vi "UNITEST MAIN v01.2.vi"() -> ()   [LabVIEW 2025]
uses:
  controls/LAB-IQ UI Data.ctl
  HEAVE vi's/Heave Write enum.ctl
  HEAVE vi's/Heave Right enum.ctl
  SWAY vi's/Sway Write enum.ctl
  SWAY vi's/Sway Right enum.ctl
  d081153b-36ca-4bc4-8478-749476f82ba4.vi
  1202965f-721d-4349-8d61-5de826f379ef.vi
  785ec975-e53d-4ed4-be48-2cc128d7a91f.vi
  02c5850b-52e8-4ed5-91f8-6f0ad62f4994.vi
  1223eb78-e4c4-4b69-bf80-185c82055158.vi
  e5651a45-6a49-4a3f-b503-ff1eaf449b4a.vi
  <vilib>/Utility/error.llb/Trim Whitespace One-Sided.vi
  support/Message Queue/Enqueue Message (Single).vi
  <vilib>/Utility/error.llb/Error Cluster From Error Code.vi
  <vilib>/Utility/file.llb/Read Delimited Spreadsheet (string).vi
  <vilib>/Utility/file.llb/Write Delimited Spreadsheet (string).vi
  <vilib>/ErrorRing/Error Ring.xnode
  support/Message Queue/LAB-IQ Message Queue.lvlib
  support/User Event - Stop/LAB-IQ User Event - Stop.lvlib
panel:
  out "Scratch Start Recording":bool
  in  "SwaySpeed Set":bool
  in  "Update":bool
  in  "Analysis Home":bool
  in  "Installation/Replacement completed":bool
  in  "Loahead":bool
  in  "Heave and Surge COM Port:":refnum<visa-resource-name>="COM9"
  in  "Sway COM Port:":refnum<visa-resource-name>="COM10"
  out "Test Trip":bool
  out "Hymidity":bool
  in  "Humidity Disable trip":bool=TRUE
  in  "CoF Trip  2":dbl=540.0 min=100.0 max=540.0 step=1.0
  in  "File Path :  2":path
  out "Wear Track Diameter":dbl
  in  "Stribeck table":bool
  in  "seq":bool=TRUE
  out "Drive Error":string
  out "mm/s  Surge":dbl=7.0 caption="Jog" min=0.001 max=50.0 step=0.0001 format="%.2f"
  in  "Update Surge Speed":bool
  out "mm/s  Sway":dbl=7.0 caption="Jog" min=0.001 max=50.0 step=0.0001 format="%.2f"
  in  "Update Sway Speed":bool
  in  "Update Heave Speed":bool
  out "mm/s Heave":dbl=7.0 caption="Jog" min=0.001 max=30.0 step=0.0001 format="%.2f"
  in  "mm/sec":dbl=1.0 caption="Jog" min=0.001 max=50.0 step=0.001 format="%.2f"
  out "Scratch Start Test":bool
  in  "HomeScratch":bool
  in  "TEST SELECTION":enum32{"Time", "Cycle"}(radio)
  in  "Sway Loop Delay":dbl
  in  "Sway PID Speed":dbl=1.0 format="%.4f"
  in  "Sway Jog Speed":dbl=1.0 format="%.4f"
  out "HEAVE ENABLE":bool
  in  "SPARE  5":u8
  in  "Manual Write SWAY":bool
  out "SWAY WRITE":string
  in  "SPARE  4":u8
  in  "SPARE  3":u8
  in  "SPARE 2":u8
  in  "SPARE 1":u8
  out "Spare 15":u8
  out "Spare 14":u8
  out "Spare 13":u8
  out "Spare 12":u8
  out "Spare 11":u8
  out "Spare 10":u8
  out "Spare 9":u8
  out "Spare 8":u8
  out "Spare 7":u8
  out "Spare 6":u8
  out "Spare 5":u8
  out "Spare 4":u8
  out "Spare 3":u8
  out "Spare 2":u8
  out "Spare 1":u8
  out "Node Id":u8
  out "Read SWAY Temp":bool
  out "fwMinor":u8
  out "fwMajor":u8
  out "faultCode":u16
  out "Rotary POSE":sgl format="%#.6f"
  out "SWAY POSE":sgl format="%#.6f"
  out "Homed":u8
  out "State":u8
  out "Ack ID":u16
  in  "SPEED":sgl=10000.0
  in  "Distance":sgl=10000.0
  in  "Mode Command":u8=2
  out "Sequence ID":u16
  out "error out Read SWAY":errorcluster
  out "error out Write  SWAY":errorcluster
  out "SWAY READ":string
  in  "min_finetune_floor":dbl=0.15
  in  "min_deadband_floor":dbl=0.05
  in  "fine_tune_pct":dbl=100.0
  out "Start Test Temp":bool
  in  "AppLoadSeq scratch":bool
  out "Pulse delta":dbl
  in  "Fine Tune Zone":dbl=10.0
  in  "PID Delay (sec)":dbl=1.0 format="%#_6p"
  in  "Max_pos_limit":dbl=50000000.0
  in  "Min_pos_limit":dbl
  in  "i_limit":dbl=10.0
  in  "Max Step Linit":dbl=10.0
  in  "Init Step":dbl=10.0
  in  "pct_scale":dbl=100.0
  in  "Deadband":dbl=0.1
  in  "Kd":dbl
  in  "Ki":dbl
  in  "Kp":dbl=1.0
  out "Current Position":dbl
  in  "Set Load":dbl
  in  "Current Load":dbl
  in  "Manual Write Heave & Surge":bool
  out "Heave and Surge Write":string
  in  "Heave Loop Delay":dbl
  in  "Heave PID Speed":dbl=15.0
  in  "Surge Jog Speed":dbl=1.0 format="%.4f"
  in  "Heave Jog Speed":dbl=15.0
  in  "SPARE 4":u8
  in  "SPARE 3":u8
  in  "SPARE 2":u8
  in  "SPARE 1":u8
  out "Spare 15":u8
  out "Spare 14":u8
  out "Spare 13":u8
  out "Spare 12":u8
  out "Spare 11":u8
  out "Spare 10":u8
  out "Spare 9":u8
  out "Spare 8":u8
  out "Spare 7":u8
  out "Spare 6":u8
  out "Spare 5":u8
  out "Spare 4":u8
  out "Spare 3":u8
  out "Spare 2":u8
  out "Spare 1":u8
  out "Node Id":u8
  out "Read Heave Temp":bool
  out "fwMinor":u8
  out "fwMajor":u8
  out "faultCode":u16
  out "SURGE POSE":sgl format="%#.6f"
  out "HEAVE POSE":sgl format="%#.6f"
  out "Homed":u8
  out "State":u8
  out "Ack ID":u16
  in  "SPEED":sgl=10000.0
  in  "Distance":sgl=10000.0
  in  "Mode Command":u8=2
  out "Sequence ID":u16
  out "error out Read":errorcluster
  out "error out Write":errorcluster
  out "Heave and Surge Read":string
  out "Load Cell Temp":bool
  in  "Stop Scratch":bool
  in  "Enter Fixed SRR 2":dbl min=0.0 max=0.0 format="%.3f"
  in  "E.Velocity 2":bool=TRUE caption="SRR"
  in  "Tab Control 3":T1(tab)
  in  "Tab Control 5":enum32{""}(tab)
  in  "Tab Control 14":T2(tab)=enum."Motor Load"
  in  "Ramp MulFac":dbl=2.0
  in  "pulses LoadDiffRamp(2..10)":dbl=9.0
  in  "PulseControlRamp(diff<=3N)":dbl=5.0 min=1.0 max=1000.0 step=1.0 format="%#.1f"
  in  "SetLoadDeadband(%) Load(0-10N)":dbl=0.1 min=0.0001 max=100.0 step=0.0001 format="%#.6f"
  in  "PID gains out delay (microForce)":T3={"proportional gain (Kc)"=300.0, "integral time (Ti, min)"=0.00011, "derivative time (Td, min)"=0.0} {"derivative time (Td, min)" format="%.3f"; "integral time (Ti, min)" min=1e-05 max=100.0 step=1e-06 format="%.6f"; "proportional gain (Kc)" format="%.3f"}
  in  "Ramp":bool
  in  "Gain 2":dbl=0.016
  in  "pulses LoadDiff(2..10)":dbl=10.0
  in  "pulses LoadDiff(11..50)":dbl=40.0
  in  "PulseControl(diff<=3N)":dbl=1.0 min=1.0 max=1000.0 step=1.0 format="%#.1f"
  out "SetLoadDeadband(%)  2":dbl=1.0 min=0.001 max=100.0 step=0.001 format="%#.6f"
  in  "Dummy Run":bool
  out "Vertical load (N)":dbl format="%#.3f"
  in  "AutoTune":bool
  in  "Offset  3":dbl=1.5
  in  "apply load":bool
  in  "Enter ByPass Load":dbl
  in  "reinit 3":bool=TRUE
  in  "output range delay":cluster{"output high":dbl, "output low":dbl}={"output high"=100.0, "output low"=-100.0} {"output low" format="%.2f"; "output high" format="%.2f"}
  in  "PID gains out delay":T3={"proportional gain (Kc)"=30.0, "integral time (Ti, min)"=0.00101, "derivative time (Td, min)"=0.0} {"derivative time (Td, min)" format="%.3f"; "integral time (Ti, min)" min=1e-05 max=100.0 step=0.0001 format="%.4f"; "proportional gain (Kc)" format="%.3f"}
  in  "Bypass Load":bool
  in  "pulsesSent":dbl=200.0
  out "pulses":dbl
  out "actpid":dbl
  out "gFF Rot 7":cluster{dbl, dbl, dbl}(graph)
  in  "pulses LoadDiff(21..1000)":dbl=40.0
  in  "Delay":dbl=1.5 min=0.001 max=5.0 step=0.001 format="%#.6f"
  in  "deadband":dbl=0.2
  in  "Tab Control 26":enum32{"Page 1", "Page 2"}(tab)
  in  "ClearAll":bool
  out "Mz(Nm)":dbl[](array[numeric])
  out "My(Nm)":dbl[](array[numeric])
  out "Mx(Nm)":dbl[](array[numeric])
  in  "Save Dwell":dbl=0.015 caption="Save Dwell (sec)" min=0.0 max=5.0 step=0.001 format="%.3f"
  out "Mx":dbl[](graph)
  out "My":dbl[](graph)
  out "Mz":dbl[](graph)
  out "Fy(N)":dbl[](graph)
  out "Fz(N)":dbl[](graph)
  in  "ZeroAll":bool
  in  "Acq Delay (ms)":dbl=10.0
  in  "Burst Delay (ms)":dbl=10.0
  out "model":string
  out "SN":i32
  out "FFx(N)":dbl[](array[numeric])
  in  "Sensor IP":string="192.168.1.100"
  in  "Port":i32=8080
  out "FFy(N)":dbl[](array[numeric])
  out "Load(N)":dbl[](array[numeric])
  out "Fx(N)":dbl[](graph)
  out "AE":bool
  in  "delete Handle":bool
  in  "Create Handle":bool=TRUE
  out "ft_data":dbl[](array[numeric])=[1.0, 1.0, 1.0, 1.0, 1.0, 1.0]
  out "ft_range":dbl[](array[numeric])=[1.0, 1.0, 1.0, 1.0, 1.0, 1.0]
  in  "stop 6":bool
  out "running_flag":bool
  out "ft_udp_handle":i32
  out "get-data-return":i32
  out "get-range-return":i32
  out "zero-return":i32
  out "filter-return":i32
  out "initial-return":i32
  out "deleteHandle-result":i32
  in  "Tab Control 19":enum32{"Platform COM", "Config ", "DevInfo"}(tab)=enum."Config "
  in  "SAMPLES":dbl=100.0
  in  "Re-initilaize":bool
  in  "Filter ON/OFF":bool=TRUE
  in  "TracHomeSurgeOffsetCounts 10MM":dbl=505100.0
  in  "TracHomeSwayOffsetCounts 10MM":dbl=1432.0
  in  "Acoustic Emission:":dbl=1.0 min=0.0001 max=200.0 step=0.0001 format="%.4f"
  in  "Apply Filter (FF)":bool
  in  "Filter% 2":dbl=50.0 min=50.0 max=100.0 step=0.1 format="%.1f"
  in  "Apply Filter (Load)":bool=TRUE
  in  "Filter%":dbl=80.0 min=50.0 max=100.0 step=0.1 format="%.1f"
  in  "Sway distance (mm)":dbl=245.0
  in  "Surge distance (mm)":dbl=370.0
  in  "DataSavingLoopDelay(ms)":dbl=15.0
  in  "SAVE  2":bool
  in  "Enter Distance":bool caption="Enter Counts"
  in  "Sway Counts:":dbl=100.0 min=0.0 max=100000000.0 step=1.0 format="%.2f"
  in  "Distance (mm): 3":dbl=100.0 caption="Distance (mm):" min=0.0 max=1500.0 step=0.001 format="%.5f"
  in  "Surge Counts:":dbl=100.0 min=0.0 max=100000000.0 step=1.0 format="%.1f"
  in  "Distance (mm): 2":dbl=100.0 caption="Distance (mm):" min=0.0 max=1500.0 step=0.0001 format="%.3f"
  in  "Distance (mm):":dbl=100.0 min=0.0 max=1500.0 step=0.001 format="%.5f"
  in  "Heave Counts:":dbl=100.0 min=0.0 max=100000000.0 step=1.0
  in  "LRMHomeSurgeOffsetCounts":dbl=307197.0
  in  "LRMHomeSwayOffsetCounts":dbl=26880.0
  in  "TracHomeSurgeOffsetCounts 20MM":dbl=505100.0
  in  "TracHomeSwayOffsetCounts 20MM":dbl=1432.0
  in  "RotHomeSwayOffsetCounts":dbl=14656.0
  in  "RotHomeSurgeOffsetCounts":dbl=311465.0
  in  "Heave distance":dbl=340.0
  out "Zmm":dbl=1600.0
  out "Heave Pulses/mm":dbl=1600.0
  out "Surge Pulses/mm":dbl=1600.0
  out "Sway Pulses/mm":dbl=320.0
  in  "Heave Pitch":dbl=4.0
  in  "Surge Pitch":dbl=3.0
  in  "Sway Pitch":dbl=2.0
  in  "Heave PPR":dbl=6400.0
  in  "Surge PPR":dbl=6400.0
  in  "Sway PPR":dbl=6400.0
  in  "GUI":T4(tab)
  in  "Platform Settings":bool caption="Password"
  in  "Configure":bool caption="Password"
  in  "Home":bool caption="Password"
  in  "EXIT":bool
  in  "Analysis":bool caption="Password"
  in  "service 2":bool caption="Password"
  in  "MainPage":T5(tab)=enum."HOME"
  in  "Select Load Head":bool
  in  "Notes :":string
  in  "FILE":string
  in  "Sample ID :":string
  in  "Operator ID :":string
  in  "Operator Name :":string
  in  "Auto":bool caption="Power Status"
  in  "Disable Axis Jog Soft Limits m":bool
  out "Sway and Surge COM Status":bool=TRUE caption="Load COM Status"
  out "Heave COM Status":bool=TRUE caption="Load COM Status"
  in  "Enable Platform":bool
  in  "Surge Forward Main":bool
  in  "Surge Backward Main":bool
  in  "Sway Right Main":bool
  in  "Sway Left Main":bool
  in  "Heave Down Main":bool
  in  "Heave Up main":bool
  in  "mm":dbl=0.001 caption="Jog" min=1.0 max=100.0 step=0.01 format="%#.3f"
  in  "Surface Analysis":bool
  in  "Imaging":bool
  in  "Image Analysis":bool
  in  "Post Analysis":bool
  in  "SSP 0.75":bool
  in  "SSP 0.5":bool
  in  "SSP 0.3":bool
  in  "Warning":enum32{"Page 2"}(tab)
  in  "gui GIF":enum32{"Check", "Deca", "kilo", "Micro"}(tab)
  out "Communication is established":bool=TRUE caption="Load COM Status"
  in  "Reference Sample":u16(ring) items=["None", "Brass", "Aluminium", "Mild Steel"]
  out "Load Cell Communication Slide":u8(slide)=1 min=1 max=10 step=1 scale=0.0..10.0
  in  "com 3":bool
  out "com":bool
  out "DecaForce COM Status":bool caption="Load COM Status"
  in  "Loading Mode":u16(ring) items=["Constant", "Ramp", "Steps", "Indentation"]
  in  "Enter the CoF Trip":dbl=1.0
  in  "Enter the Friction Force Trip":dbl=520.0 min=500.0 max=500.0 step=1.0 format="%#.1f"
  in  "Enter the Normal load Trip":dbl=520.0 min=500.0 max=500.0 step=0.001 format="%.3f"
  in  "KiloForce":bool
  in  "DecaForce":bool
  in  "MicroForce":bool
  in  "LHBack":bool
  in  "LHNext":bool
  in  "Load Selection":T6(tab)
  in  "Enter the Load  (N)":dbl=2.0 caption="Enter the Load (N)" min=2.0 max=200.0 step=0.1 format="%#.4f"
  in  "Enter the Final Load (N)":dbl=1.0 min=0.0 max=500.0 step=1.0 format="%#.0f"
  in  "Enter the Loading Rate (N/min)":dbl=60.0 min=1.0 max=1200.0 step=0.1 format="%.2f"
  out "Warning 2":bool
  in  "Stribeck Table  For loading":string[][](table)
  in  "Clear 3":bool
  out "Message":string="Load Entered is out of range!!!"
  in  "Indentation":string[][](table)=[["Detection", "5", "2"], ["Unload", "0", "5"], ["Load", "10", "2"], ["Unload", "0", "5"], ["Detection", "5", "2"], ["Unload", "0", "5"]]
  in  "Multipoint":bool caption="Singlepoint"
  in  "AppLoad 4":bool
  in  "zNL":bool
  out "NL disp":dbl caption="Normal Load ( N )" min=-2000.0 max=2000.0 step=0.0001 format="%.1f"
  in  "Traction":bool
  in  "Surge Forward MM":bool
  in  "Surge Backward MM":bool
  in  "M3 Image":enum32{"Page 1", "Page 2"}(tab)
  in  "String 39":string="Jog heave to bring the upper sample closer to the lower sample within 1mm."
  in  "Sway Left MM":bool
  in  "Sway Right MM":bool
  in  "Disable Axis Jog Soft Limits":bool
  in  "mm":dbl=0.001 caption="Jog" min=0.001 max=5.0 step=0.0001 format="%#.3f"
  in  "Heave Down MM":bool
  in  "Heave Up MM":bool
  in  "Wear Track Diameter (mm)":dbl=30.0 caption="Wear Track Diameter (mm):" min=1.0 max=30.0 step=1.0 format="%.2f"
  in  "Set WTD":bool
  in  "HomeScratch":bool
  in  "HomeRot":bool
  in  "PlaceModule":bool
  in  "Motion Mode:":u16(ring) items=["Uniform Rotation", "Angular Oscillation", "Stribeck ", "Steps"]
  in  "LR Sway":bool
  in  "Rot Hor":bool
  in  "Rot Ver":bool
  in  "Scratch":bool
  in  "LR Cam":bool
  in  "MMBack":bool
  in  "MMNext":bool
  in  "Rotary Module Selection":T7(tab)
  in  "SPEED SELECTION :":enum32{"Speed in RPM", "Speed in m/sec"}(radio)=enum."Speed in m/sec"
  in  "Enter the Speed(mm/sec)":dbl=0.1 min=0.1 max=10.0 step=0.1 format="%.3f"
  in  "Enter the Speed (RPM)":dbl=45.0 min=1.0 max=3000.0 step=1.0
  in  "Enter the Frequency (Hz)":dbl=1.0 min=0.1 max=10.0 step=0.1 format="%.1f"
  in  "Enter the Angle (Deg)":dbl=45.0 min=5.0 max=300.0 step=1.0
  in  "Angular Oscillation Set":bool
  in  "Rotary Tab":enum32{"Page 1", "Page 2"}(tab)
  out "e.v/ssr 2":enum32{"E.V", "SSR"}(tab)
  in  "Enter the Final E.Velocity (m/s) 2":dbl=1.0 min=0.001 max=4.0 step=0.001 format="%.3f"
  in  "Enter initial E.Velocity (m/s) 2":dbl=2.0 min=0.001 max=4.0 step=0.001 format="%.3f"
  in  "Enter Fixed E.Velocity 2":dbl=1.0 min=0.001 max=2.0 step=0.001 format="%.3f"
  in  "Enter Final SRR 2":dbl=1.0 min=0.001 max=1.0 step=0.001 format="%.2f"
  in  "Enter initial SRR 2":dbl=1.0 min=0.001 max=1.0 step=0.001 format="%.2f"
  out "Final Speed (RPM) 3":dbl=1.0 min=0.1 max=3000.0 step=0.1 format="%.1f"
  out "Initial Speed (RPM) 2":dbl=100.0 min=0.1 max=3000.0 step=0.1 format="%.1f"
  in  "Enter the Final Velocity (m/s) 3":dbl=1.0 min=0.001 max=2.0 step=0.001 format="%.3f"
  in  "Enter initial Velocity (m/s)  3":dbl=2.0 min=0.001 max=2.0 step=0.001 format="%.3f"
  out "Ramp Up 2":bool caption="Ramp Down"
  in  "Import 2":bool
  in  "Save 2":bool
  in  "SPEED SELECTION : rotary":enum32{"Speed in Rpm", "Speed in m/sec"}(radio)=enum."Speed in m/sec"
  in  "calculate rotary":bool
  in  "String 45":string="File Path Location : C:-->LAB-IQ 150 --> User Defined\n                                       Protocol-->File.txt"
  in  "Step Speed":enum32{"Step Speed", "Step (load-Speed)"}(tab)
  in  "StepTable For Speed":string[][](table)
  in  "StepTable For Load-Speed":string[][](table)=[["", "", ""], ["", "", ""], ["", "", ""], ["", "", ""]]
  in  "StepTable For Speed 3":string[][](table)=[["", "", ""], ["", "", ""], ["", "", ""], ["", "", ""]]
  in  "Motion Direction:  3":u16(ring) items=["Clockwise", "Counter Clockwise"]
  in  "Enter Scratch length (mm):":dbl=1.0 min=1.0 max=50.0 step=0.0001 format="%.4f"
  in  "Enter Scratch Speed (mm/s):":dbl=1.0 min=0.003 max=10.0 step=0.0031 format="%.5f"
  in  "Scartch Offset":dbl=1.0 caption="Scratch Offset: (mm)" min=0.1 max=5.0 step=0.1 format="%.1f"
  in  "Motion type:":u16(ring) items=["Unidirection", "Bidirection"]
  in  "Scratch Mode":u16(ring) items=["Scratch", "Pre-Post Scan", "Multi Scratch"]
  in  "Rotary Speed Exced":string="Motor Speed Out of Range"
  in  "No of Scratch":dbl=1.0 min=1.0 max=50.0 step=0.0001
  out "Humidity  Status  3":bool caption="Communication Status"
  out "Low Temp  Status  2":bool=TRUE caption="Communication Status"
  out "TK4 status 2":bool=TRUE caption="Communication Status"
  in  "String 40":string="Before selecting Acoustic make sure the sensor output pin is connected to A4."
  in  "Stage Temperature":dbl[](array[numeric])=[150.0, 230.0, 300.0, 350.0, 400.0, 450.0, 500.0]
  in  "Sample Temperature":dbl[](array[numeric])=[100.0, 150.0, 200.0, 250.0, 300.0, 350.0, 400.0]
  in  "Humidity (Amb)":bool
  in  "Clear List":bool
  out "Sensors Picked":string
  in  "Add to list":bool
  in  "Wear":bool
  in  "Vibration":bool
  in  "Humidity (Chamber)":bool
  in  "Temperature (Chamber)":bool
  in  "ECR":bool
  in  "Temperature (Amb)":bool
  in  "Microphone":bool
  in  "Acoustic Emission 3":bool
  in  "SNext":bool
  in  "APBack":bool
  in  "Enter the Temperature (°C):":dbl
  in  "Enter the Stage \nTemperature (°C):":dbl=20.0 min=20.0 max=150.0 step=1.0 format="%#.0f"
  in  "Enter the Humidity (%Rh):":dbl=30.0 min=30.0 max=85.0 step=1.0
  in  "Low Temp":bool
  in  "High Temp":bool
  in  "Humidity":bool
  in  "Main Screen Tab":T8(tab)
  in  "ClrLog":bool
  out "Trip Log":string
  in  "Start Test":bool
  out "Test status":bool caption="Test Status"
  out "AR Led":bool caption="AR"
  out "Data":bool=TRUE
  out "Health":bool=TRUE
  out "Sway COM Status":bool=TRUE caption="Load COM Status"
  out "Heave COM Status":bool=TRUE caption="Load COM Status"
  in  "Grp Tab":enum32{"Rot/LRM", "FBT"}(tab)
  out "Depth Trip":dbl=600.0
  in  "Depth Trip":bool=TRUE
  out "Weart Deapth":bool
  in  "Depth Reset Graph":bool
  out "Weart":bool
  in  "Depthz":bool
  out "Depth (µm)":dbl min=-200.0 max=200.0 step=0.1 format="%.1f"
  out "WearGp":dbl(graph)=0.13298760003255525
  out "NL Trip 2":dbl=600.0
  out "Load pid":bool
  in  "Load Disable Trip":bool=TRUE
  in  "Load Reset Graph":bool
  out "NL Display 4":dbl caption="Normal Load ( N )" min=-2000.0 max=2000.0 step=0.0001 format="%.1f"
  out "Main Chart 3":cluster{dbl, "NL disp":dbl, dbl}(graph)
  in  "FF Tab":T9(tab)
  in  "COF Reset Graph":bool
  in  "COF Disable Trip":bool=TRUE
  out "COF TRIP":dbl=600.0
  out "Coefficient of Friction":dbl(graph)=0.13298760003255525
  in  "zFF":bool
  in  "FF Reset Graph":bool
  in  "FF Disable Trip":bool=TRUE
  out "FF TRIP":dbl=600.0
  out "Friction Force (N)":dbl min=-2000.0 max=2000.0 step=0.0001 format="%.3f"
  out "Friction Force (N) Graph":dbl(graph)=0.13298760003255525
  out "Cyclic FF TRIP":dbl=600.0
  in  "Cyclic FF Disable Trip":bool=TRUE
  in  "Cyclic FF Reset Graph":bool
  in  "CZ FF":bool
  out "Cyclic Friction Force (N) Graph":dbl(graph)=0.13298760003255525
  out "Cyclic Friction Force (N)":dbl min=-2000.0 max=2000.0 step=0.0001 format="%.3f"
  out "cyclic COF TRIP":dbl=600.0
  in  "cyclic COF Disable Trip":bool=TRUE
  in  "cyclic COF Reset Graph":bool
  out "Cyclic Coefficient of Friction":dbl(graph)=0.13298760003255525
  in  "Sub Graph":T10(tab)
  in  "Speed Tab":enum32{" Rotary Disc", "MTM Ball", "MTM Disc"}(tab)
  out "speed mm/sec":dbl(graph)=0.13298760003255525
  in  "Speed Reset Graph":bool
  out "MTM BALL SPEED":dbl(graph)=0.13298760003255525
  out "MTM DISC  SPEED":dbl(graph)=0.13298760003255525
  in  "Temperature Reset":bool
  out "Temperature (deg c)":dbl(graph)=0.13298760003255525
  in  "ECR RESET":bool
  out "ECR":dbl(graph)=0.13298760003255525
  out "Acoustic Emission (mV)":dbl min=0.0 max=5000.0 step=0.1
  in  "Aqucostic Reset Graph":bool
  out "gACQUOS":dbl(graph)=0.13298760003255525
  in  "Humidity Reset Graph":bool
  out "HumrGp":dbl(graph)=0.13298760003255525
  out "SD (mm)":dbl caption="Sliding Distance ( mm )" min=-200.0 max=200.0 step=0.1 format="%.4f"
  in  "Siliding distance Reset Graph":bool
  out "SDGp":dbl(graph)=0.13298760003255525
  in  "BACK":bool
  out "Ambient \nTemperature":dbl min=0.0 max=5000.0 step=0.1 format="%.1f"
  out "Ambient\n Humidity":dbl min=0.0 max=5000.0 step=0.1 format="%.2f"
  out "NL disp 2":dbl caption="Normal Load ( N )" min=-2000.0 max=2000.0 step=0.0001 format="%.1f"
  out "Set Humidity":dbl caption="Set Humidity  (% Rh)" min=-2000.0 max=2000.0 step=1.0 format="%.1f"
  out "humidity disp":dbl caption="Humidity (% Rh)" min=-2000.0 max=2000.0 step=1.0 format="%.1f"
  in  "Humidity On":bool
  in  "zNL 2":bool
  out "NLt":bool
  in  "Load En":bool
  out "Freq (Hz)":dbl min=0.0 max=5000.0 step=0.1 format="%.4f"
  out "HumCOMStatus":bool caption="Communication Status"
  out "Load Communication":bool
  in  "Temp Tabs":enum32{"Low Temp", "High Temp"}(tab)=enum."High Temp"
  out "Controller  Status":bool
  out "ChamberTemp":dbl format="%#.1f"
  in  "SetTmp":dbl=-190.0 caption="Set Temperature (Deg C)" min=-190.0 max=100.0 step=1.0 format="%.1f"
  in  "Cooling":bool
  in  "Heater":bool
  out "TK4 status":bool caption="Controller  Status"
  out "ChamberTemp":dbl format="%#.1f"
  in  "SetTmp":dbl caption="Set Temperature (Deg C)" min=0.0 max=1000.0 step=1.0 format="%.1f"
  in  "Set Load (N)":dbl=100.0 min=0.01 max=1500.0 step=0.01 format="%.1f"
  in  "Time Tab":enum32{"cycles", "duration"}(tab)=enum."duration"
  out "Test Duration 4":dbl=600.0 caption="Test Duration\n(HH:MM:SS)" min=0.0083 max=180000.0 step=0.0001 format="%<%H:%M:%S>t"
  out "TEST CYCLE":dbl min=0.0 max=5000.0 step=0.01 format="%.2f"
  in  "TOTAL CYCLES":dbl min=0.0 max=5000.0 step=0.1 format="%.4f"
  out "Time ( HH:MM:SS ) 2":dbl min=0.0 max=144000.0 step=1.0 format="%<%H:%M:%S>t"
  in  "Test Duration":dbl=600.0 caption="Test Duration\n(HH:MM:SS)" min=0.0083 max=180000.0 step=0.0001 format="%<%H:%M:%S>t"
  in  "Main Speed Tab":enum32{"ROTARY", "TRACTION"}(tab)
  in  "SPEED TAB":enum32{"RPM", "m/sec"}(tab)
  out "Speed (RPM)":dbl min=0.0 max=5000.0 step=0.1 format="%.1f"
  out "Set Speed":dbl caption="Set Speed (RPM)" min=0.0 max=1500.0 step=0.1 format="%.1f"
  out "Speed (m/sec)":dbl min=0.0 max=5000.0 step=0.001 format="%.4f"
  out "Set Speed (m/sec)":dbl min=0.0 max=1500.0 step=0.001 format="%.4f"
  in  "MTM MOTOR DISPLAY":enum32{"MTM RPM", "MTM m/sec"}(tab)
  out "Disc Speed (RPM)":dbl min=0.0 max=1500.0 step=0.1 format="%.1f"
  out "Ball Speed (RPM)":dbl min=0.0 max=1500.0 step=0.1 format="%.1f"
  out "Disc Speed (m/sec)":dbl min=0.0 max=1500.0 step=0.1 format="%.1f"
  out "Ball Speed (m/sec)":dbl min=0.0 max=1500.0 step=0.1 format="%.1f"
  in  "Angle and Frequency":enum32{"angular", "lrm"}(tab)
  out "Angle (Deg)":dbl min=0.0 max=5000.0 step=0.01 format="%.2f"
  out "Stroke (mm)":dbl min=0.0 max=5000.0 step=0.01 format="%.2f"
  in  "STOP":bool
  out "Multi Scratch Pass":dbl min=0.0 max=5000.0 step=0.1
  in  "X-AXIS":u16(ring) items=["None", "Time ( Sec )", "Normal Load ( N )", "Frictional Force ( N )", "Coefficient of Friction", "Depth ( Microns )", "Speed ( RPM )", "Frequency ( Hz )", "Angle ( Degree )", "Cyclic Friction Force ( N )", "Cyclic Co efficient Friction ", "Stage temperature ( Degree celcius )", "Sample temperature ( Degree celcius )", "Stroke Length ( mm )", "Scratch Speed ( mm/sec )", "Amb Humidity ( % Rh ) ", "Amb Temperature (Deg C)", "Acoustic (mV)", "Mx (Nm)", "My (Nm)", "Mz (Nm)", "Humidity ( % Rh )", "Sliding Distance (mm)", "Wear Track Diameter (mm)", "Fx(N)", "Fy(N)", "MTM BallSpeed (RPM)", "MTM DiscSpeed (RPM)", "Entrainment Speed", "Slide Role", "Slip(%)", "Rotary Speed (m/sec)", "MTM Ball Speed (m/sec)", "MTM Disc Speed (m/sec)", "ECR (ohms)"]
  in  "Y-AXIS":u16(ring) items=["None", "Time ( Sec )", "Normal Load ( N )", "Frictional Force ( N )", "Coefficient of Friction", "Depth ( Microns )", "Speed ( RPM )", "Frequency ( Hz )", "Angle ( Degree )", "Cyclic Friction Force ( N )", "Cyclic Co efficient Friction ", "Stage temperature ( Degree celcius )", "Sample temperature ( Degree celcius )", "Stroke Length ( mm )", "Scratch Speed ( mm/sec )", "Amb Humidity ( % Rh ) ", "Amb Temperature (Deg C)", "Acoustic (mV)", "Mx (Nm)", "My (Nm)", "Mz (Nm)", "Humidity ( % Rh )", "Sliding Distance (mm)", "Wear Track Diameter (mm)", "Fx(N)", "Fy(N)", "MTM BallSpeed (RPM)", "MTM DiscSpeed (RPM)", "Entrainment Speed", "Slide Role", "Slip(%)", "Rotary Speed (m/sec)", "MTM Ball Speed (m/sec)", "MTM Disc Speed (m/sec)", "ECR (ohms)"]
  out "XY Graph":cluster{"Array 2":dbl[], "Array 2":dbl[]}[](graph) caption="XY Graph 20"
  out "VARIANCE":dbl=-0.0 format="%0.2f"
  out "SD":dbl=-0.0 format="%.3f"
  out "MEAN":dbl format="%.3f"
  out "VARIANCE":dbl=-0.0 format="%0.2f"
  out "SD":dbl=-0.0 format="%.3f"
  out "MEAN":dbl format="%.3f"
  out "VARIANCE":dbl=-0.0 format="%0.2f"
  out "SD":dbl=-0.0 format="%.3f"
  out "MEAN":dbl format="%.3f"
  out "VARIANCE":dbl=-0.0 format="%0.2f"
  out "SD":dbl=-0.0 format="%.3f"
  out "MEAN":dbl format="%.3f"
  in  "Analysis Home new":bool
  out "File 2 Discription":string="\r"
  out "File 1 Discription":string="\r"
  in  "OPEN 1":bool
  in  "OPEN 2":bool
  out "File Name 1":string
  out "File Name 2":string
  in  "Refresh 2":bool
  in  "OPEN 3":bool
  out "File Name 3":string
  out "File Name 4":string
  in  "OPEN 4":bool
  out "File 4 Discription":string="\r"
  out "File 3 Discription":string="\r"
  in  "Password":string
  in  "Home Service":bool
  in  "Advanced Setting":bool
  in  "About Tab":enum32{"Primary"}(tab)
  in  "ECR Port:":refnum<visa-resource-name>="COM10"
  in  "Ramp Port:":refnum<visa-resource-name>="COM10"
  in  "Temp Modbus:":refnum<visa-resource-name>="COM14"
  in  "Humidity Port:":refnum<visa-resource-name>="COM10"
  in  "Edit Gain Constants":bool
  in  "Save Gain Constants":bool
  in  "Service About":bool
  # "SET JOG SPEED"
  # "NOTE: This operation needs to be done only when the machine is ON."
  # "Speed Exceed the limit of the Motor"
  # "Motor Speed Out of Range"
  # "load Aquisition off"
  # "load Aquisition On"
  # "Configuration"
  # "Limits for Heave Surge and Sway"
  # "Modules Offset Parameters"
  # "Counts-Distance Calculator"
  # "File Name :"
  # "Ensure the traction module is aligned\n horizontally with the stage before ENABLE."
  # "JOG MODE"
  # "Module Selection"
  # "Positioning Control"
  # "Connect the controller\ncable to M3"
  # "Environment"
  # "Sensors"
  # "Data Points"
  # "Data Points"
  # "Data Points"
  # "Data Points"
  # "ohms"
  # "Data Points"
  # "Data Points"
  # "Data Points"
  # "LAB-IQ 150 / UNITEST / WO2456 / UT150  v05 / AUGUST 2025"
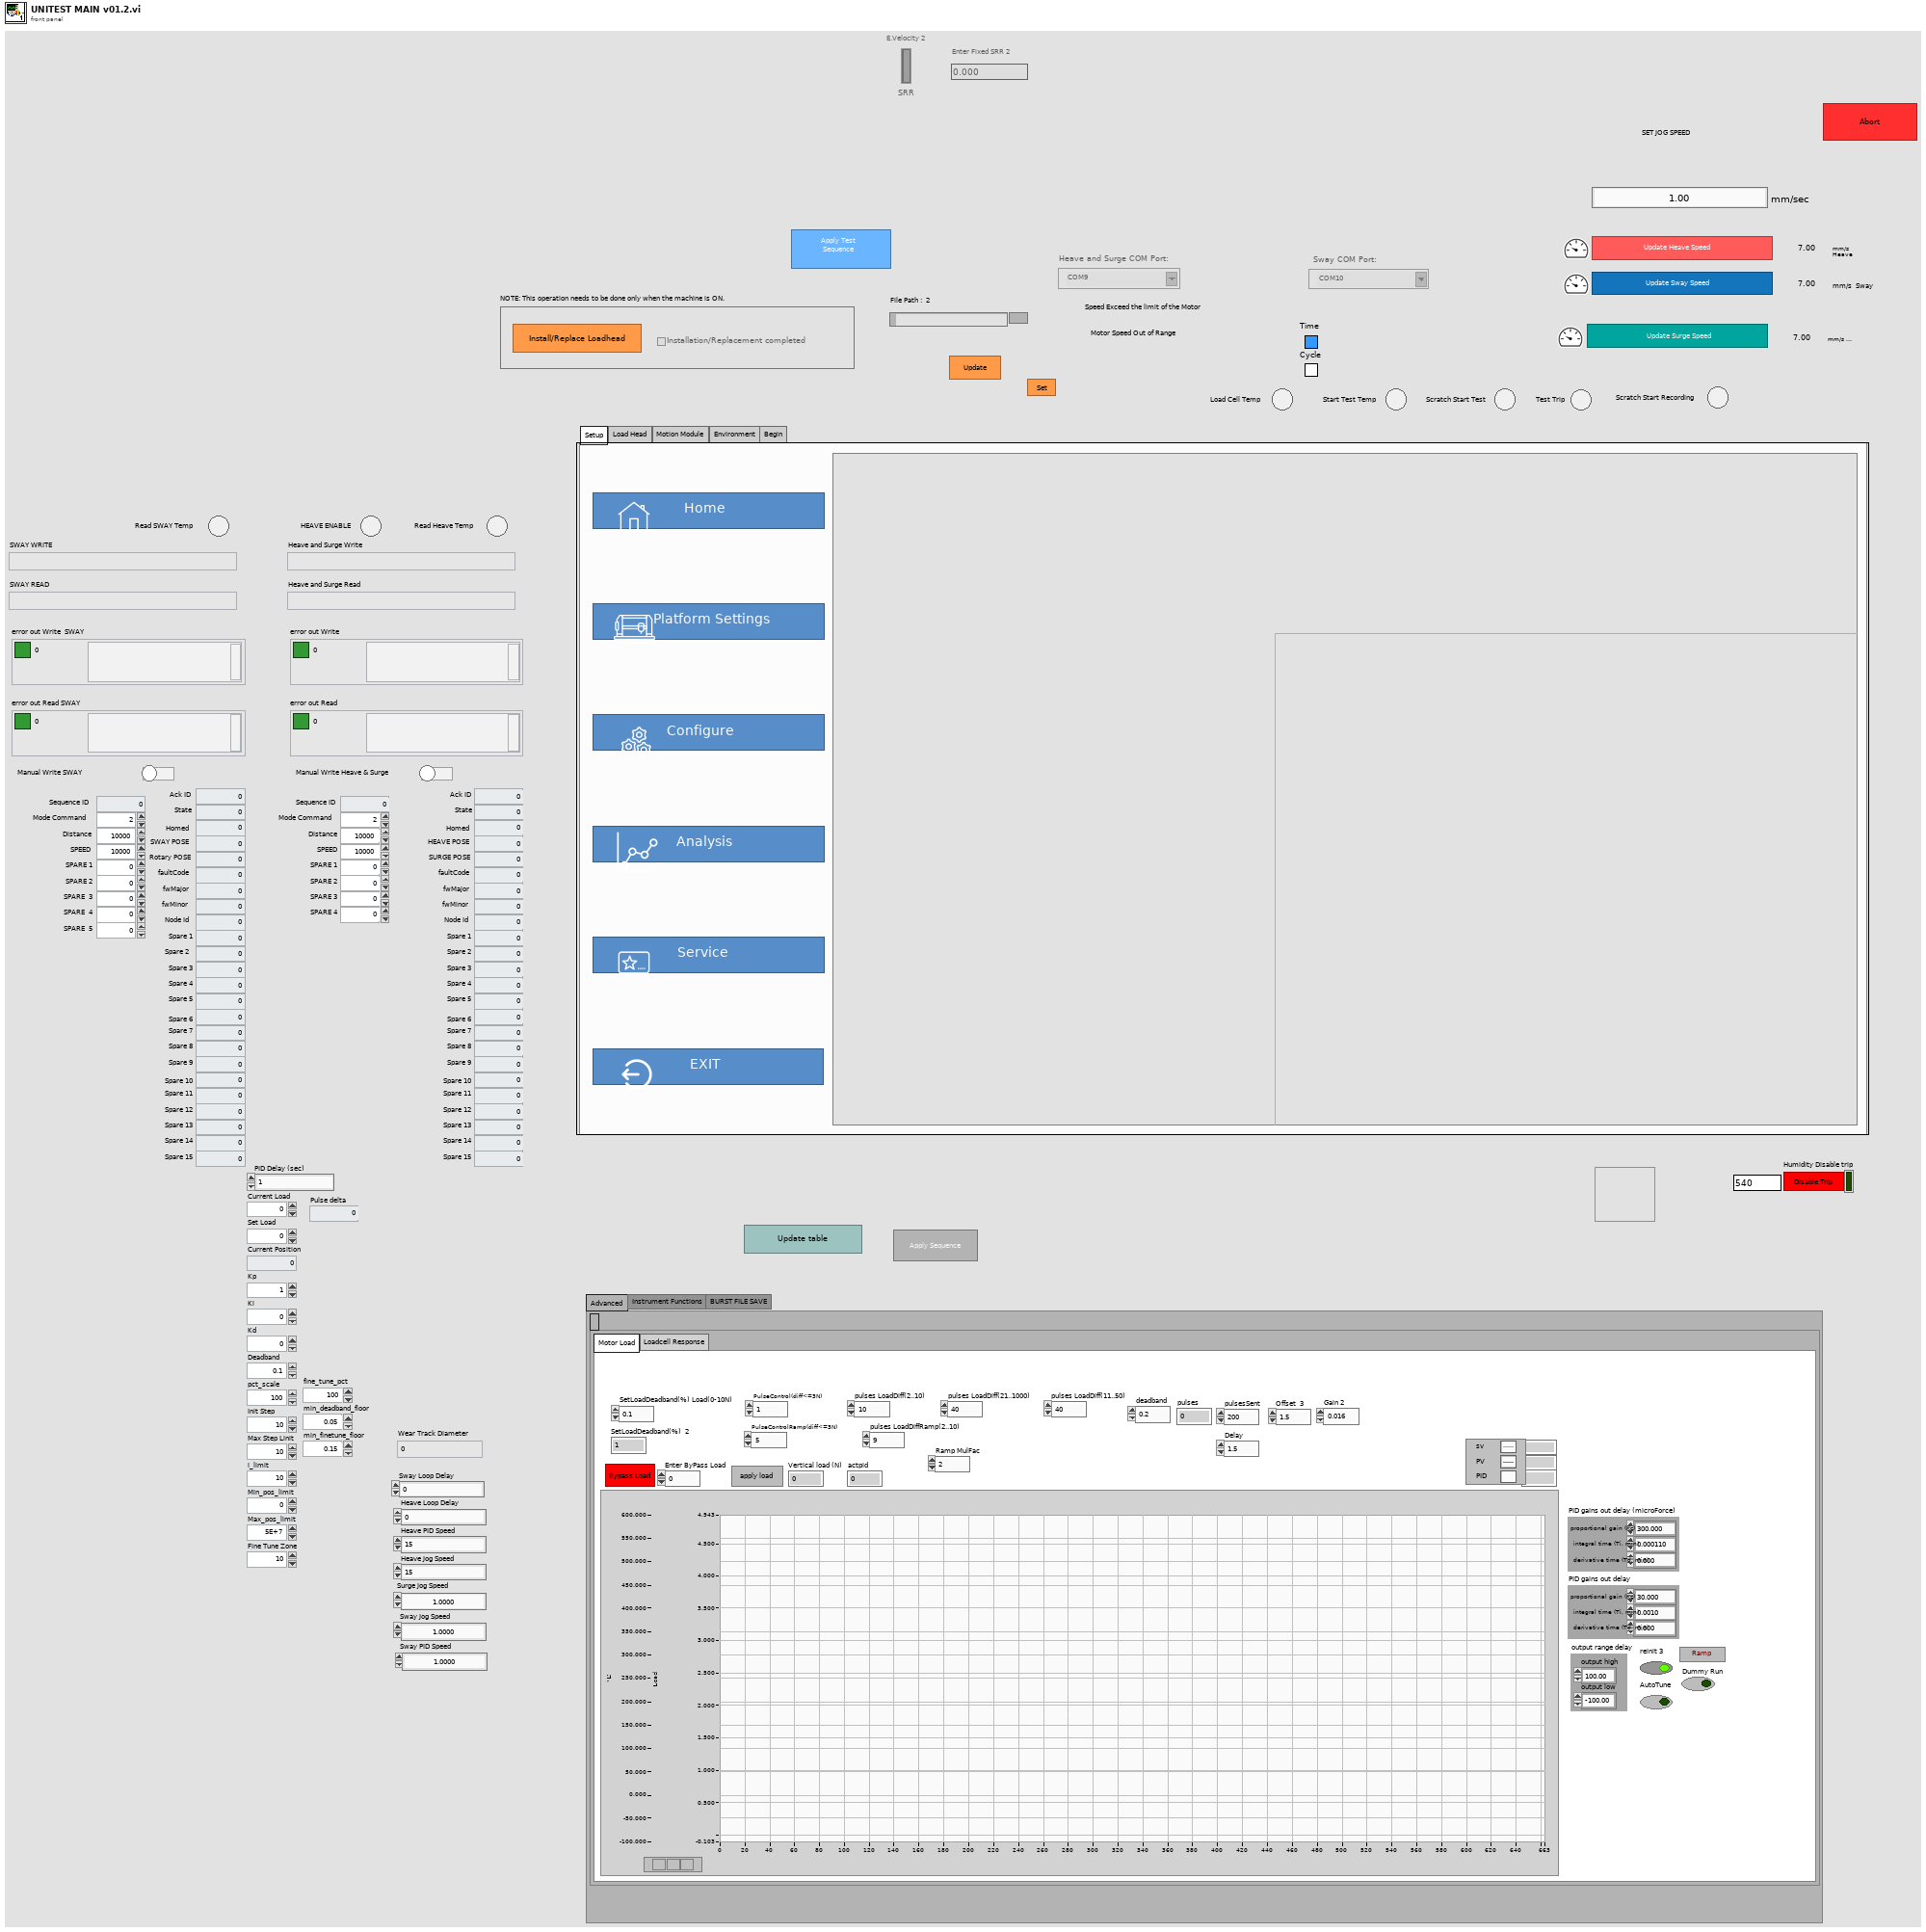
[diagram p1: front panel]
types:
  T1 = enum32{"Advanced", "Motor", "Depth_graph", "UIO Communicator", "Add to list parametrs", "Instrument Functions", "BURST FILE SAVE"}
  T2 = enum32{"LRM heating", "FBT_Heating", "Motor Load", "Loadcell Response", "Voice Load", "Step loading and speed ", "Depth"}
  T3 = cluster{"proportional gain (Kc)":dbl, "integral time (Ti, min)":dbl, "derivative time (Td, min)":dbl}
  T4 = enum32{"Setup", "Load Head", "Motion Module", "Environment", "Begin"}
  T5 = enum32{"Details", "PlatformSetting", "Analysis", "HOME"}
  T6 = enum32{"Constant", "Ramp", "Step", "Indentation"}
  T7 = enum32{"Uniform Rotation", "Angular Oscillation", "Speed Ramp", "Speed Step"}
  T8 = enum32{"  Acquire  ", "Compare Files Rot", "About", "Service"}
  T9 = enum32{"Coefficient of Friction ", "Friction Force (N)", "Cyclic Friction Force (N)", "Cyclic Coefficient of Friction "}
  T10 = enum32{"Speed", "Temperature", "ECR", "Acoustic Emission", "Humidity", "Sliding Distance"}
  T11 = typedef "LAB-IQ UI Data.ctl" = cluster{"Main Home Screen":cluster{"GUI":refnum<vi>, "Platform Settings":refnum<vi>, "Configure":refnum<vi>, "Home":refnum<vi>, "EXIT":refnum<vi>, "service 2":refnum<vi>, "MainPage":refnum<vi>, "Analysis":refnum<vi>}, "Platform Settings":cluster{"mm/s  Surge":refnum<vi>, "Update Surge Speed":refnum<vi>, "Drive Error":refnum<vi>, "Disable Axis Jog Soft Limits":refnum<vi>, "mm/s  Sway":refnum<vi>, "Sway and Surge COM Status":refnum<vi>, "Heave COM Status":refnum<vi>, "Enable Platform":refnum<vi>, "Surge Forward Main":refnum<vi>, "Sway Right Main":refnum<vi>, "Sway Left Main":refnum<vi>, "Heave Down Main":refnum<vi>, "Heave Up main":refnum<vi>, "Update Sway Speed":refnum<vi>, "Update Heave Speed":refnum<vi>, "mm/s Heave":refnum<vi>, "mm/sec":refnum<vi>, "mm":refnum<vi>, "Surge Backward Main":refnum<vi>}, "Analysis Screen":cluster{"Analysis Home":refnum<vi>, "Surface Analysis":refnum<vi>, "Imaging":refnum<vi>, "Image Analysis":refnum<vi>, "Post Analysis":refnum<vi>}, "Config Screen":cluster{"Select Load Head":refnum<vi>, "Notes :":refnum<vi>, "FILE":refnum<vi>, "Sample ID :":refnum<vi>, "Operator ID :":refnum<vi>, "Operator Name :":refnum<vi>, "Auto":refnum<vi>}, "Motion Module":cluster{"zNL":refnum<vi>, "NL disp":refnum<vi>, "Rotary Tab":refnum<vi>, "Motion Direction:  3":refnum<vi>, "E.Velocity 2":refnum<vi>, "e.v/ssr 2":refnum<vi>, "Enter Fixed E.Velocity 2":refnum<vi>, "Enter Final SRR 2":refnum<vi>, "Enter initial SRR 2":refnum<vi>, "Enter Fixed SRR 2":refnum<vi>, "Enter the Final E.Velocity (m/s) 2":refnum<vi>, "Enter initial E.Velocity (m/s) 2":refnum<vi>, "Final Speed (RPM) 3":refnum<vi>, "Initial Speed (RPM) 2":refnum<vi>, "Enter the Final Velocity (m/s) 3":refnum<vi>, "Enter initial Velocity (m/s)  3":refnum<vi>, "Ramp Up 2":refnum<vi>, "TEST SELECTION":refnum<vi>, "SPEED SELECTION : ":refnum<vi>, "Angular Oscillation Set":refnum<vi>, "Traction":refnum<vi>, "Step Speed":refnum<vi>, "StepTable For Load-Speed":refnum<vi>, "StepTable For Speed":refnum<vi>, "Surge Forward MM":refnum<vi>, "Surge Backward MM":refnum<vi>, "M3 Image":refnum<vi>, "String 39":refnum<vi>, "Sway Left MM":refnum<vi>, "Sway Right MM":refnum<vi>, "Disable Axis Jog Soft Limits":refnum<vi>, "mm":refnum<vi>, "Heave Down MM":refnum<vi>, "Heave Up MM":refnum<vi>, "Wear Track Diameter (mm)":refnum<vi>, "Set WTD":refnum<vi>, "HomeScratch":refnum<vi>, "HomeRot":refnum<vi>, "PlaceModule":refnum<vi>, "Enter the Angle (Deg)":refnum<vi>, "Enter the Frequency (Hz)":refnum<vi>, "Motion Mode:":refnum<vi>, "LR Sway":refnum<vi>, "Rot Hor":refnum<vi>, "Scratch":refnum<vi>, "LR Cam":refnum<vi>, "MMBack":refnum<vi>, "MMNext":refnum<vi>, "Rot Ver":refnum<vi>, "Rotary Module Selection":refnum<vi>, "calculate rotary":refnum<vi>, "SPEED SELECTION : rotary":refnum<vi>, "Import 2":refnum<vi>, "Save 2":refnum<vi>, "File Path :  2":refnum<vi>, "String 45":refnum<vi>, "StepTable For Speed 3":refnum<vi>, "Enter the Speed(mm/sec)":refnum<vi>, "Enter the Speed(RPM)":refnum<vi>, "Enter Scratch Speed (mm/s):":refnum<vi>, "SwaySpeed Set":refnum<vi>, "Scartch Offset":refnum<vi>, "Motion type:":refnum<vi>, "HomeScratch 2":refnum<vi>, "Enter Scratch length (mm):":refnum<vi>, "Wear Track Diameter":refnum<vi>, "Rotary Speed Exced":refnum<vi>, "Scratch Mode":refnum<vi>, "No of Scratch":refnum<vi>}, "Environmental control":cluster{"Humidity  Status  3":refnum<vi>, "Low Temp  Status  2":refnum<vi>, "TK4 status 2":refnum<vi>, "Stage Temperature":refnum<vi>, "Sample Temperature":refnum<vi>, "Humidity (Amb)":refnum<vi>, "Clear List":refnum<vi>, "Add to list":refnum<vi>, "Wear":refnum<vi>, "Vibration":refnum<vi>, "Humidity (Chamber)":refnum<vi>, "Temperature (Chamber)":refnum<vi>, "ECR ":refnum<vi>, "Temperature (Amb)":refnum<vi>, "Microphone":refnum<vi>, "Acoustic Emission 3":refnum<vi>, "SNext":refnum<vi>, "APBack":refnum<vi>, "Enter the Temperature (°C):":refnum<vi>, "Enter the Stage \nTemperature (°C):":refnum<vi>, "Enter the Humidity (%Rh):":refnum<vi>, "Low Temp":refnum<vi>, "High Temp":refnum<vi>, "Humidity":refnum<vi>, "Sensors Picked":refnum<vi>}, "About Screen":cluster{"Password":refnum<vi>, "Home Service":refnum<vi>, "Advanced Setting":refnum<vi>, "About Tab":refnum<vi>, "ECR Port:":refnum<vi>, "Ramp Port:":refnum<vi>, "Installation/Replacement completed":refnum<vi>, "Loahead":refnum<vi>, "Heave and Surge COM Port:":refnum<vi>, "Sway COM Port:":refnum<vi>, "Temp Modbus:":refnum<vi>, "Humidity Port:":refnum<vi>, "Edit Gain Constants":refnum<vi>, "Save Gain Constants":refnum<vi>}, "Main Screen":cluster{"Main Screen Tab":refnum<vi>, "Angle and Frequency":refnum<vi>, "Stroke (mm)":refnum<vi>, "Angle (Deg)":refnum<vi>, "Main Speed Tab":refnum<vi>, "MTM MOTOR DISPLAY":refnum<vi>, "Disc Speed (m/sec)":refnum<vi>, "Ball Speed (m/sec)":refnum<vi>, "Disc Speed (RPM)":refnum<vi>, "Ball Speed (RPM)":refnum<vi>, "SPEED TAB":refnum<vi>, "Speed (m/sec)":refnum<vi>, "Set Speed (m/sec)":refnum<vi>, "Speed (RPM)":refnum<vi>, "Set Speed":refnum<vi>, "Time Tab":refnum<vi>, "Time ( HH:MM:SS ) 2":refnum<vi>, "Test Duration":refnum<vi>, "Test Duration 4":refnum<vi>, "TEST CYCLE":refnum<vi>, "TOTAL CYCLES":refnum<vi>, "Set Load (N)":refnum<vi>, "Temp Tabs":refnum<vi>, "Heater":refnum<vi>, "TK4 status":refnum<vi>, "ChamberTemp":refnum<vi>, "SetTmp":refnum<vi>, "Controller  Status":refnum<vi>, "ChamberTemp 2":refnum<vi>, "SetTmp 2":refnum<vi>, "Controller  Status 2":refnum<vi>, "ChamberTemp 3":refnum<vi>, "SetTmp 3":refnum<vi>, "Cooling":refnum<vi>, "Load Communication":refnum<vi>, "Ambient \nTemperature":refnum<vi>, "HumCOMStatus":refnum<vi>, "Ambient\n Humidity":refnum<vi>, "Freq (Hz)":refnum<vi>, "Load En":refnum<vi>, "NLt":refnum<vi>, "zNL 2":refnum<vi>, "Humidity On":refnum<vi>, "humidity disp":refnum<vi>, "Set Humidity":refnum<vi>, "NL disp 2":refnum<vi>, "Humidity On 2":refnum<vi>, "humidity disp 2":refnum<vi>, "Set Humidity 2":refnum<vi>, "NL disp 3":refnum<vi>, "AppLoadSeq scratch":refnum<vi>, "Stop Scratch":refnum<vi>, "ClrLog":refnum<vi>, "Trip Log":refnum<vi>, "STOP":refnum<vi>, "Start Test":refnum<vi>, "Test status":refnum<vi>, "AR Led":refnum<vi>, "Data":refnum<vi>, "Health":refnum<vi>, "Sway COM Status":refnum<vi>, "Heave COM Status":refnum<vi>, "Grp Tab":refnum<vi>, "Sub Graph":refnum<vi>, "SD (mm)":refnum<vi>, "Siliding distance Reset Graph":refnum<vi>, "SDGp":refnum<vi>, "Humidity Reset Graph":refnum<vi>, "HumrGp":refnum<vi>, "Acoustic Emission (mV)":refnum<vi>, "Aqucostic Reset Graph":refnum<vi>, "gACQUOS":refnum<vi>, "ECR RESET":refnum<vi>, "ECR":refnum<vi>, "Temperature Reset":refnum<vi>, "Acoustic Emission (mV) 2":refnum<vi>, "Aqucostic Reset Graph 2":refnum<vi>, "gACQUOS 2":refnum<vi>, "ECR RESET 2":refnum<vi>, "ECR 2":refnum<vi>, "Temperature Reset 2":refnum<vi>, "Temperature (deg c)":refnum<vi>, "Speed Reset Graph":refnum<vi>, "Speed Tab":refnum<vi>, "MTM DISC  SPEED":refnum<vi>, "MTM BALL SPEED":refnum<vi>, "speed mm/sec":refnum<vi>, "Hymidity":refnum<vi>, "Humidity Disable trip":refnum<vi>, "CoF Trip  2":refnum<vi>, "Depth Trip":refnum<vi>, "Weart Deapth":refnum<vi>, "Depth Reset Graph":refnum<vi>, "Weart":refnum<vi>, "Depthz":refnum<vi>, "Depth (µm)":refnum<vi>, "WearGp":refnum<vi>, "NL Trip 2":refnum<vi>, "Load pid":refnum<vi>, "Load Disable Trip":refnum<vi>, "Load Reset Graph":refnum<vi>, "NL Display 4":refnum<vi>, "Main Chart 3":refnum<vi>, "BACK":refnum<vi>, "Depth Trip 2":refnum<vi>, "COF TRIP ":refnum<vi>, "Friction Force (N)":refnum<vi>, "FF Reset Graph":refnum<vi>, "FF Disable Trip":refnum<vi>, "FF TRIP":refnum<vi>, "COF Disable Trip":refnum<vi>, "COF Reset Graph":refnum<vi>, "Start Test Temp":refnum<vi>, "zFF":refnum<vi>, "Friction Force (N) Graph":refnum<vi>, "Coefficient of Friction":refnum<vi>, "Scratch Start Test":refnum<vi>, "FF Tab":refnum<vi>, "Cyclic Friction Force (N)":refnum<vi>, "CZ FF":refnum<vi>, "Cyclic Friction Force (N) Graph":refnum<vi>, "Cyclic Coefficient of Friction":refnum<vi>, "Cyclic FF TRIP":refnum<vi>, "Cyclic FF Disable Trip":refnum<vi>, "cyclic COF Disable Trip":refnum<vi>, "cyclic COF TRIP":refnum<vi>, "cyclic COF Reset Graph":refnum<vi>, "Cyclic FF Reset Graph":refnum<vi>, "Test Trip":refnum<vi>, "Multi Scratch Pass":refnum<vi>}, "Loading":cluster{"Indentation":refnum<vi>, "Reference Sample":refnum<vi>, "Load Cell Communication Slide":refnum<vi>, "com 3":refnum<vi>, "com":refnum<vi>, "DecaForce COM Status":refnum<vi>, "Update":refnum<vi>, "Clear 3":refnum<vi>, "seq":refnum<vi>, "Stribeck table":refnum<vi>, "Stribeck Table  For loading":refnum<vi>, "Loading Mode":refnum<vi>, "Enter the Final Load (N)":refnum<vi>, "Enter the CoF Trip":refnum<vi>, "Enter the Friction Force Trip":refnum<vi>, "Enter the Normal load Trip":refnum<vi>, "Enter the Load  (N)":refnum<vi>, "KiloForce":refnum<vi>, "DecaForce ":refnum<vi>, "MicroForce":refnum<vi>, "LHBack":refnum<vi>, "LHNext":refnum<vi>, "Enter the Loading Rate (N/min)":refnum<vi>, "Message":refnum<vi>, "Warning 2":refnum<vi>, "SSP 0.75":refnum<vi>, "SSP 0.5":refnum<vi>, "SSP 0.3":refnum<vi>, "Warning":refnum<vi>, "gui GIF":refnum<vi>, "Communication is established":refnum<vi>, "AppLoad 4":refnum<vi>, "Multipoint":refnum<vi>, "Load Selection":refnum<vi>}, "PID":cluster{"Ramp MulFac":refnum<vi>, "pulses LoadDiffRamp(2..10)":refnum<vi>, "PulseControlRamp(diff<=3N)":refnum<vi>, "SetLoadDeadband(%) Load(0-10N)":refnum<vi>, "PID gains out delay (microForce)":refnum<vi>, "Ramp":refnum<vi>, "Gain 2":refnum<vi>, "pulses LoadDiff(2..10)":refnum<vi>, "pulses LoadDiff(11..50)":refnum<vi>, "PulseControl(diff<=3N)":refnum<vi>, "SetLoadDeadband(%)  2":refnum<vi>, "Dummy Run":refnum<vi>, "Vertical load (N)":refnum<vi>, "AutoTune":refnum<vi>, "Offset 3 ":refnum<vi>, "apply load":refnum<vi>, "Offset  3":refnum<vi>, "apply load 2":refnum<vi>, "Enter ByPass Load":refnum<vi>, "reinit 3":refnum<vi>, "output range delay":refnum<vi>, "PID gains out delay":refnum<vi>, "Bypass Load":refnum<vi>, "pulsesSent":refnum<vi>, "pulses ":refnum<vi>, "actpid":refnum<vi>, "gFF Rot":refnum<vi>, "pulses LoadDiff(21..1000)":refnum<vi>, "Delay":refnum<vi>, "deadband":refnum<vi>}, "Config Parameters":cluster{"Tab Control 3":refnum<vi>, "Tab Control 19":refnum<vi>, "SAMPLES":refnum<vi>, "Re-initilaize":refnum<vi>, "Filter ON/OFF":refnum<vi>, "TracHomeSurgeOffsetCounts 10MM":refnum<vi>, "TracHomeSwayOffsetCounts 10MM":refnum<vi>, "Acoustic Emission:":refnum<vi>, "Apply Filter (FF)":refnum<vi>, "Filter% 2":refnum<vi>, "Apply Filter (Load)":refnum<vi>, "Filter% ":refnum<vi>, "Sway distance (mm)":refnum<vi>, "Surge distance (mm)":refnum<vi>, "DataSavingLoopDelay(ms)":refnum<vi>, "SAVE 2":refnum<vi>, "Enter Distance":refnum<vi>, "Sway Counts:":refnum<vi>, "Distance (mm): 3":refnum<vi>, "Surge Counts:":refnum<vi>, "Distance (mm): 2":refnum<vi>, "Distance (mm):":refnum<vi>, "Heave Counts:":refnum<vi>, "LRMHomeSurgeOffsetCounts":refnum<vi>, "LRMHomeSwayOffsetCounts":refnum<vi>, "TracHomeSurgeOffsetCounts 20MM":refnum<vi>, "TracHomeSwayOffsetCounts 20MM":refnum<vi>, "RotHomeSwayOffsetCounts":refnum<vi>, "RotHomeSurgeOffsetCounts":refnum<vi>, "Heave distance":refnum<vi>, "Zmm":refnum<vi>, "Heave Pulses/mm":refnum<vi>, "Surge Pulses/mm":refnum<vi>, "Sway Pulses/mm":refnum<vi>, "Heave Pitch":refnum<vi>, "Surge Pitch":refnum<vi>, "Sway Pitch":refnum<vi>, "Heave PPR":refnum<vi>, "Surge PPR":refnum<vi>, "Sway PPR":refnum<vi>, "Tab Control 5":refnum<vi>, "Tab Control 14":refnum<vi>, "Tab Control 26":refnum<vi>, "AE":refnum<vi>, "Heave Loop Delay":refnum<vi>, "Heave PID Speed":refnum<vi>, "Surge Jog Speed":refnum<vi>, "Heave Jog Speed":refnum<vi>, "Sway Loop Delay":refnum<vi>, "Sway PID Speed":refnum<vi>, "Sway Jog Speed":refnum<vi>}, "Loading Com Port":cluster{"ClearAll":refnum<vi>, "Mz(Nm)":refnum<vi>, "My(Nm)":refnum<vi>, "Mx(Nm)":refnum<vi>, "Save Dwell":refnum<vi>, "Mx ":refnum<vi>, "My ":refnum<vi>, "Mz":refnum<vi>, "Fx(N)":refnum<vi>, "Fy(N)":refnum<vi>, "Fz(N)":refnum<vi>, "ZeroAll":refnum<vi>, "Acq Delay (ms)":refnum<vi>, "Burst Delay (ms)":refnum<vi>, "model":refnum<vi>, "SN":refnum<vi>, "FFx(N)":refnum<vi>, "Sensor IP":refnum<vi>, "Port":refnum<vi>, "FFy(N)":refnum<vi>, "Load(N)":refnum<vi>, "delete Handle":refnum<vi>, "Create Handle":refnum<vi>, "ft_data":refnum<vi>, "ft_range":refnum<vi>, "ft_data 2":refnum<vi>, "stop 6":refnum<vi>, "running_flag":refnum<vi>, "ft_udp_handle":refnum<vi>, "get-data-return":refnum<vi>, "get-range-return":refnum<vi>, "zero-return":refnum<vi>, "filter-return":refnum<vi>, "initial-return":refnum<vi>, "deleteHandle-result":refnum<vi>, "Load Cell Temp":refnum<vi>}, "Heave AND Surge":cluster{"SURGE POSE":refnum<vi>, "error out Read":refnum<vi>, "HEAVE POSE":refnum<vi>, "State":refnum<vi>, "Homed":refnum<vi>, "Sequence ID":refnum<vi>, "error out Write":refnum<vi>, "faultCode":refnum<vi>, "Ack ID":refnum<vi>, "SPEED":refnum<vi>, "Distance":refnum<vi>, "Mode Command":refnum<vi>, "Heave and Surge Read":refnum<vi>, "Read Heave Temp":refnum<vi>, "Spare 15":refnum<vi>, "Spare 14":refnum<vi>, "Spare 13":refnum<vi>, "Spare 12":refnum<vi>, "Spare 11":refnum<vi>, "Spare 10":refnum<vi>, "Spare 9":refnum<vi>, "Spare 8":refnum<vi>, "Spare 7":refnum<vi>, "Spare 6":refnum<vi>, "Spare 5":refnum<vi>, "Spare 4":refnum<vi>, "Spare 2":refnum<vi>, "Spare 1":refnum<vi>, "Node Id":refnum<vi>, "Spare 3":refnum<vi>, "SPARE 4":refnum<vi>, "SPARE 3":refnum<vi>, "SPARE 2":refnum<vi>, "SPARE 1":refnum<vi>, "fwMajor":refnum<vi>, "fwMinor":refnum<vi>, "Manual Write":refnum<vi>, "Heave and Surge Write":refnum<vi>}, "New PID LOGIC":cluster{"Fine Tune Zone":refnum<vi>, "PID SDelay":refnum<vi>, "Max_pos_limit":refnum<vi>, "Min_pos_limit":refnum<vi>, "i_limit":refnum<vi>, "pct_scale":refnum<vi>, "Deadband":refnum<vi>, "Kd":refnum<vi>, "Ki":refnum<vi>, "Kp":refnum<vi>, "Current Position":refnum<vi>, "Set Load":refnum<vi>, "Current Load":refnum<vi>, "Pulse delta":refnum<vi>, "Init Step":refnum<vi>, "Max Step Linit":refnum<vi>}, "SWAY ":cluster{"fwMajor":refnum<vi>, "Homed":refnum<vi>, "Rotary POSE":refnum<vi>, "State":refnum<vi>, "SWAY POSE":refnum<vi>, "Ack ID":refnum<vi>, "faultCode":refnum<vi>, "Node Id":refnum<vi>, "fwMinor":refnum<vi>, "Spare 6":refnum<vi>, "Spare 5":refnum<vi>, "Spare 4":refnum<vi>, "Spare 3":refnum<vi>, "Spare 2":refnum<vi>, "Spare 1":refnum<vi>, "Spare 7":refnum<vi>, "SPARE  5":refnum<vi>, "error out Write  SWAY ":refnum<vi>, "error out Read SWAY ":refnum<vi>, "Manual Write SWAY ":refnum<vi>, "SWAY WRITE":refnum<vi>, "SPARE  4":refnum<vi>, "SPARE  3":refnum<vi>, "SPARE 2":refnum<vi>, "SPARE 1":refnum<vi>, "Spare 15":refnum<vi>, "Spare 14":refnum<vi>, "Spare 13":refnum<vi>, "Spare 12":refnum<vi>, "Spare 11":refnum<vi>, "Spare 9":refnum<vi>, "Spare 8":refnum<vi>, "SPEED":refnum<vi>, "Distance":refnum<vi>, "Mode Command":refnum<vi>, "Sequence ID":refnum<vi>, "SWAY READ":refnum<vi>, "Spare 10":refnum<vi>, "Read SWAY Temp":refnum<vi>}, "Analysis Screen":cluster{"Analysis Home":refnum<vi>, "Refresh 2":refnum<vi>, "MEAN 4":refnum<vi>, "SD 4":refnum<vi>, "VARIANCE 4":refnum<vi>, "MEAN  3":refnum<vi>, "SD  3":refnum<vi>, "VARIANCE  3":refnum<vi>, "MEAN 2":refnum<vi>, "SD  2":refnum<vi>, "VARIANCE 2":refnum<vi>, "MEAN":refnum<vi>, "SD":refnum<vi>, "VARIANCE":refnum<vi>, "File 4 Discription":refnum<vi>, "OPEN 4":refnum<vi>, "File Name 4":refnum<vi>, "OPEN 3":refnum<vi>, "File 3 Discription":refnum<vi>, "File Name 3":refnum<vi>, "Y-AXIS":refnum<vi>, "X-AXIS":refnum<vi>, "XY Graph":refnum<vi>, "File Name 2":refnum<vi>, "File Name 1":refnum<vi>, "OPEN 2":refnum<vi>, "OPEN 1":refnum<vi>, "File 1 Discription ":refnum<vi>, "File 2 Discription":refnum<vi>}}
  T12 = typedef "init queue out loop.ctl" = cluster{"UI Loop":refnum<queue>, "LOAD COM LOOP ":refnum<queue>, "SWAY MOTOR COM LOOP":refnum<queue>, "HEAVE MOTOR COM LOOP":refnum<queue>, "TEMPERATURE COM LOOP":refnum<queue>, "RAMP MOTOR COM LOOP":refnum<queue>, "ECR PORT":refnum<queue>, "HUMIDITY COM PORT":refnum<queue>, "PROGRAM LOOP":refnum<queue>, "MONITOR LOOP":refnum<queue>, "REPORT":refnum<queue>, "LOAD PID":refnum<queue>}
  T13 = enum8{"Enabled", "Disabled", "Disabled and Grayed Out"}
  T14 = enum16{"INIT", "SETLOWPASSFILTER", "SETZERO", "GETSENSORINFO", "GETRANGE", "ZEROALL", "READDATA", "UNINITIAL", "DELETEHANDLE"}
  T15 = typedef "Heave Write enum.ctl" = enum16{"INIT", "WRITE", "CLOSE", "REINIT"}
  T16 = typedef "Sway Write enum.ctl" = enum16{"INIT", "WRITE", "CLOSE", "REINIT"}
  T17 = typedef "Sway Right enum.ctl" = enum16{"INIT", "READ", "CLOSE", "REINIT", ""}
  T18 = typedef "Heave Right enum.ctl" = enum16{"INIT", "READ", "CLOSE", "REINIT", ""}
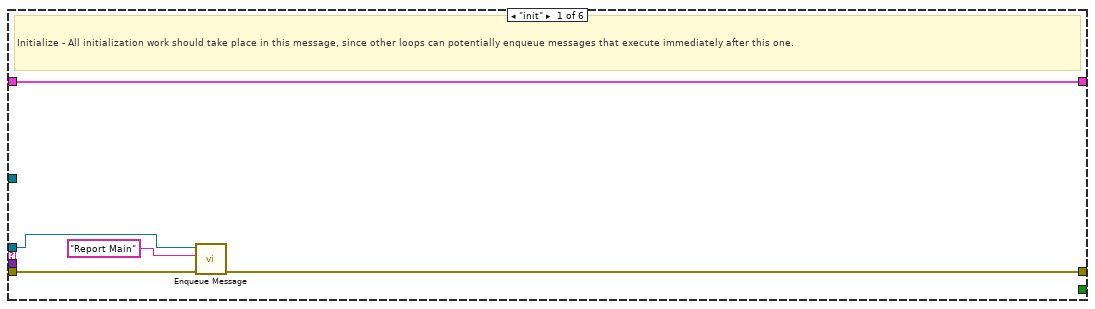
[diagram p2: hidden frame]
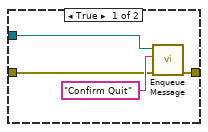
[diagram p3: hidden frame]
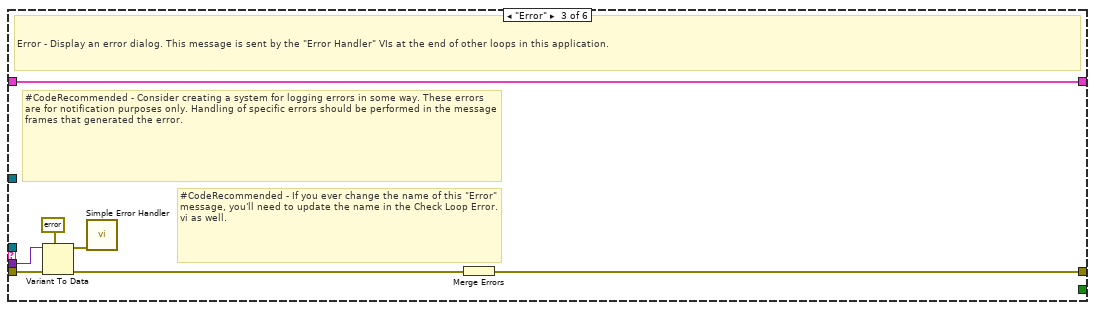
[diagram p4: hidden frame]
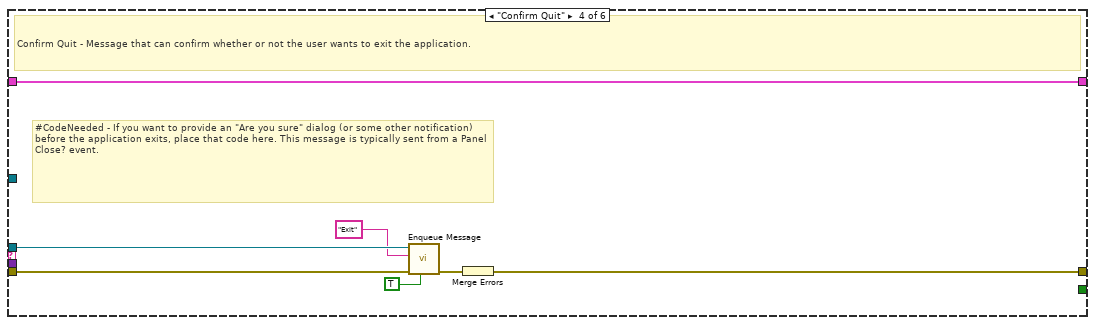
[diagram p5: hidden frame]
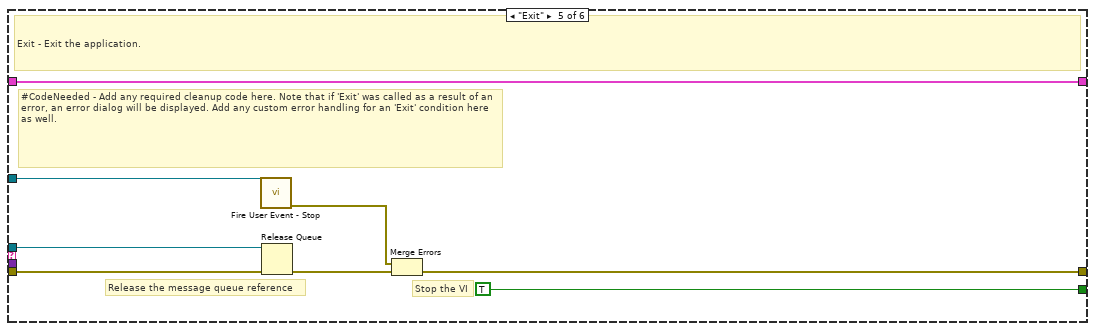
[diagram p6: hidden frame]
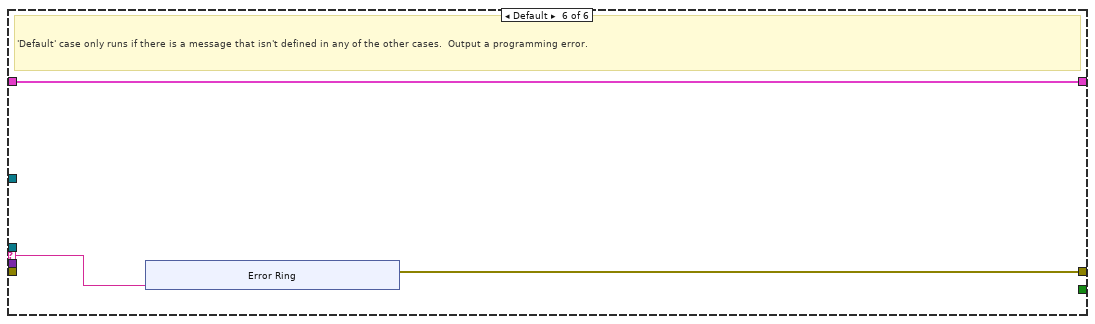
[diagram p7: hidden frame]
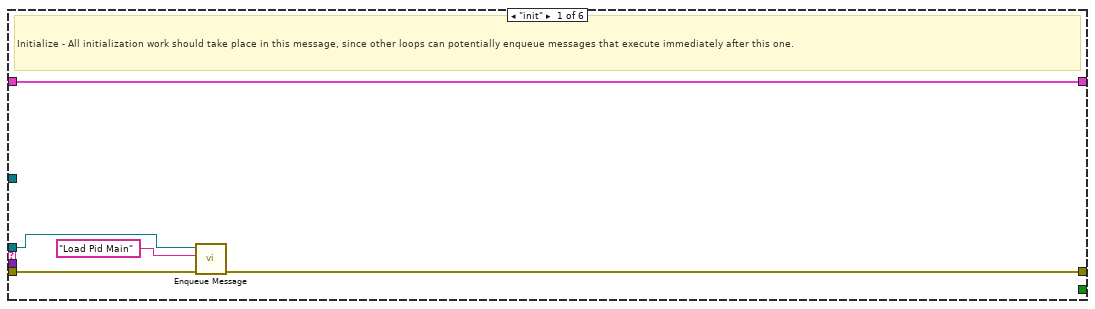
[diagram p8: hidden frame]
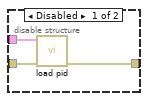
[diagram p10: hidden frame]
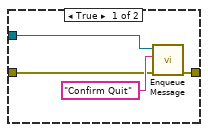
[diagram p11: hidden frame]
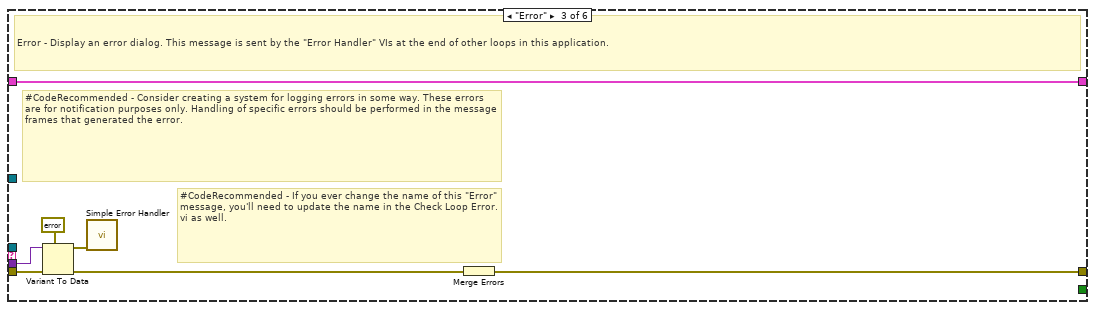
[diagram p12: hidden frame]
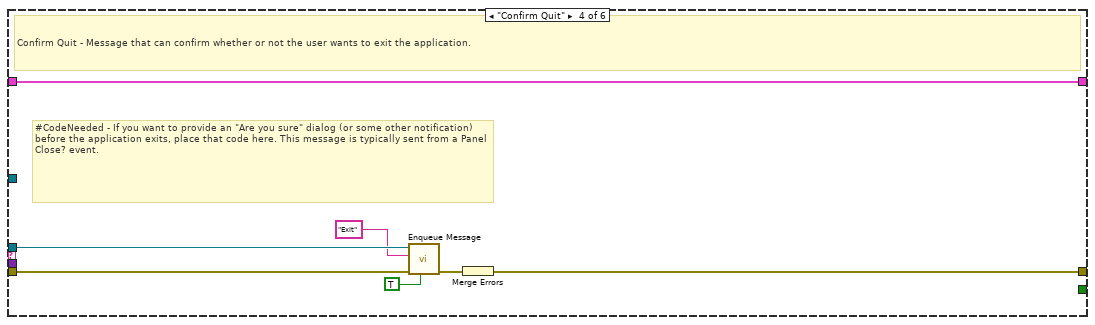
[diagram p13: hidden frame]
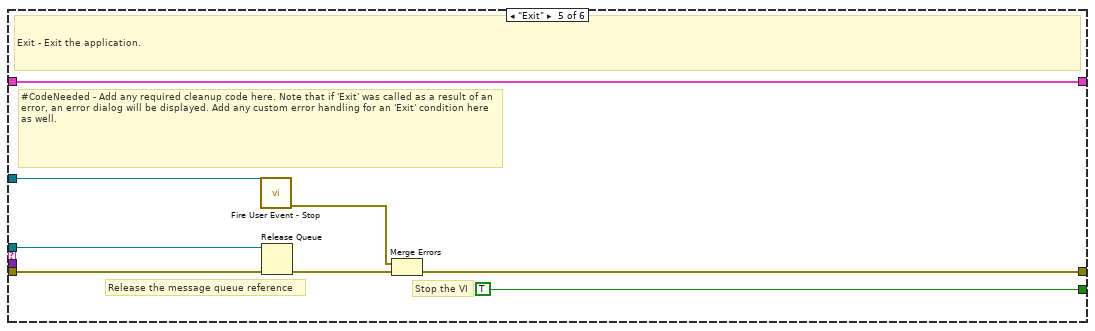
[diagram p14: hidden frame]
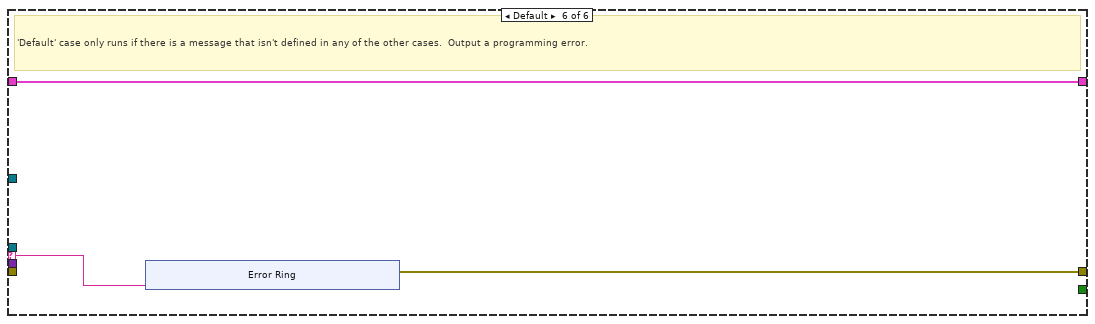
[diagram p15: hidden frame]
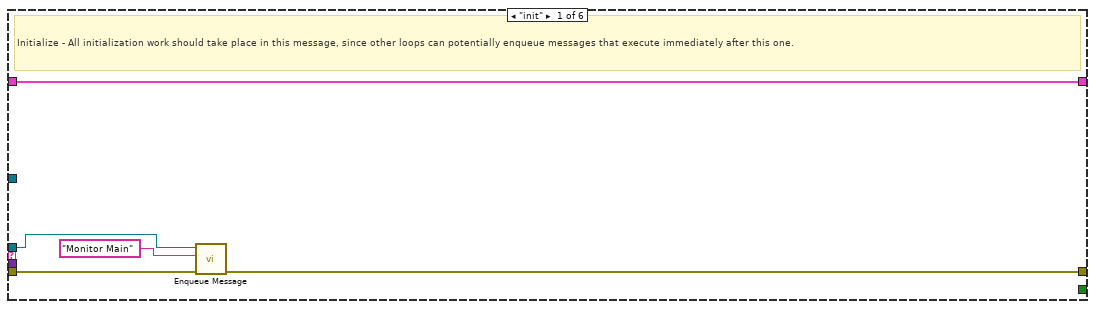
[diagram p16: hidden frame]
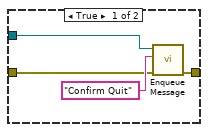
[diagram p17: hidden frame]
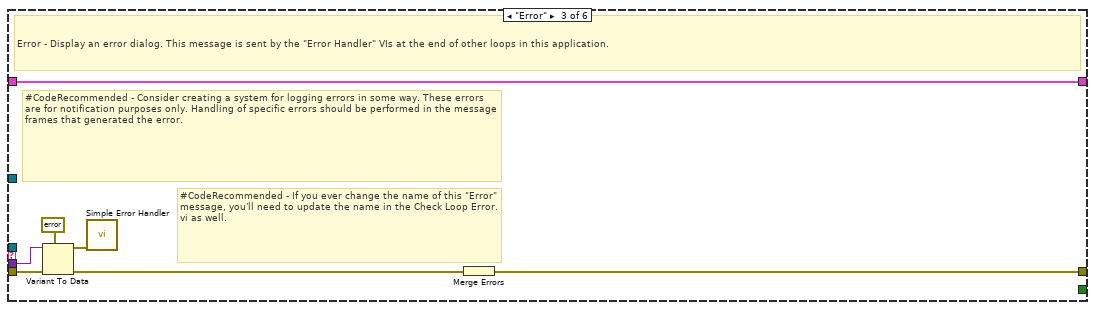
[diagram p18: hidden frame]
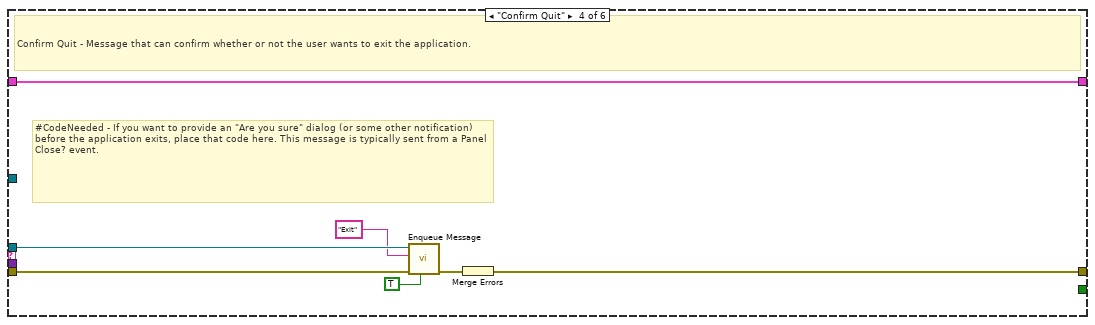
[diagram p19: hidden frame]
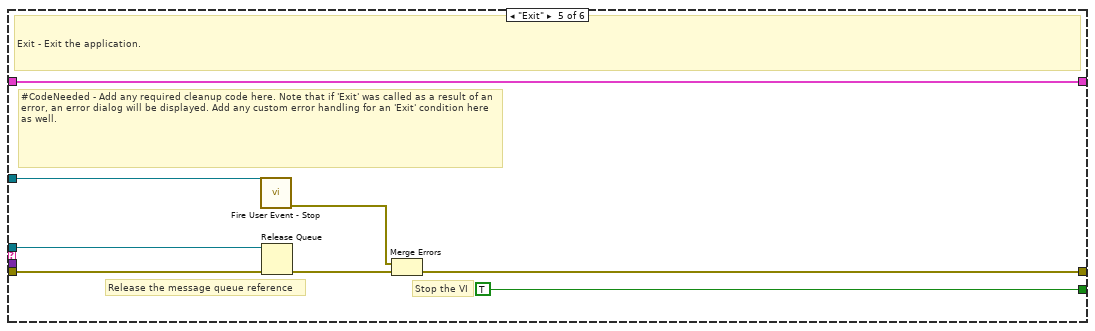
[diagram p20: hidden frame]
diagram:
  n1 = flat-sequence {
    tunnel: [w56] -> w43
    tunnel: T11 {"Main Home Screen"={"GUI"=refnum, "Platform Settings"=refnum, "Configure"=refnum, "Home"=refnum, "EXIT"=refnum, "service 2"=refnum, "MainPage"=refnum, "Analysis"=refnum}, "Platform Settings"={"mm/s  Surge"=refnum, "Update Surge Speed"=refnum, "Drive Error"=refnum, "Disable Axis Jog Soft Limits"=refnum, "mm/s  Sway"=refnum, "Sway and Surge COM Status"=refnum, "Heave COM Status"=refnum, "Enable Platform"=refnum, "Surge Forward Main"=refnum, "Sway Right Main"=refnum, "Sway Left Main"=refnum, "Heave Down Main"=refnum, "Heave Up main"=refnum, "Update Sway Speed"=refnum, "Update Heave Speed"=refnum, "mm/s Heave"=refnum, "mm/sec"=refnum, "mm"=refnum, "Surge Backward Main"=refnum}, "Analysis Screen"={"Analysis Home"=refnum, "Surface Analysis"=refnum, "Imaging"=refnum, "Image Analysis"=refnum, "Post Analysis"=refnum}, "Config Screen"={"Select Load Head"=refnum, "Notes :"=refnum, "FILE"=refnum, "Sample ID :"=refnum, "Operator ID :"=refnum, "Operator Name :"=refnum, "Auto"=refnum}, "Motion Module"={"zNL"=refnum, "NL disp"=refnum, "Rotary Tab"=refnum, "Motion Direction:  3"=refnum, "E.Velocity 2"=refnum, "e.v/ssr 2"=refnum, "Enter Fixed E.Velocity 2"=refnum, "Enter Final SRR 2"=refnum, "Enter initial SRR 2"=refnum, "Enter Fixed SRR 2"=refnum, "Enter the Final E.Velocity (m/s) 2"=refnum, "Enter initial E.Velocity (m/s) 2"=refnum, "Final Speed (RPM) 3"=refnum, "Initial Speed (RPM) 2"=refnum, "Enter the Final Velocity (m/s) 3"=refnum, "Enter initial Velocity (m/s)  3"=refnum, "Ramp Up 2"=refnum, "TEST SELECTION"=refnum, "SPEED SELECTION : "=refnum, "Angular Oscillation Set"=refnum, "Traction"=refnum, "Step Speed"=refnum, "StepTable For Load-Speed"=refnum, "StepTable For Speed"=refnum, "Surge Forward MM"=refnum, "Surge Backward MM"=refnum, "M3 Image"=refnum, "String 39"=refnum, "Sway Left MM"=refnum, "Sway Right MM"=refnum, "Disable Axis Jog Soft Limits"=refnum, "mm"=refnum, "Heave Down MM"=refnum, "Heave Up MM"=refnum, "Wear Track Diameter (mm)"=refnum, "Set WTD"=refnum, "HomeScratch"=refnum, "HomeRot"=refnum, "PlaceModule"=refnum, "Enter the Angle (Deg)"=refnum, "Enter the Frequency (Hz)"=refnum, "Motion Mode:"=refnum, "LR Sway"=refnum, "Rot Hor"=refnum, "Scratch"=refnum, "LR Cam"=refnum, "MMBack"=refnum, "MMNext"=refnum, "Rot Ver"=refnum, "Rotary Module Selection"=refnum, "calculate rotary"=refnum, "SPEED SELECTION : rotary"=refnum, "Import 2"=refnum, "Save 2"=refnum, "File Path :  2"=refnum, "String 45"=refnum, "StepTable For Speed 3"=refnum, "Enter the Speed(mm/sec)"=refnum, "Enter the Speed(RPM)"=refnum, "Enter Scratch Speed (mm/s):"=refnum, "SwaySpeed Set"=refnum, "Scartch Offset"=refnum, "Motion type:"=refnum, "HomeScratch 2"=refnum, "Enter Scratch length (mm):"=refnum, "Wear Track Diameter"=refnum, "Rotary Speed Exced"=refnum, "Scratch Mode"=refnum, "No of Scratch"=refnum}, "Environmental control"={"Humidity  Status  3"=refnum, "Low Temp  Status  2"=refnum, "TK4 status 2"=refnum, "Stage Temperature"=refnum, "Sample Temperature"=refnum, "Humidity (Amb)"=refnum, "Clear List"=refnum, "Add to list"=refnum, "Wear"=refnum, "Vibration"=refnum, "Humidity (Chamber)"=refnum, "Temperature (Chamber)"=refnum, "ECR "=refnum, "Temperature (Amb)"=refnum, "Microphone"=refnum, "Acoustic Emission 3"=refnum, "SNext"=refnum, "APBack"=refnum, "Enter the Temperature (°C):"=refnum, "Enter the Stage \nTemperature (°C):"=refnum, "Enter the Humidity (%Rh):"=refnum, "Low Temp"=refnum, "High Temp"=refnum, "Humidity"=refnum, "Sensors Picked"=refnum}, "About Screen"={"Password"=refnum, "Home Service"=refnum, "Advanced Setting"=refnum, "About Tab"=refnum, "ECR Port:"=refnum, "Ramp Port:"=refnum, "Installation/Replacement completed"=refnum, "Loahead"=refnum, "Heave and Surge COM Port:"=refnum, "Sway COM Port:"=refnum, "Temp Modbus:"=refnum, "Humidity Port:"=refnum, "Edit Gain Constants"=refnum, "Save Gain Constants"=refnum}, "Main Screen"={"Main Screen Tab"=refnum, "Angle and Frequency"=refnum, "Stroke (mm)"=refnum, "Angle (Deg)"=refnum, "Main Speed Tab"=refnum, "MTM MOTOR DISPLAY"=refnum, "Disc Speed (m/sec)"=refnum, "Ball Speed (m/sec)"=refnum, "Disc Speed (RPM)"=refnum, "Ball Speed (RPM)"=refnum, "SPEED TAB"=refnum, "Speed (m/sec)"=refnum, "Set Speed (m/sec)"=refnum, "Speed (RPM)"=refnum, "Set Speed"=refnum, "Time Tab"=refnum, "Time ( HH:MM:SS ) 2"=refnum, "Test Duration"=refnum, "Test Duration 4"=refnum, "TEST CYCLE"=refnum, "TOTAL CYCLES"=refnum, "Set Load (N)"=refnum, "Temp Tabs"=refnum, "Heater"=refnum, "TK4 status"=refnum, "ChamberTemp"=refnum, "SetTmp"=refnum, "Controller  Status"=refnum, "ChamberTemp 2"=refnum, "SetTmp 2"=refnum, "Controller  Status 2"=refnum, "ChamberTemp 3"=refnum, "SetTmp 3"=refnum, "Cooling"=refnum, "Load Communication"=refnum, "Ambient \nTemperature"=refnum, "HumCOMStatus"=refnum, "Ambient\n Humidity"=refnum, "Freq (Hz)"=refnum, "Load En"=refnum, "NLt"=refnum, "zNL 2"=refnum, "Humidity On"=refnum, "humidity disp"=refnum, "Set Humidity"=refnum, "NL disp 2"=refnum, "Humidity On 2"=refnum, "humidity disp 2"=refnum, "Set Humidity 2"=refnum, "NL disp 3"=refnum, "AppLoadSeq scratch"=refnum, "Stop Scratch"=refnum, "ClrLog"=refnum, "Trip Log"=refnum, "STOP"=refnum, "Start Test"=refnum, "Test status"=refnum, "AR Led"=refnum, "Data"=refnum, "Health"=refnum, "Sway COM Status"=refnum, "Heave COM Status"=refnum, "Grp Tab"=refnum, "Sub Graph"=refnum, "SD (mm)"=refnum, "Siliding distance Reset Graph"=refnum, "SDGp"=refnum, "Humidity Reset Graph"=refnum, "HumrGp"=refnum, "Acoustic Emission (mV)"=refnum, "Aqucostic Reset Graph"=refnum, "gACQUOS"=refnum, "ECR RESET"=refnum, "ECR"=refnum, "Temperature Reset"=refnum, "Acoustic Emission (mV) 2"=refnum, "Aqucostic Reset Graph 2"=refnum, "gACQUOS 2"=refnum, "ECR RESET 2"=refnum, "ECR 2"=refnum, "Temperature Reset 2"=refnum, "Temperature (deg c)"=refnum, "Speed Reset Graph"=refnum, "Speed Tab"=refnum, "MTM DISC  SPEED"=refnum, "MTM BALL SPEED"=refnum, "speed mm/sec"=refnum, "Hymidity"=refnum, "Humidity Disable trip"=refnum, "CoF Trip  2"=refnum, "Depth Trip"=refnum, "Weart Deapth"=refnum, "Depth Reset Graph"=refnum, "Weart"=refnum, "Depthz"=refnum, "Depth (µm)"=refnum, "WearGp"=refnum, "NL Trip 2"=refnum, "Load pid"=refnum, "Load Disable Trip"=refnum, "Load Reset Graph"=refnum, "NL Display 4"=refnum, "Main Chart 3"=refnum, "BACK"=refnum, "Depth Trip 2"=refnum, "COF TRIP "=refnum, "Friction Force (N)"=refnum, "FF Reset Graph"=refnum, "FF Disable Trip"=refnum, "FF TRIP"=refnum, "COF Disable Trip"=refnum, "COF Reset Graph"=refnum, "Start Test Temp"=refnum, "zFF"=refnum, "Friction Force (N) Graph"=refnum, "Coefficient of Friction"=refnum, "Scratch Start Test"=refnum, "FF Tab"=refnum, "Cyclic Friction Force (N)"=refnum, "CZ FF"=refnum, "Cyclic Friction Force (N) Graph"=refnum, "Cyclic Coefficient of Friction"=refnum, "Cyclic FF TRIP"=refnum, "Cyclic FF Disable Trip"=refnum, "cyclic COF Disable Trip"=refnum, "cyclic COF TRIP"=refnum, "cyclic COF Reset Graph"=refnum, "Cyclic FF Reset Graph"=refnum, "Test Trip"=refnum, "Multi Scratch Pass"=refnum}, "Loading"={"Indentation"=refnum, "Reference Sample"=refnum, "Load Cell Communication Slide"=refnum, "com 3"=refnum, "com"=refnum, "DecaForce COM Status"=refnum, "Update"=refnum, "Clear 3"=refnum, "seq"=refnum, "Stribeck table"=refnum, "Stribeck Table  For loading"=refnum, "Loading Mode"=refnum, "Enter the Final Load (N)"=refnum, "Enter the CoF Trip"=refnum, "Enter the Friction Force Trip"=refnum, "Enter the Normal load Trip"=refnum, "Enter the Load  (N)"=refnum, "KiloForce"=refnum, "DecaForce "=refnum, "MicroForce"=refnum, "LHBack"=refnum, "LHNext"=refnum, "Enter the Loading Rate (N/min)"=refnum, "Message"=refnum, "Warning 2"=refnum, "SSP 0.75"=refnum, "SSP 0.5"=refnum, "SSP 0.3"=refnum, "Warning"=refnum, "gui GIF"=refnum, "Communication is established"=refnum, "AppLoad 4"=refnum, "Multipoint"=refnum, "Load Selection"=refnum}, "PID"={"Ramp MulFac"=refnum, "pulses LoadDiffRamp(2..10)"=refnum, "PulseControlRamp(diff<=3N)"=refnum, "SetLoadDeadband(%) Load(0-10N)"=refnum, "PID gains out delay (microForce)"=refnum, "Ramp"=refnum, "Gain 2"=refnum, "pulses LoadDiff(2..10)"=refnum, "pulses LoadDiff(11..50)"=refnum, "PulseControl(diff<=3N)"=refnum, "SetLoadDeadband(%)  2"=refnum, "Dummy Run"=refnum, "Vertical load (N)"=refnum, "AutoTune"=refnum, "Offset 3 "=refnum, "apply load"=refnum, "Offset  3"=refnum, "apply load 2"=refnum, "Enter ByPass Load"=refnum, "reinit 3"=refnum, "output range delay"=refnum, "PID gains out delay"=refnum, "Bypass Load"=refnum, "pulsesSent"=refnum, "pulses "=refnum, "actpid"=refnum, "gFF Rot"=refnum, "pulses LoadDiff(21..1000)"=refnum, "Delay"=refnum, "deadband"=refnum}, "Config Parameters"={"Tab Control 3"=refnum, "Tab Control 19"=refnum, "SAMPLES"=refnum, "Re-initilaize"=refnum, "Filter ON/OFF"=refnum, "TracHomeSurgeOffsetCounts 10MM"=refnum, "TracHomeSwayOffsetCounts 10MM"=refnum, "Acoustic Emission:"=refnum, "Apply Filter (FF)"=refnum, "Filter% 2"=refnum, "Apply Filter (Load)"=refnum, "Filter% "=refnum, "Sway distance (mm)"=refnum, "Surge distance (mm)"=refnum, "DataSavingLoopDelay(ms)"=refnum, "SAVE 2"=refnum, "Enter Distance"=refnum, "Sway Counts:"=refnum, "Distance (mm): 3"=refnum, "Surge Counts:"=refnum, "Distance (mm): 2"=refnum, "Distance (mm):"=refnum, "Heave Counts:"=refnum, "LRMHomeSurgeOffsetCounts"=refnum, "LRMHomeSwayOffsetCounts"=refnum, "TracHomeSurgeOffsetCounts 20MM"=refnum, "TracHomeSwayOffsetCounts 20MM"=refnum, "RotHomeSwayOffsetCounts"=refnum, "RotHomeSurgeOffsetCounts"=refnum, "Heave distance"=refnum, "Zmm"=refnum, "Heave Pulses/mm"=refnum, "Surge Pulses/mm"=refnum, "Sway Pulses/mm"=refnum, "Heave Pitch"=refnum, "Surge Pitch"=refnum, "Sway Pitch"=refnum, "Heave PPR"=refnum, "Surge PPR"=refnum, "Sway PPR"=refnum, "Tab Control 5"=refnum, "Tab Control 14"=refnum, "Tab Control 26"=refnum, "AE"=refnum, "Heave Loop Delay"=refnum, "Heave PID Speed"=refnum, "Surge Jog Speed"=refnum, "Heave Jog Speed"=refnum, "Sway Loop Delay"=refnum, "Sway PID Speed"=refnum, "Sway Jog Speed"=refnum}, "Loading Com Port"={"ClearAll"=refnum, "Mz(Nm)"=refnum, "My(Nm)"=refnum, "Mx(Nm)"=refnum, "Save Dwell"=refnum, "Mx "=refnum, "My "=refnum, "Mz"=refnum, "Fx(N)"=refnum, "Fy(N)"=refnum, "Fz(N)"=refnum, "ZeroAll"=refnum, "Acq Delay (ms)"=refnum, "Burst Delay (ms)"=refnum, "model"=refnum, "SN"=refnum, "FFx(N)"=refnum, "Sensor IP"=refnum, "Port"=refnum, "FFy(N)"=refnum, "Load(N)"=refnum, "delete Handle"=refnum, "Create Handle"=refnum, "ft_data"=refnum, "ft_range"=refnum, "ft_data 2"=refnum, "stop 6"=refnum, "running_flag"=refnum, "ft_udp_handle"=refnum, "get-data-return"=refnum, "get-range-return"=refnum, "zero-return"=refnum, "filter-return"=refnum, "initial-return"=refnum, "deleteHandle-result"=refnum, "Load Cell Temp"=refnum}, "Heave AND Surge"={"SURGE POSE"=refnum, "error out Read"=refnum, "HEAVE POSE"=refnum, "State"=refnum, "Homed"=refnum, "Sequence ID"=refnum, "error out Write"=refnum, "faultCode"=refnum, "Ack ID"=refnum, "SPEED"=refnum, "Distance"=refnum, "Mode Command"=refnum, "Heave and Surge Read"=refnum, "Read Heave Temp"=refnum, "Spare 15"=refnum, "Spare 14"=refnum, "Spare 13"=refnum, "Spare 12"=refnum, "Spare 11"=refnum, "Spare 10"=refnum, "Spare 9"=refnum, "Spare 8"=refnum, "Spare 7"=refnum, "Spare 6"=refnum, "Spare 5"=refnum, "Spare 4"=refnum, "Spare 2"=refnum, "Spare 1"=refnum, "Node Id"=refnum, "Spare 3"=refnum, "SPARE 4"=refnum, "SPARE 3"=refnum, "SPARE 2"=refnum, "SPARE 1"=refnum, "fwMajor"=refnum, "fwMinor"=refnum, "Manual Write"=refnum, "Heave and Surge Write"=refnum}, "New PID LOGIC"={"Fine Tune Zone"=refnum, "PID SDelay"=refnum, "Max_pos_limit"=refnum, "Min_pos_limit"=refnum, "i_limit"=refnum, "pct_scale"=refnum, "Deadband"=refnum, "Kd"=refnum, "Ki"=refnum, "Kp"=refnum, "Current Position"=refnum, "Set Load"=refnum, "Current Load"=refnum, "Pulse delta"=refnum, "Init Step"=refnum, "Max Step Linit"=refnum}, "SWAY "={"fwMajor"=refnum, "Homed"=refnum, "Rotary POSE"=refnum, "State"=refnum, "SWAY POSE"=refnum, "Ack ID"=refnum, "faultCode"=refnum, "Node Id"=refnum, "fwMinor"=refnum, "Spare 6"=refnum, "Spare 5"=refnum, "Spare 4"=refnum, "Spare 3"=refnum, "Spare 2"=refnum, "Spare 1"=refnum, "Spare 7"=refnum, "SPARE  5"=refnum, "error out Write  SWAY "=refnum, "error out Read SWAY "=refnum, "Manual Write SWAY "=refnum, "SWAY WRITE"=refnum, "SPARE  4"=refnum, "SPARE  3"=refnum, "SPARE 2"=refnum, "SPARE 1"=refnum, "Spare 15"=refnum, "Spare 14"=refnum, "Spare 13"=refnum, "Spare 12"=refnum, "Spare 11"=refnum, "Spare 9"=refnum, "Spare 8"=refnum, "SPEED"=refnum, "Distance"=refnum, "Mode Command"=refnum, "Sequence ID"=refnum, "SWAY READ"=refnum, "Spare 10"=refnum, "Read SWAY Temp"=refnum}, "Analysis Screen"={"Analysis Home"=refnum, "Refresh 2"=refnum, "MEAN 4"=refnum, "SD 4"=refnum, "VARIANCE 4"=refnum, "MEAN  3"=refnum, "SD  3"=refnum, "VARIANCE  3"=refnum, "MEAN 2"=refnum, "SD  2"=refnum, "VARIANCE 2"=refnum, "MEAN"=refnum, "SD"=refnum, "VARIANCE"=refnum, "File 4 Discription"=refnum, "OPEN 4"=refnum, "File Name 4"=refnum, "OPEN 3"=refnum, "File 3 Discription"=refnum, "File Name 3"=refnum, "Y-AXIS"=refnum, "X-AXIS"=refnum, "XY Graph"=refnum, "File Name 2"=refnum, "File Name 1"=refnum, "OPEN 2"=refnum, "OPEN 1"=refnum, "File 1 Discription "=refnum, "File 2 Discription"=refnum}} ("Data Cluster") -> [w55]
    tunnel: w43 -> [w85]
    tunnel: [w65] -> w42
    tunnel: w42 -> [w92]
    tunnel: [w86] -> w41
    tunnel: w41 -> [w101]
    tunnel: [w100] -> w40
    tunnel: w40 -> [w137]
    tunnel: [w136] -> w38
    tunnel: w38 -> [w208]
    tunnel: [w207] -> w37
    tunnel: w37 -> [w235]
    tunnel: [w234] -> w36
    tunnel: w36 -> [w251]
    tunnel: [w250] -> w35
    tunnel: w35 -> [w370]
    tunnel: [w369] -> w10
    tunnel: w10 -> [w400]
    tunnel: [w399] -> w9
    tunnel: w9 -> [w453]
    tunnel: [w452] -> w8
    tunnel: w8 -> [w490]
    tunnel: [w489] -> w7
    tunnel: w7 -> [w530]
    tunnel: [w529] -> w4
    tunnel: w4 -> [w548]
    tunnel: [w547] -> w3
    tunnel: w3 -> [w589]
    tunnel: [w588] -> w1
    tunnel: [w619] -> w15
    tunnel: w1 -> [w620]
    frame #0 {
      n2 = control-ref of="GUI"() -> (w64:refnum<vi>)
      n3 = control-ref of="MainPage"() -> (w58:refnum<vi>)
      n4 = control-ref of="Platform Settings"() -> (w63:refnum<vi>)
      n5 = control-ref of="Configure"() -> (w62:refnum<vi>)
      n6 = control-ref of="Home"() -> (w61:refnum<vi>)
      n7 = control-ref of="EXIT"() -> (w60:refnum<vi>)
      n8 = control-ref of="service 2"() -> (w59:refnum<vi>)
      n9 = control-ref of="Analysis"() -> (w57:refnum<vi>)
      n10 = Bundle By Name(cluster=w55, "Main Home Screen.GUI"=w64, "Main Home Screen.Platform Settings"=w63, "Main Home Screen.Configure"=w62, "Main Home Screen.Home"=w61, "Main Home Screen.EXIT"=w60, "Main Home Screen.service 2"=w59, "Main Home Screen.MainPage"=w58, "Main Home Screen.Analysis"=w57) -> (w56:T11)
    }
    frame #1 {
      n11 = control-ref of="Sway Right Main"() -> (w75:refnum<vi>)
      n12 = control-ref of="Sway Left Main"() -> (w74:refnum<vi>)
      n13 = control-ref of="Heave Down Main"() -> (w73:refnum<vi>)
      n14 = control-ref of="Heave Up main"() -> (w72:refnum<vi>)
      n15 = control-ref of="Update Sway Speed"() -> (w71:refnum<vi>)
      n16 = control-ref of="Update Heave Speed"() -> (w70:refnum<vi>)
      n17 = control-ref of="Surge Backward Main"() -> (w66:refnum<vi>)
      n18 = control-ref of="Update Surge Speed"() -> (w83:refnum<vi>)
      n19 = control-ref of="Disable Axis Jog Soft Limits m"() -> (w81:refnum<vi>)
      n20 = control-ref of="Sway and Surge COM Status"() -> (w79:refnum<vi>)
      n21 = control-ref of="Heave COM Status"() -> (w78:refnum<vi>)
      n22 = control-ref of="Enable Platform"() -> (w77:refnum<vi>)
      n23 = control-ref of="Surge Forward Main"() -> (w76:refnum<vi>)
      n24 = control-ref of="mm/s Heave"() -> (w69:refnum<vi>)
      n25 = control-ref of="mm/sec"() -> (w68:refnum<vi>)
      n26 = control-ref of="mm"() -> (w67:refnum<vi>)
      n27 = control-ref of="mm/s  Surge"() -> (w84:refnum<vi>)
      n28 = control-ref of="mm/s  Sway"() -> (w80:refnum<vi>)
      n29 = control-ref of="Drive Error"() -> (w82:refnum<vi>)
      n30 = Bundle By Name(cluster=w85, "Platform Settings.mm/s  Surge"=w84, "Platform Settings.Update Surge Speed"=w83, "Platform Settings.Drive Error"=w82, "Platform Settings.Disable Axis Jog Soft Limits"=w81, "Platform Settings.mm/s  Sway"=w80, "Platform Settings.Sway and Surge COM Status"=w79, "Platform Settings.Heave COM Status"=w78, "Platform Settings.Enable Platform"=w77, "Platform Settings.Surge Forward Main"=w76, "Platform Settings.Sway Right Main"=w75, "Platform Settings.Sway Left Main"=w74, "Platform Settings.Heave Down Main"=w73, "Platform Settings.Heave Up main"=w72, "Platform Settings.Update Sway Speed"=w71, "Platform Settings.Update Heave Speed"=w70, "Platform Settings.mm/s Heave"=w69, "Platform Settings.mm/sec"=w68, "Platform Settings.mm"=w67, "Platform Settings.Surge Backward Main"=w66) -> (w65:T11)
    }
    frame #2 {
      n31 = control-ref of="Analysis Home"() -> (w91:refnum<vi>)
      n32 = control-ref of="Surface Analysis"() -> (w90:refnum<vi>)
      n33 = control-ref of="Imaging"() -> (w89:refnum<vi>)
      n34 = control-ref of="Image Analysis"() -> (w88:refnum<vi>)
      n35 = control-ref of="Post Analysis"() -> (w87:refnum<vi>)
      n36 = Bundle By Name(cluster=w92, "Analysis Screen.Analysis Home"=w91, "Analysis Screen.Surface Analysis"=w90, "Analysis Screen.Imaging"=w89, "Analysis Screen.Image Analysis"=w88, "Analysis Screen.Post Analysis"=w87) -> (w86:T11)
    }
    frame #3 {
      n37 = control-ref of="Select Load Head"() -> (w99:refnum<vi>)
      n38 = control-ref of="Auto"() -> (w93:refnum<vi>)
      n39 = control-ref of="Notes :"() -> (w98:refnum<vi>)
      n40 = control-ref of="FILE"() -> (w97:refnum<vi>)
      n41 = control-ref of="Sample ID :"() -> (w96:refnum<vi>)
      n42 = control-ref of="Operator ID :"() -> (w95:refnum<vi>)
      n43 = control-ref of="Operator Name :"() -> (w94:refnum<vi>)
      n44 = Bundle By Name(cluster=w101, "Config Screen.Select Load Head"=w99, "Config Screen.Notes :"=w98, "Config Screen.FILE"=w97, "Config Screen.Sample ID :"=w96, "Config Screen.Operator ID :"=w95, "Config Screen.Operator Name :"=w94, "Config Screen.Auto"=w93) -> (w100:T11)
    }
    frame #4 {
      n45 = control-ref of="Warning"() -> (w129:refnum<vi>)
      n46 = control-ref of="gui GIF"() -> (w128:refnum<vi>)
      n47 = control-ref of="Load Selection"() -> (w102:refnum<vi>)
      n48 = control-ref of="Warning 2"() -> (w133:refnum<vi>)
      n49 = control-ref of="SSP 0.75"() -> (w132:refnum<vi>)
      n50 = control-ref of="SSP 0.5"() -> (w131:refnum<vi>)
      n51 = control-ref of="SSP 0.3"() -> (w130:refnum<vi>)
      n52 = control-ref of="Communication is established"() -> (w127:refnum<vi>)
      n53 = control-ref of="AppLoad 4"() -> (w126:refnum<vi>)
      n54 = control-ref of="Multipoint"() -> (w125:refnum<vi>)
      n55 = control-ref of="com 3"() -> (w121:refnum<vi>)
      n56 = control-ref of="com"() -> (w120:refnum<vi>)
      n57 = control-ref of="DecaForce COM Status"() -> (w119:refnum<vi>)
      n58 = control-ref of="Update"() -> (w118:refnum<vi>)
      n59 = control-ref of="Clear 3"() -> (w117:refnum<vi>)
      n60 = control-ref of="seq"() -> (w116:refnum<vi>)
      n61 = control-ref of="Stribeck table"() -> (w115:refnum<vi>)
      n62 = control-ref of="KiloForce"() -> (w107:refnum<vi>)
      n63 = control-ref of="DecaForce"() -> (w106:refnum<vi>)
      n64 = control-ref of="MicroForce"() -> (w105:refnum<vi>)
      n65 = control-ref of="LHBack"() -> (w104:refnum<vi>)
      n66 = control-ref of="LHNext"() -> (w103:refnum<vi>)
      n67 = control-ref of="Enter the Loading Rate (N/min)"() -> (w135:refnum<vi>)
      n68 = control-ref of="Enter the Final Load (N)"() -> (w112:refnum<vi>)
      n69 = control-ref of="Enter the CoF Trip"() -> (w111:refnum<vi>)
      n70 = control-ref of="Enter the Friction Force Trip"() -> (w110:refnum<vi>)
      n71 = control-ref of="Enter the Normal load Trip"() -> (w109:refnum<vi>)
      n72 = control-ref of="Enter the Load  (N)"() -> (w108:refnum<vi>)
      n73 = control-ref of="Message"() -> (w134:refnum<vi>)
      n74 = control-ref of="Indentation"() -> (w124:refnum<vi>)
      n75 = control-ref of="Stribeck Table  For loading"() -> (w114:refnum<vi>)
      n76 = control-ref of="Reference Sample"() -> (w123:refnum<vi>)
      n77 = control-ref of="Load Cell Communication Slide"() -> (w122:refnum<vi>)
      n78 = control-ref of="Loading Mode"() -> (w113:refnum<vi>)
      n79 = Bundle By Name(cluster=w137, "Loading.Enter the Loading Rate (N/min)"=w135, "Loading.Message"=w134, "Loading.Warning 2"=w133, "Loading.SSP 0.75"=w132, "Loading.SSP 0.5"=w131, "Loading.SSP 0.3"=w130, "Loading.Warning"=w129, "Loading.gui GIF"=w128, "Loading.Communication is established"=w127, "Loading.AppLoad 4"=w126, "Loading.Multipoint"=w125, "Loading.Indentation"=w124, "Loading.Reference Sample"=w123, "Loading.Load Cell Communication Slide"=w122, "Loading.com 3"=w121, "Loading.com"=w120, "Loading.DecaForce COM Status"=w119, "Loading.Update"=w118, "Loading.Clear 3"=w117, "Loading.seq"=w116, "Loading.Stribeck table"=w115, "Loading.Stribeck Table  For loading"=w114, "Loading.Loading Mode"=w113, "Loading.Enter the Final Load (N)"=w112, "Loading.Enter the CoF Trip"=w111, "Loading.Enter the Friction Force Trip"=w110, "Loading.Enter the Normal load Trip"=w109, "Loading.Enter the Load  (N)"=w108, "Loading.KiloForce"=w107, "Loading.DecaForce"=w106, "Loading.MicroForce"=w105, "Loading.LHBack"=w104, "Loading.LHNext"=w103, "Loading.Load Selection"=w102) -> (w136:T11)
    }
    frame #5 {
      n80 = control-ref of="TEST SELECTION"() -> (w189:refnum<vi>)
      n81 = control-ref of="SPEED SELECTION :"() -> (w188:refnum<vi>)
      n82 = control-ref of="SPEED SELECTION : rotary"() -> (w155:refnum<vi>)
      n83 = control-ref of="Rotary Tab"() -> (w204:refnum<vi>)
      n84 = control-ref of="e.v/ssr 2"() -> (w201:refnum<vi>)
      n85 = control-ref of="Step Speed"() -> (w185:refnum<vi>)
      n86 = control-ref of="M3 Image"() -> (w180:refnum<vi>)
      n87 = control-ref of="Rotary Module Selection"() -> (w157:refnum<vi>)
      n88 = control-ref of="zNL"() -> (w206:refnum<vi>)
      n89 = control-ref of="E.Velocity 2"() -> (w202:refnum<vi>)
      n90 = control-ref of="Ramp Up 2"() -> (w190:refnum<vi>)
      n91 = control-ref of="Angular Oscillation Set"() -> (w187:refnum<vi>)
      n92 = control-ref of="Traction"() -> (w186:refnum<vi>)
      n93 = control-ref of="Surge Forward MM"() -> (w182:refnum<vi>)
      n94 = control-ref of="Surge Backward MM"() -> (w181:refnum<vi>)
      n95 = control-ref of="Sway Left MM"() -> (w178:refnum<vi>)
      n96 = control-ref of="Sway Right MM"() -> (w177:refnum<vi>)
      n97 = control-ref of="Disable Axis Jog Soft Limits"() -> (w176:refnum<vi>)
      n98 = control-ref of="Heave Down MM"() -> (w174:refnum<vi>)
      n99 = control-ref of="Heave Up MM"() -> (w173:refnum<vi>)
      n100 = control-ref of="Set WTD"() -> (w171:refnum<vi>)
      n101 = control-ref of="HomeScratch"() -> (w170:refnum<vi>)
      n102 = control-ref of="HomeRot"() -> (w169:refnum<vi>)
      n103 = control-ref of="PlaceModule"() -> (w168:refnum<vi>)
      n104 = control-ref of="LR Sway"() -> (w164:refnum<vi>)
      n105 = control-ref of="Rot Hor"() -> (w163:refnum<vi>)
      n106 = control-ref of="Scratch"() -> (w162:refnum<vi>)
      n107 = control-ref of="LR Cam"() -> (w161:refnum<vi>)
      n108 = control-ref of="MMBack"() -> (w160:refnum<vi>)
      n109 = control-ref of="MMNext"() -> (w159:refnum<vi>)
      n110 = control-ref of="Rot Ver"() -> (w158:refnum<vi>)
      n111 = control-ref of="calculate rotary"() -> (w156:refnum<vi>)
      n112 = control-ref of="Import 2"() -> (w154:refnum<vi>)
      n113 = control-ref of="Save 2"() -> (w153:refnum<vi>)
      n114 = control-ref of="SwaySpeed Set"() -> (w146:refnum<vi>)
      n115 = control-ref of="HomeScratch"() -> (w142:refnum<vi>)
      n116 = control-ref of="NL disp"() -> (w205:refnum<vi>)
      n117 = control-ref of="Enter Fixed E.Velocity 2"() -> (w200:refnum<vi>)
      n118 = control-ref of="Enter Final SRR 2"() -> (w199:refnum<vi>)
      n119 = control-ref of="Enter initial SRR 2"() -> (w198:refnum<vi>)
      n120 = control-ref of="Enter Fixed SRR 2"() -> (w197:refnum<vi>)
      n121 = control-ref of="Enter the Final E.Velocity (m/s) 2"() -> (w196:refnum<vi>)
      n122 = control-ref of="Enter initial E.Velocity (m/s) 2"() -> (w195:refnum<vi>)
      n123 = control-ref of="Final Speed (RPM) 3"() -> (w194:refnum<vi>)
      n124 = control-ref of="Initial Speed (RPM) 2"() -> (w193:refnum<vi>)
      n125 = control-ref of="Enter the Final Velocity (m/s) 3"() -> (w192:refnum<vi>)
      n126 = control-ref of="Enter initial Velocity (m/s)  3"() -> (w191:refnum<vi>)
      n127 = control-ref of="mm"() -> (w175:refnum<vi>)
      n128 = control-ref of="Wear Track Diameter (mm)"() -> (w172:refnum<vi>)
      n129 = control-ref of="Enter the Angle (Deg)"() -> (w167:refnum<vi>)
      n130 = control-ref of="Enter the Frequency (Hz)"() -> (w166:refnum<vi>)
      n131 = control-ref of="Enter the Speed(mm/sec)"() -> (w149:refnum<vi>)
      n132 = control-ref of="Enter the Speed (RPM)"() -> (w148:refnum<vi>)
      n133 = control-ref of="Enter Scratch Speed (mm/s):"() -> (w147:refnum<vi>)
      n134 = control-ref of="Scartch Offset"() -> (w145:refnum<vi>)
      n135 = control-ref of="Enter Scratch length (mm):"() -> (w141:refnum<vi>)
      n136 = control-ref of="Wear Track Diameter"() -> (w140:refnum<vi>)
      n137 = control-ref of="No of Scratch"() -> (w138:refnum<vi>)
      n138 = control-ref of="String 39"() -> (w179:refnum<vi>)
      n139 = control-ref of="String 45"() -> (w151:refnum<vi>)
      n140 = control-ref of="Rotary Speed Exced"() -> (w139:refnum<vi>)
      n141 = control-ref of="StepTable For Load-Speed"() -> (w184:refnum<vi>)
      n142 = control-ref of="StepTable For Speed"() -> (w183:refnum<vi>)
      n143 = control-ref of="StepTable For Speed 3"() -> (w150:refnum<vi>)
      n144 = control-ref of="Motion Direction:  3"() -> (w203:refnum<vi>)
      n145 = control-ref of="Motion Mode:"() -> (w165:refnum<vi>)
      n146 = control-ref of="Scratch Mode"() -> (w144:refnum<vi>)
      n147 = control-ref of="Motion type:"() -> (w143:refnum<vi>)
      n148 = control-ref of="File Path :  2"() -> (w152:refnum<vi>)
      n149 = Bundle By Name(cluster=w208, "Motion Module.zNL"=w206, "Motion Module.NL disp"=w205, "Motion Module.Rotary Tab"=w204, "Motion Module.Motion Direction:  3"=w203, "Motion Module.E.Velocity 2"=w202, "Motion Module.e.v/ssr 2"=w201, "Motion Module.Enter Fixed E.Velocity 2"=w200, "Motion Module.Enter Final SRR 2"=w199, "Motion Module.Enter initial SRR 2"=w198, "Motion Module.Enter Fixed SRR 2"=w197, "Motion Module.Enter the Final E.Velocity (m/s) 2"=w196, "Motion Module.Enter initial E.Velocity (m/s) 2"=w195, "Motion Module.Final Speed (RPM) 3"=w194, "Motion Module.Initial Speed (RPM) 2"=w193, "Motion Module.Enter the Final Velocity (m/s) 3"=w192, "Motion Module.Enter initial Velocity (m/s)  3"=w191, "Motion Module.Ramp Up 2"=w190, "Motion Module.TEST SELECTION"=w189, "Motion Module.SPEED SELECTION :"=w188, "Motion Module.Angular Oscillation Set"=w187, "Motion Module.Traction"=w186, "Motion Module.Step Speed"=w185, "Motion Module.StepTable For Load-Speed"=w184, "Motion Module.StepTable For Speed"=w183, "Motion Module.Surge Forward MM"=w182, "Motion Module.Surge Backward MM"=w181, "Motion Module.M3 Image"=w180, "Motion Module.String 39"=w179, "Motion Module.Sway Left MM"=w178, "Motion Module.Sway Right MM"=w177, "Motion Module.Disable Axis Jog Soft Limits"=w176, "Motion Module.mm"=w175, "Motion Module.Heave Down MM"=w174, "Motion Module.Heave Up MM"=w173, "Motion Module.Wear Track Diameter (mm)"=w172, "Motion Module.Set WTD"=w171, "Motion Module.HomeScratch"=w170, "Motion Module.HomeRot"=w169, "Motion Module.PlaceModule"=w168, "Motion Module.Enter the Angle (Deg)"=w167, "Motion Module.Enter the Frequency (Hz)"=w166, "Motion Module.Motion Mode:"=w165, "Motion Module.LR Sway"=w164, "Motion Module.Rot Hor"=w163, "Motion Module.Scratch"=w162, "Motion Module.LR Cam"=w161, "Motion Module.MMBack"=w160, "Motion Module.MMNext"=w159, "Motion Module.Rot Ver"=w158, "Motion Module.Rotary Module Selection"=w157, "Motion Module.calculate rotary"=w156, "Motion Module.SPEED SELECTION : rotary"=w155, "Motion Module.Import 2"=w154, "Motion Module.Save 2"=w153, "Motion Module.File Path :  2"=w152, "Motion Module.String 45"=w151, "Motion Module.StepTable For Speed 3"=w150, "Motion Module.Enter the Speed(mm/sec)"=w149, "Motion Module.Enter the Speed(RPM)"=w148, "Motion Module.Enter Scratch Speed (mm/s):"=w147, "Motion Module.SwaySpeed Set"=w146, "Motion Module.Scartch Offset"=w145, "Motion Module.Scratch Mode"=w144, "Motion Module.Motion type:"=w143, "Motion Module.HomeScratch 2"=w142, "Motion Module.Enter Scratch length (mm):"=w141, "Motion Module.Wear Track Diameter"=w140, "Motion Module.Rotary Speed Exced"=w139, "Motion Module.No of Scratch"=w138) -> (w207:T11)
    }
    frame #6 {
      n150 = control-ref of="Add to list"() -> (w226:refnum<vi>)
      n151 = control-ref of="Wear"() -> (w225:refnum<vi>)
      n152 = control-ref of="Vibration"() -> (w224:refnum<vi>)
      n153 = control-ref of="Humidity (Chamber)"() -> (w223:refnum<vi>)
      n154 = control-ref of="Temperature (Chamber)"() -> (w222:refnum<vi>)
      n155 = control-ref of="ECR"() -> (w221:refnum<vi>)
      n156 = control-ref of="Temperature (Amb)"() -> (w220:refnum<vi>)
      n157 = control-ref of="Microphone"() -> (w219:refnum<vi>)
      n158 = control-ref of="Acoustic Emission 3"() -> (w218:refnum<vi>)
      n159 = control-ref of="SNext"() -> (w217:refnum<vi>)
      n160 = control-ref of="APBack"() -> (w216:refnum<vi>)
      n161 = control-ref of="Low Temp"() -> (w212:refnum<vi>)
      n162 = control-ref of="High Temp"() -> (w211:refnum<vi>)
      n163 = control-ref of="Humidity"() -> (w210:refnum<vi>)
      n164 = control-ref of="Humidity  Status  3"() -> (w233:refnum<vi>)
      n165 = control-ref of="Low Temp  Status  2"() -> (w232:refnum<vi>)
      n166 = control-ref of="TK4 status 2"() -> (w231:refnum<vi>)
      n167 = control-ref of="Humidity (Amb)"() -> (w228:refnum<vi>)
      n168 = control-ref of="Clear List"() -> (w227:refnum<vi>)
      n169 = control-ref of="Enter the Temperature (°C):"() -> (w215:refnum<vi>)
      n170 = control-ref of="Enter the Stage \nTemperature (°C):"() -> (w214:refnum<vi>)
      n171 = control-ref of="Enter the Humidity (%Rh):"() -> (w213:refnum<vi>)
      n172 = control-ref of="Sensors Picked"() -> (w209:refnum<vi>)
      n173 = control-ref of="Stage Temperature"() -> (w230:refnum<vi>)
      n174 = control-ref of="Sample Temperature"() -> (w229:refnum<vi>)
      n175 = Bundle By Name(cluster=w235, "Environmental control.Humidity  Status  3"=w233, "Environmental control.Low Temp  Status  2"=w232, "Environmental control.TK4 status 2"=w231, "Environmental control.Stage Temperature"=w230, "Environmental control.Sample Temperature"=w229, "Environmental control.Humidity (Amb)"=w228, "Environmental control.Clear List"=w227, "Environmental control.Add to list"=w226, "Environmental control.Wear"=w225, "Environmental control.Vibration"=w224, "Environmental control.Humidity (Chamber)"=w223, "Environmental control.Temperature (Chamber)"=w222, "Environmental control.ECR"=w221, "Environmental control.Temperature (Amb)"=w220, "Environmental control.Microphone"=w219, "Environmental control.Acoustic Emission 3"=w218, "Environmental control.SNext"=w217, "Environmental control.APBack"=w216, "Environmental control.Enter the Temperature (°C):"=w215, "Environmental control.Enter the Stage \nTemperature (°C):"=w214, "Environmental control.Enter the Humidity (%Rh):"=w213, "Environmental control.Low Temp"=w212, "Environmental control.High Temp"=w211, "Environmental control.Humidity"=w210, "Environmental control.Sensors Picked"=w209) -> (w234:T11)
    }
    frame #7 {
      n176 = control-ref of="ECR Port:"() -> (w245:refnum<vi>)
      n177 = control-ref of="Ramp Port:"() -> (w244:refnum<vi>)
      n178 = control-ref of="Heave and Surge COM Port:"() -> (w241:refnum<vi>)
      n179 = control-ref of="Sway COM Port:"() -> (w240:refnum<vi>)
      n180 = control-ref of="Temp Modbus:"() -> (w239:refnum<vi>)
      n181 = control-ref of="Humidity Port:"() -> (w238:refnum<vi>)
      n182 = control-ref of="About Tab"() -> (w246:refnum<vi>)
      n183 = control-ref of="Home Service"() -> (w248:refnum<vi>)
      n184 = control-ref of="Advanced Setting"() -> (w247:refnum<vi>)
      n185 = control-ref of="Installation/Replacement completed"() -> (w243:refnum<vi>)
      n186 = control-ref of="Loahead"() -> (w242:refnum<vi>)
      n187 = control-ref of="Edit Gain Constants"() -> (w237:refnum<vi>)
      n188 = control-ref of="Save Gain Constants"() -> (w236:refnum<vi>)
      n189 = control-ref of="Password"() -> (w249:refnum<vi>)
      n190 = Bundle By Name(cluster=w251, "About Screen.Password"=w249, "About Screen.Home Service"=w248, "About Screen.Advanced Setting"=w247, "About Screen.About Tab"=w246, "About Screen.ECR Port:"=w245, "About Screen.Ramp Port:"=w244, "About Screen.Installation/Replacement completed"=w243, "About Screen.Loahead"=w242, "About Screen.Heave and Surge COM Port:"=w241, "About Screen.Sway COM Port:"=w240, "About Screen.Temp Modbus:"=w239, "About Screen.Humidity Port:"=w238, "About Screen.Edit Gain Constants"=w237, "About Screen.Save Gain Constants"=w236) -> (w250:T11)
    }
    frame #8 {
      n191 = control-ref of="Cyclic Friction Force (N) Graph"() -> (w261:refnum<vi>)
      n192 = control-ref of="Cyclic Coefficient of Friction"() -> (w260:refnum<vi>)
      n193 = control-ref of="SDGp"() -> (w309:refnum<vi>)
      n194 = control-ref of="HumrGp"() -> (w307:refnum<vi>)
      n195 = control-ref of="gACQUOS"() -> (w304:refnum<vi>)
      n196 = control-ref of="ECR"() -> (w302:refnum<vi>)
      n197 = control-ref of="Temperature (deg c)"() -> (w300:refnum<vi>)
      n198 = control-ref of="MTM DISC  SPEED"() -> (w297:refnum<vi>)
      n199 = control-ref of="MTM BALL SPEED"() -> (w296:refnum<vi>)
      n200 = control-ref of="speed mm/sec"() -> (w295:refnum<vi>)
      n201 = control-ref of="WearGp"() -> (w285:refnum<vi>)
      n202 = control-ref of="Main Chart 3"() -> (w279:refnum<vi>)
      n203 = control-ref of="Friction Force (N) Graph"() -> (w267:refnum<vi>)
      n204 = control-ref of="Coefficient of Friction"() -> (w266:refnum<vi>)
      n205 = control-ref of="Main Screen Tab"() -> (w368:refnum<vi>)
      n206 = control-ref of="Angle and Frequency"() -> (w367:refnum<vi>)
      n207 = control-ref of="Main Speed Tab"() -> (w364:refnum<vi>)
      n208 = control-ref of="MTM MOTOR DISPLAY"() -> (w363:refnum<vi>)
      n209 = control-ref of="SPEED TAB"() -> (w358:refnum<vi>)
      n210 = control-ref of="Time Tab"() -> (w353:refnum<vi>)
      n211 = control-ref of="Temp Tabs"() -> (w346:refnum<vi>)
      n212 = control-ref of="Grp Tab"() -> (w313:refnum<vi>)
      n213 = control-ref of="Sub Graph"() -> (w312:refnum<vi>)
      n214 = control-ref of="Speed Tab"() -> (w298:refnum<vi>)
      n215 = control-ref of="FF Tab"() -> (w264:refnum<vi>)
      n216 = control-ref of="CZ FF"() -> (w262:refnum<vi>)
      n217 = control-ref of="Cyclic FF Disable Trip"() -> (w258:refnum<vi>)
      n218 = control-ref of="cyclic COF Disable Trip"() -> (w257:refnum<vi>)
      n219 = control-ref of="cyclic COF Reset Graph"() -> (w255:refnum<vi>)
      n220 = control-ref of="Cyclic FF Reset Graph"() -> (w254:refnum<vi>)
      n221 = control-ref of="Test Trip"() -> (w253:refnum<vi>)
      n222 = control-ref of="Scratch Start Test"() -> (w265:refnum<vi>)
      n223 = control-ref of="Heater"() -> (w345:refnum<vi>)
      n224 = control-ref of="TK4 status"() -> (w344:refnum<vi>)
      n225 = control-ref of="Controller  Status"() -> (w341:refnum<vi>)
      n226 = control-ref of="Cooling"() -> (w338:refnum<vi>)
      n227 = control-ref of="Load Communication"() -> (w337:refnum<vi>)
      n228 = control-ref of="HumCOMStatus"() -> (w335:refnum<vi>)
      n229 = control-ref of="Load En"() -> (w332:refnum<vi>)
      n230 = control-ref of="NLt"() -> (w331:refnum<vi>)
      n231 = control-ref of="zNL 2"() -> (w330:refnum<vi>)
      n232 = control-ref of="Humidity On"() -> (w329:refnum<vi>)
      n233 = control-ref of="AppLoadSeq scratch"() -> (w325:refnum<vi>)
      n234 = control-ref of="Stop Scratch"() -> (w324:refnum<vi>)
      n235 = control-ref of="ClrLog"() -> (w323:refnum<vi>)
      n236 = control-ref of="STOP"() -> (w321:refnum<vi>)
      n237 = control-ref of="Start Test"() -> (w320:refnum<vi>)
      n238 = control-ref of="Test status"() -> (w319:refnum<vi>)
      n239 = control-ref of="AR Led"() -> (w318:refnum<vi>)
      n240 = control-ref of="Data"() -> (w317:refnum<vi>)
      n241 = control-ref of="Health"() -> (w316:refnum<vi>)
      n242 = control-ref of="Sway COM Status"() -> (w315:refnum<vi>)
      n243 = control-ref of="Heave COM Status"() -> (w314:refnum<vi>)
      n244 = control-ref of="Siliding distance Reset Graph"() -> (w310:refnum<vi>)
      n245 = control-ref of="Humidity Reset Graph"() -> (w308:refnum<vi>)
      n246 = control-ref of="Aqucostic Reset Graph"() -> (w305:refnum<vi>)
      n247 = control-ref of="ECR RESET"() -> (w303:refnum<vi>)
      n248 = control-ref of="Temperature Reset"() -> (w301:refnum<vi>)
      n249 = control-ref of="Speed Reset Graph"() -> (w299:refnum<vi>)
      n250 = control-ref of="Hymidity"() -> (w294:refnum<vi>)
      n251 = control-ref of="Humidity Disable trip"() -> (w293:refnum<vi>)
      n252 = control-ref of="Weart Deapth"() -> (w290:refnum<vi>)
      n253 = control-ref of="Depth Reset Graph"() -> (w289:refnum<vi>)
      n254 = control-ref of="Weart"() -> (w288:refnum<vi>)
      n255 = control-ref of="Depthz"() -> (w287:refnum<vi>)
      n256 = control-ref of="Load pid"() -> (w283:refnum<vi>)
      n257 = control-ref of="Load Disable Trip"() -> (w282:refnum<vi>)
      n258 = control-ref of="Load Reset Graph"() -> (w281:refnum<vi>)
      n259 = control-ref of="BACK"() -> (w278:refnum<vi>)
      n260 = control-ref of="zFF"() -> (w268:refnum<vi>)
      n261 = control-ref of="FF Reset Graph"() -> (w274:refnum<vi>)
      n262 = control-ref of="FF Disable Trip"() -> (w273:refnum<vi>)
      n263 = control-ref of="COF Disable Trip"() -> (w271:refnum<vi>)
      n264 = control-ref of="COF Reset Graph"() -> (w270:refnum<vi>)
      n265 = control-ref of="Start Test Temp"() -> (w269:refnum<vi>)
      n266 = control-ref of="Depth Trip"() -> (w277:refnum<vi>)
      n267 = control-ref of="Multi Scratch Pass"() -> (w252:refnum<vi>)
      n268 = control-ref of="Cyclic Friction Force (N)"() -> (w263:refnum<vi>)
      n269 = control-ref of="Cyclic FF TRIP"() -> (w259:refnum<vi>)
      n270 = control-ref of="cyclic COF TRIP"() -> (w256:refnum<vi>)
      n271 = control-ref of="Stroke (mm)"() -> (w366:refnum<vi>)
      n272 = control-ref of="Angle (Deg)"() -> (w365:refnum<vi>)
      n273 = control-ref of="Disc Speed (m/sec)"() -> (w362:refnum<vi>)
      n274 = control-ref of="Ball Speed (m/sec)"() -> (w361:refnum<vi>)
      n275 = control-ref of="Disc Speed (RPM)"() -> (w360:refnum<vi>)
      n276 = control-ref of="Ball Speed (RPM)"() -> (w359:refnum<vi>)
      n277 = control-ref of="Speed (m/sec)"() -> (w357:refnum<vi>)
      n278 = control-ref of="Set Speed (m/sec)"() -> (w356:refnum<vi>)
      n279 = control-ref of="Speed (RPM)"() -> (w355:refnum<vi>)
      n280 = control-ref of="Set Speed"() -> (w354:refnum<vi>)
      n281 = control-ref of="Time ( HH:MM:SS ) 2"() -> (w352:refnum<vi>)
      n282 = control-ref of="Test Duration"() -> (w351:refnum<vi>)
      n283 = control-ref of="Test Duration 4"() -> (w350:refnum<vi>)
      n284 = control-ref of="TEST CYCLE"() -> (w349:refnum<vi>)
      n285 = control-ref of="TOTAL CYCLES"() -> (w348:refnum<vi>)
      n286 = control-ref of="Set Load (N)"() -> (w347:refnum<vi>)
      n287 = control-ref of="ChamberTemp"() -> (w343:refnum<vi>)
      n288 = control-ref of="SetTmp"() -> (w342:refnum<vi>)
      n289 = control-ref of="ChamberTemp"() -> (w340:refnum<vi>)
      n290 = control-ref of="SetTmp"() -> (w339:refnum<vi>)
      n291 = control-ref of="Ambient \nTemperature"() -> (w336:refnum<vi>)
      n292 = control-ref of="Ambient\n Humidity"() -> (w334:refnum<vi>)
      n293 = control-ref of="Freq (Hz)"() -> (w333:refnum<vi>)
      n294 = control-ref of="humidity disp"() -> (w328:refnum<vi>)
      n295 = control-ref of="Set Humidity"() -> (w327:refnum<vi>)
      n296 = control-ref of="NL disp 2"() -> (w326:refnum<vi>)
      n297 = control-ref of="SD (mm)"() -> (w311:refnum<vi>)
      n298 = control-ref of="Acoustic Emission (mV)"() -> (w306:refnum<vi>)
      n299 = control-ref of="CoF Trip  2"() -> (w292:refnum<vi>)
      n300 = control-ref of="Depth Trip"() -> (w291:refnum<vi>)
      n301 = control-ref of="Depth (µm)"() -> (w286:refnum<vi>)
      n302 = control-ref of="NL Trip 2"() -> (w284:refnum<vi>)
      n303 = control-ref of="NL Display 4"() -> (w280:refnum<vi>)
      n304 = control-ref of="COF TRIP"() -> (w276:refnum<vi>)
      n305 = control-ref of="Friction Force (N)"() -> (w275:refnum<vi>)
      n306 = control-ref of="FF TRIP"() -> (w272:refnum<vi>)
      n307 = control-ref of="Trip Log"() -> (w322:refnum<vi>)
      n308 = Bundle By Name(cluster=w370, "Main Screen.Test Trip"=w253, "Main Screen.Main Screen Tab"=w368, "Main Screen.Angle and Frequency"=w367, "Main Screen.Stroke (mm)"=w366, "Main Screen.Angle (Deg)"=w365, "Main Screen.Main Speed Tab"=w364, "Main Screen.MTM MOTOR DISPLAY"=w363, "Main Screen.Disc Speed (m/sec)"=w362, "Main Screen.Ball Speed (m/sec)"=w361, "Main Screen.Disc Speed (RPM)"=w360, "Main Screen.Ball Speed (RPM)"=w359, "Main Screen.SPEED TAB"=w358, "Main Screen.Speed (m/sec)"=w357, "Main Screen.Set Speed (m/sec)"=w356, "Main Screen.Speed (RPM)"=w355, "Main Screen.Set Speed"=w354, "Main Screen.Time Tab"=w353, "Main Screen.Time ( HH:MM:SS ) 2"=w352, "Main Screen.Test Duration"=w351, "Main Screen.Test Duration 4"=w350, "Main Screen.TEST CYCLE"=w349, "Main Screen.TOTAL CYCLES"=w348, "Main Screen.Set Load (N)"=w347, "Main Screen.Temp Tabs"=w346, "Main Screen.Heater"=w345, "Main Screen.TK4 status"=w344, "Main Screen.ChamberTemp"=w343, "Main Screen.SetTmp"=w342, "Main Screen.Controller  Status"=w341, "Main Screen.ChamberTemp 2"=w340, "Main Screen.SetTmp 2"=w339, "Main Screen.Cooling"=w338, "Main Screen.Load Communication"=w337, "Main Screen.Ambient \nTemperature"=w336, "Main Screen.HumCOMStatus"=w335, "Main Screen.Ambient\n Humidity"=w334, "Main Screen.Freq (Hz)"=w333, "Main Screen.Load En"=w332, "Main Screen.NLt"=w331, "Main Screen.zNL 2"=w330, "Main Screen.Humidity On"=w329, "Main Screen.humidity disp"=w328, "Main Screen.Set Humidity"=w327, "Main Screen.NL disp 2"=w326, "Main Screen.AppLoadSeq scratch"=w325, "Main Screen.Stop Scratch"=w324, "Main Screen.ClrLog"=w323, "Main Screen.Trip Log"=w322, "Main Screen.STOP"=w321, "Main Screen.Start Test"=w320, "Main Screen.Test status"=w319, "Main Screen.AR Led"=w318, "Main Screen.Data"=w317, "Main Screen.Health"=w316, "Main Screen.Sway COM Status"=w315, "Main Screen.Heave COM Status"=w314, "Main Screen.Grp Tab"=w313, "Main Screen.Sub Graph"=w312, "Main Screen.SD (mm)"=w311, "Main Screen.Siliding distance Reset Graph"=w310, "Main Screen.SDGp"=w309, "Main Screen.Humidity Reset Graph"=w308, "Main Screen.HumrGp"=w307, "Main Screen.Acoustic Emission (mV)"=w306, "Main Screen.Aqucostic Reset Graph"=w305, "Main Screen.gACQUOS"=w304, "Main Screen.ECR RESET"=w303, "Main Screen.ECR"=w302, "Main Screen.Temperature Reset"=w301, "Main Screen.Temperature (deg c)"=w300, "Main Screen.Speed Reset Graph"=w299, "Main Screen.Speed Tab"=w298, "Main Screen.MTM DISC  SPEED"=w297, "Main Screen.MTM BALL SPEED"=w296, "Main Screen.speed mm/sec"=w295, "Main Screen.Hymidity"=w294, "Main Screen.Humidity Disable trip"=w293, "Main Screen.CoF Trip  2"=w292, "Main Screen.Depth Trip"=w291, "Main Screen.Weart Deapth"=w290, "Main Screen.Depth Reset Graph"=w289, "Main Screen.Weart"=w288, "Main Screen.Depthz"=w287, "Main Screen.Depth (µm)"=w286, "Main Screen.WearGp"=w285, "Main Screen.NL Trip 2"=w284, "Main Screen.Load pid"=w283, "Main Screen.Load Disable Trip"=w282, "Main Screen.Load Reset Graph"=w281, "Main Screen.NL Display 4"=w280, "Main Screen.Main Chart 3"=w279, "Main Screen.BACK"=w278, "Main Screen.Depth Trip 2"=w277, "Main Screen.COF TRIP"=w276, "Main Screen.Friction Force (N)"=w275, "Main Screen.FF Reset Graph"=w274, "Main Screen.FF Disable Trip"=w273, "Main Screen.FF TRIP"=w272, "Main Screen.COF Disable Trip"=w271, "Main Screen.COF Reset Graph"=w270, "Main Screen.FF Tab"=w264, "Main Screen.Start Test Temp"=w269, "Main Screen.zFF"=w268, "Main Screen.Friction Force (N) Graph"=w267, "Main Screen.Coefficient of Friction"=w266, "Main Screen.Scratch Start Test"=w265, "Main Screen.Cyclic Friction Force (N)"=w263, "Main Screen.CZ FF"=w262, "Main Screen.Cyclic Friction Force (N) Graph"=w261, "Main Screen.Cyclic Coefficient of Friction"=w260, "Main Screen.Cyclic FF TRIP"=w259, "Main Screen.Cyclic FF Disable Trip"=w258, "Main Screen.cyclic COF Disable Trip"=w257, "Main Screen.cyclic COF TRIP"=w256, "Main Screen.cyclic COF Reset Graph"=w255, "Main Screen.Cyclic FF Reset Graph"=w254, "Main Screen.Multi Scratch Pass"=w252) -> (w369:T11)
    }
    frame #9 {
      n309 = control-ref of="gFF Rot 7"() -> (w374:refnum<vi>)
      n310 = control-ref of="Ramp"() -> (w393:refnum<vi>)
      n311 = control-ref of="Dummy Run"() -> (w387:refnum<vi>)
      n312 = control-ref of="AutoTune"() -> (w385:refnum<vi>)
      n313 = control-ref of="apply load"() -> (w383:refnum<vi>)
      n314 = control-ref of="reinit 3"() -> (w381:refnum<vi>)
      n315 = control-ref of="Bypass Load"() -> (w378:refnum<vi>)
      n316 = control-ref of="PID gains out delay (microForce)"() -> (w394:refnum<vi>)
      n317 = control-ref of="output range delay"() -> (w380:refnum<vi>)
      n318 = control-ref of="PID gains out delay"() -> (w379:refnum<vi>)
      n319 = control-ref of="Ramp MulFac"() -> (w398:refnum<vi>)
      n320 = control-ref of="pulses LoadDiffRamp(2..10)"() -> (w397:refnum<vi>)
      n321 = control-ref of="PulseControlRamp(diff<=3N)"() -> (w396:refnum<vi>)
      n322 = control-ref of="SetLoadDeadband(%) Load(0-10N)"() -> (w395:refnum<vi>)
      n323 = control-ref of="Gain 2"() -> (w392:refnum<vi>)
      n324 = control-ref of="pulses LoadDiff(2..10)"() -> (w391:refnum<vi>)
      n325 = control-ref of="pulses LoadDiff(11..50)"() -> (w390:refnum<vi>)
      n326 = control-ref of="PulseControl(diff<=3N)"() -> (w389:refnum<vi>)
      n327 = control-ref of="SetLoadDeadband(%)  2"() -> (w388:refnum<vi>)
      n328 = control-ref of="Vertical load (N)"() -> (w386:refnum<vi>)
      n329 = control-ref of="Offset  3"() -> (w384:refnum<vi>)
      n330 = control-ref of="Enter ByPass Load"() -> (w382:refnum<vi>)
      n331 = control-ref of="pulsesSent"() -> (w377:refnum<vi>)
      n332 = control-ref of="pulses"() -> (w376:refnum<vi>)
      n333 = control-ref of="actpid"() -> (w375:refnum<vi>)
      n334 = control-ref of="pulses LoadDiff(21..1000)"() -> (w373:refnum<vi>)
      n335 = control-ref of="Delay"() -> (w372:refnum<vi>)
      n336 = control-ref of="deadband"() -> (w371:refnum<vi>)
      n337 = Bundle By Name(cluster=w400, "PID.Ramp MulFac"=w398, "PID.pulses LoadDiffRamp(2..10)"=w397, "PID.PulseControlRamp(diff<=3N)"=w396, "PID.SetLoadDeadband(%) Load(0-10N)"=w395, "PID.PID gains out delay (microForce)"=w394, "PID.Ramp"=w393, "PID.Gain 2"=w392, "PID.pulses LoadDiff(2..10)"=w391, "PID.pulses LoadDiff(11..50)"=w390, "PID.PulseControl(diff<=3N)"=w389, "PID.SetLoadDeadband(%)  2"=w388, "PID.Dummy Run"=w387, "PID.Vertical load (N)"=w386, "PID.AutoTune"=w385, "PID.Offset 3"=w384, "PID.apply load"=w383, "PID.Enter ByPass Load"=w382, "PID.reinit 3"=w381, "PID.output range delay"=w380, "PID.PID gains out delay"=w379, "PID.Bypass Load"=w378, "PID.pulsesSent"=w377, "PID.pulses"=w376, "PID.actpid"=w375, "PID.gFF Rot"=w374, "PID.pulses LoadDiff(21..1000)"=w373, "PID.Delay"=w372, "PID.deadband"=w371) -> (w399:T11)
    }
    frame #10 {
      n338 = control-ref of="Tab Control 3"() -> (w451:refnum<vi>)
      n339 = control-ref of="Tab Control 19"() -> (w450:refnum<vi>)
      n340 = control-ref of="Tab Control 5"() -> (w411:refnum<vi>)
      n341 = control-ref of="Tab Control 14"() -> (w410:refnum<vi>)
      n342 = control-ref of="Tab Control 26"() -> (w409:refnum<vi>)
      n343 = control-ref of="Re-initilaize"() -> (w448:refnum<vi>)
      n344 = control-ref of="Filter ON/OFF"() -> (w447:refnum<vi>)
      n345 = control-ref of="Apply Filter (FF)"() -> (w443:refnum<vi>)
      n346 = control-ref of="Apply Filter (Load)"() -> (w441:refnum<vi>)
      n347 = control-ref of="SAVE  2"() -> (w436:refnum<vi>)
      n348 = control-ref of="Enter Distance"() -> (w435:refnum<vi>)
      n349 = control-ref of="AE"() -> (w408:refnum<vi>)
      n350 = control-ref of="Heave Loop Delay"() -> (w407:refnum<vi>)
      n351 = control-ref of="Heave PID Speed"() -> (w406:refnum<vi>)
      n352 = control-ref of="Surge Jog Speed"() -> (w405:refnum<vi>)
      n353 = control-ref of="Heave Jog Speed"() -> (w404:refnum<vi>)
      n354 = control-ref of="Sway Loop Delay"() -> (w403:refnum<vi>)
      n355 = control-ref of="Sway PID Speed"() -> (w402:refnum<vi>)
      n356 = control-ref of="Sway Jog Speed"() -> (w401:refnum<vi>)
      n357 = control-ref of="SAMPLES"() -> (w449:refnum<vi>)
      n358 = control-ref of="TracHomeSurgeOffsetCounts 10MM"() -> (w446:refnum<vi>)
      n359 = control-ref of="TracHomeSwayOffsetCounts 10MM"() -> (w445:refnum<vi>)
      n360 = control-ref of="Acoustic Emission:"() -> (w444:refnum<vi>)
      n361 = control-ref of="Filter% 2"() -> (w442:refnum<vi>)
      n362 = control-ref of="Filter%"() -> (w440:refnum<vi>)
      n363 = control-ref of="Sway distance (mm)"() -> (w439:refnum<vi>)
      n364 = control-ref of="Surge distance (mm)"() -> (w438:refnum<vi>)
      n365 = control-ref of="DataSavingLoopDelay(ms)"() -> (w437:refnum<vi>)
      n366 = control-ref of="Sway Counts:"() -> (w434:refnum<vi>)
      n367 = control-ref of="Distance (mm): 3"() -> (w433:refnum<vi>)
      n368 = control-ref of="Surge Counts:"() -> (w432:refnum<vi>)
      n369 = control-ref of="Distance (mm): 2"() -> (w431:refnum<vi>)
      n370 = control-ref of="Distance (mm):"() -> (w430:refnum<vi>)
      n371 = control-ref of="Heave Counts:"() -> (w429:refnum<vi>)
      n372 = control-ref of="LRMHomeSurgeOffsetCounts"() -> (w428:refnum<vi>)
      n373 = control-ref of="LRMHomeSwayOffsetCounts"() -> (w427:refnum<vi>)
      n374 = control-ref of="TracHomeSurgeOffsetCounts 20MM"() -> (w426:refnum<vi>)
      n375 = control-ref of="TracHomeSwayOffsetCounts 20MM"() -> (w425:refnum<vi>)
      n376 = control-ref of="RotHomeSwayOffsetCounts"() -> (w424:refnum<vi>)
      n377 = control-ref of="RotHomeSurgeOffsetCounts"() -> (w423:refnum<vi>)
      n378 = control-ref of="Heave distance"() -> (w422:refnum<vi>)
      n379 = control-ref of="Zmm"() -> (w421:refnum<vi>)
      n380 = control-ref of="Heave Pulses/mm"() -> (w420:refnum<vi>)
      n381 = control-ref of="Surge Pulses/mm"() -> (w419:refnum<vi>)
      n382 = control-ref of="Sway Pulses/mm"() -> (w418:refnum<vi>)
      n383 = control-ref of="Heave Pitch"() -> (w417:refnum<vi>)
      n384 = control-ref of="Surge Pitch"() -> (w416:refnum<vi>)
      n385 = control-ref of="Sway Pitch"() -> (w415:refnum<vi>)
      n386 = control-ref of="Heave PPR"() -> (w414:refnum<vi>)
      n387 = control-ref of="Surge PPR"() -> (w413:refnum<vi>)
      n388 = control-ref of="Sway PPR"() -> (w412:refnum<vi>)
      n389 = Bundle By Name(cluster=w453, "Config Parameters.Tab Control 3"=w451, "Config Parameters.Tab Control 19"=w450, "Config Parameters.SAMPLES"=w449, "Config Parameters.Re-initilaize"=w448, "Config Parameters.Filter ON/OFF"=w447, "Config Parameters.TracHomeSurgeOffsetCounts 10MM"=w446, "Config Parameters.TracHomeSwayOffsetCounts 10MM"=w445, "Config Parameters.Acoustic Emission:"=w444, "Config Parameters.Apply Filter (FF)"=w443, "Config Parameters.Filter% 2"=w442, "Config Parameters.Apply Filter (Load)"=w441, "Config Parameters.Filter%"=w440, "Config Parameters.Sway distance (mm)"=w439, "Config Parameters.Surge distance (mm)"=w438, "Config Parameters.DataSavingLoopDelay(ms)"=w437, "Config Parameters.SAVE 2"=w436, "Config Parameters.Enter Distance"=w435, "Config Parameters.Sway Counts:"=w434, "Config Parameters.Distance (mm): 3"=w433, "Config Parameters.Surge Counts:"=w432, "Config Parameters.Distance (mm): 2"=w431, "Config Parameters.Distance (mm):"=w430, "Config Parameters.Heave Counts:"=w429, "Config Parameters.LRMHomeSurgeOffsetCounts"=w428, "Config Parameters.LRMHomeSwayOffsetCounts"=w427, "Config Parameters.TracHomeSurgeOffsetCounts 20MM"=w426, "Config Parameters.TracHomeSwayOffsetCounts 20MM"=w425, "Config Parameters.RotHomeSwayOffsetCounts"=w424, "Config Parameters.RotHomeSurgeOffsetCounts"=w423, "Config Parameters.Heave distance"=w422, "Config Parameters.Zmm"=w421, "Config Parameters.Heave Pulses/mm"=w420, "Config Parameters.Surge Pulses/mm"=w419, "Config Parameters.Sway Pulses/mm"=w418, "Config Parameters.Heave Pitch"=w417, "Config Parameters.Surge Pitch"=w416, "Config Parameters.Sway Pitch"=w415, "Config Parameters.Heave PPR"=w414, "Config Parameters.Surge PPR"=w413, "Config Parameters.Sway PPR"=w412, "Config Parameters.Tab Control 5"=w411, "Config Parameters.Tab Control 14"=w410, "Config Parameters.Tab Control 26"=w409, "Config Parameters.AE"=w408, "Config Parameters.Heave Loop Delay"=w407, "Config Parameters.Heave PID Speed"=w406, "Config Parameters.Surge Jog Speed"=w405, "Config Parameters.Heave Jog Speed"=w404, "Config Parameters.Sway Loop Delay"=w403, "Config Parameters.Sway PID Speed"=w402, "Config Parameters.Sway Jog Speed"=w401) -> (w452:T11)
    }
    frame #11 {
      n390 = control-ref of="Mx"() -> (w483:refnum<vi>)
      n391 = control-ref of="My"() -> (w482:refnum<vi>)
      n392 = control-ref of="Mz"() -> (w481:refnum<vi>)
      n393 = control-ref of="Fx(N)"() -> (w480:refnum<vi>)
      n394 = control-ref of="Fy(N)"() -> (w479:refnum<vi>)
      n395 = control-ref of="Fz(N)"() -> (w478:refnum<vi>)
      n396 = control-ref of="Load Cell Temp"() -> (w454:refnum<vi>)
      n397 = control-ref of="ClearAll"() -> (w488:refnum<vi>)
      n398 = control-ref of="ZeroAll"() -> (w477:refnum<vi>)
      n399 = control-ref of="delete Handle"() -> (w467:refnum<vi>)
      n400 = control-ref of="Create Handle"() -> (w466:refnum<vi>)
      n401 = control-ref of="stop 6"() -> (w463:refnum<vi>)
      n402 = control-ref of="running_flag"() -> (w462:refnum<vi>)
      n403 = control-ref of="Save Dwell"() -> (w484:refnum<vi>)
      n404 = control-ref of="Acq Delay (ms)"() -> (w476:refnum<vi>)
      n405 = control-ref of="Burst Delay (ms)"() -> (w475:refnum<vi>)
      n406 = control-ref of="SN"() -> (w473:refnum<vi>)
      n407 = control-ref of="Port"() -> (w470:refnum<vi>)
      n408 = control-ref of="ft_udp_handle"() -> (w461:refnum<vi>)
      n409 = control-ref of="get-data-return"() -> (w460:refnum<vi>)
      n410 = control-ref of="get-range-return"() -> (w459:refnum<vi>)
      n411 = control-ref of="zero-return"() -> (w458:refnum<vi>)
      n412 = control-ref of="filter-return"() -> (w457:refnum<vi>)
      n413 = control-ref of="initial-return"() -> (w456:refnum<vi>)
      n414 = control-ref of="deleteHandle-result"() -> (w455:refnum<vi>)
      n415 = control-ref of="model"() -> (w474:refnum<vi>)
      n416 = control-ref of="Sensor IP"() -> (w471:refnum<vi>)
      n417 = control-ref of="Mz(Nm)"() -> (w487:refnum<vi>)
      n418 = control-ref of="My(Nm)"() -> (w486:refnum<vi>)
      n419 = control-ref of="Mx(Nm)"() -> (w485:refnum<vi>)
      n420 = control-ref of="FFx(N)"() -> (w472:refnum<vi>)
      n421 = control-ref of="FFy(N)"() -> (w469:refnum<vi>)
      n422 = control-ref of="Load(N)"() -> (w468:refnum<vi>)
      n423 = control-ref of="ft_data"() -> (w465:refnum<vi>)
      n424 = control-ref of="ft_range"() -> (w464:refnum<vi>)
      n425 = Bundle By Name(cluster=w490, "Loading Com Port.ClearAll"=w488, "Loading Com Port.Mz(Nm)"=w487, "Loading Com Port.My(Nm)"=w486, "Loading Com Port.Mx(Nm)"=w485, "Loading Com Port.Save Dwell"=w484, "Loading Com Port.Mx"=w483, "Loading Com Port.My"=w482, "Loading Com Port.Mz"=w481, "Loading Com Port.Fx(N)"=w480, "Loading Com Port.Fy(N)"=w479, "Loading Com Port.Fz(N)"=w478, "Loading Com Port.ZeroAll"=w477, "Loading Com Port.Acq Delay (ms)"=w476, "Loading Com Port.Burst Delay (ms)"=w475, "Loading Com Port.model"=w474, "Loading Com Port.SN"=w473, "Loading Com Port.FFx(N)"=w472, "Loading Com Port.Sensor IP"=w471, "Loading Com Port.Port"=w470, "Loading Com Port.FFy(N)"=w469, "Loading Com Port.Load(N)"=w468, "Loading Com Port.delete Handle"=w467, "Loading Com Port.Create Handle"=w466, "Loading Com Port.ft_data"=w465, "Loading Com Port.ft_range"=w464, "Loading Com Port.stop 6"=w463, "Loading Com Port.running_flag"=w462, "Loading Com Port.ft_udp_handle"=w461, "Loading Com Port.get-data-return"=w460, "Loading Com Port.get-range-return"=w459, "Loading Com Port.zero-return"=w458, "Loading Com Port.filter-return"=w457, "Loading Com Port.initial-return"=w456, "Loading Com Port.deleteHandle-result"=w455, "Loading Com Port.Load Cell Temp"=w454) -> (w489:T11)
    }
    frame #12 {
      n426 = control-ref of="Manual Write Heave & Surge"() -> (w492:refnum<vi>)
      n427 = control-ref of="Read Heave Temp"() -> (w515:refnum<vi>)
      n428 = control-ref of="error out Read"() -> (w527:refnum<vi>)
      n429 = control-ref of="error out Write"() -> (w522:refnum<vi>)
      n430 = control-ref of="SURGE POSE"() -> (w528:refnum<vi>)
      n431 = control-ref of="HEAVE POSE"() -> (w526:refnum<vi>)
      n432 = control-ref of="State"() -> (w525:refnum<vi>)
      n433 = control-ref of="Homed"() -> (w524:refnum<vi>)
      n434 = control-ref of="Sequence ID"() -> (w523:refnum<vi>)
      n435 = control-ref of="faultCode"() -> (w521:refnum<vi>)
      n436 = control-ref of="Ack ID"() -> (w520:refnum<vi>)
      n437 = control-ref of="SPEED"() -> (w519:refnum<vi>)
      n438 = control-ref of="Distance"() -> (w518:refnum<vi>)
      n439 = control-ref of="Mode Command"() -> (w517:refnum<vi>)
      n440 = control-ref of="SPARE 2"() -> (w514:refnum<vi>)
      n441 = control-ref of="SPARE 1"() -> (w513:refnum<vi>)
      n442 = control-ref of="Spare 15"() -> (w512:refnum<vi>)
      n443 = control-ref of="Spare 14"() -> (w511:refnum<vi>)
      n444 = control-ref of="Spare 13"() -> (w510:refnum<vi>)
      n445 = control-ref of="Spare 12"() -> (w509:refnum<vi>)
      n446 = control-ref of="Spare 11"() -> (w508:refnum<vi>)
      n447 = control-ref of="Spare 10"() -> (w507:refnum<vi>)
      n448 = control-ref of="Spare 9"() -> (w506:refnum<vi>)
      n449 = control-ref of="Spare 8"() -> (w505:refnum<vi>)
      n450 = control-ref of="Spare 7"() -> (w504:refnum<vi>)
      n451 = control-ref of="Spare 6"() -> (w503:refnum<vi>)
      n452 = control-ref of="Spare 5"() -> (w502:refnum<vi>)
      n453 = control-ref of="Spare 4"() -> (w501:refnum<vi>)
      n454 = control-ref of="Spare 3"() -> (w500:refnum<vi>)
      n455 = control-ref of="Spare 2"() -> (w499:refnum<vi>)
      n456 = control-ref of="Spare 1"() -> (w498:refnum<vi>)
      n457 = control-ref of="Node Id"() -> (w497:refnum<vi>)
      n458 = control-ref of="SPARE 3"() -> (w496:refnum<vi>)
      n459 = control-ref of="SPARE 4"() -> (w495:refnum<vi>)
      n460 = control-ref of="fwMajor"() -> (w494:refnum<vi>)
      n461 = control-ref of="fwMinor"() -> (w493:refnum<vi>)
      n462 = control-ref of="Heave and Surge Write"() -> (w491:refnum<vi>)
      n463 = control-ref of="Heave and Surge Read"() -> (w516:refnum<vi>)
      n464 = Bundle By Name(cluster=w530, "Heave AND Surge.SURGE POSE"=w528, "Heave AND Surge.error out Read"=w527, "Heave AND Surge.HEAVE POSE"=w526, "Heave AND Surge.State"=w525, "Heave AND Surge.Homed"=w524, "Heave AND Surge.Sequence ID"=w523, "Heave AND Surge.error out Write"=w522, "Heave AND Surge.faultCode"=w521, "Heave AND Surge.Ack ID"=w520, "Heave AND Surge.SPEED"=w519, "Heave AND Surge.Distance"=w518, "Heave AND Surge.Mode Command"=w517, "Heave AND Surge.Heave and Surge Read"=w516, "Heave AND Surge.Read Heave Temp"=w515, "Heave AND Surge.SPARE 2"=w514, "Heave AND Surge.SPARE 1"=w513, "Heave AND Surge.Spare 15"=w512, "Heave AND Surge.Spare 14"=w511, "Heave AND Surge.Spare 13"=w510, "Heave AND Surge.Spare 12"=w509, "Heave AND Surge.Spare 11"=w508, "Heave AND Surge.Spare 10"=w507, "Heave AND Surge.Spare 9"=w506, "Heave AND Surge.Spare 8"=w505, "Heave AND Surge.Spare 7"=w504, "Heave AND Surge.Spare 6"=w503, "Heave AND Surge.Spare 5"=w502, "Heave AND Surge.Spare 4"=w501, "Heave AND Surge.Spare 3"=w500, "Heave AND Surge.Spare 2"=w499, "Heave AND Surge.Spare 1"=w498, "Heave AND Surge.Node Id"=w497, "Heave AND Surge.SPARE 3"=w496, "Heave AND Surge.SPARE 4"=w495, "Heave AND Surge.fwMajor"=w494, "Heave AND Surge.fwMinor"=w493, "Heave AND Surge.Manual Write"=w492, "Heave AND Surge.Heave and Surge Write"=w491) -> (w529:T11)
    }
    frame #13 {
      n465 = control-ref of="Fine Tune Zone"() -> (w546:refnum<vi>)
      n466 = control-ref of="PID Delay (sec)"() -> (w545:refnum<vi>)
      n467 = control-ref of="Max_pos_limit"() -> (w544:refnum<vi>)
      n468 = control-ref of="Min_pos_limit"() -> (w543:refnum<vi>)
      n469 = control-ref of="i_limit"() -> (w542:refnum<vi>)
      n470 = control-ref of="pct_scale"() -> (w533:refnum<vi>)
      n471 = control-ref of="Deadband"() -> (w541:refnum<vi>)
      n472 = control-ref of="Kd"() -> (w540:refnum<vi>)
      n473 = control-ref of="Ki"() -> (w539:refnum<vi>)
      n474 = control-ref of="Kp"() -> (w538:refnum<vi>)
      n475 = control-ref of="Current Position"() -> (w537:refnum<vi>)
      n476 = control-ref of="Set Load"() -> (w536:refnum<vi>)
      n477 = control-ref of="Current Load"() -> (w535:refnum<vi>)
      n478 = control-ref of="Pulse delta"() -> (w534:refnum<vi>)
      n479 = control-ref of="Init Step"() -> (w532:refnum<vi>)
      n480 = control-ref of="Max Step Linit"() -> (w531:refnum<vi>)
      n481 = Bundle By Name(cluster=w548, "New PID LOGIC.Fine Tune Zone"=w546, "New PID LOGIC.PID SDelay"=w545, "New PID LOGIC.Max_pos_limit"=w544, "New PID LOGIC.Min_pos_limit"=w543, "New PID LOGIC.i_limit"=w542, "New PID LOGIC.pct_scale"=w533, "New PID LOGIC.Deadband"=w541, "New PID LOGIC.Kd"=w540, "New PID LOGIC.Ki"=w539, "New PID LOGIC.Kp"=w538, "New PID LOGIC.Current Position"=w537, "New PID LOGIC.Set Load"=w536, "New PID LOGIC.Current Load"=w535, "New PID LOGIC.Pulse delta"=w534, "New PID LOGIC.Init Step"=w532, "New PID LOGIC.Max Step Linit"=w531) -> (w547:T11)
    }
    frame #14 {
      n482 = control-ref of="Manual Write SWAY"() -> (w568:refnum<vi>)
      n483 = control-ref of="Read SWAY Temp"() -> (w549:refnum<vi>)
      n484 = control-ref of="error out Write  SWAY"() -> (w570:refnum<vi>)
      n485 = control-ref of="error out Read SWAY"() -> (w569:refnum<vi>)
      n486 = control-ref of="fwMajor"() -> (w587:refnum<vi>)
      n487 = control-ref of="Homed"() -> (w586:refnum<vi>)
      n488 = control-ref of="Rotary POSE"() -> (w585:refnum<vi>)
      n489 = control-ref of="State"() -> (w584:refnum<vi>)
      n490 = control-ref of="SWAY POSE"() -> (w583:refnum<vi>)
      n491 = control-ref of="Ack ID"() -> (w582:refnum<vi>)
      n492 = control-ref of="faultCode"() -> (w581:refnum<vi>)
      n493 = control-ref of="Node Id"() -> (w580:refnum<vi>)
      n494 = control-ref of="fwMinor"() -> (w579:refnum<vi>)
      n495 = control-ref of="Spare 6"() -> (w578:refnum<vi>)
      n496 = control-ref of="Spare 5"() -> (w577:refnum<vi>)
      n497 = control-ref of="Spare 4"() -> (w576:refnum<vi>)
      n498 = control-ref of="Spare 3"() -> (w575:refnum<vi>)
      n499 = control-ref of="Spare 2"() -> (w574:refnum<vi>)
      n500 = control-ref of="Spare 1"() -> (w573:refnum<vi>)
      n501 = control-ref of="Spare 7"() -> (w572:refnum<vi>)
      n502 = control-ref of="SPARE  5"() -> (w571:refnum<vi>)
      n503 = control-ref of="SPARE  4"() -> (w566:refnum<vi>)
      n504 = control-ref of="SPARE  3"() -> (w565:refnum<vi>)
      n505 = control-ref of="SPARE 2"() -> (w564:refnum<vi>)
      n506 = control-ref of="SPARE 1"() -> (w563:refnum<vi>)
      n507 = control-ref of="Spare 15"() -> (w562:refnum<vi>)
      n508 = control-ref of="Spare 14"() -> (w561:refnum<vi>)
      n509 = control-ref of="Spare 13"() -> (w560:refnum<vi>)
      n510 = control-ref of="Spare 12"() -> (w559:refnum<vi>)
      n511 = control-ref of="Spare 11"() -> (w558:refnum<vi>)
      n512 = control-ref of="Spare 9"() -> (w557:refnum<vi>)
      n513 = control-ref of="Spare 8"() -> (w556:refnum<vi>)
      n514 = control-ref of="SPEED"() -> (w555:refnum<vi>)
      n515 = control-ref of="Distance"() -> (w554:refnum<vi>)
      n516 = control-ref of="Mode Command"() -> (w553:refnum<vi>)
      n517 = control-ref of="Sequence ID"() -> (w552:refnum<vi>)
      n518 = control-ref of="Spare 10"() -> (w550:refnum<vi>)
      n519 = control-ref of="SWAY WRITE"() -> (w567:refnum<vi>)
      n520 = control-ref of="SWAY READ"() -> (w551:refnum<vi>)
      n521 = Bundle By Name(cluster=w589, "SWAY.fwMajor"=w587, "SWAY.Homed"=w586, "SWAY.Rotary POSE"=w585, "SWAY.State"=w584, "SWAY.SWAY POSE"=w583, "SWAY.Ack ID"=w582, "SWAY.faultCode"=w581, "SWAY.Node Id"=w580, "SWAY.fwMinor"=w579, "SWAY.Spare 6"=w578, "SWAY.Spare 5"=w577, "SWAY.Spare 4"=w576, "SWAY.Spare 3"=w575, "SWAY.Spare 2"=w574, "SWAY.Spare 1"=w573, "SWAY.Spare 7"=w572, "SWAY.SPARE  5"=w571, "SWAY.error out Write  SWAY"=w570, "SWAY.error out Read SWAY"=w569, "SWAY.Manual Write SWAY"=w568, "SWAY.SWAY WRITE"=w567, "SWAY.SPARE  4"=w566, "SWAY.SPARE  3"=w565, "SWAY.SPARE 2"=w564, "SWAY.SPARE 1"=w563, "SWAY.Spare 15"=w562, "SWAY.Spare 14"=w561, "SWAY.Spare 13"=w560, "SWAY.Spare 12"=w559, "SWAY.Spare 11"=w558, "SWAY.Spare 9"=w557, "SWAY.Spare 8"=w556, "SWAY.SPEED"=w555, "SWAY.Distance"=w554, "SWAY.Mode Command"=w553, "SWAY.Sequence ID"=w552, "SWAY.SWAY READ"=w551, "SWAY.Spare 10"=w550, "SWAY.Read SWAY Temp"=w549) -> (w588:T11)
    }
    frame #15 {
      n522 = control-ref of="Analysis Home new"() -> (w618:refnum<vi>)
      n523 = control-ref of="Refresh 2"() -> (w617:refnum<vi>)
      n524 = control-ref of="OPEN 4"() -> (w603:refnum<vi>)
      n525 = control-ref of="OPEN 3"() -> (w601:refnum<vi>)
      n526 = control-ref of="XY Graph"() -> (w596:refnum<vi>)
      n527 = control-ref of="OPEN 2"() -> (w593:refnum<vi>)
      n528 = control-ref of="OPEN 1"() -> (w592:refnum<vi>)
      n529 = control-ref of="MEAN"() -> (w616:refnum<vi>)
      n530 = control-ref of="SD"() -> (w615:refnum<vi>)
      n531 = control-ref of="VARIANCE"() -> (w614:refnum<vi>)
      n532 = control-ref of="MEAN"() -> (w613:refnum<vi>)
      n533 = control-ref of="SD"() -> (w612:refnum<vi>)
      n534 = control-ref of="VARIANCE"() -> (w611:refnum<vi>)
      n535 = control-ref of="MEAN"() -> (w610:refnum<vi>)
      n536 = control-ref of="SD"() -> (w609:refnum<vi>)
      n537 = control-ref of="VARIANCE"() -> (w608:refnum<vi>)
      n538 = control-ref of="MEAN"() -> (w607:refnum<vi>)
      n539 = control-ref of="SD"() -> (w606:refnum<vi>)
      n540 = control-ref of="VARIANCE"() -> (w605:refnum<vi>)
      n541 = control-ref of="File 4 Discription"() -> (w604:refnum<vi>)
      n542 = control-ref of="File Name 4"() -> (w602:refnum<vi>)
      n543 = control-ref of="File 3 Discription"() -> (w600:refnum<vi>)
      n544 = control-ref of="File Name 3"() -> (w599:refnum<vi>)
      n545 = control-ref of="File Name 2"() -> (w595:refnum<vi>)
      n546 = control-ref of="File Name 1"() -> (w594:refnum<vi>)
      n547 = control-ref of="File 1 Discription"() -> (w591:refnum<vi>)
      n548 = control-ref of="File 2 Discription"() -> (w590:refnum<vi>)
      n549 = control-ref of="Y-AXIS"() -> (w598:refnum<vi>)
      n550 = control-ref of="X-AXIS"() -> (w597:refnum<vi>)
      n551 = Bundle By Name(cluster=w620, "Analysis Screen.Analysis Home"=w618, "Analysis Screen.Refresh 2"=w617, "Analysis Screen.MEAN 4"=w616, "Analysis Screen.SD 4"=w615, "Analysis Screen.VARIANCE 4"=w614, "Analysis Screen.MEAN  3"=w613, "Analysis Screen.SD  3"=w612, "Analysis Screen.VARIANCE  3"=w611, "Analysis Screen.MEAN 2"=w610, "Analysis Screen.SD  2"=w609, "Analysis Screen.VARIANCE 2"=w608, "Analysis Screen.MEAN"=w607, "Analysis Screen.SD"=w606, "Analysis Screen.VARIANCE"=w605, "Analysis Screen.File 4 Discription"=w604, "Analysis Screen.OPEN 4"=w603, "Analysis Screen.File Name 4"=w602, "Analysis Screen.OPEN 3"=w601, "Analysis Screen.File 3 Discription"=w600, "Analysis Screen.File Name 3"=w599, "Analysis Screen.Y-AXIS"=w598, "Analysis Screen.X-AXIS"=w597, "Analysis Screen.XY Graph"=w596, "Analysis Screen.File Name 2"=w595, "Analysis Screen.File Name 1"=w594, "Analysis Screen.OPEN 2"=w593, "Analysis Screen.OPEN 1"=w592, "Analysis Screen.File 1 Discription"=w591, "Analysis Screen.File 2 Discription"=w590) -> (w619:T11)
    }
  }
  n552 = call <userlib>:"Fit VI window to Largest Dec.vi"() -> ("error out"=w31:errorcluster, "dup VI Ref"=w28:refnum<vi>)  [unwired: 6 in]
  n553 = invoke on="Invoke Node" class="VI" method="FP.Run-Time Position.Maximized"(reference=w28, error in=w31) -> (error out=w30:errorcluster)  [unwired: 2 in, 3 out]
  n554 = call <vilib>:"Clear Errors.vi"("error in (no error)"=w30) -> ("error out"=w29:errorcluster)  [unwired: 5 in, 1 out]
  n555 = control-ref of="This VI"() -> (w34:refnum<vi>)
  n556 = invoke on="Invoke Node" class="VI" method="Default Vals.Reinit All"(reference=w34, error in=w29) -> (reference out=w32:refnum<vi>, error out=w33:errorcluster)  [unwired: 1 in, 1 out]
  n557 = Close Reference(reference=w32, error in (no error)=w33) -> (error out=w27:errorcluster)
  n558 = call "Create User Event - Stop.vi"("error in (no error)"=w27) -> ("error out"=w5:errorcluster, "User Event - Stop"=w14:refnum<user-event>)  [unwired: 9 in]
  n559 = call "main screen queue out Unitest.vi"("error in (no error)"=w5) -> ("error out"=w54:errorcluster, "output Queue"=w26:T12)  [unwired: 9 in]
  n560 = Unbundle By Name(w26) -> ("RAMP MOTOR COM LOOP"=w19:refnum<queue>)
  n561 = Unbundle By Name(w26) -> ("TEMPERATURE COM LOOP"=w21:refnum<queue>)
  n562 = Unbundle By Name(w26) -> ("ECR PORT"=w18:refnum<queue>)
  n563 = Unbundle By Name(w26) -> ("SWAY MOTOR COM LOOP"=w23:refnum<queue>)
  n564 = Unbundle By Name(w26) -> ("UI Loop"=w52:refnum<queue>)
  n565 = Unbundle By Name(w26) -> ("LOAD COM LOOP"=w24:refnum<queue>)
  n566 = Unbundle By Name(w26) -> ("HEAVE MOTOR COM LOOP"=w6:refnum<queue>)
  n567 = Unbundle By Name(w26) -> ("HUMIDITY COM PORT"=w17:refnum<queue>)
  n568 = Unbundle By Name(w26) -> ("PROGRAM LOOP"=w16:refnum<queue>)
  n569 = Unbundle By Name(w26) -> ("MONITOR LOOP"=w13:refnum<queue>)
  n570 = Unbundle By Name(w26) -> ("LOAD PID"=w12:refnum<queue>)
  n571 = Unbundle By Name(w26) -> ("REPORT"=w11:refnum<queue>)
  n572 = register-events(w14) -> (reference out=w46:refnum<event-registration>, error out=w44:errorcluster)  [unwired: 2 in]
  n573 = Merge Errors(w44, w54) -> (w45:errorcluster)
  n574 = while {
    tunnel: w52 -> [w628]
    shift-right: [w626] -> w49
    shift-left: w46 -> [w627]
    tunnel: [w622] -> w47
    stop <- w624 stop-if-true
    # "Event Handling Loop"
    n575 = event shown="[68] \"Scratch Mode\": Value Change" {
      selector: w627 -> [_ _ _ _ _ _ _ _ _ _ _ _ _ _ _ _ _ _ _ _ _ _ _ _ _ _ _ _ _ _ _ _ _ _ _ _ _ _ _ _ _ _ _ _ _ _ _ _ _ _ _ _ _ _ _ _ _ _ _ _ _ _ _ _ _ _ _ _ _ _ _ _]
      dyn-events: [_ _ _ _ _ _ _ _ _ _ _ _ _ _ _ _ _ _ _ _ _ _ _ _ _ _ _ _ _ _ _ _ _ _ _ _ _ _ _ _ _ _ _ _ _ _ _ _ _ _ _ _ _ _ _ _ _ _ _ _ _ _ _ _ _ _ _ _ _ _ _ _] -> w626
      timeout: 10 -> [_ _ _ _ _ _ _ _ _ _ _ _ _ _ _ _ _ _ _ _ _ _ _ _ _ _ _ _ _ _ _ _ _ _ _ _ _ _ _ _ _ _ _ _ _ _ _ _ _ _ _ _ _ _ _ _ _ _ _ _ _ _ _ _ _ _ _ _ _ _ _ _]
      tunnel: [_ _ _ _ _ _ _ _ _ _ _ _ _ _ _ _ _ _ _ _ _ _ _ _ _ _ _ _ _ _ _ _ _ _ _ _ _ _ _ _ _ _ _ _ _ _ _ _ _ _ _ _ _ _ _ _ _ _ _ _ _ _ _ _ _ _ _ _ _ _ _ TRUE ("Discard?")] -> w624
      tunnel: w628 -> [w633 w637 w642 w647 w652 w657 w662 w667 w672 w677 w682 w687 w692 w697 w702 w707 w712 w717 w722 w727 w732 w737 w742 w747 w752 w757 w762 w767 w772 w777 w782 w787 w792 w797 w802 w807 w812 w817 w822 w827 w832 w837 w842 w847 w852 w857 w862 w867 w872 w877 w882 w887 w892 w897 w902 w907 w912 w917 w922 w927 w932 w937 w942 w947 w952 w957 w962 w967 w972 w975 w980 w982]
      tunnel: [w632 w635 w640 w645 w650 w655 w660 w665 w670 w675 w680 w685 w690 w695 w700 w705 w710 w715 w720 w725 w730 w735 w740 w745 w750 w755 w760 w765 w770 w775 w780 w785 w790 w795 w800 w805 w810 w815 w820 w825 w830 w835 w840 w845 w850 w855 w860 w865 w870 w875 w880 w885 w890 w895 w900 w905 w910 w915 w920 w925 w930 w935 w940 w945 w950 w955 w960 w965 w970 _ w979 _] -> w625
      tunnel: [w631 w636 w641 w646 w651 w656 w661 w666 w671 w676 w681 w686 w691 w696 w701 w706 w711 w716 w721 w726 w731 w736 w741 w746 w751 w756 w761 w766 w771 w776 w781 w786 w791 w796 w801 w806 w811 w816 w821 w826 w831 w836 w841 w846 w851 w856 w861 w866 w871 w876 w881 w886 w891 w896 w901 w906 w911 w916 w921 w926 w931 w936 w941 w946 w951 w956 w961 w966 w971 w975 w978 w982] -> w623
      event Panel Close? {
        n576 = event-data() -> ()  [unwired: 1 in, 1 out]
        n577 = call-poly "Enqueue Message.vi"("Priority Message? (F)"=TRUE, "Message"="Confirm Quit", "Message Queue"=w633) -> ("error out"=w632:errorcluster, "dup Message Queue"=w631:refnum<queue>)  [unwired: 7 in]
        n578 = event-data("Discard?"=TRUE) -> ()  [unwired: 1 in, 1 out]
      }
      event Timeout {
        n579 = event-data() -> ()  [unwired: 1 in, 1 out]
        n580 = call-poly "Enqueue Message.vi"("Priority Message? (F)"=TRUE, "Message"="Time Out", "Message Queue"=w637) -> ("error out"=w635:errorcluster, "dup Message Queue"=w636:refnum<queue>)  [unwired: 7 in]
      }
      event "SAVE  2": Value Change {
        n581 = event-data() -> ()  [unwired: 1 in, 1 out]
        n582 = call-poly "Enqueue Message.vi"("Priority Message? (F)"=TRUE, "Message"="Service Save", "Message Queue"=w642) -> ("error out"=w640:errorcluster, "dup Message Queue"=w641:refnum<queue>)  [unwired: 7 in]
      }
      event "Home": Value Change {
        n583 = event-data() -> ()  [unwired: 1 in, 1 out]
        n584 = call-poly "Enqueue Message.vi"("Priority Message? (F)"=TRUE, "Message"="HOME", "Message Queue"=w647) -> ("error out"=w645:errorcluster, "dup Message Queue"=w646:refnum<queue>)  [unwired: 7 in]
      }
      event "Platform Settings": Value Change {
        n585 = event-data() -> ()  [unwired: 1 in, 1 out]
        n586 = call-poly "Enqueue Message.vi"("Priority Message? (F)"=TRUE, "Message"="Platform Setting", "Message Queue"=w652) -> ("error out"=w650:errorcluster, "dup Message Queue"=w651:refnum<queue>)  [unwired: 7 in]
      }
      event "Configure": Value Change {
        n587 = event-data() -> ()  [unwired: 1 in, 1 out]
        n588 = call-poly "Enqueue Message.vi"("Priority Message? (F)"=TRUE, "Message"="Configure", "Message Queue"=w657) -> ("error out"=w655:errorcluster, "dup Message Queue"=w656:refnum<queue>)  [unwired: 7 in]
      }
      event "Analysis": Value Change {
        n589 = event-data() -> ()  [unwired: 1 in, 1 out]
        n590 = call-poly "Enqueue Message.vi"("Priority Message? (F)"=TRUE, "Message"="Analysis", "Message Queue"=w662) -> ("error out"=w660:errorcluster, "dup Message Queue"=w661:refnum<queue>)  [unwired: 7 in]
      }
      event "service 2": Value Change {
        n591 = event-data() -> ()  [unwired: 1 in, 1 out]
        n592 = call-poly "Enqueue Message.vi"("Priority Message? (F)"=TRUE, "Message"="service 2", "Message Queue"=w667) -> ("error out"=w665:errorcluster, "dup Message Queue"=w666:refnum<queue>)  [unwired: 7 in]
      }
      event "Auto": Value Change {
        n593 = event-data() -> ()  [unwired: 1 in, 1 out]
        n594 = call-poly "Enqueue Message.vi"("Priority Message? (F)"=TRUE, "Message"="Auto", "Message Queue"=w672) -> ("error out"=w670:errorcluster, "dup Message Queue"=w671:refnum<queue>)  [unwired: 7 in]
      }
      event "Select Load Head": Value Change {
        n595 = event-data() -> ()  [unwired: 1 in, 1 out]
        n596 = call-poly "Enqueue Message.vi"("Priority Message? (F)"=TRUE, "Message"="Select Load Head", "Message Queue"=w677) -> ("error out"=w675:errorcluster, "dup Message Queue"=w676:refnum<queue>)  [unwired: 7 in]
      }
      event "com 3": Value Change {
        n597 = event-data() -> ()  [unwired: 1 in, 1 out]
        n598 = call-poly "Enqueue Message.vi"("Priority Message? (F)"=TRUE, "Message"="com 3", "Message Queue"=w682) -> ("error out"=w680:errorcluster, "dup Message Queue"=w681:refnum<queue>)  [unwired: 7 in]
      }
      event "Loading Mode": Value Change {
        n599 = event-data() -> ()  [unwired: 1 in, 1 out]
        n600 = call-poly "Enqueue Message.vi"("Priority Message? (F)"=TRUE, "Message"="Loading Mode", "Message Queue"=w687) -> ("error out"=w685:errorcluster, "dup Message Queue"=w686:refnum<queue>)  [unwired: 7 in]
      }
      event "SSP 0.3": Value Change {
        n601 = event-data() -> ()  [unwired: 1 in, 1 out]
        n602 = call-poly "Enqueue Message.vi"("Priority Message? (F)"=TRUE, "Message"="SSP 0.3", "Message Queue"=w692) -> ("error out"=w690:errorcluster, "dup Message Queue"=w691:refnum<queue>)  [unwired: 7 in]
      }
      event "SSP 0.5": Value Change {
        n603 = event-data() -> ()  [unwired: 1 in, 1 out]
        n604 = call-poly "Enqueue Message.vi"("Priority Message? (F)"=TRUE, "Message"="SSP 0.5", "Message Queue"=w697) -> ("error out"=w695:errorcluster, "dup Message Queue"=w696:refnum<queue>)  [unwired: 7 in]
      }
      event "SSP 0.75": Value Change {
        n605 = event-data() -> ()  [unwired: 1 in, 1 out]
        n606 = call-poly "Enqueue Message.vi"("Priority Message? (F)"=TRUE, "Message"="SSP 0.75", "Message Queue"=w702) -> ("error out"=w700:errorcluster, "dup Message Queue"=w701:refnum<queue>)  [unwired: 7 in]
      }
      event "LHBack": Value Change {
        n607 = event-data() -> ()  [unwired: 1 in, 1 out]
        n608 = call-poly "Enqueue Message.vi"("Priority Message? (F)"=TRUE, "Message"="LHBack", "Message Queue"=w707) -> ("error out"=w705:errorcluster, "dup Message Queue"=w706:refnum<queue>)  [unwired: 7 in]
      }
      event "LHNext": Value Change {
        n609 = event-data() -> ()  [unwired: 1 in, 1 out]
        n610 = call-poly "Enqueue Message.vi"("Priority Message? (F)"=TRUE, "Message"="LHNext", "Message Queue"=w712) -> ("error out"=w710:errorcluster, "dup Message Queue"=w711:refnum<queue>)  [unwired: 7 in]
      }
      event "Rot Ver": Value Change {
        n611 = event-data() -> ()  [unwired: 1 in, 1 out]
        n612 = call-poly "Enqueue Message.vi"("Priority Message? (F)"=TRUE, "Message"="Rot Ver", "Message Queue"=w717) -> ("error out"=w715:errorcluster, "dup Message Queue"=w716:refnum<queue>)  [unwired: 7 in]
      }
      event "Scratch": Value Change {
        n613 = event-data() -> ()  [unwired: 1 in, 1 out]
        n614 = call-poly "Enqueue Message.vi"("Priority Message? (F)"=TRUE, "Message"="Scratch", "Message Queue"=w722) -> ("error out"=w720:errorcluster, "dup Message Queue"=w721:refnum<queue>)  [unwired: 7 in]
      }
      event "Motion Mode:": Value Change {
        n615 = event-data() -> ()  [unwired: 1 in, 1 out]
        n616 = call-poly "Enqueue Message.vi"("Priority Message? (F)"=TRUE, "Message"="Motion Mode:", "Message Queue"=w727) -> ("error out"=w725:errorcluster, "dup Message Queue"=w726:refnum<queue>)  [unwired: 7 in]
      }
      event "MMBack": Value Change {
        n617 = event-data() -> ()  [unwired: 1 in, 1 out]
        n618 = call-poly "Enqueue Message.vi"("Priority Message? (F)"=TRUE, "Message"="MMBack", "Message Queue"=w732) -> ("error out"=w730:errorcluster, "dup Message Queue"=w731:refnum<queue>)  [unwired: 7 in]
      }
      event "MMNext": Value Change {
        n619 = event-data() -> ()  [unwired: 1 in, 1 out]
        n620 = call-poly "Enqueue Message.vi"("Priority Message? (F)"=TRUE, "Message"="MMNext", "Message Queue"=w737) -> ("error out"=w735:errorcluster, "dup Message Queue"=w736:refnum<queue>)  [unwired: 7 in]
      }
      event "APBack": Value Change {
        n621 = event-data() -> ()  [unwired: 1 in, 1 out]
        n622 = call-poly "Enqueue Message.vi"("Priority Message? (F)"=TRUE, "Message"="APBack", "Message Queue"=w742) -> ("error out"=w740:errorcluster, "dup Message Queue"=w741:refnum<queue>)  [unwired: 7 in]
      }
      event "SNext": Value Change {
        n623 = event-data() -> ()  [unwired: 1 in, 1 out]
        n624 = call-poly "Enqueue Message.vi"("Priority Message? (F)"=TRUE, "Message"="SNext", "Message Queue"=w747) -> ("error out"=w745:errorcluster, "dup Message Queue"=w746:refnum<queue>)  [unwired: 7 in]
      }
      event "ZeroAll": Value Change {
        n625 = event-data() -> ()  [unwired: 1 in, 1 out]
        n626 = call-poly "Enqueue Message.vi"("Priority Message? (F)"=TRUE, "Message"="ZeroAll", "Message Queue"=w752) -> ("error out"=w750:errorcluster, "dup Message Queue"=w751:refnum<queue>)  [unwired: 7 in]
      }
      event "Enable Platform": Value Change {
        n627 = event-data() -> ()  [unwired: 1 in, 1 out]
        n628 = call-poly "Enqueue Message.vi"("Priority Message? (F)"=TRUE, "Message"="Enable Platform", "Message Queue"=w757) -> ("error out"=w755:errorcluster, "dup Message Queue"=w756:refnum<queue>)  [unwired: 7 in]
      }
      event "Heave Up main": Value Change {
        n629 = event-data() -> ()  [unwired: 1 in, 1 out]
        n630 = call-poly "Enqueue Message.vi"("Priority Message? (F)"=TRUE, "Message"="Heave Up main", "Message Queue"=w762) -> ("error out"=w760:errorcluster, "dup Message Queue"=w761:refnum<queue>)  [unwired: 7 in]
      }
      event "Heave Up MM": Value Change {
        n631 = event-data() -> ()  [unwired: 1 in, 1 out]
        n632 = call-poly "Enqueue Message.vi"("Priority Message? (F)"=TRUE, "Message"="Heave Up MM", "Message Queue"=w767) -> ("error out"=w765:errorcluster, "dup Message Queue"=w766:refnum<queue>)  [unwired: 7 in]
      }
      event "Heave Down Main": Value Change {
        n633 = event-data() -> ()  [unwired: 1 in, 1 out]
        n634 = call-poly "Enqueue Message.vi"("Priority Message? (F)"=TRUE, "Message"="Heave Down Main", "Message Queue"=w772) -> ("error out"=w770:errorcluster, "dup Message Queue"=w771:refnum<queue>)  [unwired: 7 in]
      }
      event "Heave Down MM": Value Change {
        n635 = event-data() -> ()  [unwired: 1 in, 1 out]
        n636 = call-poly "Enqueue Message.vi"("Priority Message? (F)"=TRUE, "Message"="Heave Down MM", "Message Queue"=w777) -> ("error out"=w775:errorcluster, "dup Message Queue"=w776:refnum<queue>)  [unwired: 7 in]
      }
      event "Manual Write Heave & Surge": Value Change {
        n637 = event-data() -> ()  [unwired: 1 in, 1 out]
        n638 = call-poly "Enqueue Message.vi"("Priority Message? (F)"=TRUE, "Message"="Manual Write Heave & Surge", "Message Queue"=w782) -> ("error out"=w780:errorcluster, "dup Message Queue"=w781:refnum<queue>)  [unwired: 7 in]
      }
      event "Manual Write SWAY": Value Change {
        n639 = event-data() -> ()  [unwired: 1 in, 1 out]
        n640 = call-poly "Enqueue Message.vi"("Priority Message? (F)"=TRUE, "Message"="Manual Write SWAY", "Message Queue"=w787) -> ("error out"=w785:errorcluster, "dup Message Queue"=w786:refnum<queue>)  [unwired: 7 in]
      }
      event "Surge Backward Main": Value Change {
        n641 = event-data() -> ()  [unwired: 1 in, 1 out]
        n642 = call-poly "Enqueue Message.vi"("Priority Message? (F)"=TRUE, "Message"="Surge Backward Main", "Message Queue"=w792) -> ("error out"=w790:errorcluster, "dup Message Queue"=w791:refnum<queue>)  [unwired: 7 in]
      }
      event "Surge Backward MM": Value Change {
        n643 = event-data() -> ()  [unwired: 1 in, 1 out]
        n644 = call-poly "Enqueue Message.vi"("Priority Message? (F)"=TRUE, "Message"="Surge Backward MM", "Message Queue"=w797) -> ("error out"=w795:errorcluster, "dup Message Queue"=w796:refnum<queue>)  [unwired: 7 in]
      }
      event "Surge Forward Main": Value Change {
        n645 = event-data() -> ()  [unwired: 1 in, 1 out]
        n646 = call-poly "Enqueue Message.vi"("Priority Message? (F)"=TRUE, "Message"="Surge Forward Main", "Message Queue"=w802) -> ("error out"=w800:errorcluster, "dup Message Queue"=w801:refnum<queue>)  [unwired: 7 in]
      }
      event "Surge Forward MM": Value Change {
        n647 = event-data() -> ()  [unwired: 1 in, 1 out]
        n648 = call-poly "Enqueue Message.vi"("Priority Message? (F)"=TRUE, "Message"="Surge Forward MM", "Message Queue"=w807) -> ("error out"=w805:errorcluster, "dup Message Queue"=w806:refnum<queue>)  [unwired: 7 in]
      }
      event "Sway Left Main": Value Change {
        n649 = event-data() -> ()  [unwired: 1 in, 1 out]
        n650 = call-poly "Enqueue Message.vi"("Priority Message? (F)"=TRUE, "Message"="Sway Left Main", "Message Queue"=w812) -> ("error out"=w810:errorcluster, "dup Message Queue"=w811:refnum<queue>)  [unwired: 7 in]
      }
      event "Sway Left MM": Value Change {
        n651 = event-data() -> ()  [unwired: 1 in, 1 out]
        n652 = call-poly "Enqueue Message.vi"("Priority Message? (F)"=TRUE, "Message"="Sway Left MM", "Message Queue"=w817) -> ("error out"=w815:errorcluster, "dup Message Queue"=w816:refnum<queue>)  [unwired: 7 in]
      }
      event "Sway Right MM": Value Change {
        n653 = event-data() -> ()  [unwired: 1 in, 1 out]
        n654 = call-poly "Enqueue Message.vi"("Priority Message? (F)"=TRUE, "Message"="Sway Right MM", "Message Queue"=w822) -> ("error out"=w820:errorcluster, "dup Message Queue"=w821:refnum<queue>)  [unwired: 7 in]
      }
      event "Sway Right Main": Value Change {
        n655 = event-data() -> ()  [unwired: 1 in, 1 out]
        n656 = call-poly "Enqueue Message.vi"("Priority Message? (F)"=TRUE, "Message"="Sway Right Main", "Message Queue"=w827) -> ("error out"=w825:errorcluster, "dup Message Queue"=w826:refnum<queue>)  [unwired: 7 in]
      }
      event "Load En": Value Change {
        n657 = event-data() -> ()  [unwired: 1 in, 1 out]
        n658 = call-poly "Enqueue Message.vi"("Priority Message? (F)"=TRUE, "Message"="Load En", "Message Queue"=w832) -> ("error out"=w830:errorcluster, "dup Message Queue"=w831:refnum<queue>)  [unwired: 7 in]
      }
      event "apply load": Value Change {
        n659 = event-data() -> ()  [unwired: 1 in, 1 out]
        n660 = call-poly "Enqueue Message.vi"("Priority Message? (F)"=TRUE, "Message"="apply load", "Message Queue"=w837) -> ("error out"=w835:errorcluster, "dup Message Queue"=w836:refnum<queue>)  [unwired: 7 in]
      }
      event "BACK": Value Change {
        n661 = event-data() -> ()  [unwired: 1 in, 1 out]
        n662 = call-poly "Enqueue Message.vi"("Priority Message? (F)"=TRUE, "Message"="BACK", "Message Queue"=w842) -> ("error out"=w840:errorcluster, "dup Message Queue"=w841:refnum<queue>)  [unwired: 7 in]
      }
      event "Start Test": Value Change {
        n663 = event-data() -> ()  [unwired: 1 in, 1 out]
        n664 = call-poly "Enqueue Message.vi"("Priority Message? (F)"=TRUE, "Message"="Start Test", "Message Queue"=w847) -> ("error out"=w845:errorcluster, "dup Message Queue"=w846:refnum<queue>)  [unwired: 7 in]
      }
      event "STOP": Value Change {
        n665 = event-data() -> ()  [unwired: 1 in, 1 out]
        n666 = call-poly "Enqueue Message.vi"("Priority Message? (F)"=TRUE, "Message"="STOP", "Message Queue"=w852) -> ("error out"=w850:errorcluster, "dup Message Queue"=w851:refnum<queue>)  [unwired: 7 in]
      }
      event "PlaceModule": Value Change {
        n667 = event-data() -> ()  [unwired: 1 in, 1 out]
        n668 = call-poly "Enqueue Message.vi"("Priority Message? (F)"=TRUE, "Message"="PlaceModule", "Message Queue"=w857) -> ("error out"=w855:errorcluster, "dup Message Queue"=w856:refnum<queue>)  [unwired: 7 in]
      }
      event "HomeRot", "HomeScratch", "HomeScratch": Value Change {
        n669 = event-data() -> ()  [unwired: 1 in, 1 out]
        n670 = call-poly "Enqueue Message.vi"("Priority Message? (F)"=TRUE, "Message"="Stage Homing", "Message Queue"=w862) -> ("error out"=w860:errorcluster, "dup Message Queue"=w861:refnum<queue>)  [unwired: 7 in]
      }
      event "Clear 3": Value Change {
        n671 = event-data() -> ()  [unwired: 1 in, 1 out]
        n672 = call-poly "Enqueue Message.vi"("Priority Message? (F)"=TRUE, "Message"="Clear 3", "Message Queue"=w867) -> ("error out"=w865:errorcluster, "dup Message Queue"=w866:refnum<queue>)  [unwired: 7 in]
      }
      event "Set WTD": Value Change {
        n673 = event-data() -> ()  [unwired: 1 in, 1 out]
        n674 = call-poly "Enqueue Message.vi"("Priority Message? (F)"=TRUE, "Message"="Set WTD", "Message Queue"=w872) -> ("error out"=w870:errorcluster, "dup Message Queue"=w871:refnum<queue>)  [unwired: 7 in]
      }
      event "Import 2": Value Change {
        n675 = event-data() -> ()  [unwired: 1 in, 1 out]
        n676 = call-poly "Enqueue Message.vi"("Priority Message? (F)"=TRUE, "Message"="Import 2", "Message Queue"=w877) -> ("error out"=w875:errorcluster, "dup Message Queue"=w876:refnum<queue>)  [unwired: 7 in]
      }
      event "Save 2": Value Change {
        n677 = event-data() -> ()  [unwired: 1 in, 1 out]
        n678 = call-poly "Enqueue Message.vi"("Priority Message? (F)"=TRUE, "Message"="Save 2", "Message Queue"=w882) -> ("error out"=w880:errorcluster, "dup Message Queue"=w881:refnum<queue>)  [unwired: 7 in]
      }
      event "calculate rotary": Value Change {
        n679 = event-data() -> ()  [unwired: 1 in, 1 out]
        n680 = call-poly "Enqueue Message.vi"("Priority Message? (F)"=TRUE, "Message"="Calculate Rotary", "Message Queue"=w887) -> ("error out"=w885:errorcluster, "dup Message Queue"=w886:refnum<queue>)  [unwired: 7 in]
      }
      event "Clear List": Value Change {
        n681 = event-data() -> ()  [unwired: 1 in, 1 out]
        n682 = call-poly "Enqueue Message.vi"("Priority Message? (F)"=TRUE, "Message"="Clear List", "Message Queue"=w892) -> ("error out"=w890:errorcluster, "dup Message Queue"=w891:refnum<queue>)  [unwired: 7 in]
      }
      event "Add to list": Value Change {
        n683 = event-data() -> ()  [unwired: 1 in, 1 out]
        n684 = call-poly "Enqueue Message.vi"("Priority Message? (F)"=TRUE, "Message"="Add to list", "Message Queue"=w897) -> ("error out"=w895:errorcluster, "dup Message Queue"=w896:refnum<queue>)  [unwired: 7 in]
      }
      event "ClrLog": Value Change {
        n685 = event-data() -> ()  [unwired: 1 in, 1 out]
        n686 = call-poly "Enqueue Message.vi"("Priority Message? (F)"=TRUE, "Message"="ClrLog", "Message Queue"=w902) -> ("error out"=w900:errorcluster, "dup Message Queue"=w901:refnum<queue>)  [unwired: 7 in]
      }
      event "Disable Axis Jog Soft Limits m": Value Change {
        n687 = event-data() -> ()  [unwired: 1 in, 1 out]
        n688 = call-poly "Enqueue Message.vi"("Priority Message? (F)"=TRUE, "Message"="Disable Axis Jog Soft Limits", "Message Queue"=w907) -> ("error out"=w905:errorcluster, "dup Message Queue"=w906:refnum<queue>)  [unwired: 7 in]
      }
      event "Home Service": Value Change {
        n689 = event-data() -> ()  [unwired: 1 in, 1 out]
        n690 = call-poly "Enqueue Message.vi"("Priority Message? (F)"=TRUE, "Message"="Home Service", "Message Queue"=w912) -> ("error out"=w910:errorcluster, "dup Message Queue"=w911:refnum<queue>)  [unwired: 7 in]
      }
      event "Edit Gain Constants": Value Change {
        n691 = event-data() -> ()  [unwired: 1 in, 1 out]
        n692 = call-poly "Enqueue Message.vi"("Priority Message? (F)"=TRUE, "Message"="Edit Gain Constants", "Message Queue"=w917) -> ("error out"=w915:errorcluster, "dup Message Queue"=w916:refnum<queue>)  [unwired: 7 in]
      }
      event "Advanced Setting": Value Change {
        n693 = event-data() -> ()  [unwired: 1 in, 1 out]
        n694 = call-poly "Enqueue Message.vi"("Priority Message? (F)"=TRUE, "Message"="Advanced Setting", "Message Queue"=w922) -> ("error out"=w920:errorcluster, "dup Message Queue"=w921:refnum<queue>)  [unwired: 7 in]
      }
      event "Password": Value Change {
        n695 = event-data() -> ()  [unwired: 1 in, 1 out]
        n696 = call-poly "Enqueue Message.vi"("Priority Message? (F)"=TRUE, "Message"="Password", "Message Queue"=w927) -> ("error out"=w925:errorcluster, "dup Message Queue"=w926:refnum<queue>)  [unwired: 7 in]
      }
      event "Service About": Value Change {
        n697 = event-data() -> ()  [unwired: 1 in, 1 out]
        n698 = call-poly "Enqueue Message.vi"("Priority Message? (F)"=TRUE, "Message"="Service About", "Message Queue"=w932) -> ("error out"=w930:errorcluster, "dup Message Queue"=w931:refnum<queue>)  [unwired: 7 in]
      }
      event "OPEN 1": Value Change {
        n699 = event-data() -> ()  [unwired: 1 in, 1 out]
        n700 = call-poly "Enqueue Message.vi"("Priority Message? (F)"=TRUE, "Message"="OPEN 1", "Message Queue"=w937) -> ("error out"=w935:errorcluster, "dup Message Queue"=w936:refnum<queue>)  [unwired: 7 in]
      }
      event "OPEN 2": Value Change {
        n701 = event-data() -> ()  [unwired: 1 in, 1 out]
        n702 = call-poly "Enqueue Message.vi"("Priority Message? (F)"=TRUE, "Message"="OPEN 2", "Message Queue"=w942) -> ("error out"=w940:errorcluster, "dup Message Queue"=w941:refnum<queue>)  [unwired: 7 in]
      }
      event "OPEN 3": Value Change {
        n703 = event-data() -> ()  [unwired: 1 in, 1 out]
        n704 = call-poly "Enqueue Message.vi"("Priority Message? (F)"=TRUE, "Message"="OPEN 3", "Message Queue"=w947) -> ("error out"=w945:errorcluster, "dup Message Queue"=w946:refnum<queue>)  [unwired: 7 in]
      }
      event "OPEN 4": Value Change {
        n705 = event-data() -> ()  [unwired: 1 in, 1 out]
        n706 = call-poly "Enqueue Message.vi"("Priority Message? (F)"=TRUE, "Message"="OPEN 4", "Message Queue"=w952) -> ("error out"=w950:errorcluster, "dup Message Queue"=w951:refnum<queue>)  [unwired: 7 in]
      }
      event "Refresh 2": Value Change {
        n707 = event-data() -> ()  [unwired: 1 in, 1 out]
        n708 = call-poly "Enqueue Message.vi"("Priority Message? (F)"=TRUE, "Message"="Refresh 2", "Message Queue"=w957) -> ("error out"=w955:errorcluster, "dup Message Queue"=w956:refnum<queue>)  [unwired: 7 in]
      }
      event "Analysis Home new": Value Change {
        n709 = event-data() -> ()  [unwired: 1 in, 1 out]
        n710 = call-poly "Enqueue Message.vi"("Priority Message? (F)"=TRUE, "Message"="Analysis Home", "Message Queue"=w962) -> ("error out"=w960:errorcluster, "dup Message Queue"=w961:refnum<queue>)  [unwired: 7 in]
      }
      event "Post Analysis": Value Change {
        n711 = event-data() -> ()  [unwired: 1 in, 1 out]
        n712 = call-poly "Enqueue Message.vi"("Priority Message? (F)"=TRUE, "Message"="Post Analysis", "Message Queue"=w967) -> ("error out"=w965:errorcluster, "dup Message Queue"=w966:refnum<queue>)  [unwired: 7 in]
      }
      event "Scratch Mode": Value Change {
        n713 = event-data() -> ()  [unwired: 1 in, 1 out]
        n714 = call-poly "Enqueue Message.vi"("Priority Message? (F)"=TRUE, "Message"="Scratch Mode", "Message Queue"=w972) -> ("error out"=w970:errorcluster, "dup Message Queue"=w971:refnum<queue>)  [unwired: 7 in]
      }
      event Application Instance Close {
        # "#CodeRecommended - When a project closes, all VIs within that project are aborted and leave memory. However, any code placed in this event frame is guaranteed to run to completion, so add any cleanup code that absolutely must happen here."
        n715 = event-data() -> ()  [unwired: 1 in, 1 out]
      }
      event "EXIT": Value Change {
        n716 = event-data() -> ()  [unwired: 1 in, 1 out]
        n717 = call-poly "Enqueue Message.vi"("Priority Message? (F)"=TRUE, "Message"="Exit", "Message Queue"=w980) -> ("error out"=w979:errorcluster, "dup Message Queue"=w978:refnum<queue>)  [unwired: 7 in]
      }
      event User Event {
        # "The Message Handling Loop processed an \"Exit\" message, which fired this event to stop the Event Handling Loop."
        n718 = event-data() -> ()  [unwired: 1 in, 1 out]
      }
    }
    n719 = call "LAB-IQ Error Handler - Event Handling Loop.vi"("error in (no error)"=w625, "Message Queue"=w623) -> ("dup error in"=w622:errorcluster)  [unwired: 8 in, 1 out]
  }
  n720 = while {
    tunnel: w52 -> [w986]
    shift-right: [w993] -> _
    shift-left: w15 -> [w994]
    tunnel: w14 -> [w991]
    tunnel: w45 -> [w990]
    tunnel: [w984] -> w53
    stop <- w992 stop-if-true
    # "Message Handling Loop"
    n721 = call "Dequeue Message.vi"("error in (no error)"=w990, "Message Queue"=w986) -> ("error out"=w989:errorcluster, "Message Data"=w987:variant, "Message"=w988:string, "dup Message Queue"=w985:refnum<queue>)  [unwired: 6 in]
    n722 = case "Message Cases" shown="\"Time Out\"" w988 {
      selector: w988 -> [_ _ _ _ _ _ _ _ _ _ _ _ _ _ _ _ _ _ _ _ _ _ _ _ _ _ _ _ _ _ _ _ _ _ _ _ _ _ _ _ _ _ _ _ _ _ _ _ _ _ _ _ _ _ _ _ _ _ _ _ _ _ _ _ _ _ _ _ _ _ _ _ _ w2285]
      tunnel: w985 -> [_ w1048 _ _ _ _ _ _ _ _ _ _ _ _ _ _ _ _ _ _ _ _ _ _ _ _ _ _ _ _ _ _ _ _ _ _ _ _ _ _ _ _ _ _ _ _ _ _ _ _ _ _ _ _ _ _ _ _ _ _ _ _ _ _ _ _ _ _ _ _ _ w2273 w2284 _]
      tunnel: w989 -> [w996 w1050 w1052 w1056 w1077 w1094 w1111 w1128 w1149 w1162 w1167 w1171 w1178 w1183 w1248 w1274 w1300 w1335 w1351 w1403 w1407 w1410 w1417 w1460 w1472 w1501 w1531 w1550 w1561 w1572 w1583 w1594 w1605 w1616 w1627 w1639 w1650 w1661 w1672 w1681 w1692 w1703 w1733 w1774 w1780 w1796 w1800 w1803 w1811 w1823 w1832 w1852 w1866 w1876 w1886 w1888 w1903 w1916 w1929 w1946 w1982 w1990 w2049 w2073 w2083 w2124 w2167 w2210 w2245 w2252 w2269 w2276 w2277 _]
      tunnel: [w1005 w1017 w1052 w1057 w1072 w1089 w1106 w1123 w1144 w1154 w1165 w1169 w1176 w1187 w1244 w1270 w1296 w1336 w1352 w1367 w1406 w1409 w1416 w1459 w1471 w1500 w1518 w1552 w1563 w1574 w1585 w1596 w1607 w1618 w1629 w1640 w1651 w1662 w1673 w1683 w1693 w1702 w1732 w1753 w1779 w1797 w1799 w1802 w1810 w1817 w1827 w1845 w1865 w1876 w1886 w1894 w1902 w1915 w1928 w1945 w1981 w1989 w2049 w2073 w2080 w2121 w2164 w2207 w2246 w2252 w2263 w2275 w2280 w2286] -> w983
      tunnel: w994 -> [w997 w1008 w1053 w1055 w1063 w1080 w1097 w1114 w1132 w1152 w1164 w1168 w1174 w1182 w1246 w1272 w1298 w1323 w1338 w1354 w1405 w1408 w1411 w1454 w1470 w1483 w1513 w1548 w1559 w1570 w1581 w1592 w1603 w1614 w1625 w1637 w1648 w1659 w1670 w1680 w1691 w1701 w1731 w1752 w1778 w1782 w1798 w1801 w1805 w1816 w1825 w1847 w1864 w1868 w1878 w1887 w1901 w1905 w1918 w1932 w1948 w1984 w2041 w2064 w2076 w2117 w2160 w2203 w2244 w2247 w2268 w2270 w2283 w2287]
      tunnel: [w997 w1008 w1053 w1055 w1063 w1080 w1097 w1114 w1132 w1152 w1164 w1168 w1174 w1182 w1246 w1272 w1298 w1323 w1338 w1354 w1405 w1408 w1411 w1454 w1470 w1483 w1513 w1548 w1559 w1570 w1581 w1592 w1603 w1614 w1625 w1637 w1648 w1659 w1670 w1680 w1691 w1701 w1731 w1752 w1778 w1782 w1798 w1801 w1805 w1816 w1825 w1847 w1864 w1868 w1878 w1887 w1901 w1905 w1918 w1932 w1948 w1984 w2041 w2064 w2076 w2117 w2160 w2203 w2244 w2247 w2268 w2270 w2283 w2287] -> w993
      tunnel: [_ _ _ _ _ _ _ _ _ _ _ _ _ _ _ _ _ _ _ _ _ _ _ _ _ _ _ _ _ _ _ _ _ _ _ _ _ _ _ _ _ _ _ _ _ _ _ _ _ _ _ _ _ _ _ _ _ _ _ _ _ _ _ _ _ _ _ _ _ _ _ _ TRUE _] -> w992
      tunnel: w987 -> [_ _ _ _ _ _ _ _ _ _ _ _ _ _ _ _ _ _ _ _ _ _ _ _ _ _ _ _ _ _ _ _ _ _ _ _ _ _ _ _ _ _ _ _ _ _ _ _ _ _ _ _ _ _ _ _ _ _ _ _ _ _ _ _ _ _ _ _ _ _ w2267 _ _ _]
      tunnel: w991 -> [_ _ _ _ _ _ _ _ _ _ _ _ _ _ _ _ _ _ _ _ _ _ _ _ _ _ _ _ _ _ _ _ _ _ _ _ _ _ _ _ _ _ _ _ _ _ _ _ _ _ _ _ _ _ _ _ _ _ _ _ _ _ _ _ _ _ _ _ _ _ _ _ w2279 _]
      frame "Time Out" {
        n723 = call "File Name Entereed Check.vi"("error in (no error)"=w996, "Data Cluster"=w997) -> ("error out"=w1002:errorcluster)  [unwired: 9 in]
        n724 = call "Load Cell and Susppension Selection Parameter.vi"("error in (no error)"=w996, "Data Cluster"=w997) -> ("error out"=w1001:errorcluster)  [unwired: 9 in]
        n725 = call "Load Cell Higher Value in Steps.vi"("error in (no error)"=w996, "main ref"=w997) -> ("error out"=w1000:errorcluster)  [unwired: 9 in]
        n726 = call "To Check whether module selected.vi"("error in (no error)"=w996, "main ref"=w997) -> ("error out"=w999:errorcluster)  [unwired: 9 in]
        n727 = call "Rotatry Speed Limit Ristriction.vi"("error in (no error)"=w996, "main ref"=w997) -> ("error out"=w998:errorcluster)  [unwired: 9 in]
        n728 = call "JOG LIMIT.vi"("error in (no error)"=w996, "main ref"=w997) -> ("error out"=w995:errorcluster)  [unwired: 9 in]
        n729 = call "Pulse_mm conversion loop.vi"("error in (no error)"=w996, "main ref"=w997) -> ("error out"=w1006:errorcluster)  [unwired: 9 in]
        n730 = call "Load Commiunication Error.vi"("error in (no error)"=w996, "main ref"=w997) -> ("error out"=w1003:errorcluster)  [unwired: 9 in]
        n731 = call "Stage Homing Error Display Status.vi"("error in (no error)"=w996, "Data Cluster"=w997) -> ("error out"=w1004:errorcluster)  [unwired: 9 in]
        n732 = Merge Errors(w1006, w1003, w1004, w1002, w1001, w1000, w999, w998, w995) -> (w1005:errorcluster)
      }
      frame "init" {
        # "Initialize - All initialization work should take place in this message, since other loops can potentially enqueue messages that execute immediately after this one."
        n733 = call-poly "Enqueue Message.vi"("error in (no error)"=w1050, "Message"="Init Other Loop", "Message Queue"=w1048) -> ("error out"=w1051:errorcluster)  [unwired: 7 in, 1 out]
        n734 = Unbundle By Name(w1008) -> ("Loading.SSP 0.3"=w1036:refnum<vi>)
        n735 = Unbundle By Name(w1008) -> ("Loading.SSP 0.5"=w1033:refnum<vi>)
        n736 = Unbundle By Name(w1008) -> ("Loading.SSP 0.75"=w1028:refnum<vi>)
        n737 = Unbundle By Name(w1008) -> ("Loading.Communication is established"=w1023:refnum<vi>)
        n738 = Unbundle By Name(w1008) -> ("Loading Com Port.Load Cell Temp"=w1042:refnum<vi>)
        n739 = Unbundle By Name(w1008) -> ("Motion Module.Set WTD"=w1016:refnum<vi>)
        n740 = call "Read Config Unitest.vi"("error in (no error)"=w1051, "main ref"=w1008) -> ("error out"=w1046:errorcluster)  [unwired: 9 in]
        n741 = Unbundle By Name(w1008) -> ("Motion Module.Wear Track Diameter"=w1010:refnum<vi>)
        n742 = Unbundle By Name(w1008) -> ("PID.Ramp"=w1020:refnum<vi>)
        n743 = call "Encrypt file path creation.vi"("error in (no error)"=w1046) -> ("error out"=w1045:errorcluster, "File Path"=w1044:path)  [unwired: 9 in]
        n744 = property class="Bool (strict)"(reference=w1042, "Value"=FALSE) -> (reference out=w1040:refnum<vi>, error out=w1041:errorcluster)  [unwired: 1 in]
        n745 = property class="Bool (strict)"(reference=w1033, "Visible"=FALSE) -> (reference out=w1031:refnum<vi>, error out=w1032:errorcluster)  [unwired: 1 in]
        n746 = property class="Bool (strict)"(reference=w1036, "Visible"=FALSE) -> (reference out=w1038:refnum<vi>, error out=w1037:errorcluster)  [unwired: 1 in]
        n747 = property class="Bool (strict)"(reference=w1028, "Visible"=FALSE) -> (reference out=w1030:refnum<vi>, error out=w1029:errorcluster)  [unwired: 1 in]
        n748 = property class="Bool (strict)"(reference=w1020, "Value"=FALSE) -> (reference out=w1022:refnum<vi>, error out=w1021:errorcluster)  [unwired: 1 in]
        n749 = property class="DigNum (strict)"(reference=w1010, "Value"=0.0) -> (reference out=w1009:refnum<vi>, error out=w1011:errorcluster)  [unwired: 1 in]
        n750 = property class="Bool (strict)"(reference=w1016, "Visible"=FALSE, "DisabledEnum"=T13."Disabled and Grayed Out" ("Disabled")) -> (reference out=w1013:refnum<vi>, error out=w1015:errorcluster)  [unwired: 1 in]
        n751 = property class="Bool (strict)"(reference=w1023, "Visible"=FALSE ("Value")) -> (reference out=w1025:refnum<vi>, error out=w1024:errorcluster)  [unwired: 1 in]
        n752 = call "DATA ENCRYPT STRING FILE WRITE.vi"("file path (dialog if empty)"=w1044, "error in (no error)"=w1045, "User Action"="System Booted", "main ref"=w1008) -> ("error out"=w1047:errorcluster)  [unwired: 5 in, 1 out]
        n753 = Close Reference(reference=w1031, error in (no error)=w1032) -> ()  [unwired: 1 out]
        n754 = Close Reference(reference=w1038, error in (no error)=w1037) -> ()  [unwired: 1 out]
        n755 = Close Reference(reference=w1030, error in (no error)=w1029) -> ()  [unwired: 1 out]
        n756 = Close Reference(reference=w1022, error in (no error)=w1021) -> ()  [unwired: 1 out]
        n757 = Close Reference(reference=w1040, error in (no error)=w1041) -> ()  [unwired: 1 out]
        n758 = Close Reference(reference=w1009, error in (no error)=w1011) -> ()  [unwired: 1 out]
        n759 = Close Reference(reference=w1013, error in (no error)=w1015) -> ()  [unwired: 1 out]
        n760 = Close Reference(reference=w1025, error in (no error)=w1024) -> ()  [unwired: 1 out]
        n761 = call "Reinitial Parameter After Test.vi"("error in (no error)"=w1047, "main ref"=w1008) -> ("error out"=w1017:errorcluster)  [unwired: 9 in]
        n762 = local write "HEAVE ENABLE"(FALSE ("HEAVE ENABLE")) -> ()
      }
      frame "Init Other Loop" {
      }
      frame "Service Save" {
        n763 = call "Write Config Unitest.vi"("error in (no error)"=w1056, "main ref"=w1055) -> ("error out"=w1061:errorcluster)  [unwired: 9 in]
        n764 = call "Stall Data Flow.vim"("value in"=w1061, "milliseconds to wait"=u32 2000) -> ("value out"=w1060:errorcluster)  [unwired: 1 out]
        n765 = call "Read Config Unitest.vi"("error in (no error)"=w1060, "main ref"=w1055) -> ("error out"=w1058:errorcluster)  [unwired: 9 in]
        n766 = call "DATA ENCRYPT STRING FILE WRITE.vi"("error in (no error)"=w1058, "User Action"="Service Parameter Saved", "main ref"=w1055) -> ("error out"=w1057:errorcluster)  [unwired: 6 in, 1 out]
      }
      frame "HOME" {
        n767 = call "DATA ENCRYPT STRING FILE WRITE.vi"("error in (no error)"=w1077, "User Action"="User Pressed Home", "main ref"=w1063) -> ("error out"=w1073:errorcluster)  [unwired: 6 in, 1 out]
        n768 = Unbundle By Name(w1063) -> ("Main Home Screen.MainPage"=w1068:refnum<vi>)
        n769 = Unbundle By Name(w1063) -> ("Main Home Screen.Home"=w1076:refnum<vi>)
        n770 = Unbundle By Name(w1063) -> ("Main Home Screen.GUI"=w1066:refnum<vi>)
        n771 = property class="Bool (strict)"(reference=w1076, error in=w1073, "Value"=FALSE) -> (reference out=w1074:refnum<vi>, error out=w1075:errorcluster)
        n772 = property class="TabCtl (strict)"(reference=w1068, "Value"=T5."HOME") -> (reference out=w1070:refnum<vi>, error out=w1069:errorcluster)  [unwired: 1 in]
        n773 = property class="TabCtl (strict)"(reference=w1066, "Value"=T4."Setup") -> (reference out=w1064:refnum<vi>, error out=w1065:errorcluster)  [unwired: 1 in]
        n774 = Close Reference(reference=w1074, error in (no error)=w1075) -> (error out=w1072:errorcluster)
        n775 = Close Reference(reference=w1070, error in (no error)=w1069) -> ()  [unwired: 1 out]
        n776 = Close Reference(reference=w1064, error in (no error)=w1065) -> ()  [unwired: 1 out]
      }
      frame "Platform Setting" {
        n777 = call "DATA ENCRYPT STRING FILE WRITE.vi"("error in (no error)"=w1094, "User Action"="User Pressed Platform Setting", "main ref"=w1080) -> ("error out"=w1090:errorcluster)  [unwired: 6 in, 1 out]
        n778 = Unbundle By Name(w1080) -> ("Main Home Screen.Platform Settings"=w1093:refnum<vi>)
        n779 = Unbundle By Name(w1080) -> ("Main Home Screen.MainPage"=w1085:refnum<vi>)
        n780 = Unbundle By Name(w1080) -> ("Main Home Screen.GUI"=w1083:refnum<vi>)
        n781 = property class="TabCtl (strict)"(reference=w1085, "Value"=T5."PlatformSetting") -> (reference out=w1087:refnum<vi>, error out=w1086:errorcluster)  [unwired: 1 in]
        n782 = property class="TabCtl (strict)"(reference=w1083, "Value"=T4."Setup") -> (reference out=w1081:refnum<vi>, error out=w1082:errorcluster)  [unwired: 1 in]
        n783 = property class="Bool (strict)"(reference=w1093, error in=w1090, "Value"=FALSE) -> (reference out=w1091:refnum<vi>, error out=w1092:errorcluster)
        n784 = Close Reference(reference=w1087, error in (no error)=w1086) -> ()  [unwired: 1 out]
        n785 = Close Reference(reference=w1081, error in (no error)=w1082) -> ()  [unwired: 1 out]
        n786 = Close Reference(reference=w1091, error in (no error)=w1092) -> (error out=w1089:errorcluster)
      }
      frame "Configure" {
        n787 = call "DATA ENCRYPT STRING FILE WRITE.vi"("error in (no error)"=w1111, "User Action"="User Pressed Configure", "main ref"=w1097) -> ("error out"=w1107:errorcluster)  [unwired: 6 in, 1 out]
        n788 = Unbundle By Name(w1097) -> ("Main Home Screen.Configure"=w1110:refnum<vi>)
        n789 = Unbundle By Name(w1097) -> ("Main Home Screen.MainPage"=w1102:refnum<vi>)
        n790 = Unbundle By Name(w1097) -> ("Main Home Screen.GUI"=w1100:refnum<vi>)
        n791 = property class="Bool (strict)"(reference=w1110, error in=w1107, "Value"=FALSE) -> (reference out=w1108:refnum<vi>, error out=w1109:errorcluster)
        n792 = property class="TabCtl (strict)"(reference=w1102, "Value"=T5."Details") -> (reference out=w1104:refnum<vi>, error out=w1103:errorcluster)  [unwired: 1 in]
        n793 = property class="TabCtl (strict)"(reference=w1100, "Value"=T4."Setup") -> (reference out=w1098:refnum<vi>, error out=w1099:errorcluster)  [unwired: 1 in]
        n794 = Close Reference(reference=w1108, error in (no error)=w1109) -> (error out=w1106:errorcluster)
        n795 = Close Reference(reference=w1104, error in (no error)=w1103) -> ()  [unwired: 1 out]
        n796 = Close Reference(reference=w1098, error in (no error)=w1099) -> ()  [unwired: 1 out]
      }
      frame "Analysis" {
        n797 = call "DATA ENCRYPT STRING FILE WRITE.vi"("error in (no error)"=w1128, "User Action"="User Pressed Analysis", "main ref"=w1114) -> ("error out"=w1124:errorcluster)  [unwired: 6 in, 1 out]
        n798 = Unbundle By Name(w1114) -> ("Main Home Screen.MainPage"=w1119:refnum<vi>)
        n799 = Unbundle By Name(w1114) -> ("Main Home Screen.Analysis"=w1127:refnum<vi>)
        n800 = Unbundle By Name(w1114) -> ("Main Home Screen.GUI"=w1117:refnum<vi>)
        n801 = property class="Bool (strict)"(reference=w1127, error in=w1124, "Value"=FALSE) -> (reference out=w1125:refnum<vi>, error out=w1126:errorcluster)
        n802 = property class="TabCtl (strict)"(reference=w1119, "Value"=T5."Analysis") -> (reference out=w1121:refnum<vi>, error out=w1120:errorcluster)  [unwired: 1 in]
        n803 = property class="TabCtl (strict)"(reference=w1117, "Value"=T4."Setup") -> (reference out=w1115:refnum<vi>, error out=w1116:errorcluster)  [unwired: 1 in]
        n804 = Close Reference(reference=w1125, error in (no error)=w1126) -> (error out=w1123:errorcluster)
        n805 = Close Reference(reference=w1121, error in (no error)=w1120) -> ()  [unwired: 1 out]
        n806 = Close Reference(reference=w1115, error in (no error)=w1116) -> ()  [unwired: 1 out]
      }
      frame "service 2" {
        n807 = call "DATA ENCRYPT STRING FILE WRITE.vi"("error in (no error)"=w1149, "User Action"="User Pressed service", "main ref"=w1132) -> ("error out"=w1145:errorcluster)  [unwired: 6 in, 1 out]
        n808 = Unbundle By Name(w1132) -> ("Main Screen.Main Screen Tab"=w1133:refnum<vi>)
        n809 = Unbundle By Name(w1132) -> ("Main Home Screen.MainPage"=w1140:refnum<vi>)
        n810 = Unbundle By Name(w1132) -> ("Main Home Screen.Analysis"=w1148:refnum<vi>)
        n811 = Unbundle By Name(w1132) -> ("Main Home Screen.GUI"=w1138:refnum<vi>)
        n812 = property class="Bool (strict)"(reference=w1148, error in=w1145, "Value"=FALSE) -> (reference out=w1146:refnum<vi>, error out=w1147:errorcluster)
        n813 = property class="TabCtl (strict)"(reference=w1140, "Value"=T5."HOME") -> (reference out=w1142:refnum<vi>, error out=w1141:errorcluster)  [unwired: 1 in]
        n814 = property class="TabCtl (strict)"(reference=w1138, "Value"=T4."Begin") -> (reference out=w1136:refnum<vi>, error out=w1137:errorcluster)  [unwired: 1 in]
        n815 = property class="TabCtl (strict)"(reference=w1133, "Value"=T8."About") -> (reference out=w1130:refnum<vi>, error out=w1134:errorcluster)  [unwired: 1 in]
        n816 = Close Reference(reference=w1146, error in (no error)=w1147) -> (error out=w1144:errorcluster)
        n817 = Close Reference(reference=w1142, error in (no error)=w1141) -> ()  [unwired: 1 out]
        n818 = Close Reference(reference=w1136, error in (no error)=w1137) -> ()  [unwired: 1 out]
        n819 = Close Reference(reference=w1130, error in (no error)=w1134) -> ()  [unwired: 1 out]
      }
      frame "Auto" {
        n820 = call "DATA ENCRYPT STRING FILE WRITE.vi"("error in (no error)"=w1162, "User Action"="User Pressed Auto File Name", "main ref"=w1152) -> ("error out"=w1159:errorcluster)  [unwired: 6 in, 1 out]
        n821 = Get Date/Time In Seconds() -> (seconds since 1Jan1904=w1160:timestamp)
        n822 = Format Into String(format string="%<%I_%M_%S_%p_%d_%B_%Y>T", error in=w1159, w1160) -> (resulting string=w1153:string, error out=w1155:errorcluster)  [unwired: 1 in]
        n823 = local write "Auto"(FALSE ("Auto")) -> ()
        n824 = Unbundle By Name(w1152) -> ("Config Screen.FILE"=w1158:refnum<vi>)
        n825 = property class="Str"(reference=w1158, error in=w1155, "Value"=w1153) -> (reference out=w1156:refnum<vi>, error out=w1157:errorcluster)
        n826 = Close Reference(reference=w1156, error in (no error)=w1157) -> (error out=w1154:errorcluster)
      }
      frame "Select Load Head" {
        n827 = call "Reinitial Parameter.vi"("error in (no error)"=w1167, "Data Cluster"=w1164) -> ("error out"=w1166:errorcluster)  [unwired: 9 in]
        n828 = call "FILE NAME RECHECK.vi"("error in (no error)"=w1166, "main ref"=w1164) -> ("error out"=w1165:errorcluster)  [unwired: 9 in]
      }
      frame "com 3" {
        n829 = call "DATA ENCRYPT STRING FILE WRITE.vi"("error in (no error)"=w1171, "User Action"="User Pressed Check Load Communication", "main ref"=w1168) -> ("error out"=w1170:errorcluster)  [unwired: 6 in, 1 out]
        n830 = call "SET LOAD PARAMETERS.vi"("error in (no error)"=w1170, "main ref"=w1168) -> ("error out"=w1169:errorcluster)  [unwired: 9 in]
      }
      frame "ZeroAll" {
        n831 = call "DATA ENCRYPT STRING FILE WRITE.vi"("error in (no error)"=w1178, "User Action"="User Pressed Zero All", "main ref"=w1174) -> ("error out"=w1177:errorcluster)  [unwired: 6 in, 1 out]
        n832 = local write "ZeroAll"(FALSE ("ZeroAll")) -> ()
        n833 = call "LOAD CELL FGV MAIN.vi"("Enum"=T14."ZEROALL", "error in (no error)"=w1177, "main ref"=w1174) -> ("error IO"=w1176:errorcluster)  [unwired: 8 in]
      }
      frame "Loading Mode" {
        n834 = Unbundle By Name(w1182) -> ("Loading.Loading Mode"=w1184:refnum<vi>)
        n835 = property class="Ring (strict)"(reference=w1184, error in=w1183) -> (reference out=w1186:refnum<vi>, error out=w1185:errorcluster, "Value"=w1180:u16)
        n836 = Close Reference(reference=w1186, error in (no error)=w1185) -> (error out=w1181:errorcluster)
        n837 = case shown="1" w1180 {
          tunnel: [w1201 w1218 w1230 w1242] -> w1187
          tunnel: w1182 -> [w1188 w1204 w1222 w1234]
          tunnel: w1181 -> [w1202 w1217 w1229 w1241]
          frame 0, Default {
            n838 = Unbundle By Name(w1188) -> ("Loading.Enter the Loading Rate (N/min)"=w1195:refnum<vi>)
            n839 = Unbundle By Name(w1188) -> ("Loading.Load Selection"=w1198:refnum<vi>)
            n840 = Unbundle By Name(w1188) -> ("Loading.Enter the Final Load (N)"=w1190:refnum<vi>)
            n841 = property class="TabCtl (strict)"(reference=w1198, "Value"=T6."Constant") -> (reference out=w1200:refnum<vi>, error out=w1199:errorcluster)  [unwired: 1 in]
            n842 = property class="DigNum (strict)"(reference=w1195, "DisabledEnum"=T13."Disabled and Grayed Out" ("Disabled")) -> (reference out=w1194:refnum<vi>, error out=w1196:errorcluster)  [unwired: 1 in]
            n843 = property class="DigNum (strict)"(reference=w1190, "DisabledEnum"=T13."Disabled and Grayed Out" ("Disabled")) -> (reference out=w1191:refnum<vi>, error out=w1189:errorcluster)  [unwired: 1 in]
            n844 = call "DATA ENCRYPT STRING FILE WRITE.vi"("error in (no error)"=w1202, "User Action"="User selected Constant Mode", "main ref"=w1188) -> ("error out"=w1201:errorcluster)  [unwired: 6 in, 1 out]
            n845 = Close Reference(reference=w1200, error in (no error)=w1199) -> ()  [unwired: 1 out]
            n846 = Close Reference(reference=w1194, error in (no error)=w1196) -> ()  [unwired: 1 out]
            n847 = Close Reference(reference=w1191, error in (no error)=w1189) -> ()  [unwired: 1 out]
          }
          frame 1 {
            n848 = Unbundle By Name(w1204) -> ("Loading.Enter the Loading Rate (N/min)"=w1215:refnum<vi>)
            n849 = Unbundle By Name(w1204) -> ("Loading.Enter the Final Load (N)"=w1210:refnum<vi>)
            n850 = Unbundle By Name(w1204) -> ("Loading.Load Selection"=w1206:refnum<vi>)
            n851 = property class="TabCtl (strict)"(reference=w1206, "Value"=T6."Constant") -> (reference out=w1208:refnum<vi>, error out=w1207:errorcluster)  [unwired: 1 in]
            n852 = property class="DigNum (strict)"(reference=w1215, "DisabledEnum"=T13."Enabled" ("Disabled")) -> (reference out=w1214:refnum<vi>, error out=w1216:errorcluster)  [unwired: 1 in]
            n853 = property class="DigNum (strict)"(reference=w1210, "DisabledEnum"=T13."Enabled" ("Disabled")) -> (reference out=w1211:refnum<vi>, error out=w1209:errorcluster)  [unwired: 1 in]
            n854 = call "DATA ENCRYPT STRING FILE WRITE.vi"("error in (no error)"=w1217, "User Action"="User selected Ramp Mode", "main ref"=w1204) -> ("error out"=w1218:errorcluster)  [unwired: 6 in, 1 out]
            n855 = Close Reference(reference=w1208, error in (no error)=w1207) -> ()  [unwired: 1 out]
            n856 = Close Reference(reference=w1214, error in (no error)=w1216) -> ()  [unwired: 1 out]
            n857 = Close Reference(reference=w1211, error in (no error)=w1209) -> ()  [unwired: 1 out]
          }
          frame 2 {
            n858 = Unbundle By Name(w1222) -> ("Loading.Load Selection"=w1226:refnum<vi>)
            n859 = Unbundle By Name(w1222) -> ("Loading.Warning 2"=w1224:refnum<vi>)
            n860 = property class="TabCtl (strict)"(reference=w1226, "Value"=T6."Step") -> (reference out=w1228:refnum<vi>, error out=w1227:errorcluster)  [unwired: 1 in]
            n861 = property class="Bool (strict)"(reference=w1224, "Visible"=FALSE) -> (reference out=w1220:refnum<vi>, error out=w1223:errorcluster)  [unwired: 1 in]
            n862 = call "DATA ENCRYPT STRING FILE WRITE.vi"("error in (no error)"=w1229, "User Action"="User selected Step Mode", "main ref"=w1222) -> ("error out"=w1230:errorcluster)  [unwired: 6 in, 1 out]
            n863 = Close Reference(reference=w1228, error in (no error)=w1227) -> ()  [unwired: 1 out]
            n864 = Close Reference(reference=w1220, error in (no error)=w1223) -> ()  [unwired: 1 out]
          }
          frame 3 {
            n865 = Unbundle By Name(w1234) -> ("Loading.Load Selection"=w1238:refnum<vi>)
            n866 = Unbundle By Name(w1234) -> ("Loading.Warning 2"=w1236:refnum<vi>)
            n867 = property class="TabCtl (strict)"(reference=w1238, "Value"=T6."Indentation") -> (reference out=w1240:refnum<vi>, error out=w1239:errorcluster)  [unwired: 1 in]
            n868 = property class="Bool (strict)"(reference=w1236, "Visible"=FALSE) -> (reference out=w1232:refnum<vi>, error out=w1235:errorcluster)  [unwired: 1 in]
            n869 = call "DATA ENCRYPT STRING FILE WRITE.vi"("error in (no error)"=w1241, "User Action"="User selected Indentation Mode", "main ref"=w1234) -> ("error out"=w1242:errorcluster)  [unwired: 6 in, 1 out]
            n870 = Close Reference(reference=w1240, error in (no error)=w1239) -> ()  [unwired: 1 out]
            n871 = Close Reference(reference=w1232, error in (no error)=w1235) -> ()  [unwired: 1 out]
          }
        }
      }
      frame "SSP 0.3" {
        n872 = Unbundle By Name(w1246) -> ("Loading.SSP 0.3"=w1249:refnum<vi>)
        n873 = property class="Bool (strict)"(reference=w1249, error in=w1248) -> (reference out=w1251:refnum<vi>, error out=w1250:errorcluster, "Value"=w1247:bool)
        n874 = Close Reference(reference=w1251, error in (no error)=w1250) -> (error out=w1245:errorcluster)
        n875 = case shown="True" w1247 {
          tunnel: w1246 -> [_ w1253]
          tunnel: w1245 -> [w1252 w1261]
          tunnel: [w1252 w1260] -> w1244
          frame False {
          }
          frame True {
            w1263 = FALSE ("Value")
            n876 = Unbundle By Name(w1253) -> ("Loading.Enter the Load  (N)"=w1259:refnum<vi>)
            n877 = Unbundle By Name(w1253) -> ("Loading.SSP 0.75"=w1264:refnum<vi>)
            n878 = Unbundle By Name(w1253) -> ("Loading.SSP 0.5"=w1269:refnum<vi>)
            n879 = property class="Bool (strict)"(reference=w1264, "Value"=w1263) -> (reference out=w1266:refnum<vi>, error out=w1265:errorcluster)  [unwired: 1 in]
            n880 = property class="Bool (strict)"(reference=w1269, "Value"=w1263) -> (reference out=w1267:refnum<vi>, error out=w1268:errorcluster)  [unwired: 1 in]
            n881 = property class="DigNum (strict)"(reference=w1259, "Minimum"=2.0 ("Data Entry Limits:Minimum"), "Maximum"=50.0 ("Data Entry Limits:Maximum"), "Increment"=0.1 ("Data Entry Limits:Increment")) -> (reference out=w1257:refnum<vi>, error out=w1258:errorcluster)  [unwired: 1 in]
            n882 = call "DATA ENCRYPT STRING FILE WRITE.vi"("error in (no error)"=w1261, "User Action"="User selected 0.3 SSP", "main ref"=w1253) -> ("error out"=w1260:errorcluster)  [unwired: 6 in, 1 out]
            n883 = Close Reference(reference=w1266, error in (no error)=w1265) -> ()  [unwired: 1 out]
            n884 = Close Reference(reference=w1267, error in (no error)=w1268) -> ()  [unwired: 1 out]
            n885 = Close Reference(reference=w1257, error in (no error)=w1258) -> ()  [unwired: 1 out]
          }
        }
      }
      frame "SSP 0.5" {
        n886 = Unbundle By Name(w1272) -> ("Loading.SSP 0.5"=w1275:refnum<vi>)
        n887 = property class="Bool (strict)"(reference=w1275, error in=w1274) -> (reference out=w1277:refnum<vi>, error out=w1276:errorcluster, "Value"=w1273:bool)
        n888 = Close Reference(reference=w1277, error in (no error)=w1276) -> (error out=w1271:errorcluster)
        n889 = case shown="True" w1273 {
          tunnel: w1272 -> [_ w1279]
          tunnel: w1271 -> [w1278 w1287]
          tunnel: [w1278 w1286] -> w1270
          frame False {
          }
          frame True {
            w1289 = FALSE ("Value")
            n890 = Unbundle By Name(w1279) -> ("Loading.Enter the Load  (N)"=w1285:refnum<vi>)
            n891 = Unbundle By Name(w1279) -> ("Loading.SSP 0.75"=w1295:refnum<vi>)
            n892 = Unbundle By Name(w1279) -> ("Loading.SSP 0.3"=w1290:refnum<vi>)
            n893 = property class="Bool (strict)"(reference=w1290, "Value"=w1289) -> (reference out=w1292:refnum<vi>, error out=w1291:errorcluster)  [unwired: 1 in]
            n894 = property class="Bool (strict)"(reference=w1295, "Value"=w1289) -> (reference out=w1293:refnum<vi>, error out=w1294:errorcluster)  [unwired: 1 in]
            n895 = property class="DigNum (strict)"(reference=w1285, "Minimum"=2.0 ("Data Entry Limits:Minimum"), "Maximum"=200.0 ("Data Entry Limits:Maximum"), "Increment"=0.1 ("Data Entry Limits:Increment")) -> (reference out=w1283:refnum<vi>, error out=w1284:errorcluster)  [unwired: 1 in]
            n896 = call "DATA ENCRYPT STRING FILE WRITE.vi"("error in (no error)"=w1287, "User Action"="User selected 0.5 SSP", "main ref"=w1279) -> ("error out"=w1286:errorcluster)  [unwired: 6 in, 1 out]
            n897 = Close Reference(reference=w1292, error in (no error)=w1291) -> ()  [unwired: 1 out]
            n898 = Close Reference(reference=w1293, error in (no error)=w1294) -> ()  [unwired: 1 out]
            n899 = Close Reference(reference=w1283, error in (no error)=w1284) -> ()  [unwired: 1 out]
          }
        }
      }
      frame "SSP 0.75" {
        n900 = Unbundle By Name(w1298) -> ("Loading.SSP 0.75"=w1301:refnum<vi>)
        n901 = property class="Bool (strict)"(reference=w1301, error in=w1300) -> (reference out=w1303:refnum<vi>, error out=w1302:errorcluster, "Value"=w1299:bool)
        n902 = Close Reference(reference=w1303, error in (no error)=w1302) -> (error out=w1297:errorcluster)
        n903 = case shown="True" w1299 {
          tunnel: w1298 -> [_ w1305]
          tunnel: w1297 -> [w1304 w1313]
          tunnel: [w1304 w1312] -> w1296
          frame False {
          }
          frame True {
            w1315 = FALSE ("Value")
            n904 = Unbundle By Name(w1305) -> ("Loading.SSP 0.3"=w1316:refnum<vi>)
            n905 = Unbundle By Name(w1305) -> ("Loading.SSP 0.5"=w1321:refnum<vi>)
            n906 = Unbundle By Name(w1305) -> ("Loading.Enter the Load  (N)"=w1311:refnum<vi>)
            n907 = property class="Bool (strict)"(reference=w1316, "Value"=w1315) -> (reference out=w1318:refnum<vi>, error out=w1317:errorcluster)  [unwired: 1 in]
            n908 = property class="Bool (strict)"(reference=w1321, "Value"=w1315) -> (reference out=w1319:refnum<vi>, error out=w1320:errorcluster)  [unwired: 1 in]
            n909 = property class="DigNum (strict)"(reference=w1311, "Minimum"=200.0 ("Data Entry Limits:Minimum"), "Maximum"=500.0 ("Data Entry Limits:Maximum"), "Increment"=0.1 ("Data Entry Limits:Increment")) -> (reference out=w1309:refnum<vi>, error out=w1310:errorcluster)  [unwired: 1 in]
            n910 = call "DATA ENCRYPT STRING FILE WRITE.vi"("error in (no error)"=w1313, "User Action"="User selected 0.75 SSP", "main ref"=w1305) -> ("error out"=w1312:errorcluster)  [unwired: 6 in, 1 out]
            n911 = Close Reference(reference=w1318, error in (no error)=w1317) -> ()  [unwired: 1 out]
            n912 = Close Reference(reference=w1319, error in (no error)=w1320) -> ()  [unwired: 1 out]
            n913 = Close Reference(reference=w1309, error in (no error)=w1310) -> ()  [unwired: 1 out]
          }
        }
      }
      frame "LHBack" {
        # "Back to Configure"
        n914 = Unbundle By Name(w1323) -> ("Main Home Screen.GUI"=w1332:refnum<vi>)
        n915 = Unbundle By Name(w1323) -> ("Main Home Screen.MainPage"=w1328:refnum<vi>)
        n916 = Unbundle By Name(w1323) -> ("Loading.LHBack"=w1326:refnum<vi>)
        n917 = property class="TabCtl (strict)"(reference=w1328, "Value"=T5."HOME") -> (reference out=w1330:refnum<vi>, error out=w1329:errorcluster)  [unwired: 1 in]
        n918 = property class="Bool (strict)"(reference=w1326, "Value"=FALSE) -> (reference out=w1324:refnum<vi>, error out=w1325:errorcluster)  [unwired: 1 in]
        n919 = property class="TabCtl (strict)"(reference=w1332, "Value"=T4."Setup") -> (reference out=w1334:refnum<vi>, error out=w1333:errorcluster)  [unwired: 1 in]
        n920 = Close Reference(reference=w1330, error in (no error)=w1329) -> ()  [unwired: 1 out]
        n921 = Close Reference(reference=w1324, error in (no error)=w1325) -> ()  [unwired: 1 out]
        n922 = Close Reference(reference=w1334, error in (no error)=w1333) -> ()  [unwired: 1 out]
        n923 = call "DATA ENCRYPT STRING FILE WRITE.vi"("error in (no error)"=w1335, "User Action"="User selected Back to Configure", "main ref"=w1323) -> ("error out"=w1336:errorcluster)  [unwired: 6 in, 1 out]
      }
      frame "MMBack" {
        # "Back to Configure"
        n924 = Unbundle By Name(w1338) -> ("Motion Module.MMBack"=w1342:refnum<vi>)
        n925 = Unbundle By Name(w1338) -> ("Main Home Screen.GUI"=w1348:refnum<vi>)
        n926 = Unbundle By Name(w1338) -> ("Main Home Screen.MainPage"=w1344:refnum<vi>)
        n927 = property class="Bool (strict)"(reference=w1342, "Value"=FALSE) -> (reference out=w1340:refnum<vi>, error out=w1341:errorcluster)  [unwired: 1 in]
        n928 = property class="TabCtl (strict)"(reference=w1344, "Value"=T5."HOME") -> (reference out=w1346:refnum<vi>, error out=w1345:errorcluster)  [unwired: 1 in]
        n929 = property class="TabCtl (strict)"(reference=w1348, "Value"=T4."Load Head") -> (reference out=w1350:refnum<vi>, error out=w1349:errorcluster)  [unwired: 1 in]
        n930 = Close Reference(reference=w1340, error in (no error)=w1341) -> ()  [unwired: 1 out]
        n931 = Close Reference(reference=w1346, error in (no error)=w1345) -> ()  [unwired: 1 out]
        n932 = Close Reference(reference=w1350, error in (no error)=w1349) -> ()  [unwired: 1 out]
        n933 = call "DATA ENCRYPT STRING FILE WRITE.vi"("error in (no error)"=w1351, "User Action"="User selected Back to Load Selection", "main ref"=w1338) -> ("error out"=w1352:errorcluster)  [unwired: 6 in, 1 out]
      }
      frame "LHNext" {
        w1388 = FALSE ("Visible")
        n934 = Unbundle By Name(w1354) -> ("Motion Module.HomeRot"=w1394:refnum<vi>)
        n935 = Unbundle By Name(w1354) -> ("Motion Module.HomeScratch"=w1389:refnum<vi>)
        n936 = Unbundle By Name(w1354) -> ("Motion Module.PlaceModule"=w1387:refnum<vi>)
        n937 = Unbundle By Name(w1354) -> ("Motion Module.Motion Mode:"=w1380:refnum<vi>)
        n938 = Unbundle By Name(w1354) -> ("Motion Module.Motion Direction:  3"=w1379:refnum<vi>)
        n939 = Unbundle By Name(w1354) -> ("Motion Module.Wear Track Diameter (mm)"=w1373:refnum<vi>)
        n940 = Unbundle By Name(w1354) -> ("Motion Module.Set WTD"=w1370:refnum<vi>)
        n941 = Unbundle By Name(w1354) -> ("Motion Module.Rotary Module Selection"=w1364:refnum<vi>)
        n942 = call "DATA ENCRYPT STRING FILE WRITE.vi"("error in (no error)"=w1403, "User Action"="User selected Select Module", "main ref"=w1354) -> ("error out"=w1367:errorcluster)  [unwired: 6 in, 1 out]
        n943 = property class="TabCtl (strict)"(reference=w1364, "Visible"=FALSE) -> (reference out=w1363:refnum<vi>, error out=w1365:errorcluster)  [unwired: 1 in]
        n944 = property class="Bool (strict)"(reference=w1394, error in=w1367, "Visible"=w1388) -> (reference out=w1392:refnum<vi>, error out=w1393:errorcluster)
        n945 = property class="Bool (strict)"(reference=w1389, error in=w1367, "Visible"=w1388) -> (reference out=w1391:refnum<vi>, error out=w1390:errorcluster)
        n946 = property class="Bool (strict)"(reference=w1387, error in=w1367, "Visible"=TRUE) -> (reference out=w1385:refnum<vi>, error out=w1386:errorcluster)
        n947 = property class="Ring (strict)"(reference=w1380, error in=w1367, "Visible"=FALSE) -> (reference out=w1382:refnum<vi>, error out=w1381:errorcluster)
        n948 = property class="Ring (strict)"(reference=w1379, error in=w1367, "Visible"=FALSE) -> (reference out=w1376:refnum<vi>, error out=w1378:errorcluster)
        n949 = property class="DigNum (strict)"(reference=w1373, "Visible"=FALSE) -> (reference out=w1372:refnum<vi>, error out=w1374:errorcluster)  [unwired: 1 in]
        n950 = property class="Bool (strict)"(reference=w1370, "Visible"=FALSE) -> (reference out=w1371:refnum<vi>, error out=w1369:errorcluster)  [unwired: 1 in]
        n951 = Close Reference(reference=w1392, error in (no error)=w1393) -> ()  [unwired: 1 out]
        n952 = Close Reference(reference=w1391, error in (no error)=w1390) -> ()  [unwired: 1 out]
        n953 = Close Reference(reference=w1385, error in (no error)=w1386) -> ()  [unwired: 1 out]
        n954 = Close Reference(reference=w1382, error in (no error)=w1381) -> ()  [unwired: 1 out]
        n955 = Close Reference(reference=w1376, error in (no error)=w1378) -> ()  [unwired: 1 out]
        n956 = Close Reference(reference=w1372, error in (no error)=w1374) -> ()  [unwired: 1 out]
        n957 = Close Reference(reference=w1363, error in (no error)=w1365) -> ()  [unwired: 1 out]
        n958 = Close Reference(reference=w1371, error in (no error)=w1369) -> ()  [unwired: 1 out]
        n959 = Unbundle By Name(w1354) -> ("Motion Module.M3 Image"=w1362:refnum<vi>)
        n960 = Unbundle By Name(w1354) -> ("Main Home Screen.GUI"=w1400:refnum<vi>)
        n961 = Unbundle By Name(w1354) -> ("Main Home Screen.MainPage"=w1396:refnum<vi>)
        n962 = Unbundle By Name(w1354) -> ("Loading.LHNext"=w1358:refnum<vi>)
        n963 = property class="TabCtl (strict)"(reference=w1362, "Value"=enum32{"Page 1", "Page 2"}."Page 2") -> (reference out=w1360:refnum<vi>, error out=w1361:errorcluster)  [unwired: 1 in]
        n964 = property class="TabCtl (strict)"(reference=w1396, "Value"=T5."HOME") -> (reference out=w1398:refnum<vi>, error out=w1397:errorcluster)  [unwired: 1 in]
        n965 = property class="TabCtl (strict)"(reference=w1400, "Value"=T4."Motion Module") -> (reference out=w1402:refnum<vi>, error out=w1401:errorcluster)  [unwired: 1 in]
        n966 = property class="Bool (strict)"(reference=w1358, "Value"=FALSE ("Visible")) -> (reference out=w1355:refnum<vi>, error out=w1357:errorcluster)  [unwired: 1 in]
        n967 = Close Reference(reference=w1360, error in (no error)=w1361) -> ()  [unwired: 1 out]
        n968 = Close Reference(reference=w1355, error in (no error)=w1357) -> ()  [unwired: 1 out]
        n969 = Close Reference(reference=w1398, error in (no error)=w1397) -> ()  [unwired: 1 out]
        n970 = Close Reference(reference=w1402, error in (no error)=w1401) -> ()  [unwired: 1 out]
      }
      frame "Rot Ver" {
        n971 = call "Rotory Module Selection.vi"("error in (no error)"=w1407, "Data Cluster"=w1405) -> ("error out"=w1406:errorcluster)  [unwired: 9 in]
      }
      frame "Scratch" {
        n972 = call "Scratch Module Selection.vi"("error in (no error)"=w1410, "Data Cluster"=w1408) -> ("error out"=w1409:errorcluster)  [unwired: 9 in]
      }
      frame "Motion Mode:" {
        n973 = Unbundle By Name(w1411) -> ("Motion Module.Motion Mode:"=w1413:refnum<vi>)
        n974 = property class="Ring (strict)"(reference=w1413) -> (reference out=w1415:refnum<vi>, error out=w1414:errorcluster, "Value"=w1412:u16)  [unwired: 1 in]
        n975 = Close Reference(reference=w1415, error in (no error)=w1414) -> ()  [unwired: 1 out]
        n976 = case shown="3" w1412 {
          tunnel: w1417 -> [w1426 w1435 w1444 w1453]
          tunnel: [w1425 w1434 w1443 w1452] -> w1416
          tunnel: w1411 -> [w1424 w1433 w1442 w1451]
          tunnel: w1411 -> [w1419 w1428 w1437 w1446]
          frame 0, Default {
            n977 = Unbundle By Name(w1419) -> ("Motion Module.Rotary Module Selection"=w1420:refnum<vi>)
            n978 = property class="TabCtl (strict)"(reference=w1420, "Value"=T7."Uniform Rotation") -> (reference out=w1422:refnum<vi>, error out=w1421:errorcluster)  [unwired: 1 in]
            n979 = Close Reference(reference=w1422, error in (no error)=w1421) -> ()  [unwired: 1 out]
            n980 = call "DATA ENCRYPT STRING FILE WRITE.vi"("error in (no error)"=w1426, "User Action"="User Selected Uniform Rotation", "main ref"=w1424) -> ("error out"=w1425:errorcluster)  [unwired: 6 in, 1 out]
          }
          frame 1 {
            n981 = Unbundle By Name(w1428) -> ("Motion Module.Rotary Module Selection"=w1429:refnum<vi>)
            n982 = property class="TabCtl (strict)"(reference=w1429, "Value"=T7."Angular Oscillation") -> (reference out=w1431:refnum<vi>, error out=w1430:errorcluster)  [unwired: 1 in]
            n983 = Close Reference(reference=w1431, error in (no error)=w1430) -> ()  [unwired: 1 out]
            n984 = call "DATA ENCRYPT STRING FILE WRITE.vi"("error in (no error)"=w1435, "User Action"="User Selected Angular Oscillation", "main ref"=w1433) -> ("error out"=w1434:errorcluster)  [unwired: 6 in, 1 out]
          }
          frame 2 {
            n985 = Unbundle By Name(w1437) -> ("Motion Module.Rotary Module Selection"=w1438:refnum<vi>)
            n986 = property class="TabCtl (strict)"(reference=w1438, "Value"=T7."Speed Ramp") -> (reference out=w1440:refnum<vi>, error out=w1439:errorcluster)  [unwired: 1 in]
            n987 = Close Reference(reference=w1440, error in (no error)=w1439) -> ()  [unwired: 1 out]
            n988 = call "DATA ENCRYPT STRING FILE WRITE.vi"("error in (no error)"=w1444, "User Action"="User Selected Ramp Mode", "main ref"=w1442) -> ("error out"=w1443:errorcluster)  [unwired: 6 in, 1 out]
          }
          frame 3 {
            n989 = Unbundle By Name(w1446) -> ("Motion Module.Rotary Module Selection"=w1447:refnum<vi>)
            n990 = property class="TabCtl (strict)"(reference=w1447, "Value"=T7."Speed Step") -> (reference out=w1449:refnum<vi>, error out=w1448:errorcluster)  [unwired: 1 in]
            n991 = Close Reference(reference=w1449, error in (no error)=w1448) -> ()  [unwired: 1 out]
            n992 = call "DATA ENCRYPT STRING FILE WRITE.vi"("error in (no error)"=w1453, "User Action"="User Selected Step Mode", "main ref"=w1451) -> ("error out"=w1452:errorcluster)  [unwired: 6 in, 1 out]
          }
        }
      }
      frame "MMNext" {
        n993 = Unbundle By Name(w1454) -> ("Motion Module.MMNext"=w1458:refnum<vi>)
        n994 = Unbundle By Name(w1454) -> ("Motion Module.MMNext"=w1465:refnum<vi>)
        n995 = Unbundle By Name(w1454) -> ("Main Home Screen.GUI"=w1467:refnum<vi>)
        n996 = property class="Bool (strict)"(reference=w1458, "Value"=FALSE ("Visible")) -> (reference out=w1455:refnum<vi>, error out=w1457:errorcluster)  [unwired: 1 in]
        n997 = property class="TabCtl (strict)"(reference=w1467, "Value"=T4."Environment") -> (reference out=w1469:refnum<vi>, error out=w1468:errorcluster)  [unwired: 1 in]
        n998 = property class="Bool (strict)"(reference=w1465, "Value"=FALSE) -> (reference out=w1463:refnum<vi>, error out=w1464:errorcluster)  [unwired: 1 in]
        n999 = Close Reference(reference=w1455, error in (no error)=w1457) -> ()  [unwired: 1 out]
        n1000 = Close Reference(reference=w1463, error in (no error)=w1464) -> ()  [unwired: 1 out]
        n1001 = Close Reference(reference=w1469, error in (no error)=w1468) -> ()  [unwired: 1 out]
        n1002 = call "DATA ENCRYPT STRING FILE WRITE.vi"("error in (no error)"=w1460, "User Action"="User Selected SetUp Module", "main ref"=w1454) -> ("error out"=w1459:errorcluster)  [unwired: 6 in, 1 out]
      }
      frame "APBack" {
        n1003 = Unbundle By Name(w1470) -> ("Environmental control.APBack"=w1477:refnum<vi>)
        n1004 = Unbundle By Name(w1470) -> ("Main Home Screen.GUI"=w1479:refnum<vi>)
        n1005 = property class="TabCtl (strict)"(reference=w1479, "Value"=T4."Motion Module") -> (reference out=w1481:refnum<vi>, error out=w1480:errorcluster)  [unwired: 1 in]
        n1006 = property class="Bool (strict)"(reference=w1477, "Value"=FALSE) -> (reference out=w1475:refnum<vi>, error out=w1476:errorcluster)  [unwired: 1 in]
        n1007 = Close Reference(reference=w1475, error in (no error)=w1476) -> ()  [unwired: 1 out]
        n1008 = Close Reference(reference=w1481, error in (no error)=w1480) -> ()  [unwired: 1 out]
        n1009 = call "DATA ENCRYPT STRING FILE WRITE.vi"("error in (no error)"=w1472, "User Action"="User Selected Back to Module", "main ref"=w1470) -> ("error out"=w1471:errorcluster)  [unwired: 6 in, 1 out]
      }
      frame "SNext" {
        w1494 = FALSE ("Value")
        n1010 = Unbundle By Name(w1483) -> ("Main Screen.zNL 2"=w1486:refnum<vi>)
        n1011 = Unbundle By Name(w1483) -> ("Main Screen.Start Test"=w1497:refnum<vi>)
        n1012 = Unbundle By Name(w1483) -> ("Main Screen.STOP"=w1496:refnum<vi>)
        n1013 = Unbundle By Name(w1483) -> ("Environmental control.SNext"=w1506:refnum<vi>)
        n1014 = Unbundle By Name(w1483) -> ("Main Home Screen.GUI"=w1508:refnum<vi>)
        n1015 = Unbundle By Name(w1483) -> ("PID.Ramp"=w1489:refnum<vi>)
        n1016 = property class="Bool (strict)"(reference=w1486, "DisabledEnum"=T13."Enabled" ("Disabled")) -> (reference out=w1484:refnum<vi>, error out=w1485:errorcluster)  [unwired: 1 in]
        n1017 = property class="Bool (strict)"(reference=w1489, "Value"=FALSE) -> (reference out=w1487:refnum<vi>, error out=w1490:errorcluster)  [unwired: 1 in]
        n1018 = property class="Bool (strict)"(reference=w1497, "Visible"=TRUE ("Value"), "Value"=FALSE) -> (reference out=w1492:refnum<vi>, error out=w1498:errorcluster)  [unwired: 1 in]
        n1019 = property class="Bool (strict)"(reference=w1496, "Value"=w1494, "Visible"=w1494) -> (reference out=w1491:refnum<vi>, error out=w1495:errorcluster)  [unwired: 1 in]
        n1020 = property class="TabCtl (strict)"(reference=w1508, "Value"=T4."Begin") -> (reference out=w1510:refnum<vi>, error out=w1509:errorcluster)  [unwired: 1 in]
        n1021 = property class="Bool (strict)"(reference=w1506, "Value"=FALSE) -> (reference out=w1504:refnum<vi>, error out=w1505:errorcluster)  [unwired: 1 in]
        n1022 = Close Reference(reference=w1484, error in (no error)=w1485) -> ()  [unwired: 1 out]
        n1023 = Close Reference(reference=w1487, error in (no error)=w1490) -> ()  [unwired: 1 out]
        n1024 = Close Reference(reference=w1492, error in (no error)=w1498) -> ()  [unwired: 1 out]
        n1025 = Close Reference(reference=w1491, error in (no error)=w1495) -> ()  [unwired: 1 out]
        n1026 = Close Reference(reference=w1504, error in (no error)=w1505) -> ()  [unwired: 1 out]
        n1027 = Close Reference(reference=w1510, error in (no error)=w1509) -> ()  [unwired: 1 out]
        n1028 = call "DATA ENCRYPT STRING FILE WRITE.vi"("error in (no error)"=w1501, "User Action"="User Pressed Setup", "main ref"=w1483) -> ("error out"=w1500:errorcluster)  [unwired: 6 in, 1 out]
      }
      frame "Enable Platform" {
        n1029 = Unbundle By Name(w1513) -> ("Heave AND Surge.Sequence ID"=w1515:refnum<vi>)
        n1030 = Unbundle By Name(w1513) -> ("Heave AND Surge.Mode Command"=w1539:refnum<vi>)
        n1031 = Unbundle By Name(w1513) -> ("Heave AND Surge.Distance"=w1536:refnum<vi>)
        n1032 = Unbundle By Name(w1513) -> ("Heave AND Surge.SPEED"=w1533:refnum<vi>)
        n1033 = Unbundle By Name(w1513) -> ("Platform Settings.Enable Platform"=w1547:refnum<vi>)
        n1034 = property class="DigNum (strict)"(reference=w1515, "Value"=u16 0) -> (reference out=w1514:refnum<vi>, error out=w1516:errorcluster)  [unwired: 1 in]
        n1035 = property class="DigNum (strict)"(reference=w1536, error in=w1531, "Value"=sgl 0.0) -> (reference out=w1537:refnum<vi>, error out=w1535:errorcluster)
        n1036 = property class="DigNum (strict)"(reference=w1533, error in=w1531, "Value"=sgl 0.0) -> (reference out=w1534:refnum<vi>, error out=w1532:errorcluster)
        n1037 = property class="DigNum (strict)"(reference=w1539, error in=w1531, "Value"=u8 1) -> (reference out=w1538:refnum<vi>, error out=w1540:errorcluster)
        n1038 = property class="Bool (strict)"(reference=w1547, "Value"=FALSE) -> (reference out=w1545:refnum<vi>, error out=w1546:errorcluster)  [unwired: 1 in]
        n1039 = Close Reference(reference=w1514, error in (no error)=w1516) -> (error out=w1512:errorcluster)
        n1040 = Close Reference(reference=w1537, error in (no error)=w1535) -> (error out=w1528:errorcluster)
        n1041 = Close Reference(reference=w1534, error in (no error)=w1532) -> (error out=w1527:errorcluster)
        n1042 = Close Reference(reference=w1538, error in (no error)=w1540) -> (error out=w1529:errorcluster)
        n1043 = Close Reference(reference=w1545, error in (no error)=w1546) -> ()  [unwired: 1 out]
        n1044 = Merge Errors(w1531, w1529, w1528, w1527, w1512) -> (w1530:errorcluster)
        n1045 = call "DATA ENCRYPT STRING FILE WRITE.vi"("error in (no error)"=w1530, "User Action"="User Pressed Enable Platform", "main ref"=w1513) -> ("error out"=w1542:errorcluster)  [unwired: 6 in, 1 out]
        n1046 = call "HEAVE WRITE FGV.vi"("Enum - Menu"=Heave_Write_enum."WRITE", "error in (no error)"=w1542, "main ref"=w1513) -> ("error out"=w1519:errorcluster)  [unwired: 8 in]
        n1047 = Unbundle By Name(w1513) -> ("Heave AND Surge.Read Heave Temp"=w1523:refnum<vi>)
        n1048 = property class="Bool (strict)"(reference=w1523, error in=w1519, "Value"=TRUE) -> (reference out=w1521:refnum<vi>, error out=w1522:errorcluster)
        n1049 = Close Reference(reference=w1521, error in (no error)=w1522) -> (error out=w1518:errorcluster)
        "HEAVE ENABLE" <- TRUE ("HEAVE ENABLE")
      }
      frame "Heave Up main" {
        n1050 = Unbundle By Name(w1548) -> ("Platform Settings.Heave Up main"=w1558:refnum<vi>)
        n1051 = call "Heave Up Main.vi"("error in (no error)"=w1550, "main ref"=w1548) -> ("error out"=w1549:errorcluster)  [unwired: 9 in]
        n1052 = property class="Bool (strict)"(reference=w1558, "Value"=FALSE) -> (reference out=w1556:refnum<vi>, error out=w1557:errorcluster)  [unwired: 1 in]
        n1053 = Close Reference(reference=w1556, error in (no error)=w1557) -> ()  [unwired: 1 out]
        n1054 = call "DATA ENCRYPT STRING FILE WRITE.vi"("error in (no error)"=w1549, "User Action"="User Pressed Heave UP", "main ref"=w1548) -> ("error out"=w1553:errorcluster)  [unwired: 6 in, 1 out]
        n1055 = call "HEAVE WRITE FGV.vi"("Enum - Menu"=Heave_Write_enum."WRITE", "error in (no error)"=w1553, "main ref"=w1548) -> ("error out"=w1552:errorcluster)  [unwired: 8 in]
      }
      frame "Heave Up MM" {
        n1056 = Unbundle By Name(w1559) -> ("Motion Module.Heave Up MM"=w1569:refnum<vi>)
        n1057 = call "Heave Up Motion Module.vi"("error in (no error)"=w1561, "main ref"=w1559) -> ("error out"=w1560:errorcluster)  [unwired: 9 in]
        n1058 = property class="Bool (strict)"(reference=w1569, "Value"=FALSE) -> (reference out=w1567:refnum<vi>, error out=w1568:errorcluster)  [unwired: 1 in]
        n1059 = Close Reference(reference=w1567, error in (no error)=w1568) -> ()  [unwired: 1 out]
        n1060 = call "DATA ENCRYPT STRING FILE WRITE.vi"("error in (no error)"=w1560, "User Action"="User Pressed Heave UP in Motion Module", "main ref"=w1559) -> ("error out"=w1564:errorcluster)  [unwired: 6 in, 1 out]
        n1061 = call "HEAVE WRITE FGV.vi"("Enum - Menu"=Heave_Write_enum."WRITE", "error in (no error)"=w1564, "main ref"=w1559) -> ("error out"=w1563:errorcluster)  [unwired: 8 in]
      }
      frame "Heave Down Main" {
        n1062 = call "Heave Down Main.vi"("error in (no error)"=w1572, "main ref"=w1570) -> ("error out"=w1571:errorcluster)  [unwired: 9 in]
        n1063 = Unbundle By Name(w1570) -> ("Platform Settings.Heave Down Main"=w1580:refnum<vi>)
        n1064 = property class="Bool (strict)"(reference=w1580, "Value"=FALSE) -> (reference out=w1578:refnum<vi>, error out=w1579:errorcluster)  [unwired: 1 in]
        n1065 = Close Reference(reference=w1578, error in (no error)=w1579) -> ()  [unwired: 1 out]
        n1066 = call "DATA ENCRYPT STRING FILE WRITE.vi"("error in (no error)"=w1571, "User Action"="User Pressed Heave DOWN", "main ref"=w1570) -> ("error out"=w1575:errorcluster)  [unwired: 6 in, 1 out]
        n1067 = call "HEAVE WRITE FGV.vi"("Enum - Menu"=Heave_Write_enum."WRITE", "error in (no error)"=w1575, "main ref"=w1570) -> ("error out"=w1574:errorcluster)  [unwired: 8 in]
      }
      frame "Heave Down MM" {
        n1068 = call "Heave Down Motion Module.vi"("error in (no error)"=w1583, "main ref"=w1581) -> ("error out"=w1582:errorcluster)  [unwired: 9 in]
        n1069 = Unbundle By Name(w1581) -> ("Motion Module.Heave Down MM"=w1591:refnum<vi>)
        n1070 = property class="Bool (strict)"(reference=w1591, "Value"=FALSE) -> (reference out=w1589:refnum<vi>, error out=w1590:errorcluster)  [unwired: 1 in]
        n1071 = Close Reference(reference=w1589, error in (no error)=w1590) -> ()  [unwired: 1 out]
        n1072 = call "DATA ENCRYPT STRING FILE WRITE.vi"("error in (no error)"=w1582, "User Action"="User Pressed Heave DOWN in Motion Module", "main ref"=w1581) -> ("error out"=w1586:errorcluster)  [unwired: 6 in, 1 out]
        n1073 = call "HEAVE WRITE FGV.vi"("Enum - Menu"=Heave_Write_enum."WRITE", "error in (no error)"=w1586, "main ref"=w1581) -> ("error out"=w1585:errorcluster)  [unwired: 8 in]
      }
      frame "Surge Backward Main" {
        n1074 = Unbundle By Name(w1592) -> ("Platform Settings.Surge Backward Main"=w1602:refnum<vi>)
        n1075 = call "Surge Backward Main.vi"("error in (no error)"=w1594, "main ref"=w1592) -> ("error out"=w1593:errorcluster)  [unwired: 9 in]
        n1076 = property class="Bool (strict)"(reference=w1602, "Value"=FALSE) -> (reference out=w1600:refnum<vi>, error out=w1601:errorcluster)  [unwired: 1 in]
        n1077 = Close Reference(reference=w1600, error in (no error)=w1601) -> ()  [unwired: 1 out]
        n1078 = call "DATA ENCRYPT STRING FILE WRITE.vi"("error in (no error)"=w1593, "User Action"="User Pressed Surge Backward", "main ref"=w1592) -> ("error out"=w1597:errorcluster)  [unwired: 6 in, 1 out]
        n1079 = call "HEAVE WRITE FGV.vi"("Enum - Menu"=Heave_Write_enum."WRITE", "error in (no error)"=w1597, "main ref"=w1592) -> ("error out"=w1596:errorcluster)  [unwired: 8 in]
      }
      frame "Surge Backward MM" {
        n1080 = Unbundle By Name(w1603) -> ("Motion Module.Surge Backward MM"=w1613:refnum<vi>)
        n1081 = call "Surge Backward Main.vi"("error in (no error)"=w1605, "main ref"=w1603) -> ("error out"=w1604:errorcluster)  [unwired: 9 in]
        n1082 = property class="Bool (strict)"(reference=w1613, "Value"=FALSE) -> (reference out=w1611:refnum<vi>, error out=w1612:errorcluster)  [unwired: 1 in]
        n1083 = Close Reference(reference=w1611, error in (no error)=w1612) -> ()  [unwired: 1 out]
        n1084 = call "DATA ENCRYPT STRING FILE WRITE.vi"("error in (no error)"=w1604, "User Action"="User Pressed Surge Backward in Motion Module", "main ref"=w1603) -> ("error out"=w1608:errorcluster)  [unwired: 6 in, 1 out]
        n1085 = call "HEAVE WRITE FGV.vi"("Enum - Menu"=Heave_Write_enum."WRITE", "error in (no error)"=w1608, "main ref"=w1603) -> ("error out"=w1607:errorcluster)  [unwired: 8 in]
      }
      frame "Surge Forward Main" {
        n1086 = Unbundle By Name(w1614) -> ("Platform Settings.Surge Forward Main"=w1624:refnum<vi>)
        n1087 = call "Surge Forward Main.vi"("error in (no error)"=w1616, "main ref"=w1614) -> ("error out"=w1615:errorcluster)  [unwired: 9 in]
        n1088 = property class="Bool (strict)"(reference=w1624, "Value"=FALSE) -> (reference out=w1622:refnum<vi>, error out=w1623:errorcluster)  [unwired: 1 in]
        n1089 = Close Reference(reference=w1622, error in (no error)=w1623) -> ()  [unwired: 1 out]
        n1090 = call "DATA ENCRYPT STRING FILE WRITE.vi"("error in (no error)"=w1615, "User Action"="User Pressed Surge Forward", "main ref"=w1614) -> ("error out"=w1619:errorcluster)  [unwired: 6 in, 1 out]
        n1091 = call "HEAVE WRITE FGV.vi"("Enum - Menu"=Heave_Write_enum."WRITE", "error in (no error)"=w1619, "main ref"=w1614) -> ("error out"=w1618:errorcluster)  [unwired: 8 in]
      }
      frame "Surge Forward MM" {
        n1092 = Unbundle By Name(w1625) -> ("Motion Module.Surge Forward MM"=w1635:refnum<vi>)
        n1093 = call "Surge Forward MM.vi"("error in (no error)"=w1627, "main ref"=w1625) -> ("error out"=w1626:errorcluster)  [unwired: 9 in]
        n1094 = property class="Bool (strict)"(reference=w1635, "Value"=FALSE) -> (reference out=w1633:refnum<vi>, error out=w1634:errorcluster)  [unwired: 1 in]
        n1095 = Close Reference(reference=w1633, error in (no error)=w1634) -> ()  [unwired: 1 out]
        n1096 = call "DATA ENCRYPT STRING FILE WRITE.vi"("error in (no error)"=w1626, "User Action"="User Pressed Surge Forward in Motion Module", "main ref"=w1625) -> ("error out"=w1630:errorcluster)  [unwired: 6 in, 1 out]
        n1097 = call "HEAVE WRITE FGV.vi"("Enum - Menu"=Heave_Write_enum."WRITE", "error in (no error)"=w1630, "main ref"=w1625) -> ("error out"=w1629:errorcluster)  [unwired: 8 in]
      }
      frame "Sway Left Main" {
        n1098 = call "Sway Left Main.vi"("error in (no error)"=w1639, "main ref"=w1637) -> ("error out"=w1638:errorcluster)  [unwired: 9 in]
        n1099 = Unbundle By Name(w1637) -> ("Platform Settings.Sway Left Main"=w1646:refnum<vi>)
        n1100 = property class="Bool (strict)"(reference=w1646, "Value"=FALSE) -> (reference out=w1644:refnum<vi>, error out=w1645:errorcluster)  [unwired: 1 in]
        n1101 = Close Reference(reference=w1644, error in (no error)=w1645) -> ()  [unwired: 1 out]
        n1102 = call "DATA ENCRYPT STRING FILE WRITE.vi"("error in (no error)"=w1638, "User Action"="User Pressed Sway Left ", "main ref"=w1637) -> ("error out"=w1641:errorcluster)  [unwired: 6 in, 1 out]
        n1103 = call "SWAY WRITE FGV.vi"("Enum - Menu"=Sway_Write_enum."WRITE", "error in (no error)"=w1641, "main ref"=w1637) -> ("error out"=w1640:errorcluster)  [unwired: 8 in]
      }
      frame "Sway Left MM" {
        n1104 = call "Sway Left MM.vi"("error in (no error)"=w1650, "main ref"=w1648) -> ("error out"=w1649:errorcluster)  [unwired: 9 in]
        n1105 = Unbundle By Name(w1648) -> ("Motion Module.Sway Left MM"=w1657:refnum<vi>)
        n1106 = property class="Bool (strict)"(reference=w1657, "Value"=FALSE) -> (reference out=w1655:refnum<vi>, error out=w1656:errorcluster)  [unwired: 1 in]
        n1107 = Close Reference(reference=w1655, error in (no error)=w1656) -> ()  [unwired: 1 out]
        n1108 = call "DATA ENCRYPT STRING FILE WRITE.vi"("error in (no error)"=w1649, "User Action"="User Pressed Sway Left in MM", "main ref"=w1648) -> ("error out"=w1652:errorcluster)  [unwired: 6 in, 1 out]
        n1109 = call "SWAY WRITE FGV.vi"("Enum - Menu"=Sway_Write_enum."WRITE", "error in (no error)"=w1652, "main ref"=w1648) -> ("error out"=w1651:errorcluster)  [unwired: 8 in]
      }
      frame "Sway Right MM" {
        n1110 = call "Sway Right MM.vi"("error in (no error)"=w1661, "main ref"=w1659) -> ("error out"=w1660:errorcluster)  [unwired: 9 in]
        n1111 = Unbundle By Name(w1659) -> ("Motion Module.Sway Right MM"=w1668:refnum<vi>)
        n1112 = property class="Bool (strict)"(reference=w1668, "Value"=FALSE) -> (reference out=w1666:refnum<vi>, error out=w1667:errorcluster)  [unwired: 1 in]
        n1113 = Close Reference(reference=w1666, error in (no error)=w1667) -> ()  [unwired: 1 out]
        n1114 = call "DATA ENCRYPT STRING FILE WRITE.vi"("error in (no error)"=w1660, "User Action"="User Pressed Sway Right in MM", "main ref"=w1659) -> ("error out"=w1663:errorcluster)  [unwired: 6 in, 1 out]
        n1115 = call "SWAY WRITE FGV.vi"("Enum - Menu"=Sway_Write_enum."WRITE", "error in (no error)"=w1663, "main ref"=w1659) -> ("error out"=w1662:errorcluster)  [unwired: 8 in]
      }
      frame "Sway Right Main" {
        n1116 = call "Sway Right Main.vi"("error in (no error)"=w1672, "main ref"=w1670) -> ("error out"=w1671:errorcluster)  [unwired: 9 in]
        n1117 = Unbundle By Name(w1670) -> ("Platform Settings.Sway Right Main"=w1679:refnum<vi>)
        n1118 = property class="Bool (strict)"(reference=w1679, "Value"=FALSE) -> (reference out=w1677:refnum<vi>, error out=w1678:errorcluster)  [unwired: 1 in]
        n1119 = Close Reference(reference=w1677, error in (no error)=w1678) -> ()  [unwired: 1 out]
        n1120 = call "DATA ENCRYPT STRING FILE WRITE.vi"("error in (no error)"=w1671, "User Action"="User Pressed Sway Right", "main ref"=w1670) -> ("error out"=w1674:errorcluster)  [unwired: 6 in, 1 out]
        n1121 = call "SWAY WRITE FGV.vi"("Enum - Menu"=Sway_Write_enum."WRITE", "error in (no error)"=w1674, "main ref"=w1670) -> ("error out"=w1673:errorcluster)  [unwired: 8 in]
      }
      frame "Manual Write Heave & Surge" {
        n1122 = Unbundle By Name(w1680) -> ("Heave AND Surge.Manual Write"=w1689:refnum<vi>)
        n1123 = property class="Bool (strict)"(reference=w1689, "Value"=FALSE) -> (reference out=w1687:refnum<vi>, error out=w1688:errorcluster)  [unwired: 1 in]
        n1124 = Close Reference(reference=w1687, error in (no error)=w1688) -> ()  [unwired: 1 out]
        n1125 = call "DATA ENCRYPT STRING FILE WRITE.vi"("error in (no error)"=w1681, "User Action"="User Pressed Manual Write Heave and Surge", "main ref"=w1680) -> ("error out"=w1684:errorcluster)  [unwired: 6 in, 1 out]
        n1126 = call "HEAVE WRITE FGV.vi"("Enum - Menu"=Heave_Write_enum."WRITE", "error in (no error)"=w1684, "main ref"=w1680) -> ("error out"=w1683:errorcluster)  [unwired: 8 in]
      }
      frame "Manual Write SWAY" {
        n1127 = Unbundle By Name(w1691) -> ("SWAY.Manual Write SWAY"=w1699:refnum<vi>)
        n1128 = property class="Bool (strict)"(reference=w1699, "Value"=FALSE) -> (reference out=w1697:refnum<vi>, error out=w1698:errorcluster)  [unwired: 1 in]
        n1129 = Close Reference(reference=w1697, error in (no error)=w1698) -> ()  [unwired: 1 out]
        n1130 = call "DATA ENCRYPT STRING FILE WRITE.vi"("error in (no error)"=w1692, "User Action"="User Pressed Manual Write Sway", "main ref"=w1691) -> ("error out"=w1694:errorcluster)  [unwired: 6 in, 1 out]
        n1131 = call "SWAY WRITE FGV.vi"("Enum - Menu"=Sway_Write_enum."WRITE", "error in (no error)"=w1694, "main ref"=w1691) -> ("error out"=w1693:errorcluster)  [unwired: 8 in]
      }
      frame "Load En" {
        # "zNL 2"
        n1132 = Unbundle By Name(w1701) -> ("Main Screen.Load En"=w1706:refnum<vi>)
        n1133 = property class="Bool (strict)"(reference=w1706) -> (reference out=w1704:refnum<vi>, error out=w1705:errorcluster, "Value"=w1700:bool)  [unwired: 1 in]
        n1134 = Close Reference(reference=w1704, error in (no error)=w1705) -> ()  [unwired: 1 out]
        n1135 = case shown="False" w1700 {
          tunnel: [w1718 w1728] -> w1702
          tunnel: w1703 -> [w1720 w1727]
          tunnel: w1701 -> [w1708 w1722]
          tunnel: w1701 -> [w1716 _]
          tunnel: w1701 -> [w1715 _]
          frame False {
            n1136 = call "DATA ENCRYPT STRING FILE WRITE.vi"("error in (no error)"=w1720, "User Action"="User Pressed UnLoad on Main Screen", "main ref"=w1708) -> ("error out"=w1709:errorcluster)  [unwired: 6 in, 1 out]
            n1137 = call "Stall Data Flow.vim"("value in"=w1709, "milliseconds to wait"=u32 2000) -> ("value out"=w1714:errorcluster)  [unwired: 1 out]
            n1138 = Unbundle By Name(w1708) -> ("Main Screen.zNL 2"=w1712:refnum<vi>)
            n1139 = property class="Bool (strict)"(reference=w1712, "DisabledEnum"=T13."Enabled" ("Disabled")) -> (reference out=w1710:refnum<vi>, error out=w1711:errorcluster)  [unwired: 1 in]
            n1140 = call "PID UNLOAD.vi"("error in (no error)"=w1714, "main ref"=w1715) -> ("error out"=w1717:errorcluster)  [unwired: 9 in]
            n1141 = Close Reference(reference=w1710, error in (no error)=w1711) -> ()  [unwired: 1 out]
            n1142 = call "HEAVE WRITE FGV.vi"("Enum - Menu"=Heave_Write_enum."WRITE", "error in (no error)"=w1717, "main ref"=w1716) -> ("error out"=w1718:errorcluster)  [unwired: 8 in]
          }
          frame True {
            n1143 = call "DATA ENCRYPT STRING FILE WRITE.vi"("error in (no error)"=w1727, "User Action"="User Pressed Load on Main Screen", "main ref"=w1722) -> ("error out"=w1728:errorcluster)  [unwired: 6 in, 1 out]
            n1144 = Unbundle By Name(w1722) -> ("Main Screen.zNL 2"=w1726:refnum<vi>)
            n1145 = property class="Bool (strict)"(reference=w1726, "DisabledEnum"=T13."Disabled and Grayed Out" ("Disabled")) -> (reference out=w1724:refnum<vi>, error out=w1725:errorcluster)  [unwired: 1 in]
            n1146 = Close Reference(reference=w1724, error in (no error)=w1725) -> ()  [unwired: 1 out]
          }
        }
      }
      frame "apply load" {
        n1147 = Unbundle By Name(w1731) -> ("Main Screen.Load En"=w1736:refnum<vi>)
        n1148 = property class="Bool (strict)"(reference=w1736) -> (reference out=w1734:refnum<vi>, error out=w1735:errorcluster, "Value"=w1730:bool)  [unwired: 1 in]
        n1149 = Close Reference(reference=w1734, error in (no error)=w1735) -> ()  [unwired: 1 out]
        n1150 = case shown="False" w1730 {
          tunnel: [w1743 w1750] -> w1732
          tunnel: w1733 -> [w1746 w1749]
          tunnel: w1731 -> [w1745 w1748]
          tunnel: w1731 -> [w1740 _]
          tunnel: w1731 -> [w1739 _]
          frame False {
            n1151 = call "DATA ENCRYPT STRING FILE WRITE.vi"("error in (no error)"=w1746, "User Action"="User Pressed UnLoad on Service Screen", "main ref"=w1745) -> ("error out"=w1742:errorcluster)  [unwired: 6 in, 1 out]
            n1152 = call "Stall Data Flow.vim"("value in"=w1742, "milliseconds to wait"=u32 2000) -> ("value out"=w1738:errorcluster)  [unwired: 1 out]
            n1153 = call "PID UNLOAD.vi"("error in (no error)"=w1738, "main ref"=w1739) -> ("error out"=w1741:errorcluster)  [unwired: 9 in]
            n1154 = call "HEAVE WRITE FGV.vi"("Enum - Menu"=Heave_Write_enum."WRITE", "error in (no error)"=w1741, "main ref"=w1740) -> ("error out"=w1743:errorcluster)  [unwired: 8 in]
          }
          frame True {
            n1155 = call "DATA ENCRYPT STRING FILE WRITE.vi"("error in (no error)"=w1749, "User Action"="User Pressed Load on Service Screen", "main ref"=w1748) -> ("error out"=w1750:errorcluster)  [unwired: 6 in, 1 out]
          }
        }
      }
      frame "BACK" {
        w1757 = FALSE ("Value")
        n1156 = Unbundle By Name(w1752) -> ("Main Screen.BACK"=w1777:refnum<vi>)
        n1157 = property class="Bool (strict)"(reference=w1777, "Value"=FALSE) -> (reference out=w1775:refnum<vi>, error out=w1776:errorcluster)  [unwired: 1 in]
        n1158 = Close Reference(reference=w1775, error in (no error)=w1776) -> ()  [unwired: 1 out]
        n1159 = call "DATA ENCRYPT STRING FILE WRITE.vi"("error in (no error)"=w1774, "User Action"="User Pressed Back on Main Screen", "main ref"=w1752) -> ("error out"=w1772:errorcluster)  [unwired: 6 in, 1 out]
        n1160 = Unbundle By Name(w1752) -> ("Main Home Screen.MainPage"=w1764:refnum<vi>)
        n1161 = Unbundle By Name(w1752) -> ("Main Screen.Start Test"=w1760:refnum<vi>)
        n1162 = Unbundle By Name(w1752) -> ("Main Screen.STOP"=w1759:refnum<vi>)
        n1163 = Unbundle By Name(w1752) -> ("Main Home Screen.GUI"=w1768:refnum<vi>)
        n1164 = property class="TabCtl (strict)"(reference=w1764, "Value"=T5."HOME") -> (reference out=w1766:refnum<vi>, error out=w1765:errorcluster)  [unwired: 1 in]
        n1165 = property class="TabCtl (strict)"(reference=w1768, "Value"=T4."Setup") -> (reference out=w1770:refnum<vi>, error out=w1769:errorcluster)  [unwired: 1 in]
        n1166 = property class="Bool (strict)"(reference=w1760, "Visible"=TRUE ("Value"), "Value"=FALSE) -> (reference out=w1755:refnum<vi>, error out=w1761:errorcluster)  [unwired: 1 in]
        n1167 = property class="Bool (strict)"(reference=w1759, "Value"=w1757, "Visible"=w1757) -> (reference out=w1754:refnum<vi>, error out=w1758:errorcluster)  [unwired: 1 in]
        n1168 = Close Reference(reference=w1770, error in (no error)=w1769) -> ()  [unwired: 1 out]
        n1169 = Close Reference(reference=w1766, error in (no error)=w1765) -> ()  [unwired: 1 out]
        n1170 = Close Reference(reference=w1755, error in (no error)=w1761) -> ()  [unwired: 1 out]
        n1171 = Close Reference(reference=w1754, error in (no error)=w1758) -> ()  [unwired: 1 out]
        n1172 = call "Reinitial Parameter After Test.vi"("error in (no error)"=w1772, "main ref"=w1752) -> ("error out"=w1753:errorcluster)  [unwired: 9 in]
      }
      frame "Start Test" {
        n1173 = call "Test Start Sequence.vi"("error in (no error)"=w1780, "Data Cluster"=w1778) -> ("error out"=w1779:errorcluster)  [unwired: 9 in]
      }
      frame "STOP" {
        n1174 = Unbundle By Name(w1782) -> ("Main Screen.Load En"=w1795:refnum<vi>)
        n1175 = Unbundle By Name(w1782) -> ("Main Screen.CZ FF"=w1790:refnum<vi>)
        n1176 = Unbundle By Name(w1782) -> ("Main Screen.zFF"=w1787:refnum<vi>)
        n1177 = property class="Bool (strict)"(reference=w1795, "DisabledEnum"=T13."Disabled and Grayed Out" ("Disabled")) -> (reference out=w1783:refnum<vi>, error out=w1794:errorcluster)  [unwired: 1 in]
        n1178 = property class="Bool (strict)"(reference=w1790, "DisabledEnum"=T13."Disabled and Grayed Out" ("Disabled"), "Value"=FALSE ("Visible")) -> (reference out=w1789:refnum<vi>, error out=w1791:errorcluster)  [unwired: 1 in]
        n1179 = property class="Bool (strict)"(reference=w1787, "DisabledEnum"=T13."Disabled and Grayed Out" ("Disabled"), "Value"=FALSE ("Visible")) -> (reference out=w1788:refnum<vi>, error out=w1786:errorcluster)  [unwired: 1 in]
        n1180 = Close Reference(reference=w1783, error in (no error)=w1794) -> ()  [unwired: 1 out]
        n1181 = Close Reference(reference=w1789, error in (no error)=w1791) -> ()  [unwired: 1 out]
        n1182 = Close Reference(reference=w1788, error in (no error)=w1786) -> ()  [unwired: 1 out]
        n1183 = call "Test Stop.vi"("error in (no error)"=w1796, "Data Cluster"=w1782) -> ("error out"=w1797:errorcluster)  [unwired: 9 in]
      }
      frame "PlaceModule" {
        n1184 = call "Place Module.vi"("error in (no error)"=w1800, "main ref"=w1798) -> ("error out"=w1799:errorcluster)  [unwired: 9 in]
      }
      frame "Stage Homing" {
        n1185 = call "HOMINING.vi"("error in (no error)"=w1803, "main ref"=w1801) -> ("error out"=w1802:errorcluster)  [unwired: 9 in]
      }
      frame "Clear 3" {
        n1186 = Unbundle By Name(w1805) -> ("Loading.Stribeck Table  For loading"=w1815:refnum<vi>)
        n1187 = Unbundle By Name(w1805) -> ("Loading.Clear 3"=w1806:refnum<vi>)
        n1188 = property class="Bool (strict)"(reference=w1806, "Value"=FALSE) -> (reference out=w1808:refnum<vi>, error out=w1807:errorcluster)  [unwired: 1 in]
        n1189 = call "DATA ENCRYPT STRING FILE WRITE.vi"("error in (no error)"=w1811, "User Action"="User Pressed Clear  on Step Load Sequence", "main ref"=w1805) -> ("error out"=w1810:errorcluster)  [unwired: 6 in, 1 out]
        n1190 = property class="Tbl (strict)"(reference=w1815, "Value"=string[][] []) -> (reference out=w1813:refnum<vi>, error out=w1814:errorcluster)  [unwired: 1 in]
        n1191 = Close Reference(reference=w1808, error in (no error)=w1807) -> ()  [unwired: 1 out]
        n1192 = Close Reference(reference=w1813, error in (no error)=w1814) -> ()  [unwired: 1 out]
      }
      frame "Set WTD" {
        n1193 = Unbundle By Name(w1816) -> ("Motion Module.Set WTD"=w1819:refnum<vi>)
        n1194 = property class="Bool (strict)"(reference=w1819, "Value"=FALSE) -> (reference out=w1821:refnum<vi>, error out=w1820:errorcluster)  [unwired: 1 in]
        n1195 = call "DATA ENCRYPT STRING FILE WRITE.vi"("error in (no error)"=w1823, "User Action"="User Pressed  on Set Wear Track", "main ref"=w1816) -> ("error out"=w1822:errorcluster)  [unwired: 6 in, 1 out]
        n1196 = call "Sway wear trac set.vi"("error in (no error)"=w1822, "main ref"=w1816) -> ("error out"=w1817:errorcluster)  [unwired: 9 in]
        n1197 = Close Reference(reference=w1821, error in (no error)=w1820) -> ()  [unwired: 1 out]
      }
      frame "Import 2" {
        n1198 = call "File Dialog"("start path"=path "C:/LAB-IQ 150/User Defined Protocol", "error in"=w1832) -> ("selected path"=w1826:path, "cancelled"=w1829:bool, "error out"=w1831:errorcluster)  [unwired: 10 in, 1 out]
        n1199 = call <vilib>:"Clear Errors.vi"("error in (no error)"=w1831) -> ("error out"=w1828:errorcluster)  [unwired: 5 in, 1 out]
        n1200 = case shown="False" w1829 {
          tunnel: w1828 -> [w1842 w1843]
          tunnel: [w1834 w1843] -> w1827
          tunnel: w1826 -> [w1841 _]
          tunnel: w1825 -> [w1836 _]
          frame False {
            n1201 = call-poly <vilib>:"Read Delimited Spreadsheet.vi"("file path (dialog if empty)"=w1841, "error in (no error)"=w1842, "delimiter (\\t)"=":" ("delimiter (\\t)")) -> ("all rows"=w1833:string[][], "error out"=w1835:errorcluster)  [unwired: 7 in, 4 out]
            n1202 = Unbundle By Name(w1836) -> ("Motion Module.StepTable For Speed"=w1839:refnum<vi>)
            n1203 = property class="Tbl (strict)"(reference=w1839, error in=w1835, "Value"=w1833) -> (reference out=w1837:refnum<vi>, error out=w1838:errorcluster)
            n1204 = Close Reference(reference=w1837, error in (no error)=w1838) -> (error out=w1834:errorcluster)
          }
          frame True {
          }
        }
      }
      frame "Save 2" {
        n1205 = Unbundle By Name(w1847) -> ("Motion Module.StepTable For Speed"=w1862:refnum<vi>)
        n1206 = property class="Tbl (strict)"(reference=w1862) -> (reference out=w1860:refnum<vi>, error out=w1861:errorcluster, "Value"=w1858:string[][])  [unwired: 1 in]
        n1207 = call "File Dialog2"("start path"=path "C:/LAB-IQ 150/User Defined Protocol", "error in"=w1852) -> ("selected path"=w1855:path, "error out"=w1854:errorcluster)  [unwired: 10 in, 2 out]
        n1208 = call <vilib>:"Clear Errors.vi"("error in (no error)"=w1854) -> ("error out"=w1853:errorcluster)  [unwired: 5 in, 1 out]
        n1209 = Close Reference(reference=w1860, error in (no error)=w1861) -> ()  [unwired: 1 out]
        n1210 = call-poly <vilib>:"Write Delimited Spreadsheet.vi"("file path (dialog if empty)"=w1855, "2D data"=w1858, "append to file? (new file:F)"=TRUE, "error in (no error)"=w1853, "delimiter (\\t)"=":" ("delimiter (\\t)")) -> ("error out"=w1851:errorcluster)  [unwired: 9 in, 1 out]
        n1211 = call <vilib>:"Clear Errors.vi"("error in (no error)"=w1851) -> ("error out"=w1846:errorcluster)  [unwired: 5 in, 1 out]
        n1212 = Unbundle By Name(w1847) -> ("Motion Module.Save 2"=w1848:refnum<vi>)
        n1213 = property class="Bool (strict)"(reference=w1848, error in=w1846, "Value"=FALSE) -> (reference out=w1850:refnum<vi>, error out=w1849:errorcluster)
        n1214 = Close Reference(reference=w1850, error in (no error)=w1849) -> (error out=w1845:errorcluster)
      }
      frame "Calculate Rotary" {
        n1215 = call "STEP LOAD MM_SEC AND RPM CONVERSION.vi"("error in (no error)"=w1866, "Data Cluster"=w1864) -> ("error out"=w1865:errorcluster)  [unwired: 9 in]
        n1216 = local write "calculate rotary"(FALSE) -> ()
      }
      frame "Clear List" {
        n1217 = Unbundle By Name(w1868) -> ("Environmental control.Sensors Picked"=w1875:refnum<vi>)
        n1218 = Unbundle By Name(w1868) -> ("Environmental control.Clear List"=w1869:refnum<vi>)
        n1219 = property class="Bool (strict)"(reference=w1869, "Value"=FALSE) -> (reference out=w1871:refnum<vi>, error out=w1870:errorcluster)  [unwired: 1 in]
        n1220 = property class="Str"(reference=w1875, "Value"="") -> (reference out=w1873:refnum<vi>, error out=w1874:errorcluster)  [unwired: 1 in]
        n1221 = Close Reference(reference=w1871, error in (no error)=w1870) -> ()  [unwired: 1 out]
        n1222 = Close Reference(reference=w1873, error in (no error)=w1874) -> ()  [unwired: 1 out]
      }
      frame "ClrLog" {
        n1223 = Unbundle By Name(w1878) -> ("Main Screen.ClrLog"=w1879:refnum<vi>)
        n1224 = Unbundle By Name(w1878) -> ("Main Screen.Trip Log"=w1885:refnum<vi>)
        n1225 = property class="Bool (strict)"(reference=w1879, "Value"=FALSE) -> (reference out=w1881:refnum<vi>, error out=w1880:errorcluster)  [unwired: 1 in]
        n1226 = property class="Str"(reference=w1885, "Value"="") -> (reference out=w1883:refnum<vi>, error out=w1884:errorcluster)  [unwired: 1 in]
        n1227 = Close Reference(reference=w1881, error in (no error)=w1880) -> ()  [unwired: 1 out]
        n1228 = Close Reference(reference=w1883, error in (no error)=w1884) -> ()  [unwired: 1 out]
      }
      frame "Add to list" {
        n1229 = Unbundle By Name(w1887) -> ("Environmental control.Sensors Picked"=w1893:refnum<vi>)
        n1230 = property class="Str"(reference=w1893, error in=w1888, "Value"="") -> (reference out=w1891:refnum<vi>, error out=w1892:errorcluster)
        n1231 = Close Reference(reference=w1891, error in (no error)=w1892) -> (error out=w1889:errorcluster)
        n1232 = call "Add  to List Loop.vi"("error in (no error)"=w1889, "Data Cluster"=w1887) -> ("error out"=w1895:errorcluster)  [unwired: 9 in]
        n1233 = Unbundle By Name(w1887) -> ("Environmental control.Add to list"=w1897:refnum<vi>)
        n1234 = property class="Bool (strict)"(reference=w1897, error in=w1895, "Value"=FALSE) -> (reference out=w1899:refnum<vi>, error out=w1898:errorcluster)
        n1235 = Close Reference(reference=w1899, error in (no error)=w1898) -> (error out=w1894:errorcluster)
      }
      frame "Disable Axis Jog Soft Limits" {
        n1236 = call "DATA ENCRYPT STRING FILE WRITE.vi"("error in (no error)"=w1903, "User Action"="User Pressed Disable Axis Jog Soft Limits in Main Screen", "main ref"=w1901) -> ("error out"=w1902:errorcluster)  [unwired: 6 in, 1 out]
      }
      frame "Home Service" {
        n1237 = Unbundle By Name(w1905) -> ("Main Home Screen.MainPage"=w1911:refnum<vi>)
        n1238 = Unbundle By Name(w1905) -> ("Main Home Screen.GUI"=w1909:refnum<vi>)
        n1239 = local write "Home Service"(FALSE ("Home Service")) -> ()
        n1240 = property class="TabCtl (strict)"(reference=w1911, "Value"=T5."HOME") -> (reference out=w1913:refnum<vi>, error out=w1912:errorcluster)  [unwired: 1 in]
        n1241 = property class="TabCtl (strict)"(reference=w1909, "Value"=T4."Setup") -> (reference out=w1907:refnum<vi>, error out=w1908:errorcluster)  [unwired: 1 in]
        n1242 = Close Reference(reference=w1913, error in (no error)=w1912) -> ()  [unwired: 1 out]
        n1243 = Close Reference(reference=w1907, error in (no error)=w1908) -> ()  [unwired: 1 out]
        n1244 = call "DATA ENCRYPT STRING FILE WRITE.vi"("error in (no error)"=w1916, "User Action"="User Pressed Home Service from Service Screen", "main ref"=w1905) -> ("error out"=w1915:errorcluster)  [unwired: 6 in, 1 out]
      }
      frame "Analysis Home" {
        n1245 = Unbundle By Name(w1918) -> ("Main Home Screen.MainPage"=w1924:refnum<vi>)
        n1246 = Unbundle By Name(w1918) -> ("Main Home Screen.GUI"=w1922:refnum<vi>)
        n1247 = local write "Analysis Home new"(FALSE ("Analysis Home new")) -> ()
        n1248 = property class="TabCtl (strict)"(reference=w1924, "Value"=T5."HOME") -> (reference out=w1926:refnum<vi>, error out=w1925:errorcluster)  [unwired: 1 in]
        n1249 = property class="TabCtl (strict)"(reference=w1922, "Value"=T4."Setup") -> (reference out=w1920:refnum<vi>, error out=w1921:errorcluster)  [unwired: 1 in]
        n1250 = Close Reference(reference=w1926, error in (no error)=w1925) -> ()  [unwired: 1 out]
        n1251 = Close Reference(reference=w1920, error in (no error)=w1921) -> ()  [unwired: 1 out]
        n1252 = call "DATA ENCRYPT STRING FILE WRITE.vi"("error in (no error)"=w1929, "User Action"="User Pressed Home from AnalysisScreen", "main ref"=w1918) -> ("error out"=w1928:errorcluster)  [unwired: 6 in, 1 out]
      }
      frame "Post Analysis" {
        n1253 = Unbundle By Name(w1932) -> ("Main Screen.Main Screen Tab"=w1935:refnum<vi>)
        n1254 = Unbundle By Name(w1932) -> ("Main Home Screen.MainPage"=w1941:refnum<vi>)
        n1255 = Unbundle By Name(w1932) -> ("Main Home Screen.GUI"=w1939:refnum<vi>)
        n1256 = property class="TabCtl (strict)"(reference=w1935, "Value"=T8."Compare Files Rot") -> (reference out=w1933:refnum<vi>, error out=w1934:errorcluster)  [unwired: 1 in]
        n1257 = property class="TabCtl (strict)"(reference=w1941, "Value"=T5."HOME") -> (reference out=w1943:refnum<vi>, error out=w1942:errorcluster)  [unwired: 1 in]
        n1258 = property class="TabCtl (strict)"(reference=w1939, "Value"=T4."Begin") -> (reference out=w1937:refnum<vi>, error out=w1938:errorcluster)  [unwired: 1 in]
        n1259 = local write "Post Analysis"(FALSE ("Post Analysis")) -> ()
        n1260 = Close Reference(reference=w1933, error in (no error)=w1934) -> ()  [unwired: 1 out]
        n1261 = Close Reference(reference=w1943, error in (no error)=w1942) -> ()  [unwired: 1 out]
        n1262 = Close Reference(reference=w1937, error in (no error)=w1938) -> ()  [unwired: 1 out]
        n1263 = call "DATA ENCRYPT STRING FILE WRITE.vi"("error in (no error)"=w1946, "User Action"="User Pressed Post Analysis ", "main ref"=w1932) -> ("error out"=w1945:errorcluster)  [unwired: 6 in, 1 out]
      }
      frame "Edit Gain Constants" {
        n1264 = Unbundle By Name(w1948) -> ("About Screen.Heave and Surge COM Port:"=w1978:refnum<vi>)
        n1265 = Unbundle By Name(w1948) -> ("About Screen.Edit Gain Constants"=w1958:refnum<vi>)
        n1266 = Unbundle By Name(w1948) -> ("About Screen.Sway COM Port:"=w1975:refnum<vi>)
        n1267 = Unbundle By Name(w1948) -> ("About Screen.Ramp Port:"=w1952:refnum<vi>)
        n1268 = Unbundle By Name(w1948) -> ("About Screen.Temp Modbus:"=w1972:refnum<vi>)
        n1269 = Unbundle By Name(w1948) -> ("About Screen.Humidity Port:"=w1971:refnum<vi>)
        n1270 = Unbundle By Name(w1948) -> ("About Screen.Password"=w1966:refnum<vi>)
        n1271 = Unbundle By Name(w1948) -> ("About Screen.ECR Port:"=w1951:refnum<vi>)
        n1272 = property class="VISAName"(reference=w1952, "DisabledEnum"=T13."Enabled" ("Disabled")) -> (reference out=w1954:refnum<vi>, error out=w1953:errorcluster)  [unwired: 1 in]
        n1273 = property class="Bool (strict)"(reference=w1958, "Value"=FALSE) -> (reference out=w1959:refnum<vi>, error out=w1957:errorcluster)  [unwired: 1 in]
        n1274 = property class="VISAName"(reference=w1951, "DisabledEnum"=T13."Enabled" ("Disabled")) -> (reference out=w1947:refnum<vi>, error out=w1950:errorcluster)  [unwired: 1 in]
        n1275 = property class="VISAName"(reference=w1978, "DisabledEnum"=T13."Enabled" ("Disabled")) -> (reference out=w1979:refnum<vi>, error out=w1977:errorcluster)  [unwired: 1 in]
        n1276 = property class="VISAName"(reference=w1975, "DisabledEnum"=T13."Enabled" ("Disabled")) -> (reference out=w1976:refnum<vi>, error out=w1974:errorcluster)  [unwired: 1 in]
        n1277 = property class="VISAName"(reference=w1972, "DisabledEnum"=T13."Enabled" ("Disabled")) -> (reference out=w1960:refnum<vi>, error out=w1973:errorcluster)  [unwired: 1 in]
        n1278 = property class="VISAName"(reference=w1971, "DisabledEnum"=T13."Enabled" ("Disabled")) -> (reference out=w1969:refnum<vi>, error out=w1970:errorcluster)  [unwired: 1 in]
        n1279 = property class="Str"(reference=w1966, "Visible"=FALSE) -> (reference out=w1968:refnum<vi>, error out=w1967:errorcluster)  [unwired: 1 in]
        n1280 = Close Reference(reference=w1954, error in (no error)=w1953) -> ()  [unwired: 1 out]
        n1281 = Close Reference(reference=w1968, error in (no error)=w1967) -> ()  [unwired: 1 out]
        n1282 = Close Reference(reference=w1947, error in (no error)=w1950) -> ()  [unwired: 1 out]
        n1283 = Close Reference(reference=w1959, error in (no error)=w1957) -> ()  [unwired: 1 out]
        n1284 = Close Reference(reference=w1979, error in (no error)=w1977) -> ()  [unwired: 1 out]
        n1285 = Close Reference(reference=w1976, error in (no error)=w1974) -> ()  [unwired: 1 out]
        n1286 = Close Reference(reference=w1960, error in (no error)=w1973) -> ()  [unwired: 1 out]
        n1287 = Close Reference(reference=w1969, error in (no error)=w1970) -> ()  [unwired: 1 out]
        n1288 = call "DATA ENCRYPT STRING FILE WRITE.vi"("error in (no error)"=w1982, "User Action"="User Pressed Home Service from Service Screen", "main ref"=w1948) -> ("error out"=w1981:errorcluster)  [unwired: 6 in, 1 out]
      }
      frame "Advanced Setting" {
        n1289 = Unbundle By Name(w1984) -> ("About Screen.Advanced Setting"=w1986:refnum<vi>)
        n1290 = property class="Bool (strict)"(reference=w1986) -> (reference out=w1987:refnum<vi>, error out=w1985:errorcluster, "Value"=w1983:bool)  [unwired: 1 in]
        n1291 = Close Reference(reference=w1987, error in (no error)=w1985) -> ()  [unwired: 1 out]
        n1292 = case shown="True" w1983 {
          tunnel: w1984 -> [w1992 w2017]
          frame True {
            n1293 = Unbundle By Name(w1992) -> ("About Screen.Heave and Surge COM Port:"=w2014:refnum<vi>)
            n1294 = Unbundle By Name(w1992) -> ("About Screen.Edit Gain Constants"=w1994:refnum<vi>)
            n1295 = Unbundle By Name(w1992) -> ("About Screen.Sway COM Port:"=w2011:refnum<vi>)
            n1296 = Unbundle By Name(w1992) -> ("About Screen.Temp Modbus:"=w2008:refnum<vi>)
            n1297 = Unbundle By Name(w1992) -> ("About Screen.Humidity Port:"=w2007:refnum<vi>)
            n1298 = Unbundle By Name(w1992) -> ("About Screen.Password"=w2002:refnum<vi>)
            n1299 = property class="Bool (strict)"(reference=w1994, "Value"=FALSE) -> (reference out=w1995:refnum<vi>, error out=w1993:errorcluster)  [unwired: 1 in]
            n1300 = property class="VISAName"(reference=w2014, "DisabledEnum"=T13."Disabled and Grayed Out" ("Disabled")) -> (reference out=w2015:refnum<vi>, error out=w2013:errorcluster)  [unwired: 1 in]
            n1301 = property class="VISAName"(reference=w2011, "DisabledEnum"=T13."Disabled and Grayed Out" ("Disabled")) -> (reference out=w2012:refnum<vi>, error out=w2010:errorcluster)  [unwired: 1 in]
            n1302 = property class="VISAName"(reference=w2008, "DisabledEnum"=T13."Disabled and Grayed Out" ("Disabled")) -> (reference out=w1996:refnum<vi>, error out=w2009:errorcluster)  [unwired: 1 in]
            n1303 = property class="VISAName"(reference=w2007, "DisabledEnum"=T13."Disabled and Grayed Out" ("Disabled")) -> (reference out=w2005:refnum<vi>, error out=w2006:errorcluster)  [unwired: 1 in]
            n1304 = property class="Str"(reference=w2002, "Visible"=TRUE) -> (reference out=w2004:refnum<vi>, error out=w2003:errorcluster)  [unwired: 1 in]
            n1305 = Close Reference(reference=w1995, error in (no error)=w1993) -> ()  [unwired: 1 out]
            n1306 = Close Reference(reference=w2015, error in (no error)=w2013) -> ()  [unwired: 1 out]
            n1307 = Close Reference(reference=w2012, error in (no error)=w2010) -> ()  [unwired: 1 out]
            n1308 = Close Reference(reference=w1996, error in (no error)=w2009) -> ()  [unwired: 1 out]
            n1309 = Close Reference(reference=w2005, error in (no error)=w2006) -> ()  [unwired: 1 out]
            n1310 = Close Reference(reference=w2004, error in (no error)=w2003) -> ()  [unwired: 1 out]
          }
          frame False {
            n1311 = Unbundle By Name(w2017) -> ("About Screen.Heave and Surge COM Port:"=w2039:refnum<vi>)
            n1312 = Unbundle By Name(w2017) -> ("About Screen.Edit Gain Constants"=w2019:refnum<vi>)
            n1313 = Unbundle By Name(w2017) -> ("About Screen.Sway COM Port:"=w2036:refnum<vi>)
            n1314 = Unbundle By Name(w2017) -> ("About Screen.Temp Modbus:"=w2033:refnum<vi>)
            n1315 = Unbundle By Name(w2017) -> ("About Screen.Humidity Port:"=w2032:refnum<vi>)
            n1316 = Unbundle By Name(w2017) -> ("About Screen.Password"=w2027:refnum<vi>)
            n1317 = property class="Bool (strict)"(reference=w2019, "Value"=FALSE) -> (reference out=w2020:refnum<vi>, error out=w2018:errorcluster)  [unwired: 1 in]
            n1318 = property class="VISAName"(reference=w2039, "DisabledEnum"=T13."Disabled and Grayed Out" ("Disabled")) -> (reference out=w2040:refnum<vi>, error out=w2038:errorcluster)  [unwired: 1 in]
            n1319 = property class="VISAName"(reference=w2036, "DisabledEnum"=T13."Disabled and Grayed Out" ("Disabled")) -> (reference out=w2037:refnum<vi>, error out=w2035:errorcluster)  [unwired: 1 in]
            n1320 = property class="VISAName"(reference=w2033, "DisabledEnum"=T13."Disabled and Grayed Out" ("Disabled")) -> (reference out=w2021:refnum<vi>, error out=w2034:errorcluster)  [unwired: 1 in]
            n1321 = property class="VISAName"(reference=w2032, "DisabledEnum"=T13."Disabled and Grayed Out" ("Disabled")) -> (reference out=w2030:refnum<vi>, error out=w2031:errorcluster)  [unwired: 1 in]
            n1322 = property class="Str"(reference=w2027, "Visible"=FALSE) -> (reference out=w2029:refnum<vi>, error out=w2028:errorcluster)  [unwired: 1 in]
            n1323 = Close Reference(reference=w2020, error in (no error)=w2018) -> ()  [unwired: 1 out]
            n1324 = Close Reference(reference=w2040, error in (no error)=w2038) -> ()  [unwired: 1 out]
            n1325 = Close Reference(reference=w2037, error in (no error)=w2035) -> ()  [unwired: 1 out]
            n1326 = Close Reference(reference=w2021, error in (no error)=w2034) -> ()  [unwired: 1 out]
            n1327 = Close Reference(reference=w2030, error in (no error)=w2031) -> ()  [unwired: 1 out]
            n1328 = Close Reference(reference=w2029, error in (no error)=w2028) -> ()  [unwired: 1 out]
          }
        }
        n1329 = call "DATA ENCRYPT STRING FILE WRITE.vi"("error in (no error)"=w1990, "User Action"="User Pressed Advance Setting in Service Screen", "main ref"=w1984) -> ("error out"=w1989:errorcluster)  [unwired: 6 in, 1 out]
      }
      frame "Password" {
        n1330 = Unbundle By Name(w2041) -> ("About Screen.Password"=w2047:refnum<vi>)
        n1331 = property class="Str"(reference=w2047) -> (reference out=w2048:refnum<vi>, error out=w2046:errorcluster, "Value"=w2045:string)  [unwired: 1 in]
        n1332 = call <vilib>:"Trim Whitespace.vi"("string"=w2045) -> ("trimmed string"=w2044:string)  [unwired: 1 in]
        n1333 = Close Reference(reference=w2048, error in (no error)=w2046) -> ()  [unwired: 1 out]
        n1334 = Equal?(x=w2044, y="UT150$") -> (x = y?=w2042:bool)
        n1335 = case shown="True" w2042 {
          tunnel: w2041 -> [_ w2051]
          frame False {
          }
          frame True {
            n1336 = Unbundle By Name(w2051) -> ("Main Screen.Main Screen Tab"=w2053:refnum<vi>)
            n1337 = Unbundle By Name(w2051) -> ("Main Home Screen.GUI"=w2057:refnum<vi>)
            n1338 = Unbundle By Name(w2051) -> ("About Screen.Password"=w2061:refnum<vi>)
            n1339 = property class="TabCtl (strict)"(reference=w2057, "Value"=T4."Begin") -> (reference out=w2058:refnum<vi>, error out=w2056:errorcluster)  [unwired: 1 in]
            n1340 = property class="TabCtl (strict)"(reference=w2053, "Value"=T8."Service") -> (reference out=w2052:refnum<vi>, error out=w2054:errorcluster)  [unwired: 1 in]
            n1341 = property class="Str"(reference=w2061, "Value"="") -> (reference out=w2062:refnum<vi>, error out=w2060:errorcluster)  [unwired: 1 in]
            n1342 = Close Reference(reference=w2062, error in (no error)=w2060) -> ()  [unwired: 1 out]
            n1343 = Close Reference(reference=w2058, error in (no error)=w2056) -> ()  [unwired: 1 out]
            n1344 = Close Reference(reference=w2052, error in (no error)=w2054) -> ()  [unwired: 1 out]
          }
        }
      }
      frame "Service About" {
        n1345 = Unbundle By Name(w2064) -> ("Main Screen.Main Screen Tab"=w2067:refnum<vi>)
        n1346 = Unbundle By Name(w2064) -> ("Main Home Screen.GUI"=w2071:refnum<vi>)
        n1347 = local write "Service About"(FALSE ("Service About")) -> ()
        n1348 = property class="TabCtl (strict)"(reference=w2071, "Value"=T4."Begin") -> (reference out=w2072:refnum<vi>, error out=w2070:errorcluster)  [unwired: 1 in]
        n1349 = property class="TabCtl (strict)"(reference=w2067, "Value"=T8."About") -> (reference out=w2066:refnum<vi>, error out=w2068:errorcluster)  [unwired: 1 in]
        n1350 = Close Reference(reference=w2072, error in (no error)=w2070) -> ()  [unwired: 1 out]
        n1351 = Close Reference(reference=w2066, error in (no error)=w2068) -> ()  [unwired: 1 out]
      }
      frame "OPEN 1" {
        n1352 = Unbundle By Name(w2076) -> ("Analysis Screen.File 1 Discription"=w2085:refnum<vi>)
        n1353 = property class="Str"(reference=w2085, error in=w2083, "Value"="") -> (reference out=w2086:refnum<vi>, error out=w2084:errorcluster)
        n1354 = Close Reference(reference=w2086, error in (no error)=w2084) -> (error out=w2082:errorcluster)
        n1355 = call <vilib>:"Application Directory.vi"() -> ("Application Directory"=w2090:path)
        n1356 = Unbundle By Name(w2076) -> ("Analysis Screen.OPEN 1"=w2078:refnum<vi>)
        n1357 = Build Path(base path=w2090, name or relative path="data") -> (appended path=w2088:path)
        n1358 = property class="Bool (strict)"(reference=w2078, "Value"=FALSE) -> (reference out=w2079:refnum<vi>, error out=w2077:errorcluster)  [unwired: 1 in]
        n1359 = call "File Dialog3"("start path"=w2088, "error in"=w2082) -> ("selected path"=w2087:path, "cancelled"=w2074:bool, "error out"=w2091:errorcluster)  [unwired: 10 in, 1 out]
        n1360 = case shown="True" w2074 {
          tunnel: w2091 -> [w2105 _]
          tunnel: w2087 -> [w2101 _]
          tunnel: [w2093 _] -> w2080
          tunnel: w2076 -> [w2092 w2107]
          frame False {
            n1361 = Path To String(path=w2101) -> (string=w2100:string)
            n1362 = Unbundle By Name(w2092) -> ("Analysis Screen.File Name 1"=w2103:refnum<vi>)
            n1363 = call <vilib>:"Clear Errors.vi"("error in (no error)"=w2105) -> ("error out"=w2099:errorcluster)  [unwired: 5 in, 1 out]
            n1364 = property class="Str"(reference=w2103, "Value"=w2100) -> (reference out=w2104:refnum<vi>, error out=w2102:errorcluster)  [unwired: 1 in]
            n1365 = call "INI FILE READ.vi"("error in (no error)"=w2099, "File Path"=w2100) -> ("error out"=w2095:errorcluster, "concatenated string"=w2094:string)  [unwired: 8 in]
            n1366 = Unbundle By Name(w2092) -> ("Analysis Screen.File 1 Discription"=w2097:refnum<vi>)
            n1367 = Close Reference(reference=w2104, error in (no error)=w2102) -> ()  [unwired: 1 out]
            n1368 = property class="Str"(reference=w2097, error in=w2095, "Value"=w2094) -> (reference out=w2098:refnum<vi>, error out=w2096:errorcluster)
            n1369 = Close Reference(reference=w2098, error in (no error)=w2096) -> (error out=w2093:errorcluster)
          }
          frame True {
            n1370 = Unbundle By Name(w2107) -> ("Analysis Screen.File 1 Discription"=w2109:refnum<vi>)
            n1371 = Unbundle By Name(w2107) -> ("Analysis Screen.File Name 1"=w2113:refnum<vi>)
            n1372 = property class="Str"(reference=w2109, "Value"="") -> (reference out=w2110:refnum<vi>, error out=w2108:errorcluster)  [unwired: 1 in]
            n1373 = property class="Str"(reference=w2113, "Value"="") -> (reference out=w2114:refnum<vi>, error out=w2112:errorcluster)  [unwired: 1 in]
            n1374 = Close Reference(reference=w2110, error in (no error)=w2108) -> ()  [unwired: 1 out]
            n1375 = Close Reference(reference=w2114, error in (no error)=w2112) -> ()  [unwired: 1 out]
          }
        }
        n1376 = Close Reference(reference=w2079, error in (no error)=w2077) -> ()  [unwired: 1 out]
      }
      frame "OPEN 2" {
        n1377 = Unbundle By Name(w2117) -> ("Analysis Screen.File 2 Discription"=w2126:refnum<vi>)
        n1378 = property class="Str"(reference=w2126, error in=w2124, "Value"="") -> (reference out=w2127:refnum<vi>, error out=w2125:errorcluster)
        n1379 = Close Reference(reference=w2127, error in (no error)=w2125) -> (error out=w2123:errorcluster)
        n1380 = call <vilib>:"Application Directory.vi"() -> ("Application Directory"=w2131:path)
        n1381 = Unbundle By Name(w2117) -> ("Analysis Screen.OPEN 2"=w2119:refnum<vi>)
        n1382 = Build Path(base path=w2131, name or relative path="data") -> (appended path=w2129:path)
        n1383 = property class="Bool (strict)"(reference=w2119, "Value"=FALSE) -> (reference out=w2120:refnum<vi>, error out=w2118:errorcluster)  [unwired: 1 in]
        n1384 = call "File Dialog4"("start path"=w2129, "error in"=w2123) -> ("selected path"=w2128:path, "cancelled"=w2115:bool, "error out"=w2132:errorcluster)  [unwired: 10 in, 1 out]
        n1385 = case shown="True" w2115 {
          tunnel: w2132 -> [w2146 w2148]
          tunnel: w2128 -> [w2142 _]
          tunnel: [w2134 w2147] -> w2121
          tunnel: w2117 -> [w2133 w2150]
          frame False {
            n1386 = Path To String(path=w2142) -> (string=w2141:string)
            n1387 = Unbundle By Name(w2133) -> ("Analysis Screen.File Name 2"=w2144:refnum<vi>)
            n1388 = call <vilib>:"Clear Errors.vi"("error in (no error)"=w2146) -> ("error out"=w2140:errorcluster)  [unwired: 5 in, 1 out]
            n1389 = property class="Str"(reference=w2144, "Value"=w2141) -> (reference out=w2145:refnum<vi>, error out=w2143:errorcluster)  [unwired: 1 in]
            n1390 = call "INI FILE READ.vi"("error in (no error)"=w2140, "File Path"=w2141) -> ("error out"=w2136:errorcluster, "concatenated string"=w2135:string)  [unwired: 8 in]
            n1391 = Unbundle By Name(w2133) -> ("Analysis Screen.File 2 Discription"=w2138:refnum<vi>)
            n1392 = Close Reference(reference=w2145, error in (no error)=w2143) -> ()  [unwired: 1 out]
            n1393 = property class="Str"(reference=w2138, error in=w2136, "Value"=w2135) -> (reference out=w2139:refnum<vi>, error out=w2137:errorcluster)
            n1394 = Close Reference(reference=w2139, error in (no error)=w2137) -> (error out=w2134:errorcluster)
          }
          frame True {
            n1395 = Unbundle By Name(w2150) -> ("Analysis Screen.File Name 2"=w2156:refnum<vi>)
            n1396 = Unbundle By Name(w2150) -> ("Analysis Screen.File 2 Discription"=w2152:refnum<vi>)
            n1397 = property class="Str"(reference=w2156, "Value"="") -> (reference out=w2157:refnum<vi>, error out=w2155:errorcluster)  [unwired: 1 in]
            n1398 = property class="Str"(reference=w2152, "Value"="") -> (reference out=w2151:refnum<vi>, error out=w2153:errorcluster)  [unwired: 1 in]
            n1399 = call <vilib>:"Clear Errors.vi"("error in (no error)"=w2148) -> ("error out"=w2147:errorcluster)  [unwired: 5 in, 1 out]
            n1400 = Close Reference(reference=w2151, error in (no error)=w2153) -> ()  [unwired: 1 out]
            n1401 = Close Reference(reference=w2157, error in (no error)=w2155) -> ()  [unwired: 1 out]
          }
        }
        n1402 = Close Reference(reference=w2120, error in (no error)=w2118) -> ()  [unwired: 1 out]
      }
      frame "OPEN 3" {
        # "3416\n4017\n4554"
        n1403 = Unbundle By Name(w2160) -> ("Analysis Screen.File 3 Discription"=w2169:refnum<vi>)
        n1404 = property class="Str"(reference=w2169, error in=w2167, "Value"="") -> (reference out=w2170:refnum<vi>, error out=w2168:errorcluster)
        n1405 = Close Reference(reference=w2170, error in (no error)=w2168) -> (error out=w2166:errorcluster)
        n1406 = call <vilib>:"Application Directory.vi"() -> ("Application Directory"=w2174:path)
        n1407 = Unbundle By Name(w2160) -> ("Analysis Screen.OPEN 3"=w2162:refnum<vi>)
        n1408 = Build Path(base path=w2174, name or relative path="data") -> (appended path=w2172:path)
        n1409 = property class="Bool (strict)"(reference=w2162, "Value"=FALSE) -> (reference out=w2163:refnum<vi>, error out=w2161:errorcluster)  [unwired: 1 in]
        n1410 = call "File Dialog5"("start path"=w2172, "error in"=w2166) -> ("selected path"=w2171:path, "cancelled"=w2158:bool, "error out"=w2175:errorcluster)  [unwired: 10 in, 1 out]
        n1411 = case shown="True" w2158 {
          tunnel: w2175 -> [w2189 w2191]
          tunnel: w2171 -> [w2185 _]
          tunnel: [w2177 w2190] -> w2164
          tunnel: w2160 -> [w2176 w2193]
          frame False {
            n1412 = Path To String(path=w2185) -> (string=w2184:string)
            n1413 = Unbundle By Name(w2176) -> ("Analysis Screen.File Name 3"=w2187:refnum<vi>)
            n1414 = call <vilib>:"Clear Errors.vi"("error in (no error)"=w2189) -> ("error out"=w2183:errorcluster)  [unwired: 5 in, 1 out]
            n1415 = property class="Str"(reference=w2187, "Value"=w2184) -> (reference out=w2188:refnum<vi>, error out=w2186:errorcluster)  [unwired: 1 in]
            n1416 = call "INI FILE READ.vi"("error in (no error)"=w2183, "File Path"=w2184) -> ("error out"=w2179:errorcluster, "concatenated string"=w2178:string)  [unwired: 8 in]
            n1417 = Unbundle By Name(w2176) -> ("Analysis Screen.File 3 Discription"=w2181:refnum<vi>)
            n1418 = Close Reference(reference=w2188, error in (no error)=w2186) -> ()  [unwired: 1 out]
            n1419 = property class="Str"(reference=w2181, error in=w2179, "Value"=w2178) -> (reference out=w2182:refnum<vi>, error out=w2180:errorcluster)
            n1420 = Close Reference(reference=w2182, error in (no error)=w2180) -> (error out=w2177:errorcluster)
          }
          frame True {
            n1421 = Unbundle By Name(w2193) -> ("Analysis Screen.File Name 3"=w2199:refnum<vi>)
            n1422 = Unbundle By Name(w2193) -> ("Analysis Screen.File 3 Discription"=w2195:refnum<vi>)
            n1423 = property class="Str"(reference=w2199, "Value"="") -> (reference out=w2200:refnum<vi>, error out=w2198:errorcluster)  [unwired: 1 in]
            n1424 = property class="Str"(reference=w2195, "Value"="") -> (reference out=w2194:refnum<vi>, error out=w2196:errorcluster)  [unwired: 1 in]
            n1425 = Close Reference(reference=w2194, error in (no error)=w2196) -> ()  [unwired: 1 out]
            n1426 = Close Reference(reference=w2200, error in (no error)=w2198) -> ()  [unwired: 1 out]
            n1427 = call <vilib>:"Clear Errors.vi"("error in (no error)"=w2191) -> ("error out"=w2190:errorcluster)  [unwired: 5 in, 1 out]
          }
        }
        n1428 = Close Reference(reference=w2163, error in (no error)=w2161) -> ()  [unwired: 1 out]
      }
      frame "OPEN 4" {
        n1429 = Unbundle By Name(w2203) -> ("Analysis Screen.File 4 Discription"=w2212:refnum<vi>)
        n1430 = property class="Str"(reference=w2212, error in=w2210, "Value"="") -> (reference out=w2213:refnum<vi>, error out=w2211:errorcluster)
        n1431 = Close Reference(reference=w2213, error in (no error)=w2211) -> (error out=w2209:errorcluster)
        n1432 = call <vilib>:"Application Directory.vi"() -> ("Application Directory"=w2217:path)
        n1433 = Unbundle By Name(w2203) -> ("Analysis Screen.OPEN 4"=w2205:refnum<vi>)
        n1434 = Build Path(base path=w2217, name or relative path="data") -> (appended path=w2215:path)
        n1435 = property class="Bool (strict)"(reference=w2205, "Value"=FALSE) -> (reference out=w2206:refnum<vi>, error out=w2204:errorcluster)  [unwired: 1 in]
        n1436 = call "File Dialog6"("start path"=w2215, "error in"=w2209) -> ("selected path"=w2214:path, "cancelled"=w2201:bool, "error out"=w2218:errorcluster)  [unwired: 10 in, 1 out]
        n1437 = case shown="True" w2201 {
          tunnel: w2218 -> [w2232 w2234]
          tunnel: w2214 -> [w2228 _]
          tunnel: [w2220 w2233] -> w2207
          tunnel: w2203 -> [w2219 w2236]
          frame False {
            n1438 = Path To String(path=w2228) -> (string=w2227:string)
            n1439 = Unbundle By Name(w2219) -> ("Analysis Screen.File Name 4"=w2230:refnum<vi>)
            n1440 = call <vilib>:"Clear Errors.vi"("error in (no error)"=w2232) -> ("error out"=w2226:errorcluster)  [unwired: 5 in, 1 out]
            n1441 = property class="Str"(reference=w2230, "Value"=w2227) -> (reference out=w2231:refnum<vi>, error out=w2229:errorcluster)  [unwired: 1 in]
            n1442 = call "INI FILE READ.vi"("error in (no error)"=w2226, "File Path"=w2227) -> ("error out"=w2222:errorcluster, "concatenated string"=w2221:string)  [unwired: 8 in]
            n1443 = Unbundle By Name(w2219) -> ("Analysis Screen.File 4 Discription"=w2224:refnum<vi>)
            n1444 = Close Reference(reference=w2231, error in (no error)=w2229) -> ()  [unwired: 1 out]
            n1445 = property class="Str"(reference=w2224, error in=w2222, "Value"=w2221) -> (reference out=w2225:refnum<vi>, error out=w2223:errorcluster)
            n1446 = Close Reference(reference=w2225, error in (no error)=w2223) -> (error out=w2220:errorcluster)
          }
          frame True {
            n1447 = Unbundle By Name(w2236) -> ("Analysis Screen.File Name 4"=w2242:refnum<vi>)
            n1448 = Unbundle By Name(w2236) -> ("Analysis Screen.File 4 Discription"=w2238:refnum<vi>)
            n1449 = property class="Str"(reference=w2242, "Value"="") -> (reference out=w2243:refnum<vi>, error out=w2241:errorcluster)  [unwired: 1 in]
            n1450 = property class="Str"(reference=w2238, "Value"="") -> (reference out=w2237:refnum<vi>, error out=w2239:errorcluster)  [unwired: 1 in]
            n1451 = Close Reference(reference=w2237, error in (no error)=w2239) -> ()  [unwired: 1 out]
            n1452 = Close Reference(reference=w2243, error in (no error)=w2241) -> ()  [unwired: 1 out]
            n1453 = call <vilib>:"Clear Errors.vi"("error in (no error)"=w2234) -> ("error out"=w2233:errorcluster)  [unwired: 5 in, 1 out]
          }
        }
        n1454 = Close Reference(reference=w2206, error in (no error)=w2204) -> ()  [unwired: 1 out]
      }
      frame "Refresh 2" {
        n1455 = call "Data Log Refresh.vi"("error in (no error)"=w2245, "Data Cluster"=w2244) -> ("error out"=w2246:errorcluster)  [unwired: 9 in]
      }
      frame "Scratch Mode" {
        n1456 = Unbundle By Name(w2247) -> ("Motion Module.Scratch Mode"=w2250:refnum<vi>)
        n1457 = property class="Ring (strict)"(reference=w2250) -> (reference out=w2251:refnum<vi>, error out=w2249:errorcluster, "Value"=w2248:u16)  [unwired: 1 in]
        n1458 = Close Reference(reference=w2251, error in (no error)=w2249) -> ()  [unwired: 1 out]
        n1459 = case shown="2" w2248 {
          tunnel: w2247 -> [w2254 w2258]
          frame 0, Default {
            n1460 = Unbundle By Name(w2254) -> ("Motion Module.No of Scratch"=w2256:refnum<vi>)
            n1461 = property class="DigNum (strict)"(reference=w2256, "Visible"=FALSE) -> (reference out=w2257:refnum<vi>, error out=w2255:errorcluster)  [unwired: 1 in]
            n1462 = Close Reference(reference=w2257, error in (no error)=w2255) -> ()  [unwired: 1 out]
          }
          frame 2 {
            n1463 = Unbundle By Name(w2258) -> ("Motion Module.No of Scratch"=w2261:refnum<vi>)
            n1464 = property class="DigNum (strict)"(reference=w2261, "Visible"=TRUE) -> (reference out=w2262:refnum<vi>, error out=w2260:errorcluster)  [unwired: 1 in]
            n1465 = Close Reference(reference=w2262, error in (no error)=w2260) -> ()  [unwired: 1 out]
          }
        }
      }
      frame "Error" {
        # "#CodeRecommended - If you ever change the name of this \"Error\" message, you'll need to update the name in the Check Loop Error.vi as well."
        # "#CodeRecommended - Consider creating a system for logging errors in some way. These errors are for notification purposes only. Handling of specific errors should be performed in the message frames that generated the error."
        # "Error - Display an error dialog. This message is sent by the \"Error Handler\" VIs at the end of other loops in this application."
        n1466 = Variant To Data(error in=w2269, type=errorcluster {"status"=FALSE, "code"=0, "source"=""} ("error constant"), Variant=w2267) -> (data=w2265:errorcluster, error out=w2264:errorcluster)
        n1467 = call <vilib>:"Simple Error Handler.vi"("error in (no error)"=w2265) -> ()  [unwired: 4 in, 5 out]
        n1468 = Merge Errors(w2264) -> (w2263:errorcluster)
      }
      frame "Confirm Quit" {
        # "#CodeNeeded - If you want to provide an \"Are you sure\" dialog (or some other notification) before the application exits, place that code here. This message is typically sent from a Panel Close? event."
        # "Confirm Quit - Message that can confirm whether or not the user wants to exit the application."
        n1469 = call-poly "Enqueue Message.vi"("Priority Message? (F)"=TRUE, "error in (no error)"=w2276, "Message"="Exit", "Message Queue"=w2273) -> ("error out"=w2274:errorcluster)  [unwired: 6 in, 1 out]
        n1470 = Merge Errors(w2274) -> (w2275:errorcluster)
      }
      frame "Exit" {
        # "Stop the VI"
        # "Release the message queue reference"
        # "#CodeNeeded - Add any required cleanup code here. Note that if 'Exit' was called as a result of an error, an error dialog will be displayed. Add any custom error handling for an 'Exit' condition here as well."
        # "Exit - Exit the application."
        n1471 = call "Fire User Event - Stop.vi"("User Event - Stop"=w2279) -> ("error out"=w2278:errorcluster)  [unwired: 10 in]
        n1472 = Release Queue(queue=w2284, error in (no error)=w2277) -> (error out=w2281:errorcluster)  [unwired: 1 in, 2 out]
        n1473 = Merge Errors(w2278, w2281) -> (w2280:errorcluster)
      }
      frame Default {
        # "'Default' case only runs if there is a message that isn't defined in any of the other cases.  Output a programming error."
        n1474 = xnode "Error Ring"("parameter 0"=w2285) -> ("error out"=w2286:errorcluster)
      }
    }
    n1475 = call "LAB-IQ Error Handler - Message Handling Loop.vi"("error in (no error)"=w983, "Message Queue"=w985) -> ("dup error in"=w984:errorcluster)  [unwired: 8 in, 1 out]
  }
  n1476 = while {
    shift-right: [w2305] -> _
    shift-left: w15 -> [w2306]
    tunnel: [w2299] -> w25
    tunnel: w24 -> [w2297]
    tunnel: w5 -> [w2296]
    tunnel: w14 -> [w2295]
    stop <- w2304 stop-if-true
    # "Load  Handling Loop"
    n1477 = call "Dequeue Message.vi"("error in (no error)"=w2296, "Message Queue"=w2297) -> ("error out"=w2303:errorcluster, "Message Data"=w2301:variant, "Message"=w2302:string, "dup Message Queue"=w2300:refnum<queue>)  [unwired: 6 in]
    n1478 = case "Message Cases" shown="\"Load Main\"" w2302 {
      selector: w2302 -> [_ _ _ _ _ w2360]
      tunnel: w2300 -> [w2307 w2320 _ w2349 w2359 _]
      tunnel: w2303 -> [w2310 w2318 w2336 w2351 w2353 _]
      tunnel: [w2311 w2321 w2330 w2337 w2355 w2361] -> w2298
      tunnel: w2306 -> [w2309 w2313 w2335 w2346 w2358 w2362]
      tunnel: [w2309 w2313 w2335 w2346 w2358 w2362] -> w2305
      tunnel: [_ _ _ _ TRUE _] -> w2304
      tunnel: w2301 -> [_ _ w2334 _ _ _]
      tunnel: w2295 -> [_ _ _ _ w2352 _]
      frame "init" {
        # "Bundle control references and a sample string value."
        # "Initialize - All initialization work should take place in this message, since other loops can potentially enqueue messages that execute immediately after this one."
        n1479 = call-poly "Enqueue Message.vi"("error in (no error)"=w2310, "Message"="Load Main", "Message Queue"=w2307) -> ("error out"=w2311:errorcluster)  [unwired: 7 in, 1 out]
      }
      frame "Load Main" {
        n1480 = call "LOAD CELL READ.vi"("error in (no error)"=w2318, "main ref"=w2313) -> ("error out"=w2314:errorcluster)  [unwired: 9 in]
        n1481 = call <vilib>:"Clear Errors.vi"("error in (no error)"=w2314) -> ("error out"=w2312:errorcluster)  [unwired: 5 in, 1 out]
        n1482 = Unbundle By Name(w2313) -> ("Main Home Screen.EXIT"=w2319:refnum<vi>)
        n1483 = property class="Bool (strict)"(reference=w2319) -> (reference out=w2316:refnum<vi>, error out=w2317:errorcluster, "Value"=w2315:bool)  [unwired: 1 in]
        n1484 = Close Reference(reference=w2316, error in (no error)=w2317) -> ()  [unwired: 1 out]
        n1485 = case shown="False" w2315 {
          tunnel: [w2324 w2328] -> w2321
          tunnel: w2320 -> [w2323 w2327]
          tunnel: w2312 -> [w2322 w2326]
          frame True {
            n1486 = call-poly "Enqueue Message.vi"("error in (no error)"=w2322, "Message"="Confirm Quit", "Message Queue"=w2323) -> ("error out"=w2324:errorcluster)  [unwired: 7 in, 1 out]
          }
          frame False {
            n1487 = call-poly "Enqueue Message.vi"("error in (no error)"=w2326, "Message"="Load Main", "Message Queue"=w2327) -> ("error out"=w2328:errorcluster)  [unwired: 7 in, 1 out]
          }
        }
      }
      frame "Error" {
        # "#CodeRecommended - If you ever change the name of this \"Error\" message, you'll need to update the name in the Check Loop Error.vi as well."
        # "#CodeRecommended - Consider creating a system for logging errors in some way. These errors are for notification purposes only. Handling of specific errors should be performed in the message frames that generated the error."
        # "Error - Display an error dialog. This message is sent by the \"Error Handler\" VIs at the end of other loops in this application."
        n1488 = Variant To Data(error in=w2336, type=errorcluster {"status"=FALSE, "code"=0, "source"=""} ("error constant"), Variant=w2334) -> (data=w2332:errorcluster, error out=w2331:errorcluster)
        n1489 = call <vilib>:"Simple Error Handler.vi"("error in (no error)"=w2332) -> ()  [unwired: 4 in, 5 out]
        n1490 = Merge Errors(w2331) -> (w2330:errorcluster)
      }
      frame "Confirm Quit" {
        # "#CodeNeeded - If you want to provide an \"Are you sure\" dialog (or some other notification) before the application exits, place that code here. This message is typically sent from a Panel Close? event."
        # "Confirm Quit - Message that can confirm whether or not the user wants to exit the application."
        n1491 = call-poly "Enqueue Message.vi"("Priority Message? (F)"=TRUE, "error in (no error)"=w2351, "Message"="Exit", "Message Queue"=w2349) -> ("error out"=w2350:errorcluster)  [unwired: 6 in, 1 out]
        n1492 = Merge Errors(w2350) -> (w2342:errorcluster)
        n1493 = call <vilib>:"Clear Errors.vi"("error in (no error)"=w2342) -> ("error out"=w2338:errorcluster)  [unwired: 5 in, 1 out]
        n1494 = call "LOAD CELL FGV MAIN.vi"("Enum"=T14."UNINITIAL", "error in (no error)"=w2338, "main ref"=w2346) -> ("error IO"=w2345:errorcluster)  [unwired: 8 in]
        n1495 = call "Stall Data Flow.vim"("value in"=w2345, "milliseconds to wait"=u32 1000) -> ("value out"=w2340:errorcluster)  [unwired: 1 out]
        n1496 = call "LOAD CELL FGV MAIN.vi"("Enum"=T14."DELETEHANDLE", "error in (no error)"=w2340, "main ref"=w2346) -> ("error IO"=w2341:errorcluster)  [unwired: 8 in]
        n1497 = call <vilib>:"Clear Errors.vi"("error in (no error)"=w2341) -> ("error out"=w2337:errorcluster)  [unwired: 5 in, 1 out]
      }
      frame "Exit" {
        # "Stop the VI"
        # "Release the message queue reference"
        # "#CodeNeeded - Add any required cleanup code here. Note that if 'Exit' was called as a result of an error, an error dialog will be displayed. Add any custom error handling for an 'Exit' condition here as well."
        # "Exit - Exit the application."
        n1498 = call "Fire User Event - Stop.vi"("User Event - Stop"=w2352) -> ("error out"=w2354:errorcluster)  [unwired: 10 in]
        n1499 = Release Queue(queue=w2359, error in (no error)=w2353) -> (error out=w2356:errorcluster)  [unwired: 1 in, 2 out]
        n1500 = Merge Errors(w2354, w2356) -> (w2355:errorcluster)
      }
      frame Default {
        # "'Default' case only runs if there is a message that isn't defined in any of the other cases.  Output a programming error."
        n1501 = xnode "Error Ring"("parameter 0"=w2360) -> ("error out"=w2361:errorcluster)
      }
    }
    n1502 = call "LAB-IQ Error Handler - Message Handling Loop.vi"("error in (no error)"=w2298, "Message Queue"=w2300) -> ("dup error in"=w2299:errorcluster)  [unwired: 8 in, 1 out]
  }
  n1503 = while {
    shift-right: [w2380] -> _
    shift-left: w15 -> [w2381]
    tunnel: [w2374] -> w22
    tunnel: w23 -> [w2372]
    tunnel: w5 -> [w2371]
    tunnel: w14 -> [w2370]
    stop <- w2379 stop-if-true
    # "Sway Motor  Handling Loop"
    n1504 = call "Dequeue Message.vi"("error in (no error)"=w2371, "Message Queue"=w2372) -> ("error out"=w2378:errorcluster, "Message Data"=w2376:variant, "Message"=w2377:string, "dup Message Queue"=w2375:refnum<queue>)  [unwired: 6 in]
    n1505 = case "Message Cases" shown="\"Sway Main\"" w2377 {
      selector: w2377 -> [_ _ _ _ _ w2465]
      tunnel: w2375 -> [w2393 w2422 _ w2452 w2464 _]
      tunnel: w2378 -> [w2395 w2403 w2449 w2456 w2458 _]
      tunnel: [w2396 w2423 w2443 w2454 w2460 w2466] -> w2373
      tunnel: w2381 -> [w2384 w2397 w2448 w2455 w2463 w2467]
      tunnel: [w2384 w2397 w2448 w2455 w2463 w2467] -> w2380
      tunnel: [_ _ _ _ TRUE _] -> w2379
      tunnel: w2376 -> [_ _ w2447 _ _ _]
      tunnel: w2370 -> [_ _ _ _ w2457 _]
      frame "init" {
        # "Initialize - All initialization work should take place in this message, since other loops can potentially enqueue messages that execute immediately after this one."
        n1506 = call "SWAY WRITE FGV.vi"("Enum - Menu"=Sway_Write_enum."INIT", "error in (no error)"=w2395, "main ref"=w2384) -> ("error out"=w2392:errorcluster)  [unwired: 8 in]
        n1507 = call <vilib>:"Clear Errors.vi"("error in (no error)"=w2392) -> ("error out"=w2383:errorcluster)  [unwired: 5 in, 1 out]
        n1508 = call "Stall Data Flow.vim"("value in"=w2383, "milliseconds to wait"=u32 1000) -> ("value out"=w2390:errorcluster)  [unwired: 1 out]
        n1509 = call "Sway Init.vi"("error in (no error)"=w2390, "main ref"=w2384) -> ("error out"=w2385:errorcluster)  [unwired: 9 in]
        n1510 = call <vilib>:"Clear Errors.vi"("error in (no error)"=w2385) -> ("error out"=w2382:errorcluster)  [unwired: 5 in, 1 out]
        n1511 = call "SWAY READ FGV.vi"("Enum - Menu"=Sway_Right_enum."INIT", "error in (no error)"=w2382, "main ref"=w2384) -> ("error out"=w2388:errorcluster)  [unwired: 7 in, 1 out]
        n1512 = call <vilib>:"Clear Errors.vi"("error in (no error)"=w2388) -> ("error out"=w2387:errorcluster)  [unwired: 5 in, 1 out]
        n1513 = call-poly "Enqueue Message.vi"("error in (no error)"=w2387, "Message"="Sway Main", "Message Queue"=w2393) -> ("error out"=w2396:errorcluster)  [unwired: 7 in, 1 out]
      }
      frame "Sway Main" {
        n1514 = Unbundle By Name(w2397) -> ("Heave AND Surge.SURGE POSE"=w2408:refnum<vi>)
        n1515 = Unbundle By Name(w2397) -> ("SWAY.Read SWAY Temp"=w2417:refnum<vi>)
        n1516 = local read "HEAVE ENABLE"() -> (w2412:bool)
        n1517 = property class="DigNum (strict)"(reference=w2408) -> (reference out=w2410:refnum<vi>, error out=w2409:errorcluster, "Value"=w2407:sgl)  [unwired: 1 in]
        n1518 = property class="Bool (strict)"(reference=w2417) -> (reference out=w2415:refnum<vi>, error out=w2416:errorcluster, "Value"=w2414:bool)  [unwired: 1 in]
        n1519 = Equal?(x=w2412, y=TRUE) -> (x = y?=w2406:bool)
        n1520 = Close Reference(reference=w2410, error in (no error)=w2409) -> ()  [unwired: 1 out]
        n1521 = Equal?(x=w2407, y=sgl 25000.0) -> (x = y?=w2405:bool)
        n1522 = Close Reference(reference=w2415, error in (no error)=w2416) -> ()  [unwired: 1 out]
        n1523 = And(x=w2406, y=w2405) -> (x .and. y?=w2404:bool)
        n1524 = case shown="True" w2404 {
          tunnel: w2397 -> [_ w2429]
          tunnel: w2403 -> [w2424 w2428]
          tunnel: [w2424 w2425] -> w2401
          frame False {
          }
          frame True {
            n1525 = call "SWAY HOME.vi"("error in (no error)"=w2428, "Data Cluster"=w2429) -> ("error out"=w2426:errorcluster)  [unwired: 9 in]
            n1526 = local write "HEAVE ENABLE"(FALSE ("HEAVE ENABLE")) -> ()
            n1527 = call <vilib>:"Clear Errors.vi"("error in (no error)"=w2426) -> ("error out"=w2425:errorcluster)  [unwired: 5 in, 1 out]
          }
        }
        n1528 = case shown="True" w2414 {
          tunnel: w2403 -> [w2430 w2434]
          tunnel: [w2430 w2433] -> w2399
          tunnel: w2397 -> [_ w2432]
          frame False {
          }
          frame True {
            n1529 = call "SWAY READ FGV.vi"("Enum - Menu"=Sway_Right_enum."READ", "error in (no error)"=w2434, "main ref"=w2432) -> ("error out"=w2433:errorcluster)  [unwired: 7 in, 1 out]
          }
        }
        n1530 = call "Sway Reinitize.vi"("error in (no error)"=w2399, "Data Cluster"=w2397) -> ("error out"=w2398:errorcluster)  [unwired: 9 in]
        n1531 = Unbundle By Name(w2397) -> ("Main Home Screen.EXIT"=w2421:refnum<vi>)
        n1532 = property class="Bool (strict)"(reference=w2421) -> (reference out=w2419:refnum<vi>, error out=w2420:errorcluster, "Value"=w2418:bool)  [unwired: 1 in]
        n1533 = call <vilib>:"Clear Errors.vi"("error in (no error)"=w2398) -> ("error out"=w2413:errorcluster)  [unwired: 5 in, 1 out]
        n1534 = Merge Errors(w2413, w2401) -> (w2402:errorcluster)
        n1535 = Close Reference(reference=w2419, error in (no error)=w2420) -> ()  [unwired: 1 out]
        n1536 = case shown="False" w2418 {
          tunnel: [w2437 w2441] -> w2423
          tunnel: w2422 -> [w2436 w2440]
          tunnel: w2402 -> [w2435 w2439]
          frame True {
            n1537 = call-poly "Enqueue Message.vi"("error in (no error)"=w2435, "Message"="Confirm Quit", "Message Queue"=w2436) -> ("error out"=w2437:errorcluster)  [unwired: 7 in, 1 out]
          }
          frame False {
            n1538 = call-poly "Enqueue Message.vi"("error in (no error)"=w2439, "Message"="Sway Main", "Message Queue"=w2440) -> ("error out"=w2441:errorcluster)  [unwired: 7 in, 1 out]
          }
        }
      }
      frame "Error" {
        # "#CodeRecommended - If you ever change the name of this \"Error\" message, you'll need to update the name in the Check Loop Error.vi as well."
        # "#CodeRecommended - Consider creating a system for logging errors in some way. These errors are for notification purposes only. Handling of specific errors should be performed in the message frames that generated the error."
        # "Error - Display an error dialog. This message is sent by the \"Error Handler\" VIs at the end of other loops in this application."
        n1539 = Variant To Data(error in=w2449, type=errorcluster {"status"=FALSE, "code"=0, "source"=""} ("error constant"), Variant=w2447) -> (data=w2445:errorcluster, error out=w2444:errorcluster)
        n1540 = call <vilib>:"Simple Error Handler.vi"("error in (no error)"=w2445) -> ()  [unwired: 4 in, 5 out]
        n1541 = Merge Errors(w2444) -> (w2443:errorcluster)
      }
      frame "Confirm Quit" {
        # "#CodeNeeded - If you want to provide an \"Are you sure\" dialog (or some other notification) before the application exits, place that code here. This message is typically sent from a Panel Close? event."
        # "Confirm Quit - Message that can confirm whether or not the user wants to exit the application."
        n1542 = call-poly "Enqueue Message.vi"("Priority Message? (F)"=TRUE, "error in (no error)"=w2456, "Message"="Exit", "Message Queue"=w2452) -> ("error out"=w2453:errorcluster)  [unwired: 6 in, 1 out]
        n1543 = Merge Errors(w2453) -> (w2454:errorcluster)
      }
      frame "Exit" {
        # "Stop the VI"
        # "Release the message queue reference"
        # "#CodeNeeded - Add any required cleanup code here. Note that if 'Exit' was called as a result of an error, an error dialog will be displayed. Add any custom error handling for an 'Exit' condition here as well."
        # "Exit - Exit the application."
        n1544 = call "Fire User Event - Stop.vi"("User Event - Stop"=w2457) -> ("error out"=w2459:errorcluster)  [unwired: 10 in]
        n1545 = Release Queue(queue=w2464, error in (no error)=w2458) -> (error out=w2461:errorcluster)  [unwired: 1 in, 2 out]
        n1546 = Merge Errors(w2459, w2461) -> (w2460:errorcluster)
      }
      frame Default {
        # "'Default' case only runs if there is a message that isn't defined in any of the other cases.  Output a programming error."
        n1547 = xnode "Error Ring"("parameter 0"=w2465) -> ("error out"=w2466:errorcluster)
      }
    }
    n1548 = call "LAB-IQ Error Handler - Message Handling Loop.vi"("error in (no error)"=w2373, "Message Queue"=w2375) -> ("dup error in"=w2374:errorcluster)  [unwired: 8 in, 1 out]
  }
  n1549 = while {
    shift-right: [w2485] -> _
    shift-left: w15 -> [w2486]
    tunnel: [w2479] -> w20
    tunnel: w6 -> [w2477]
    tunnel: w5 -> [w2476]
    tunnel: w14 -> [w2475]
    stop <- w2484 stop-if-true
    # "Heave Motor  Handling Loop"
    n1550 = call "Dequeue Message.vi"("error in (no error)"=w2476, "Message Queue"=w2477) -> ("error out"=w2483:errorcluster, "Message Data"=w2481:variant, "Message"=w2482:string, "dup Message Queue"=w2480:refnum<queue>)  [unwired: 6 in]
    n1551 = case "Message Cases" shown="\"Heave Main\"" w2482 {
      selector: w2482 -> [_ _ _ _ _ w2557]
      tunnel: w2480 -> [w2499 w2514 _ w2545 w2556 _]
      tunnel: w2483 -> [w2496 w2512 w2535 w2548 w2550 _]
      tunnel: [w2497 w2515 w2529 w2536 w2552 w2558] -> w2478
      tunnel: w2486 -> [w2495 w2502 w2534 w2539 w2555 w2559]
      tunnel: [w2495 w2502 w2534 w2539 w2555 w2559] -> w2485
      tunnel: [_ _ _ _ TRUE _] -> w2484
      tunnel: w2481 -> [_ _ w2533 _ _ _]
      tunnel: w2475 -> [_ _ _ _ w2549 _]
      frame "init" {
        # "Initialize - All initialization work should take place in this message, since other loops can potentially enqueue messages that execute immediately after this one."
        n1552 = call "HEAVE WRITE FGV.vi"("Enum - Menu"=Heave_Write_enum."INIT", "error in (no error)"=w2496, "main ref"=w2495) -> ("error out"=w2494:errorcluster)  [unwired: 8 in]
        n1553 = call <vilib>:"Clear Errors.vi"("error in (no error)"=w2494) -> ("error out"=w2488:errorcluster)  [unwired: 5 in, 1 out]
        n1554 = call "Stall Data Flow.vim"("value in"=w2488, "milliseconds to wait"=u32 1000) -> ("value out"=w2492:errorcluster)  [unwired: 1 out]
        n1555 = call "Heave Init.vi"("error in (no error)"=w2492, "main ref"=w2495) -> ("error out"=w2489:errorcluster)  [unwired: 9 in]
        n1556 = call "HEAVE READ FGV.vi"("Enum - Menu"=Heave_Right_enum."INIT", "error in (no error)"=w2489, "main ref"=w2495) -> ("error out"=w2490:errorcluster)  [unwired: 7 in, 1 out]
        n1557 = call <vilib>:"Clear Errors.vi"("error in (no error)"=w2490) -> ("error out"=w2498:errorcluster)  [unwired: 5 in, 1 out]
        n1558 = call-poly "Enqueue Message.vi"("error in (no error)"=w2498, "Message"="Heave Main", "Message Queue"=w2499) -> ("error out"=w2497:errorcluster)  [unwired: 7 in, 1 out]
      }
      frame "Heave Main" {
        n1559 = Unbundle By Name(w2502) -> ("Heave AND Surge.Read Heave Temp"=w2508:refnum<vi>)
        n1560 = property class="Bool (strict)"(reference=w2508) -> (reference out=w2506:refnum<vi>, error out=w2507:errorcluster, "Value"=w2505:bool)  [unwired: 1 in]
        n1561 = Close Reference(reference=w2506, error in (no error)=w2507) -> ()  [unwired: 1 out]
        n1562 = case shown="True" w2505 {
          tunnel: w2512 -> [w2516 w2520]
          tunnel: [w2516 w2519] -> w2503
          tunnel: w2502 -> [_ w2518]
          frame False {
          }
          frame True {
            n1563 = call "HEAVE READ FGV.vi"("Enum - Menu"=Heave_Right_enum."READ", "error in (no error)"=w2520, "main ref"=w2518) -> ("error out"=w2519:errorcluster)  [unwired: 7 in, 1 out]
          }
        }
        n1564 = call "Heave Reinitial.vi"("error in (no error)"=w2503, "Data Cluster"=w2502) -> ("error out"=w2501:errorcluster)  [unwired: 9 in]
        n1565 = Unbundle By Name(w2502) -> ("Main Home Screen.EXIT"=w2513:refnum<vi>)
        n1566 = property class="Bool (strict)"(reference=w2513) -> (reference out=w2510:refnum<vi>, error out=w2511:errorcluster, "Value"=w2509:bool)  [unwired: 1 in]
        n1567 = call <vilib>:"Clear Errors.vi"("error in (no error)"=w2501) -> ("error out"=w2504:errorcluster)  [unwired: 5 in, 1 out]
        n1568 = Close Reference(reference=w2510, error in (no error)=w2511) -> ()  [unwired: 1 out]
        n1569 = case shown="False" w2509 {
          tunnel: [w2523 w2527] -> w2515
          tunnel: w2514 -> [w2522 w2526]
          tunnel: w2504 -> [w2521 w2525]
          frame True {
            n1570 = call-poly "Enqueue Message.vi"("error in (no error)"=w2521, "Message"="Confirm Quit", "Message Queue"=w2522) -> ("error out"=w2523:errorcluster)  [unwired: 7 in, 1 out]
          }
          frame False {
            n1571 = call-poly "Enqueue Message.vi"("error in (no error)"=w2525, "Message"="Heave Main", "Message Queue"=w2526) -> ("error out"=w2527:errorcluster)  [unwired: 7 in, 1 out]
          }
        }
      }
      frame "Error" {
        # "#CodeRecommended - If you ever change the name of this \"Error\" message, you'll need to update the name in the Check Loop Error.vi as well."
        # "#CodeRecommended - Consider creating a system for logging errors in some way. These errors are for notification purposes only. Handling of specific errors should be performed in the message frames that generated the error."
        # "Error - Display an error dialog. This message is sent by the \"Error Handler\" VIs at the end of other loops in this application."
        n1572 = Variant To Data(error in=w2535, type=errorcluster {"status"=FALSE, "code"=0, "source"=""} ("error constant"), Variant=w2533) -> (data=w2531:errorcluster, error out=w2530:errorcluster)
        n1573 = call <vilib>:"Simple Error Handler.vi"("error in (no error)"=w2531) -> ()  [unwired: 4 in, 5 out]
        n1574 = Merge Errors(w2530) -> (w2529:errorcluster)
      }
      frame "Confirm Quit" {
        # "#CodeNeeded - If you want to provide an \"Are you sure\" dialog (or some other notification) before the application exits, place that code here. This message is typically sent from a Panel Close? event."
        # "Confirm Quit - Message that can confirm whether or not the user wants to exit the application."
        n1575 = call-poly "Enqueue Message.vi"("Priority Message? (F)"=TRUE, "error in (no error)"=w2548, "Message"="Exit", "Message Queue"=w2545) -> ("error out"=w2546:errorcluster)  [unwired: 6 in, 1 out]
        n1576 = Merge Errors(w2546) -> (w2547:errorcluster)
        n1577 = call "HEAVE READ FGV.vi"("Enum - Menu"=Heave_Right_enum."CLOSE", "error in (no error)"=w2547, "main ref"=w2539) -> ("error out"=w2542:errorcluster)  [unwired: 7 in, 1 out]
        n1578 = call <vilib>:"Clear Errors.vi"("error in (no error)"=w2542) -> ("error out"=w2537:errorcluster)  [unwired: 5 in, 1 out]
        n1579 = call "HEAVE WRITE FGV.vi"("Enum - Menu"=Heave_Write_enum."CLOSE", "error in (no error)"=w2537, "main ref"=w2539) -> ("error out"=w2540:errorcluster)  [unwired: 8 in]
        n1580 = call <vilib>:"Clear Errors.vi"("error in (no error)"=w2540) -> ("error out"=w2536:errorcluster)  [unwired: 5 in, 1 out]
      }
      frame "Exit" {
        # "Stop the VI"
        # "Release the message queue reference"
        # "#CodeNeeded - Add any required cleanup code here. Note that if 'Exit' was called as a result of an error, an error dialog will be displayed. Add any custom error handling for an 'Exit' condition here as well."
        # "Exit - Exit the application."
        n1581 = call "Fire User Event - Stop.vi"("User Event - Stop"=w2549) -> ("error out"=w2551:errorcluster)  [unwired: 10 in]
        n1582 = Release Queue(queue=w2556, error in (no error)=w2550) -> (error out=w2553:errorcluster)  [unwired: 1 in, 2 out]
        n1583 = Merge Errors(w2551, w2553) -> (w2552:errorcluster)
      }
      frame Default {
        # "'Default' case only runs if there is a message that isn't defined in any of the other cases.  Output a programming error."
        n1584 = xnode "Error Ring"("parameter 0"=w2557) -> ("error out"=w2558:errorcluster)
      }
    }
    n1585 = call "LAB-IQ Error Handler - Message Handling Loop.vi"("error in (no error)"=w2478, "Message Queue"=w2480) -> ("dup error in"=w2479:errorcluster)  [unwired: 8 in, 1 out]
  }
  n1586 = while {
    shift-right: [w2577] -> _
    shift-left: w15 -> [w2578]
    tunnel: [w2571] -> w2
    tunnel: w21 -> [w2569]
    tunnel: w5 -> [w2568]
    tunnel: w14 -> [w2567]
    stop <- w2576 stop-if-true
    # "Temperature  Handling Loop"
    n1587 = call "Dequeue Message.vi"("error in (no error)"=w2568, "Message Queue"=w2569) -> ("error out"=w2575:errorcluster, "Message Data"=w2573:variant, "Message"=w2574:string, "dup Message Queue"=w2572:refnum<queue>)  [unwired: 6 in]
    n1588 = case "Message Cases" shown="\"Temperature Main\"" w2574 {
      selector: w2574 -> [_ _ _ _ _ w2622]
      tunnel: w2572 -> [w2579 w2590 _ w2609 w2621 _]
      tunnel: w2575 -> [w2582 w2587 w2606 w2613 w2615 _]
      tunnel: [w2583 w2591 w2600 w2611 w2617 w2623] -> w2570
      tunnel: w2578 -> [w2581 w2589 w2605 w2612 w2620 w2624]
      tunnel: [w2581 w2589 w2605 w2612 w2620 w2624] -> w2577
      tunnel: [_ _ _ _ TRUE _] -> w2576
      tunnel: w2573 -> [_ _ w2604 _ _ _]
      tunnel: w2567 -> [_ _ _ _ w2614 _]
      frame "init" {
        # "Initialize - All initialization work should take place in this message, since other loops can potentially enqueue messages that execute immediately after this one."
        n1589 = call-poly "Enqueue Message.vi"("error in (no error)"=w2582, "Message"="Temperature Main", "Message Queue"=w2579) -> ("error out"=w2583:errorcluster)  [unwired: 7 in, 1 out]
      }
      frame "Temperature Main" {
        n1590 = Unbundle By Name(w2589) -> ("Main Home Screen.EXIT"=w2588:refnum<vi>)
        n1591 = property class="Bool (strict)"(reference=w2588) -> (reference out=w2585:refnum<vi>, error out=w2586:errorcluster, "Value"=w2584:bool)  [unwired: 1 in]
        n1592 = case shown="False" w2584 {
          tunnel: [w2594 w2598] -> w2591
          tunnel: w2590 -> [w2593 w2597]
          tunnel: w2587 -> [w2592 w2596]
          frame True {
            n1593 = call-poly "Enqueue Message.vi"("error in (no error)"=w2592, "Message"="Confirm Quit", "Message Queue"=w2593) -> ("error out"=w2594:errorcluster)  [unwired: 7 in, 1 out]
          }
          frame False {
            n1594 = call-poly "Enqueue Message.vi"("error in (no error)"=w2596, "Message"="Temperature Main", "Message Queue"=w2597) -> ("error out"=w2598:errorcluster)  [unwired: 7 in, 1 out]
          }
        }
        n1595 = Close Reference(reference=w2585, error in (no error)=w2586) -> ()  [unwired: 1 out]
      }
      frame "Error" {
        # "#CodeRecommended - If you ever change the name of this \"Error\" message, you'll need to update the name in the Check Loop Error.vi as well."
        # "#CodeRecommended - Consider creating a system for logging errors in some way. These errors are for notification purposes only. Handling of specific errors should be performed in the message frames that generated the error."
        # "Error - Display an error dialog. This message is sent by the \"Error Handler\" VIs at the end of other loops in this application."
        n1596 = Variant To Data(error in=w2606, type=errorcluster {"status"=FALSE, "code"=0, "source"=""} ("error constant"), Variant=w2604) -> (data=w2602:errorcluster, error out=w2601:errorcluster)
        n1597 = call <vilib>:"Simple Error Handler.vi"("error in (no error)"=w2602) -> ()  [unwired: 4 in, 5 out]
        n1598 = Merge Errors(w2601) -> (w2600:errorcluster)
      }
      frame "Confirm Quit" {
        # "#CodeNeeded - If you want to provide an \"Are you sure\" dialog (or some other notification) before the application exits, place that code here. This message is typically sent from a Panel Close? event."
        # "Confirm Quit - Message that can confirm whether or not the user wants to exit the application."
        n1599 = call-poly "Enqueue Message.vi"("Priority Message? (F)"=TRUE, "error in (no error)"=w2613, "Message"="Exit", "Message Queue"=w2609) -> ("error out"=w2610:errorcluster)  [unwired: 6 in, 1 out]
        n1600 = Merge Errors(w2610) -> (w2611:errorcluster)
      }
      frame "Exit" {
        # "Stop the VI"
        # "Release the message queue reference"
        # "#CodeNeeded - Add any required cleanup code here. Note that if 'Exit' was called as a result of an error, an error dialog will be displayed. Add any custom error handling for an 'Exit' condition here as well."
        # "Exit - Exit the application."
        n1601 = call "Fire User Event - Stop.vi"("User Event - Stop"=w2614) -> ("error out"=w2616:errorcluster)  [unwired: 10 in]
        n1602 = Release Queue(queue=w2621, error in (no error)=w2615) -> (error out=w2618:errorcluster)  [unwired: 1 in, 2 out]
        n1603 = Merge Errors(w2616, w2618) -> (w2617:errorcluster)
      }
      frame Default {
        # "'Default' case only runs if there is a message that isn't defined in any of the other cases.  Output a programming error."
        n1604 = xnode "Error Ring"("parameter 0"=w2622) -> ("error out"=w2623:errorcluster)
      }
    }
    n1605 = call "LAB-IQ Error Handler - Message Handling Loop.vi"("error in (no error)"=w2570, "Message Queue"=w2572) -> ("dup error in"=w2571:errorcluster)  [unwired: 8 in, 1 out]
  }
  n1606 = while {
    shift-right: [w2642] -> _
    shift-left: w15 -> [w2643]
    tunnel: [w2636] -> _
    tunnel: w19 -> [w2634]
    tunnel: w5 -> [w2633]
    tunnel: w14 -> [w2632]
    stop <- w2641 stop-if-true
    # "Ramp Motor  Handling Loop"
    n1607 = call "Dequeue Message.vi"("error in (no error)"=w2633, "Message Queue"=w2634) -> ("error out"=w2640:errorcluster, "Message Data"=w2638:variant, "Message"=w2639:string, "dup Message Queue"=w2637:refnum<queue>)  [unwired: 6 in]
    n1608 = case "Message Cases" shown="\"Ramp Main\"" w2639 {
      selector: w2639 -> [_ _ _ _ _ w2687]
      tunnel: w2637 -> [w2644 w2655 _ w2674 w2686 _]
      tunnel: w2640 -> [w2647 w2652 w2671 w2678 w2680 _]
      tunnel: [w2648 w2656 w2665 w2676 w2682 w2688] -> w2635
      tunnel: w2643 -> [w2646 w2654 w2670 w2677 w2685 w2689]
      tunnel: [w2646 w2654 w2670 w2677 w2685 w2689] -> w2642
      tunnel: [_ _ _ _ TRUE _] -> w2641
      tunnel: w2638 -> [_ _ w2669 _ _ _]
      tunnel: w2632 -> [_ _ _ _ w2679 _]
      frame "init" {
        # "Initialize - All initialization work should take place in this message, since other loops can potentially enqueue messages that execute immediately after this one."
        n1609 = call-poly "Enqueue Message.vi"("error in (no error)"=w2647, "Message"="Ramp Main", "Message Queue"=w2644) -> ("error out"=w2648:errorcluster)  [unwired: 7 in, 1 out]
      }
      frame "Ramp Main" {
        n1610 = Unbundle By Name(w2654) -> ("Main Home Screen.EXIT"=w2653:refnum<vi>)
        n1611 = property class="Bool (strict)"(reference=w2653) -> (reference out=w2650:refnum<vi>, error out=w2651:errorcluster, "Value"=w2649:bool)  [unwired: 1 in]
        n1612 = case shown="False" w2649 {
          tunnel: [w2659 w2663] -> w2656
          tunnel: w2655 -> [w2658 w2662]
          tunnel: w2652 -> [w2657 w2661]
          frame True {
            n1613 = call-poly "Enqueue Message.vi"("error in (no error)"=w2657, "Message"="Confirm Quit", "Message Queue"=w2658) -> ("error out"=w2659:errorcluster)  [unwired: 7 in, 1 out]
          }
          frame False {
            n1614 = call-poly "Enqueue Message.vi"("error in (no error)"=w2661, "Message"="Ramp Main", "Message Queue"=w2662) -> ("error out"=w2663:errorcluster)  [unwired: 7 in, 1 out]
          }
        }
        n1615 = Close Reference(reference=w2650, error in (no error)=w2651) -> ()  [unwired: 1 out]
      }
      frame "Error" {
        # "#CodeRecommended - If you ever change the name of this \"Error\" message, you'll need to update the name in the Check Loop Error.vi as well."
        # "#CodeRecommended - Consider creating a system for logging errors in some way. These errors are for notification purposes only. Handling of specific errors should be performed in the message frames that generated the error."
        # "Error - Display an error dialog. This message is sent by the \"Error Handler\" VIs at the end of other loops in this application."
        n1616 = Variant To Data(error in=w2671, type=errorcluster {"status"=FALSE, "code"=0, "source"=""} ("error constant"), Variant=w2669) -> (data=w2667:errorcluster, error out=w2666:errorcluster)
        n1617 = call <vilib>:"Simple Error Handler.vi"("error in (no error)"=w2667) -> ()  [unwired: 4 in, 5 out]
        n1618 = Merge Errors(w2666) -> (w2665:errorcluster)
      }
      frame "Confirm Quit" {
        # "#CodeNeeded - If you want to provide an \"Are you sure\" dialog (or some other notification) before the application exits, place that code here. This message is typically sent from a Panel Close? event."
        # "Confirm Quit - Message that can confirm whether or not the user wants to exit the application."
        n1619 = call-poly "Enqueue Message.vi"("Priority Message? (F)"=TRUE, "error in (no error)"=w2678, "Message"="Exit", "Message Queue"=w2674) -> ("error out"=w2675:errorcluster)  [unwired: 6 in, 1 out]
        n1620 = Merge Errors(w2675) -> (w2676:errorcluster)
      }
      frame "Exit" {
        # "Stop the VI"
        # "Release the message queue reference"
        # "#CodeNeeded - Add any required cleanup code here. Note that if 'Exit' was called as a result of an error, an error dialog will be displayed. Add any custom error handling for an 'Exit' condition here as well."
        # "Exit - Exit the application."
        n1621 = call "Fire User Event - Stop.vi"("User Event - Stop"=w2679) -> ("error out"=w2681:errorcluster)  [unwired: 10 in]
        n1622 = Release Queue(queue=w2686, error in (no error)=w2680) -> (error out=w2683:errorcluster)  [unwired: 1 in, 2 out]
        n1623 = Merge Errors(w2681, w2683) -> (w2682:errorcluster)
      }
      frame Default {
        # "'Default' case only runs if there is a message that isn't defined in any of the other cases.  Output a programming error."
        n1624 = xnode "Error Ring"("parameter 0"=w2687) -> ("error out"=w2688:errorcluster)
      }
    }
    n1625 = call "LAB-IQ Error Handler - Message Handling Loop.vi"("error in (no error)"=w2635, "Message Queue"=w2637) -> ("dup error in"=w2636:errorcluster)  [unwired: 8 in, 1 out]
  }
  n1626 = while {
    shift-right: [w2707] -> _
    shift-left: w15 -> [w2708]
    tunnel: [w2701] -> _
    tunnel: w18 -> [w2699]
    tunnel: w5 -> [w2698]
    tunnel: w14 -> [w2697]
    stop <- w2706 stop-if-true
    # "ECR  Handling Loop"
    n1627 = call "Dequeue Message.vi"("error in (no error)"=w2698, "Message Queue"=w2699) -> ("error out"=w2705:errorcluster, "Message Data"=w2703:variant, "Message"=w2704:string, "dup Message Queue"=w2702:refnum<queue>)  [unwired: 6 in]
    n1628 = case "Message Cases" shown="\"ECR Main\"" w2704 {
      selector: w2704 -> [_ _ _ _ _ w2752]
      tunnel: w2702 -> [w2709 w2720 _ w2739 w2751 _]
      tunnel: w2705 -> [w2712 w2717 w2736 w2743 w2745 _]
      tunnel: [w2713 w2721 w2730 w2741 w2747 w2753] -> w2700
      tunnel: w2708 -> [w2711 w2719 w2735 w2742 w2750 w2754]
      tunnel: [w2711 w2719 w2735 w2742 w2750 w2754] -> w2707
      tunnel: [_ _ _ _ TRUE _] -> w2706
      tunnel: w2703 -> [_ _ w2734 _ _ _]
      tunnel: w2697 -> [_ _ _ _ w2744 _]
      frame "init" {
        # "Initialize - All initialization work should take place in this message, since other loops can potentially enqueue messages that execute immediately after this one."
        n1629 = call-poly "Enqueue Message.vi"("error in (no error)"=w2712, "Message"="ECR Main", "Message Queue"=w2709) -> ("error out"=w2713:errorcluster)  [unwired: 7 in, 1 out]
      }
      frame "ECR Main" {
        n1630 = Unbundle By Name(w2719) -> ("Main Home Screen.EXIT"=w2718:refnum<vi>)
        n1631 = property class="Bool (strict)"(reference=w2718) -> (reference out=w2715:refnum<vi>, error out=w2716:errorcluster, "Value"=w2714:bool)  [unwired: 1 in]
        n1632 = case shown="False" w2714 {
          tunnel: [w2724 w2728] -> w2721
          tunnel: w2720 -> [w2723 w2727]
          tunnel: w2717 -> [w2722 w2726]
          frame True {
            n1633 = call-poly "Enqueue Message.vi"("error in (no error)"=w2722, "Message"="Confirm Quit", "Message Queue"=w2723) -> ("error out"=w2724:errorcluster)  [unwired: 7 in, 1 out]
          }
          frame False {
            n1634 = call-poly "Enqueue Message.vi"("error in (no error)"=w2726, "Message"="ECR Main", "Message Queue"=w2727) -> ("error out"=w2728:errorcluster)  [unwired: 7 in, 1 out]
          }
        }
        n1635 = Close Reference(reference=w2715, error in (no error)=w2716) -> ()  [unwired: 1 out]
      }
      frame "Error" {
        # "#CodeRecommended - If you ever change the name of this \"Error\" message, you'll need to update the name in the Check Loop Error.vi as well."
        # "#CodeRecommended - Consider creating a system for logging errors in some way. These errors are for notification purposes only. Handling of specific errors should be performed in the message frames that generated the error."
        # "Error - Display an error dialog. This message is sent by the \"Error Handler\" VIs at the end of other loops in this application."
        n1636 = Variant To Data(error in=w2736, type=errorcluster {"status"=FALSE, "code"=0, "source"=""} ("error constant"), Variant=w2734) -> (data=w2732:errorcluster, error out=w2731:errorcluster)
        n1637 = call <vilib>:"Simple Error Handler.vi"("error in (no error)"=w2732) -> ()  [unwired: 4 in, 5 out]
        n1638 = Merge Errors(w2731) -> (w2730:errorcluster)
      }
      frame "Confirm Quit" {
        # "#CodeNeeded - If you want to provide an \"Are you sure\" dialog (or some other notification) before the application exits, place that code here. This message is typically sent from a Panel Close? event."
        # "Confirm Quit - Message that can confirm whether or not the user wants to exit the application."
        n1639 = call-poly "Enqueue Message.vi"("Priority Message? (F)"=TRUE, "error in (no error)"=w2743, "Message"="Exit", "Message Queue"=w2739) -> ("error out"=w2740:errorcluster)  [unwired: 6 in, 1 out]
        n1640 = Merge Errors(w2740) -> (w2741:errorcluster)
      }
      frame "Exit" {
        # "Stop the VI"
        # "Release the message queue reference"
        # "#CodeNeeded - Add any required cleanup code here. Note that if 'Exit' was called as a result of an error, an error dialog will be displayed. Add any custom error handling for an 'Exit' condition here as well."
        # "Exit - Exit the application."
        n1641 = call "Fire User Event - Stop.vi"("User Event - Stop"=w2744) -> ("error out"=w2746:errorcluster)  [unwired: 10 in]
        n1642 = Release Queue(queue=w2751, error in (no error)=w2745) -> (error out=w2748:errorcluster)  [unwired: 1 in, 2 out]
        n1643 = Merge Errors(w2746, w2748) -> (w2747:errorcluster)
      }
      frame Default {
        # "'Default' case only runs if there is a message that isn't defined in any of the other cases.  Output a programming error."
        n1644 = xnode "Error Ring"("parameter 0"=w2752) -> ("error out"=w2753:errorcluster)
      }
    }
    n1645 = call "LAB-IQ Error Handler - Message Handling Loop.vi"("error in (no error)"=w2700, "Message Queue"=w2702) -> ("dup error in"=w2701:errorcluster)  [unwired: 8 in, 1 out]
  }
  n1646 = while {
    shift-right: [w2772] -> _
    shift-left: w15 -> [w2773]
    tunnel: [w2766] -> _
    tunnel: w17 -> [w2764]
    tunnel: w5 -> [w2763]
    tunnel: w14 -> [w2762]
    stop <- w2771 stop-if-true
    # "Humidity  Handling Loop"
    n1647 = call "Dequeue Message.vi"("error in (no error)"=w2763, "Message Queue"=w2764) -> ("error out"=w2770:errorcluster, "Message Data"=w2768:variant, "Message"=w2769:string, "dup Message Queue"=w2767:refnum<queue>)  [unwired: 6 in]
    n1648 = case "Message Cases" shown="\"Humidity Main\"" w2769 {
      selector: w2769 -> [_ _ _ _ _ w2817]
      tunnel: w2767 -> [w2774 w2785 _ w2804 w2816 _]
      tunnel: w2770 -> [w2777 w2782 w2801 w2808 w2810 _]
      tunnel: [w2778 w2786 w2795 w2806 w2812 w2818] -> w2765
      tunnel: w2773 -> [w2776 w2784 w2800 w2807 w2815 w2819]
      tunnel: [w2776 w2784 w2800 w2807 w2815 w2819] -> w2772
      tunnel: [_ _ _ _ TRUE _] -> w2771
      tunnel: w2768 -> [_ _ w2799 _ _ _]
      tunnel: w2762 -> [_ _ _ _ w2809 _]
      frame "init" {
        # "Initialize - All initialization work should take place in this message, since other loops can potentially enqueue messages that execute immediately after this one."
        n1649 = call-poly "Enqueue Message.vi"("error in (no error)"=w2777, "Message"="Humidity Main", "Message Queue"=w2774) -> ("error out"=w2778:errorcluster)  [unwired: 7 in, 1 out]
      }
      frame "Humidity Main" {
        n1650 = Unbundle By Name(w2784) -> ("Main Home Screen.EXIT"=w2783:refnum<vi>)
        n1651 = property class="Bool (strict)"(reference=w2783) -> (reference out=w2780:refnum<vi>, error out=w2781:errorcluster, "Value"=w2779:bool)  [unwired: 1 in]
        n1652 = case shown="False" w2779 {
          tunnel: [w2789 w2793] -> w2786
          tunnel: w2785 -> [w2788 w2792]
          tunnel: w2782 -> [w2787 w2791]
          frame True {
            n1653 = call-poly "Enqueue Message.vi"("error in (no error)"=w2787, "Message"="Confirm Quit", "Message Queue"=w2788) -> ("error out"=w2789:errorcluster)  [unwired: 7 in, 1 out]
          }
          frame False {
            n1654 = call-poly "Enqueue Message.vi"("error in (no error)"=w2791, "Message"="Humidity Main", "Message Queue"=w2792) -> ("error out"=w2793:errorcluster)  [unwired: 7 in, 1 out]
          }
        }
        n1655 = Close Reference(reference=w2780, error in (no error)=w2781) -> ()  [unwired: 1 out]
      }
      frame "Error" {
        # "#CodeRecommended - If you ever change the name of this \"Error\" message, you'll need to update the name in the Check Loop Error.vi as well."
        # "#CodeRecommended - Consider creating a system for logging errors in some way. These errors are for notification purposes only. Handling of specific errors should be performed in the message frames that generated the error."
        # "Error - Display an error dialog. This message is sent by the \"Error Handler\" VIs at the end of other loops in this application."
        n1656 = Variant To Data(error in=w2801, type=errorcluster {"status"=FALSE, "code"=0, "source"=""} ("error constant"), Variant=w2799) -> (data=w2797:errorcluster, error out=w2796:errorcluster)
        n1657 = call <vilib>:"Simple Error Handler.vi"("error in (no error)"=w2797) -> ()  [unwired: 4 in, 5 out]
        n1658 = Merge Errors(w2796) -> (w2795:errorcluster)
      }
      frame "Confirm Quit" {
        # "#CodeNeeded - If you want to provide an \"Are you sure\" dialog (or some other notification) before the application exits, place that code here. This message is typically sent from a Panel Close? event."
        # "Confirm Quit - Message that can confirm whether or not the user wants to exit the application."
        n1659 = call-poly "Enqueue Message.vi"("Priority Message? (F)"=TRUE, "error in (no error)"=w2808, "Message"="Exit", "Message Queue"=w2804) -> ("error out"=w2805:errorcluster)  [unwired: 6 in, 1 out]
        n1660 = Merge Errors(w2805) -> (w2806:errorcluster)
      }
      frame "Exit" {
        # "Stop the VI"
        # "Release the message queue reference"
        # "#CodeNeeded - Add any required cleanup code here. Note that if 'Exit' was called as a result of an error, an error dialog will be displayed. Add any custom error handling for an 'Exit' condition here as well."
        # "Exit - Exit the application."
        n1661 = call "Fire User Event - Stop.vi"("User Event - Stop"=w2809) -> ("error out"=w2811:errorcluster)  [unwired: 10 in]
        n1662 = Release Queue(queue=w2816, error in (no error)=w2810) -> (error out=w2813:errorcluster)  [unwired: 1 in, 2 out]
        n1663 = Merge Errors(w2811, w2813) -> (w2812:errorcluster)
      }
      frame Default {
        # "'Default' case only runs if there is a message that isn't defined in any of the other cases.  Output a programming error."
        n1664 = xnode "Error Ring"("parameter 0"=w2817) -> ("error out"=w2818:errorcluster)
      }
    }
    n1665 = call "LAB-IQ Error Handler - Message Handling Loop.vi"("error in (no error)"=w2765, "Message Queue"=w2767) -> ("dup error in"=w2766:errorcluster)  [unwired: 8 in, 1 out]
  }
  n1666 = while {
    shift-right: [w2837] -> _
    shift-left: w15 -> [w2838]
    tunnel: [w2831] -> _
    tunnel: w16 -> [w2829]
    tunnel: w5 -> [w2828]
    tunnel: w14 -> [w2827]
    stop <- w2836 stop-if-true
    # "Program  Handling Loop"
    n1667 = call "Dequeue Message.vi"("error in (no error)"=w2828, "Message Queue"=w2829) -> ("error out"=w2835:errorcluster, "Message Data"=w2833:variant, "Message"=w2834:string, "dup Message Queue"=w2832:refnum<queue>)  [unwired: 6 in]
    n1668 = case "Message Cases" shown="\"Program Main\"" w2834 {
      selector: w2834 -> [_ _ _ _ _ w2883]
      tunnel: w2832 -> [w2839 w2851 _ w2870 w2882 _]
      tunnel: w2835 -> [w2842 w2845 w2867 w2874 w2876 _]
      tunnel: [w2843 w2852 w2861 w2872 w2878 w2884] -> w2830
      tunnel: w2838 -> [w2841 w2844 w2866 w2873 w2881 w2885]
      tunnel: [w2841 w2844 w2866 w2873 w2881 w2885] -> w2837
      tunnel: [_ _ _ _ TRUE _] -> w2836
      tunnel: w2833 -> [_ _ w2865 _ _ _]
      tunnel: w2827 -> [_ _ _ _ w2875 _]
      frame "init" {
        # "Initialize - All initialization work should take place in this message, since other loops can potentially enqueue messages that execute immediately after this one."
        n1669 = call-poly "Enqueue Message.vi"("error in (no error)"=w2842, "Message"="Program Main", "Message Queue"=w2839) -> ("error out"=w2843:errorcluster)  [unwired: 7 in, 1 out]
      }
      frame "Program Main" {
        n1670 = call "Main Program Loop Vi.vi"("error in (no error)"=w2845, "Data Cluster"=w2844) -> ("error out"=w2846:errorcluster)  [unwired: 9 in]
        n1671 = Unbundle By Name(w2844) -> ("Main Home Screen.EXIT"=w2850:refnum<vi>)
        n1672 = property class="Bool (strict)"(reference=w2850) -> (reference out=w2848:refnum<vi>, error out=w2849:errorcluster, "Value"=w2847:bool)  [unwired: 1 in]
        n1673 = case shown="False" w2847 {
          tunnel: [w2855 w2859] -> w2852
          tunnel: w2851 -> [w2854 w2858]
          tunnel: w2846 -> [w2853 w2857]
          frame True {
            n1674 = call-poly "Enqueue Message.vi"("error in (no error)"=w2853, "Message"="Confirm Quit", "Message Queue"=w2854) -> ("error out"=w2855:errorcluster)  [unwired: 7 in, 1 out]
          }
          frame False {
            n1675 = call-poly "Enqueue Message.vi"("error in (no error)"=w2857, "Message"="Program Main", "Message Queue"=w2858) -> ("error out"=w2859:errorcluster)  [unwired: 7 in, 1 out]
          }
        }
        n1676 = Close Reference(reference=w2848, error in (no error)=w2849) -> ()  [unwired: 1 out]
      }
      frame "Error" {
        # "#CodeRecommended - If you ever change the name of this \"Error\" message, you'll need to update the name in the Check Loop Error.vi as well."
        # "#CodeRecommended - Consider creating a system for logging errors in some way. These errors are for notification purposes only. Handling of specific errors should be performed in the message frames that generated the error."
        # "Error - Display an error dialog. This message is sent by the \"Error Handler\" VIs at the end of other loops in this application."
        n1677 = Variant To Data(error in=w2867, type=errorcluster {"status"=FALSE, "code"=0, "source"=""} ("error constant"), Variant=w2865) -> (data=w2863:errorcluster, error out=w2862:errorcluster)
        n1678 = call <vilib>:"Simple Error Handler.vi"("error in (no error)"=w2863) -> ()  [unwired: 4 in, 5 out]
        n1679 = Merge Errors(w2862) -> (w2861:errorcluster)
      }
      frame "Confirm Quit" {
        # "#CodeNeeded - If you want to provide an \"Are you sure\" dialog (or some other notification) before the application exits, place that code here. This message is typically sent from a Panel Close? event."
        # "Confirm Quit - Message that can confirm whether or not the user wants to exit the application."
        n1680 = call-poly "Enqueue Message.vi"("Priority Message? (F)"=TRUE, "error in (no error)"=w2874, "Message"="Exit", "Message Queue"=w2870) -> ("error out"=w2871:errorcluster)  [unwired: 6 in, 1 out]
        n1681 = Merge Errors(w2871) -> (w2872:errorcluster)
      }
      frame "Exit" {
        # "Stop the VI"
        # "Release the message queue reference"
        # "#CodeNeeded - Add any required cleanup code here. Note that if 'Exit' was called as a result of an error, an error dialog will be displayed. Add any custom error handling for an 'Exit' condition here as well."
        # "Exit - Exit the application."
        n1682 = call "Fire User Event - Stop.vi"("User Event - Stop"=w2875) -> ("error out"=w2877:errorcluster)  [unwired: 10 in]
        n1683 = Release Queue(queue=w2882, error in (no error)=w2876) -> (error out=w2879:errorcluster)  [unwired: 1 in, 2 out]
        n1684 = Merge Errors(w2877, w2879) -> (w2878:errorcluster)
      }
      frame Default {
        # "'Default' case only runs if there is a message that isn't defined in any of the other cases.  Output a programming error."
        n1685 = xnode "Error Ring"("parameter 0"=w2883) -> ("error out"=w2884:errorcluster)
      }
    }
    n1686 = call "LAB-IQ Error Handler - Message Handling Loop.vi"("error in (no error)"=w2830, "Message Queue"=w2832) -> ("dup error in"=w2831:errorcluster)  [unwired: 8 in, 1 out]
  }
  n1687 = while {
    shift-right: [w2903] -> _
    shift-left: w15 -> [w2904]
    tunnel: [w2897] -> _
    tunnel: w13 -> [w2895]
    tunnel: w5 -> [w2894]
    tunnel: w14 -> [w2893]
    stop <- w2902 stop-if-true
    # "Monitor  Handling Loop"
    n1688 = call "Dequeue Message.vi"("error in (no error)"=w2894, "Message Queue"=w2895) -> ("error out"=w2901:errorcluster, "Message Data"=w2899:variant, "Message"=w2900:string, "dup Message Queue"=w2898:refnum<queue>)  [unwired: 6 in]
    n1689 = case "Message Cases" shown="\"Monitor Main\"" w2900 {
      selector: w2900 -> [_ _ _ _ _ w2952]
      tunnel: w2898 -> [w2905 w2920 _ w2939 w2951 _]
      tunnel: w2901 -> [w2908 w2913 w2936 w2943 w2945 _]
      tunnel: [w2909 w2921 w2930 w2941 w2947 w2953] -> w2896
      tunnel: w2904 -> [w2907 w2914 w2935 w2942 w2950 w2954]
      tunnel: [w2907 w2914 w2935 w2942 w2950 w2954] -> w2903
      tunnel: [_ _ _ _ TRUE _] -> w2902
      tunnel: w2899 -> [_ _ w2934 _ _ _]
      tunnel: w2893 -> [_ _ _ _ w2944 _]
      frame "init" {
        # "Initialize - All initialization work should take place in this message, since other loops can potentially enqueue messages that execute immediately after this one."
        n1690 = call-poly "Enqueue Message.vi"("error in (no error)"=w2908, "Message"="Monitor Main", "Message Queue"=w2905) -> ("error out"=w2909:errorcluster)  [unwired: 7 in, 1 out]
      }
      frame "Monitor Main" {
        n1691 = call "Main Monitor Loop.vi"("error in (no error)"=w2913, "main ref"=w2914) -> ("error out"=w2915:errorcluster)  [unwired: 9 in]
        n1692 = call "LOAD SELECTION MAIN CODE.vi"("error in (no error)"=w2913, "main ref"=w2914) -> ("error out"=w2911:errorcluster)  [unwired: 9 in]
        n1693 = call "Trip Log and Trip Monitor.vi"("error in (no error)"=w2913, "main ref"=w2914) -> ("error out"=w2910:errorcluster)  [unwired: 9 in]
        n1694 = Merge Errors(w2915, w2911, w2910) -> (w2912:errorcluster)
        n1695 = Unbundle By Name(w2914) -> ("Main Home Screen.EXIT"=w2919:refnum<vi>)
        n1696 = property class="Bool (strict)"(reference=w2919) -> (reference out=w2917:refnum<vi>, error out=w2918:errorcluster, "Value"=w2916:bool)  [unwired: 1 in]
        n1697 = case shown="False" w2916 {
          tunnel: [w2924 w2928] -> w2921
          tunnel: w2920 -> [w2923 w2927]
          tunnel: w2912 -> [w2922 w2926]
          frame True {
            n1698 = call-poly "Enqueue Message.vi"("error in (no error)"=w2922, "Message"="Confirm Quit", "Message Queue"=w2923) -> ("error out"=w2924:errorcluster)  [unwired: 7 in, 1 out]
          }
          frame False {
            n1699 = call-poly "Enqueue Message.vi"("error in (no error)"=w2926, "Message"="Monitor Main", "Message Queue"=w2927) -> ("error out"=w2928:errorcluster)  [unwired: 7 in, 1 out]
          }
        }
        n1700 = Close Reference(reference=w2917, error in (no error)=w2918) -> ()  [unwired: 1 out]
      }
      frame "Error" {
        # "#CodeRecommended - If you ever change the name of this \"Error\" message, you'll need to update the name in the Check Loop Error.vi as well."
        # "#CodeRecommended - Consider creating a system for logging errors in some way. These errors are for notification purposes only. Handling of specific errors should be performed in the message frames that generated the error."
        # "Error - Display an error dialog. This message is sent by the \"Error Handler\" VIs at the end of other loops in this application."
        n1701 = Variant To Data(error in=w2936, type=errorcluster {"status"=FALSE, "code"=0, "source"=""} ("error constant"), Variant=w2934) -> (data=w2932:errorcluster, error out=w2931:errorcluster)
        n1702 = call <vilib>:"Simple Error Handler.vi"("error in (no error)"=w2932) -> ()  [unwired: 4 in, 5 out]
        n1703 = Merge Errors(w2931) -> (w2930:errorcluster)
      }
      frame "Confirm Quit" {
        # "#CodeNeeded - If you want to provide an \"Are you sure\" dialog (or some other notification) before the application exits, place that code here. This message is typically sent from a Panel Close? event."
        # "Confirm Quit - Message that can confirm whether or not the user wants to exit the application."
        n1704 = call-poly "Enqueue Message.vi"("Priority Message? (F)"=TRUE, "error in (no error)"=w2943, "Message"="Exit", "Message Queue"=w2939) -> ("error out"=w2940:errorcluster)  [unwired: 6 in, 1 out]
        n1705 = Merge Errors(w2940) -> (w2941:errorcluster)
      }
      frame "Exit" {
        # "Stop the VI"
        # "Release the message queue reference"
        # "#CodeNeeded - Add any required cleanup code here. Note that if 'Exit' was called as a result of an error, an error dialog will be displayed. Add any custom error handling for an 'Exit' condition here as well."
        # "Exit - Exit the application."
        n1706 = call "Fire User Event - Stop.vi"("User Event - Stop"=w2944) -> ("error out"=w2946:errorcluster)  [unwired: 10 in]
        n1707 = Release Queue(queue=w2951, error in (no error)=w2945) -> (error out=w2948:errorcluster)  [unwired: 1 in, 2 out]
        n1708 = Merge Errors(w2946, w2948) -> (w2947:errorcluster)
      }
      frame Default {
        # "'Default' case only runs if there is a message that isn't defined in any of the other cases.  Output a programming error."
        n1709 = xnode "Error Ring"("parameter 0"=w2952) -> ("error out"=w2953:errorcluster)
      }
    }
    n1710 = call "LAB-IQ Error Handler - Message Handling Loop.vi"("error in (no error)"=w2896, "Message Queue"=w2898) -> ("dup error in"=w2897:errorcluster)  [unwired: 8 in, 1 out]
  }
  n1711 = while {
    shift-right: [w2972] -> _
    shift-left: w15 -> [w2973]
    tunnel: [w2966] -> _
    tunnel: w12 -> [w2964]
    tunnel: w5 -> [w2963]
    tunnel: w14 -> [w2962]
    stop <- w2971 stop-if-true
    # "Load Pid  Handling Loop"
    n1712 = call "Dequeue Message.vi"("error in (no error)"=w2963, "Message Queue"=w2964) -> ("error out"=w2970:errorcluster, "Message Data"=w2968:variant, "Message"=w2969:string, "dup Message Queue"=w2967:refnum<queue>)  [unwired: 6 in]
    n1713 = case "Message Cases" shown="\"Load Pid Main\"" w2969 {
      selector: w2969 -> [_ _ _ _ _ w3038]
      tunnel: w2967 -> [w2974 w2995 _ w3025 w3037 _]
      tunnel: w2970 -> [w2977 w2993 w3022 w3029 w3031 _]
      tunnel: [w2978 w2996 w3016 w3027 w3033 w3039] -> w2965
      tunnel: w2973 -> [w2976 w2982 w3021 w3028 w3036 w3040]
      tunnel: [w2976 w2982 w3021 w3028 w3036 w3040] -> w2972
      tunnel: [_ _ _ _ TRUE _] -> w2971
      tunnel: w2968 -> [_ _ w3020 _ _ _]
      tunnel: w2962 -> [_ _ _ _ w3030 _]
      frame "init" {
        # "Initialize - All initialization work should take place in this message, since other loops can potentially enqueue messages that execute immediately after this one."
        n1714 = call-poly "Enqueue Message.vi"("error in (no error)"=w2977, "Message"="Load Pid Main", "Message Queue"=w2974) -> ("error out"=w2978:errorcluster)  [unwired: 7 in, 1 out]
      }
      frame "Load Pid Main" {
        n1715 = Unbundle By Name(w2982) -> ("Main Screen.Load En"=w2988:refnum<vi>)
        n1716 = Unbundle By Name(w2982) -> ("PID.apply load"=w2983:refnum<vi>)
        n1717 = property class="Bool (strict)"(reference=w2988) -> (reference out=w2986:refnum<vi>, error out=w2987:errorcluster, "Value"=w2981:bool)  [unwired: 1 in]
        n1718 = property class="Bool (strict)"(reference=w2983) -> (reference out=w2985:refnum<vi>, error out=w2984:errorcluster, "Value"=w2980:bool)  [unwired: 1 in]
        n1719 = Close Reference(reference=w2986, error in (no error)=w2987) -> ()  [unwired: 1 out]
        n1720 = Close Reference(reference=w2985, error in (no error)=w2984) -> ()  [unwired: 1 out]
        n1721 = Or(x=w2981, y=w2980) -> (x .or. y?=w2979:bool)
        n1722 = case shown="True" w2979 {
          tunnel: w2993 -> [w2997 w3000]
          tunnel: [w2997 w2999] -> w2989
          tunnel: w2982 -> [_ w2998]
          frame False {
          }
          frame True {
            n1723 = disable-structure shown="Enabled" {
              disable-tunnel: w3000 -> [w3003 w3007]
              disable-tunnel: [w3002 w3006] -> w2999
              disable-tunnel: w2998 -> [w3001 w3005]
              frame Disabled {
                n1724 = call "load pid.vi"("error in (no error)"=w3003, "main ref"=w3001) -> ("error out"=w3002:errorcluster)  [unwired: 9 in]
              }
              frame Enabled {
                n1725 = call "NEW LOAD CELL PID.vi"("error in (no error)"=w3007, "Checkbox"=TRUE, "main ref"=w3005) -> ("error out"=w3006:errorcluster)  [unwired: 8 in]
              }
            }
          }
        }
        n1726 = Unbundle By Name(w2982) -> ("Main Home Screen.EXIT"=w2994:refnum<vi>)
        n1727 = property class="Bool (strict)"(reference=w2994) -> (reference out=w2991:refnum<vi>, error out=w2992:errorcluster, "Value"=w2990:bool)  [unwired: 1 in]
        n1728 = case shown="False" w2990 {
          tunnel: [w3010 w3014] -> w2996
          tunnel: w2995 -> [w3009 w3013]
          tunnel: w2989 -> [w3008 w3012]
          frame True {
            n1729 = call-poly "Enqueue Message.vi"("error in (no error)"=w3008, "Message"="Confirm Quit", "Message Queue"=w3009) -> ("error out"=w3010:errorcluster)  [unwired: 7 in, 1 out]
          }
          frame False {
            n1730 = call-poly "Enqueue Message.vi"("error in (no error)"=w3012, "Message"="Load Pid Main", "Message Queue"=w3013) -> ("error out"=w3014:errorcluster)  [unwired: 7 in, 1 out]
          }
        }
        n1731 = Close Reference(reference=w2991, error in (no error)=w2992) -> ()  [unwired: 1 out]
      }
      frame "Error" {
        # "#CodeRecommended - If you ever change the name of this \"Error\" message, you'll need to update the name in the Check Loop Error.vi as well."
        # "#CodeRecommended - Consider creating a system for logging errors in some way. These errors are for notification purposes only. Handling of specific errors should be performed in the message frames that generated the error."
        # "Error - Display an error dialog. This message is sent by the \"Error Handler\" VIs at the end of other loops in this application."
        n1732 = Variant To Data(error in=w3022, type=errorcluster {"status"=FALSE, "code"=0, "source"=""} ("error constant"), Variant=w3020) -> (data=w3018:errorcluster, error out=w3017:errorcluster)
        n1733 = call <vilib>:"Simple Error Handler.vi"("error in (no error)"=w3018) -> ()  [unwired: 4 in, 5 out]
        n1734 = Merge Errors(w3017) -> (w3016:errorcluster)
      }
      frame "Confirm Quit" {
        # "#CodeNeeded - If you want to provide an \"Are you sure\" dialog (or some other notification) before the application exits, place that code here. This message is typically sent from a Panel Close? event."
        # "Confirm Quit - Message that can confirm whether or not the user wants to exit the application."
        n1735 = call-poly "Enqueue Message.vi"("Priority Message? (F)"=TRUE, "error in (no error)"=w3029, "Message"="Exit", "Message Queue"=w3025) -> ("error out"=w3026:errorcluster)  [unwired: 6 in, 1 out]
        n1736 = Merge Errors(w3026) -> (w3027:errorcluster)
      }
      frame "Exit" {
        # "Stop the VI"
        # "Release the message queue reference"
        # "#CodeNeeded - Add any required cleanup code here. Note that if 'Exit' was called as a result of an error, an error dialog will be displayed. Add any custom error handling for an 'Exit' condition here as well."
        # "Exit - Exit the application."
        n1737 = call "Fire User Event - Stop.vi"("User Event - Stop"=w3030) -> ("error out"=w3032:errorcluster)  [unwired: 10 in]
        n1738 = Release Queue(queue=w3037, error in (no error)=w3031) -> (error out=w3034:errorcluster)  [unwired: 1 in, 2 out]
        n1739 = Merge Errors(w3032, w3034) -> (w3033:errorcluster)
      }
      frame Default {
        # "'Default' case only runs if there is a message that isn't defined in any of the other cases.  Output a programming error."
        n1740 = xnode "Error Ring"("parameter 0"=w3038) -> ("error out"=w3039:errorcluster)
      }
    }
    n1741 = call "LAB-IQ Error Handler - Message Handling Loop.vi"("error in (no error)"=w2965, "Message Queue"=w2967) -> ("dup error in"=w2966:errorcluster)  [unwired: 8 in, 1 out]
  }
  n1742 = while {
    shift-right: [w3058] -> _
    shift-left: w15 -> [w3059]
    tunnel: [w3052] -> _
    tunnel: w11 -> [w3050]
    tunnel: w5 -> [w3049]
    tunnel: w14 -> [w3048]
    stop <- w3057 stop-if-true
    # "Report  Handling Loop"
    n1743 = call "Dequeue Message.vi"("error in (no error)"=w3049, "Message Queue"=w3050) -> ("error out"=w3056:errorcluster, "Message Data"=w3054:variant, "Message"=w3055:string, "dup Message Queue"=w3053:refnum<queue>)  [unwired: 6 in]
    n1744 = case "Message Cases" shown="\"Report Main\"" w3055 {
      selector: w3055 -> [_ _ _ _ _ w3104]
      tunnel: w3053 -> [w3060 w3072 _ w3091 w3103 _]
      tunnel: w3056 -> [w3063 w3070 w3088 w3095 w3097 _]
      tunnel: [w3064 w3073 w3082 w3093 w3099 w3105] -> w3051
      tunnel: w3059 -> [w3062 w3065 w3087 w3094 w3102 w3106]
      tunnel: [w3062 w3065 w3087 w3094 w3102 w3106] -> w3058
      tunnel: [_ _ _ _ TRUE _] -> w3057
      tunnel: w3054 -> [_ _ w3086 _ _ _]
      tunnel: w3048 -> [_ _ _ _ w3096 _]
      frame "init" {
        # "Initialize - All initialization work should take place in this message, since other loops can potentially enqueue messages that execute immediately after this one."
        n1745 = call-poly "Enqueue Message.vi"("error in (no error)"=w3063, "Message"="Report Main", "Message Queue"=w3060) -> ("error out"=w3064:errorcluster)  [unwired: 7 in, 1 out]
      }
      frame "Report Main" {
        n1746 = call "Main Data Log.vi"("error in (no error)"=w3070, "main ref"=w3065) -> ("error out"=w3066:errorcluster)  [unwired: 9 in]
        n1747 = Unbundle By Name(w3065) -> ("Main Home Screen.EXIT"=w3071:refnum<vi>)
        n1748 = property class="Bool (strict)"(reference=w3071) -> (reference out=w3068:refnum<vi>, error out=w3069:errorcluster, "Value"=w3067:bool)  [unwired: 1 in]
        n1749 = case shown="False" w3067 {
          tunnel: [w3076 w3080] -> w3073
          tunnel: w3072 -> [w3075 w3079]
          tunnel: w3066 -> [w3074 w3078]
          frame True {
            n1750 = call-poly "Enqueue Message.vi"("error in (no error)"=w3074, "Message"="Confirm Quit", "Message Queue"=w3075) -> ("error out"=w3076:errorcluster)  [unwired: 7 in, 1 out]
          }
          frame False {
            n1751 = call-poly "Enqueue Message.vi"("error in (no error)"=w3078, "Message"="Report Main", "Message Queue"=w3079) -> ("error out"=w3080:errorcluster)  [unwired: 7 in, 1 out]
          }
        }
        n1752 = Close Reference(reference=w3068, error in (no error)=w3069) -> ()  [unwired: 1 out]
      }
      frame "Error" {
        # "#CodeRecommended - If you ever change the name of this \"Error\" message, you'll need to update the name in the Check Loop Error.vi as well."
        # "#CodeRecommended - Consider creating a system for logging errors in some way. These errors are for notification purposes only. Handling of specific errors should be performed in the message frames that generated the error."
        # "Error - Display an error dialog. This message is sent by the \"Error Handler\" VIs at the end of other loops in this application."
        n1753 = Variant To Data(error in=w3088, type=errorcluster {"status"=FALSE, "code"=0, "source"=""} ("error constant"), Variant=w3086) -> (data=w3084:errorcluster, error out=w3083:errorcluster)
        n1754 = call <vilib>:"Simple Error Handler.vi"("error in (no error)"=w3084) -> ()  [unwired: 4 in, 5 out]
        n1755 = Merge Errors(w3083) -> (w3082:errorcluster)
      }
      frame "Confirm Quit" {
        # "#CodeNeeded - If you want to provide an \"Are you sure\" dialog (or some other notification) before the application exits, place that code here. This message is typically sent from a Panel Close? event."
        # "Confirm Quit - Message that can confirm whether or not the user wants to exit the application."
        n1756 = call-poly "Enqueue Message.vi"("Priority Message? (F)"=TRUE, "error in (no error)"=w3095, "Message"="Exit", "Message Queue"=w3091) -> ("error out"=w3092:errorcluster)  [unwired: 6 in, 1 out]
        n1757 = Merge Errors(w3092) -> (w3093:errorcluster)
      }
      frame "Exit" {
        # "Stop the VI"
        # "Release the message queue reference"
        # "#CodeNeeded - Add any required cleanup code here. Note that if 'Exit' was called as a result of an error, an error dialog will be displayed. Add any custom error handling for an 'Exit' condition here as well."
        # "Exit - Exit the application."
        n1758 = call "Fire User Event - Stop.vi"("User Event - Stop"=w3096) -> ("error out"=w3098:errorcluster)  [unwired: 10 in]
        n1759 = Release Queue(queue=w3103, error in (no error)=w3097) -> (error out=w3100:errorcluster)  [unwired: 1 in, 2 out]
        n1760 = Merge Errors(w3098, w3100) -> (w3099:errorcluster)
      }
      frame Default {
        # "'Default' case only runs if there is a message that isn't defined in any of the other cases.  Output a programming error."
        n1761 = xnode "Error Ring"("parameter 0"=w3104) -> ("error out"=w3105:errorcluster)
      }
    }
    n1762 = call "LAB-IQ Error Handler - Message Handling Loop.vi"("error in (no error)"=w3051, "Message Queue"=w3053) -> ("dup error in"=w3052:errorcluster)  [unwired: 8 in, 1 out]
  }
  n1763 = Unregister For Events(event registration refnum=w49, error in=w47) -> (error out=w50:errorcluster)
  n1764 = Merge Errors(w50, w53, w25, w22, w20, w2) -> (w51:errorcluster)
  n1765 = call "Destroy User Event - Stop.vi"("error in (no error)"=w51, "User Event - Stop"=w14) -> ("error out"=w48:errorcluster)  [unwired: 9 in]
  n1766 = disable-structure shown="RUN_TIME_ENGINE==True" {
    disable-tunnel: w48 -> [_ _]
    frame condition #0 (active) {
    }
    frame condition #1 {
      # "Call Quit LabVIEW if running as a built application."
      n1767 = Quit LabVIEW() -> ()  [unwired: 1 in]
    }
  }
